vi "tvac_gui_chamber.vi"() -> ()   [LabVIEW 2017]
doc: "GUI For Thermal Vacuum Chamber - Rev 1.0 by S.O. 11/6/2017"
uses:
  Type_Defs/Zones.ctl
  Type_Defs/generalStatus.ctl
  Type_Defs/Digital_In_1.ctl
  Type_Defs/Digital_In_SW_States.ctl
  Type_Defs/Digital_In_SW_Wire_Faults.ctl
  Type_Defs/Cryo_Pump_MCC_Status.ctl
  Type_Defs/Cryo_Pump_MCC_CryoPump.ctl
  Type_Defs/Cryo_Pump_MCC_RoughingInterlock.ctl
  Type_Defs/Cryo_Pump_MCC_Status_Status.ctl
  Type_Defs/Cryo_Pump_Compressor_Status.ctl
  Type_Defs/Cryo_Pump_Compressor_Status_Status.ctl
  <vilib>/httpClient/ClientHandle.ctl
  <vilib>/Utility/miscctls.llb/LVPositionTypeDef.ctl
  <vilib>/Utility/error.llb/DialogType.ctl
  Type_Defs/Cryo_Pump_Plots.ctl
  <vilib>/Utility/miscctls.llb/LVBoundsTypeDef.ctl
  msg7171_linux.llb/send single message.vi
  <vilib>/httpClient/POSTBuffer.vi
  <vilib>/Utility/file.llb/Read Delimited Spreadsheet (string).vi
  <vilib>/Utility/file.llb/Write Delimited Spreadsheet (string).vi
  <vilib>/httpClient/LabVIEWHTTPClient.lvlib
panel:
  out "UTC":string
  out "Local Time":string
  out "Taskbar Status":T1 {"Chamber" format="%#_2g"; "Cryo" format="%#_2g"; "Roughing" format="%#_2g"}
  in  "importexe":dbl
  in  "Path to PNG file":path=path "C:/Users/stefan/Documents/GitHub/TVAC/head/Labview2017/TVAC_GUI/Visualization/chamber_test.png"
  in  "Moving 1":bool
  in  "TC1to45PicRef":refnum<vi>
  in  "profilearray":dbl[][](array[numeric])
  in  "LastSetPt":i32
  in  "string":string
  in  "tprofilesheet":string[][](array[string])
  in  "Custom Graph Selector":i32
  in  "exit":bool
  in  "AlarmColor":u32(colorbox)
  in  "Alarm String":string
  in  "Plot Color":u32(colorbox)=16860
  in  "Temperature":dbl format="%#_13g"
  in  "TC Label":string
  in  "Graph ON/OFF":u32(colorbox)=4250624
  in  "index (col)":i32
  in  "index (row)":i32
  out "working array":bool[](array[boolean])
  in  "Tab Control":T2(tab)
  in  "Log/Linear Y-Axis":u16(ring) items=["Linear", "Log"]
  in  "Total Time":dbl
  in  "Set Time TC Graph":bool
  in  "Graphing Selection":u16(ring) items=["User Selection", "Graph All Thermocouples", "Clear Graph"]
  in  "Time Scale":u16(ring) items=["Minutes", "Hours", "Seconds"]
  out "Waveform Chart":waveform(dbl)[](graph)
  out "Thermocouples":T3(array[cluster])
  in  "Log/Linear Y-Axis 6":u16(ring) items=["Linear", "Log"]
  in  "Log/Linear Y-Axis 5":u16(ring) items=["Linear", "Log"]
  in  "Log/Linear Y-Axis 3":u16(ring) items=["Linear", "Log"]
  in  "Log/Linear Y-Axis 2":u16(ring) items=["Linear", "Log"]
  in  "Total Time 6":dbl=30.0
  in  "Set Time TC Graph 6":bool
  in  "Time Scale 6":u16(ring) items=["Minutes", "Hours", "Seconds"]
  in  "Total Time 5":dbl=30.0
  in  "Set Time TC Graph 5":bool
  in  "Time Scale 5":u16(ring) items=["Minutes", "Hours", "Seconds"]
  in  "Total Time 4":dbl=30.0
  in  "Set Time TC Graph 4":bool
  in  "Time Scale 4":u16(ring) items=["Minutes", "Hours", "Seconds"]
  in  "Total Time 3":dbl=30.0
  in  "Set Time TC Graph 3":bool
  in  "Time Scale 3":u16(ring) items=["Minutes", "Hours", "Seconds"]
  in  "Total Time 2":dbl=30.0
  in  "Set Time TC Graph 2":bool
  in  "Time Scale 2":u16(ring) items=["Minutes", "Hours", "Seconds"]
  in  "Log/Linear Y-Axis 1":u16(ring) items=["Linear", "Log"]
  in  "Total Time 1":dbl=30.0
  in  "Set Time TC Graph 1":bool
  in  "Time Scale 1":u16(ring) items=["Minutes", "Hours", "Seconds"]
  in  "Custom Chart 2 Selection":i32[](listbox)=[0]
  in  "Custom Chart 1 Selection":i32[](listbox)=[0]
  out "Custom Chart 1":waveform(dbl)[](graph)
  in  "Custom Chart 3 Selection":i32[](listbox)=[0]
  in  "Custom Chart 4 Selection":i32[](listbox)=[0]
  in  "Custom Chart 5 Selection":i32[](listbox)=[0]
  in  "Custom Chart 6 Selection":i32[](listbox)=[0]
  out "Custom Chart 2":waveform(dbl)[](graph)
  out "Custom Chart 3":waveform(dbl)[](graph)
  out "Custom Chart 4":waveform(dbl)[](graph)
  out "Custom Chart 5":waveform(dbl)[](graph)
  out "Custom Chart 6":waveform(dbl)[](graph)
  in  "Log/Linear Y-Axis 4":u16(ring) items=["Linear", "Log"]
  in  "Complete Event List":i32(listbox)
  in  "Database Logging On/Off":bool
  out "Thermal Profile Compiling Summary":string
  out "Active Profile":bool
  out "ThermalProfileStatus":string
  out "Thermal Profile":cluster{dbl, dbl, "temp":dbl[][]}(graph)
  in  "Thermal Profile Loader":T4(tab)
  in  "ZoneSetup":T5={"Number of Set points"=0.0, "Zone Selection"=[8], "Initiate Setup"=FALSE, "Thermal Profile Name"="", "Saved Database Profiles"=0, "Import CSV as a Thermal Profile"=path "C:/Users/stefan/Documents/GitHub/TVAC/head/Labview2017/TVAC_GUI/DatabaseCSV/start.csv", "Import Profile"=FALSE, "LoadFromDatabase"=FALSE} {"Saved Database Profiles" items=["debug2"]}
  in  "RampSoakTimes":cluster{"RampSoakTimes":dbl[][]}
  in  "Zone 1":T6={"Zone Thermocouples"=[0], "Temperature Calculation"=0, "Thermocouples Selected"="", "Temperature Goal"=[], "Max Allowable Temp"="", "Min Allowable Temp"="", "Max Temp Slope (K/min)  "=""} {"Temperature Calculation" items=["Average", "Minimum", "Maximum"]}
  in  "Zone 2":T6={"Zone Thermocouples"=[0], "Temperature Calculation"=0, "Thermocouples Selected"="", "Temperature Goal"=[], "Max Allowable Temp"="", "Min Allowable Temp"="", "Max Temp Slope (K/min)  "=""} {"Temperature Calculation" items=["Average", "Minimum", "Maximum"]}
  in  "Zone 3":T6={"Zone Thermocouples"=[0], "Temperature Calculation"=0, "Thermocouples Selected"="", "Temperature Goal"=[], "Max Allowable Temp"="", "Min Allowable Temp"="", "Max Temp Slope (K/min)  "=""} {"Temperature Calculation" items=["Average", "Minimum", "Maximum"]}
  in  "Zone 4":T6={"Zone Thermocouples"=[0], "Temperature Calculation"=0, "Thermocouples Selected"="", "Temperature Goal"=[], "Max Allowable Temp"="", "Min Allowable Temp"="", "Max Temp Slope (K/min)  "=""} {"Temperature Calculation" items=["Average", "Minimum", "Maximum"]}
  in  "Zone 5":T6={"Zone Thermocouples"=[0], "Temperature Calculation"=0, "Thermocouples Selected"="", "Temperature Goal"=[], "Max Allowable Temp"="", "Min Allowable Temp"="", "Max Temp Slope (K/min)  "=""} {"Temperature Calculation" items=["Average", "Minimum", "Maximum"]}
  in  "Zone 6":T6={"Zone Thermocouples"=[0], "Temperature Calculation"=0, "Thermocouples Selected"="", "Temperature Goal"=[], "Max Allowable Temp"="", "Min Allowable Temp"="", "Max Temp Slope (K/min)  "=""} {"Temperature Calculation" items=["Average", "Minimum", "Maximum"]}
  in  "Zone 7":T6={"Zone Thermocouples"=[0], "Temperature Calculation"=0, "Thermocouples Selected"="", "Temperature Goal"=[], "Max Allowable Temp"="", "Min Allowable Temp"="", "Max Temp Slope (K/min)  "=""} {"Temperature Calculation" items=["Average", "Minimum", "Maximum"]}
  in  "Zone 8":T6={"Zone Thermocouples"=[0], "Temperature Calculation"=0, "Thermocouples Selected"="", "Temperature Goal"=[], "Max Allowable Temp"="", "Min Allowable Temp"="", "Max Temp Slope (K/min)  "=""} {"Temperature Calculation" items=["Average", "Minimum", "Maximum"]}
  in  "Zone 9":T6={"Zone Thermocouples"=[0], "Temperature Calculation"=0, "Thermocouples Selected"="", "Temperature Goal"=[], "Max Allowable Temp"="", "Min Allowable Temp"="", "Max Temp Slope (K/min)  "=""} {"Temperature Calculation" items=["Average", "Minimum", "Maximum"]}
  out "Compiled Profile Name":string
  in  "Database Rename":bool
  in  "New Compiled File Name":string
  in  "Compiled Rename":bool
  in  "2. Save Into Database and CSV":bool
  in  "1. Compile Profile":bool
  in  "3. Run Profile":bool
  in  "Rename Existing Database Profile":u16(ring) items=["debug2"]
  in  "HARD STOP":bool
  in  "Hold Profile":bool
  out "tpStatus":T7 {"Chamber" format="%#_2g"; "Cryo" format="%#_2g"; "Roughing" format="%#_2g"}
  out "GenStatus":T7 {"Chamber" format="%#_2g"; "Cryo" format="%#_2g"; "Roughing" format="%#_2g"}
  in  "Tab Control 2":T8(tab)=enum."TCs 76-80, 96-120"
  out "TC1to75visual":T9={"1"=TRUE, "2"=TRUE, "3"=TRUE, "4"=TRUE, "5"=TRUE, "6"=TRUE, "7"=TRUE, "8"=TRUE, "9"=TRUE, "10"=TRUE, "11"=TRUE, "12"=TRUE, "13"=TRUE, "14"=TRUE, "15"=TRUE, "16"=TRUE, "17"=TRUE, "18"=TRUE, "19"=TRUE, "20"=TRUE, "21"=TRUE, "22"=TRUE, "23"=TRUE, "24"=TRUE, "25"=TRUE, "26"=TRUE, "27"=TRUE, "28"=TRUE, "29"=TRUE, "30"=TRUE, "31"=TRUE, "32"=TRUE, "33"=TRUE, "34"=TRUE, "35"=TRUE, "36"=TRUE, "37"=TRUE, "38"=TRUE, "39"=TRUE, "40"=TRUE, "41"=TRUE, "42"=TRUE, "43"=TRUE, "44"=TRUE, "45"=TRUE, "46"=TRUE, "47"=TRUE, "48"=TRUE, "49"=TRUE, "50"=TRUE, "51"=TRUE, "52"=TRUE, "53"=TRUE, "54"=TRUE, "55"=TRUE, "56"=TRUE, "57"=TRUE, "58"=TRUE, "59"=TRUE, "60"=TRUE, "61"=TRUE, "62"=TRUE, "63"=TRUE, "64"=TRUE, "65"=TRUE, "66"=TRUE, "67"=TRUE, "68"=TRUE, "69"=TRUE, "70"=TRUE, "71"=TRUE, "72"=TRUE, "73"=TRUE, "74"=TRUE, "75"=TRUE, "new picture"=bytes[0]}
  in  "Reset All TC Positions":bool
  in  "Import UUT":bool
  out "Chamber Layout":T10 {"TC 120" format="%#_5g"; "TC 119" format="%#_5g"; "TC 118" format="%#_5g"; "TC 117" format="%#_5g"; "TC 116" format="%#_5g"; "TC 115" format="%#_5g"; "TC 114" format="%#_5g"; "TC 113" format="%#_5g"; "TC 112" format="%#_5g"; "TC 111" format="%#_5g"; "TC 110" format="%#_5g"; "TC 109" format="%#_5g"; "TC 108" format="%#_5g"; "TC 107" format="%#_5g"; "TC 106" format="%#_5g"; "TC 105" format="%#_5g"; "TC 104" format="%#_5g"; "TC 103" format="%#_5g"; "TC 102" format="%#_5g"; "TC 101" format="%#_5g"; "TC 100" format="%#_5g"; "TC 99" format="%#_5g"; "TC 98" format="%#_5g"; "TC 97" format="%#_5g"; "TC 96" format="%#_5g"; "TC 80" format="%#_5g"; "TC 79" format="%#_5g"; "TC 78" format="%#_5g"; "TC 77" format="%#_5g"; "TC 76" format="%#_5g"}
  out "Chamber Layout Picture":picture
  out "Miscellaneous TCs":T11
  in  "Events":enum32{"Current", "Past"}(tab)
  in  "Clear All Events":bool
  in  "Current Events (click to clear)":i32(listbox)
  in  "Export Events":bool
  in  "Event History":i32(listbox)
  in  "Errors":enum32{"Current", "Past"}(tab)
  in  "Current Errors (click to clear)":i32(listbox)
  in  "Clear All Errors":bool
  in  "Export Errors":bool
  in  "Error History":i32(listbox)
  in  "Query Expected Temperatures":cluster{"Expected Thermal Profile":bool}
  in  "Complete Event List 2":i32(listbox)
  in  "Query Thermocouples Selection":T12={"UUT Thermocouples (1-75)"=TRUE, "Shroud Thermocouples (96-120)"=TRUE, "Platen Thermocouples (76-80)"=TRUE}
  in  "Query Specific Gauge Pressures":T13={"Roughing Pressure"=TRUE, "Cryopump Pressure"=TRUE, "Chamber Pressure"=TRUE}
  in  "Select Path and Check Save Before Pressing Query":path
  in  "Save Results":bool
  in  "Query Database":bool
  in  "End Time UTC":timestamp format="%^<%H:%M:%S\n%Y/%m/%d>T"
  in  "Start Time UTC":timestamp format="%^<%H:%M:%S\n%Y/%m/%d>T"
  in  "Vacuum Commands":T14 {"LN2 Heater - Platen Duty Cycle %" min=0.0 max=100.0 step=1.0; "LN2 Heater - Shroud Duty Cycle %" min=0.0 max=100.0 step=1.0}
  in  "Interlock Status":T15
  in  "Compressor":T16
  in  "MCC Status":T18
  out "sw wf":T22
  out "in sw":T23
  out "in bits":T24
  out "value":cluster{bool, bool, bool, bool, bool, bool}
  in  "Engineering Interfaces":bool
  in  "getTvacStatus":bool=TRUE
  in  "GetError":bool=TRUE
  in  "ZoneTemps On":bool=TRUE
  in  "MCC On":bool=TRUE
  in  "Pressure On":bool=TRUE
  in  "TCs On":bool=TRUE
  in  "GetEvent":bool=TRUE
  in  "TVAC Labview":bool=TRUE
  in  "Local Debug":bool
  out "system log event":string
  out "error out":errorcluster
  # "Hidden Controls"
  # "Active Thermal Profile Commands"
  # "Create a New Thermal Profile"
  # "Import CSV as a Thermal Profile"
  # "Run Saved Database Profile"
  # "Set Pt #"
  # "Ramp Time (min)"
  # "Soak Time (min)"
  # "Set Pt #"
  # "Goal Temp (K)"
  # "Set Pt #"
  # "Goal Temp (K)"
  # "Set Pt #"
  # "Goal Temp (K)"
  # "Set Pt #"
  # "Goal Temp (K)"
  # "Set Pt #"
  # "Goal Temp (K)"
  # "Set Pt #"
  # "Goal Temp (K)"
  # "Set Pt #"
  # "Goal Temp (K)"
  # "Set Pt #"
  # "Goal Temp (K)"
  # "Set Pt #"
  # "Goal Temp (K)"
  # "Historical Database Query for Thermcouples and Pressure"
  # "General Vacuum and Heater Commands"
  # "General Vacuum Commands"
  # "Cryopump Commands"
  # "TDK Lambda Heaters"
  # "Turn Off Individual Get Calls to Server"
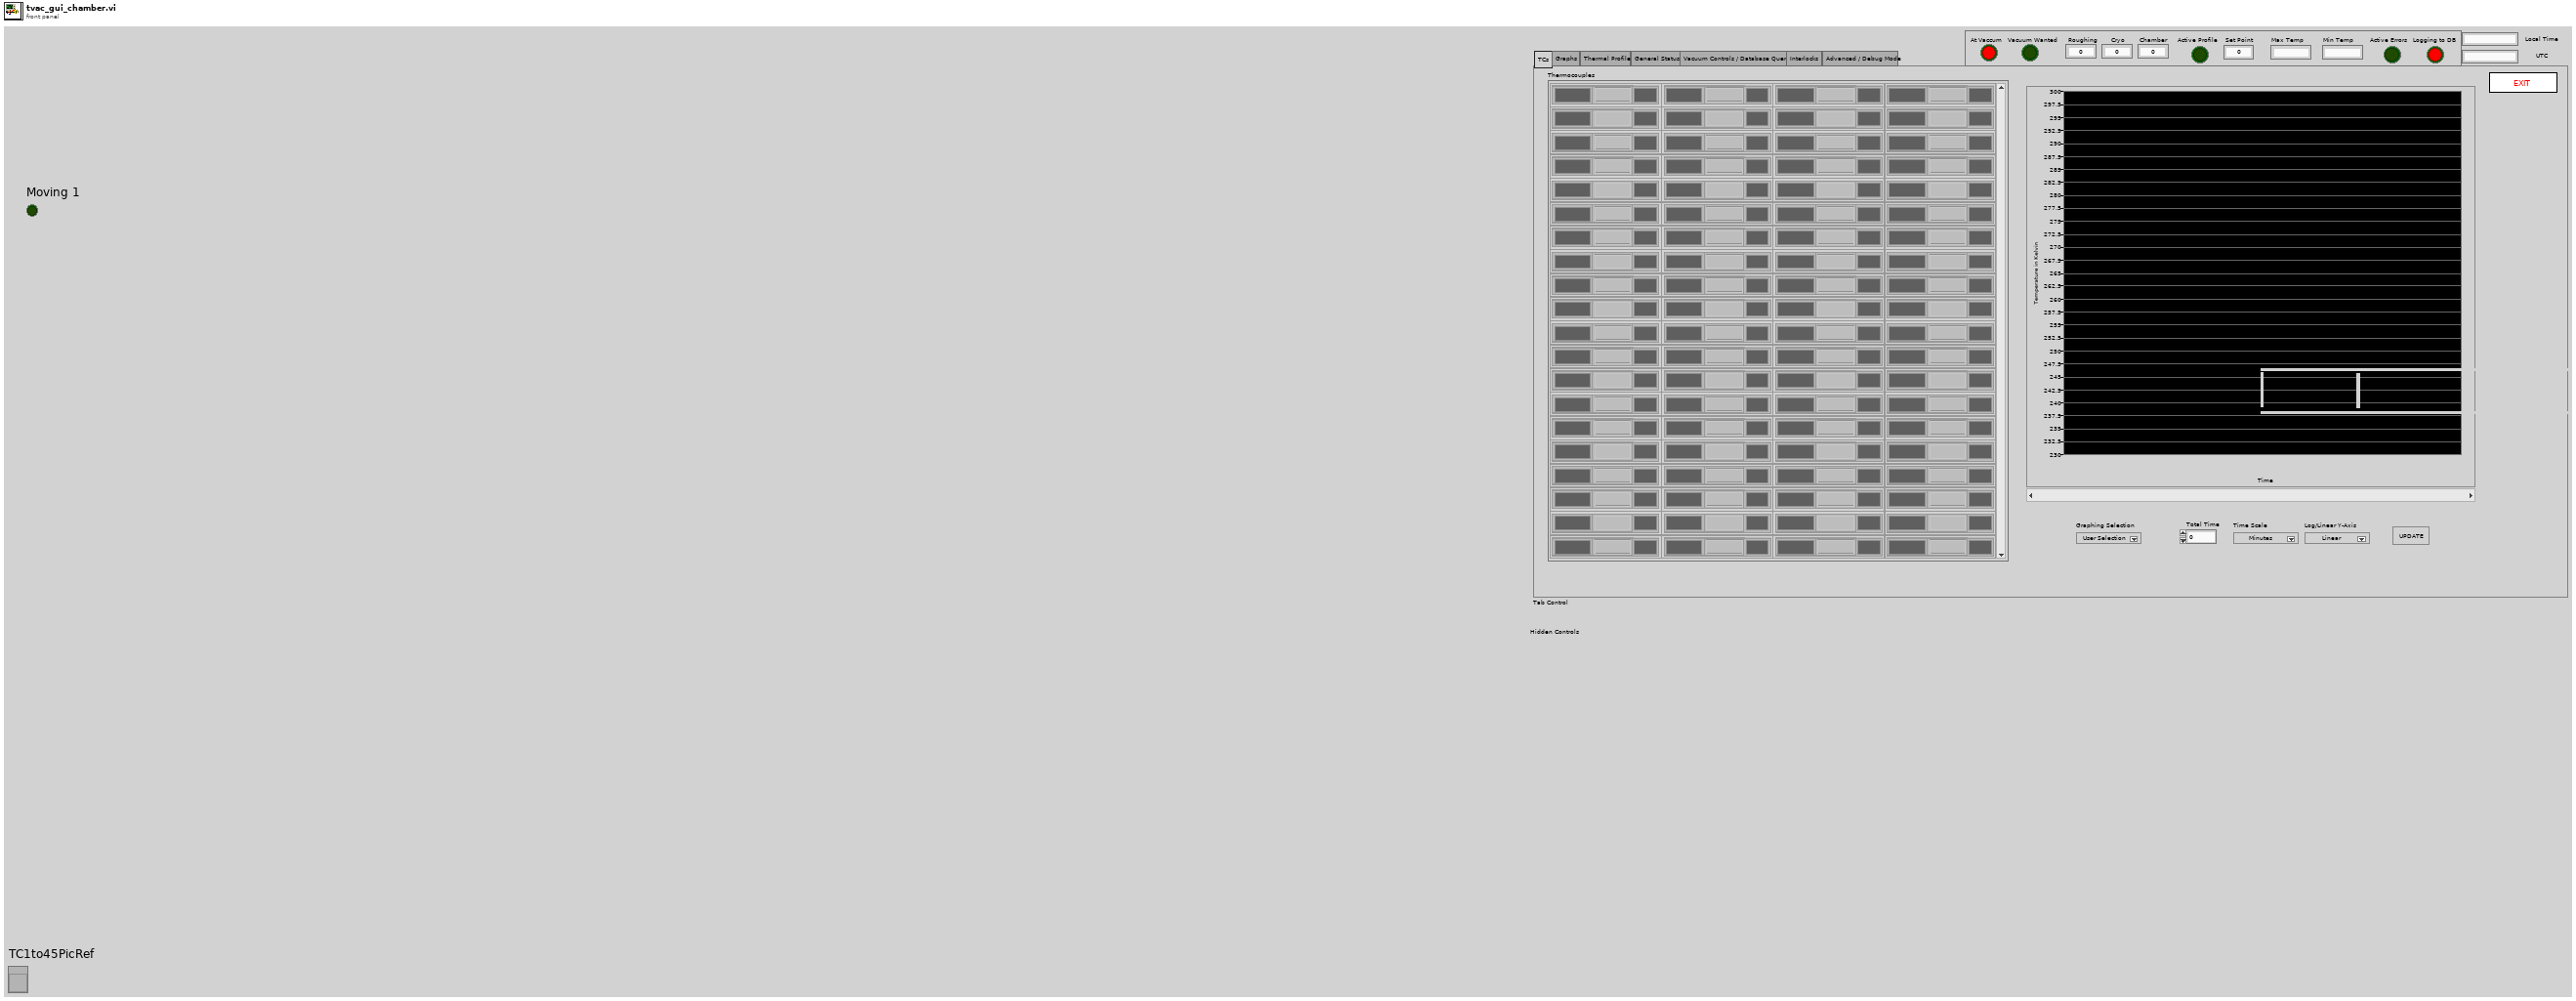
[diagram p1: front panel]
types:
  T1 = cluster{"At Vaccum":bool, "Vacuum Wanted":bool, "Roughing":dbl, "Cryo":dbl, "Chamber":dbl, "Active Profile":bool, "Set Point":dbl, "Max Temp":string, "Min Temp":string, "Active Errors":bool, "Logging to DB":bool}
  T2 = enum32{"TCs", "Graphs", "Thermal Profile", "General Status", "Vacuum Controls / Database Query", "Interlocks", "Advanced / Debug Mode"}
  T3 = cluster{"TC Label":string, "Alarm Status":string, "Alarm Color":u32, "Temperature":string, "PlotColor":u32, "Graph On/Off":u32}[][]
  T4 = enum32{"Setup", "Set Point Timing", "Zone 1", "Zone 2", "Zone 3", "Zone 4", "Zone 5", "Zone 6", "Zone 7", "Zone 8", "Zone 9", "Run"}
  T5 = cluster{"Number of Set points":dbl, "Zone Selection":i32[], "Initiate Setup":bool, "Thermal Profile Name":string, "Saved Database Profiles":u16, "Import CSV as a Thermal Profile":path, "Import Profile":bool, "LoadFromDatabase":bool}
  T6 = typedef "Zones.ctl" = cluster{"Zone Thermocouples":i32[], "Temperature Calculation":u16, "Thermocouples Selected":string, "Temperature Goal":dbl[][], "Max Allowable Temp":string, "Min Allowable Temp":string, "Max Temp Slope (K/min)  ":string}
  T7 = typedef "generalStatus.ctl" = cluster{"Set Point":dbl, "Vacuum Wanted":bool, "Profile State":string, "Active Profile":bool, "Roughing":dbl, "Cryo":dbl, "Chamber":dbl, "Zone Temps:   Z1              Z2              Z3              Z4             Z5              Z6             Z7              Z8              Z9":dbl[], "At Vacuum":bool, "Logging to DB":bool, "Max Temp":string, "Min Temp":string}
  T8 = enum32{"TCs 1-75", "TCs 76-80, 96-120", "TCs 81-95"}
  T9 = cluster{"1":bool, "2":bool, "3":bool, "4":bool, "5":bool, "6":bool, "7":bool, "8":bool, "9":bool, "10":bool, "11":bool, "12":bool, "13":bool, "14":bool, "15":bool, "16":bool, "17":bool, "18":bool, "19":bool, "20":bool, "21":bool, "22":bool, "23":bool, "24":bool, "25":bool, "26":bool, "27":bool, "28":bool, "29":bool, "30":bool, "31":bool, "32":bool, "33":bool, "34":bool, "35":bool, "36":bool, "37":bool, "38":bool, "39":bool, "40":bool, "41":bool, "42":bool, "43":bool, "44":bool, "45":bool, "46":bool, "47":bool, "48":bool, "49":bool, "50":bool, "51":bool, "52":bool, "53":bool, "54":bool, "55":bool, "56":bool, "57":bool, "58":bool, "59":bool, "60":bool, "61":bool, "62":bool, "63":bool, "64":bool, "65":bool, "66":bool, "67":bool, "68":bool, "69":bool, "70":bool, "71":bool, "72":bool, "73":bool, "74":bool, "75":bool, "new picture":picture}
  T10 = cluster{"TC 76":dbl, "TC 77":dbl, "TC 78":dbl, "TC 79":dbl, "TC 80":dbl, "TC 96":dbl, "TC 97":dbl, "TC 98":dbl, "TC 99":dbl, "TC 100":dbl, "TC 101":dbl, "TC 102":dbl, "TC 103":dbl, "TC 104":dbl, "TC 105":dbl, "TC 106":dbl, "TC 107":dbl, "TC 108":dbl, "TC 109":dbl, "TC 110":dbl, "TC 111":dbl, "TC 112":dbl, "TC 113":dbl, "TC 114":dbl, "TC 115":dbl, "TC 116":dbl, "TC 117":dbl, "TC 118":dbl, "TC 119":dbl, "TC 120":dbl}
  T11 = cluster{"TC 81 Platen LN2 In":dbl, "TC 82 Platen Vent 1":dbl, "TC 83 Platen Vent 2":dbl, "TC 84 Platen Vent 3":dbl, "TC 85 F-thruP LN2 In":dbl, "TC 86 F-thruP Vent 1":dbl, "TC 87 F-thruP Vent 2":dbl, "TC 88 F-thruP Vent 3":dbl, "TC 89 Chamber Wall 1":dbl, "TC 90 Chamber Wall 2":dbl, "TC 91 F-thruS LN2 In":dbl, "TC 92 F-thruS Vent 1":dbl, "TC 93 F-thru S Vent 2":dbl, "TC 94 Shroud Vent 1":dbl, "TC 95 Shroud Vent 2":dbl}
  T12 = cluster{"UUT Thermocouples (1-75)":bool, "Shroud Thermocouples (96-120)":bool, "Platen Thermocouples (76-80)":bool}
  T13 = cluster{"Roughing Pressure":bool, "Cryopump Pressure":bool, "Chamber Pressure":bool}
  T14 = cluster{"Vacuum State":bool, "LN2 Heater - Shroud Duty Cycle %":dbl[unit], "LN2 Heater - Platen Duty Cycle %":dbl[unit], "Start Heating Shroud":bool, "Start Heating Platen":bool, "Stop Cryopumping\n(Vacuum Not Maintained)":bool, "Stop Pumping and Shut Off Cryopump":bool, "Stop Roughing Pump":bool, "Vacuum State":string, "Last Response ":string}
  T15 = cluster{"Door Status":bool, "Over Temperature":bool, "Over Pressure":bool, "Gate Valve Interlock":bool, "TC / Temperature Interlock":bool, "Pressure Gauge Interlock":bool, "LN2 Interlock":bool, "Cryopump Gate Valve":bool, "TDK Lambda Heaters":bool, "Main Power Status":bool, "Helium Compressor Status":bool, "Roughing Pump Status":bool}
  T16 = typedef "Cryo_Pump_Compressor_Status.ctl" = cluster{"Helium Return Pressure (psig)":u32, "Helium Discharge Temp (K)":u32, "Water Inlet Temp (K)":u32, "Water Outlet Temp (K)":u32, "Firmware Version":string, "Operating Hours Elapsed":dbl, "Op-State":string, "RS-232 Config":string, "Status":T17}
  T17 = typedef "Cryo_Pump_Compressor_Status_Status.ctl" = cluster{"Solenoid ON":bool, "Pressure Alarm":bool, "Oil Level Alarm":bool, "Water Flow Alarm":bool, "Water Temp Alarm":bool, "Helium Temp Alarm":bool, "Phase/Fuse Alarm":bool, "Motor Temp Alarm":bool, "System ON":bool}
  T18 = typedef "Cryo_Pump_MCC_Status.ctl" = cluster{"Duty Cycle (0-100)":dbl, "1st stage Temp (K)":dbl, "2nd stage Temp (K)":dbl, "Cryo Pump Motor":T19, "Purge Valve State":bool, "Regen Error":string, "Regen Step":string, "Roughing Valve State":bool, "Roughing Interlock":T20, "Status":T21, "Tc Pressure":dbl}
  T19 = typedef "Cryo_Pump_MCC_CryoPump.ctl" = cluster{"Motor On":bool, "Ready":bool}
  T20 = typedef "Cryo_Pump_MCC_RoughingInterlock.ctl" = cluster{"Roughing Permission":bool, "Roughing Needed":bool, "Cryopump is Running":bool}
  T21 = typedef "Cryo_Pump_MCC_Status_Status.ctl" = cluster{"Pump On":bool, "Rough Open":bool, "Purge Open":bool, "Thermocouple Gauge On":bool, "Power Failure Occurred":bool}
  T22 = typedef "Digital_In_SW_Wire_Faults.ctl" = cluster{"LN2-P-Sol-Open: WF":bool, "LN2-P-Sol-Closed: WF":bool, "LN2-S-Sol-Open: WF":bool, "LN2-S-Sol-Closed: WF":bool, "CryoP-GV-Open: WF":bool, "CryoP-GV-Closed: WF":bool, "RoughP Powered: WF":bool, "RoughP_On_Sw: WF":bool}
  T23 = typedef "Digital_In_SW_States.ctl" = cluster{"LN2-P-Sol-Open":bool, "LN2-P-Sol-Closed":bool, "LN2-S-Sol-Open":bool, "LN2-S-Sol-Closed":bool, "CryoP-GV-Open":bool, "CryoP-GV-Closed":bool, "RoughP-GV-Open":bool, "RoughP-GV-Closed":bool, "RoughP Powered":bool, "RoughP_On_Sw":bool, "Chamber Closed":bool}
  T24 = typedef "Digital_In_1.ctl" = cluster{"PG-SW-RoughP-Relay 1":bool, "PG-SW-RoughP-Relay 2":bool, "PG-SW-CryoP-Relay 1":bool, "PG-SW-CryoP-Relay 2":bool, "PG-SW-Chamber-Relay 1":bool, "PG-SW-Chamber-Relay 2":bool, "LN2-P-Sol-Open: NC":bool, "LN2-P-Sol-Open: O":bool, "LN2-P-Sol-Closed: NC":bool, "LN2-P-Sol-Closed: O":bool, "LN2-S-Sol-Open: NC":bool, "LN2-S-Sol-Open: O":bool, "LN2-S-Sol-Closed: NC":bool, "LN2-S-Sol-Closed: O":bool, "CryoP-GV-Open: NC":bool, "CryoP-GV-Open: O":bool, "CryoP-GV-Closed: NC":bool, "CryoP-GV-Closed: O":bool, "RoughP-GV-Open":bool, "RoughP-GV-Closed":bool, "RoughP-Pwr: NC":bool, "RoughP-Pwr: O":bool, "RoughP-On: NC":bool, "RoughP-On: O":bool, "Air supply LN2 OK":bool, "Air supply OK":bool, "Front Door Closed":bool, "Back Door Closed":bool}
  T25 = typedef "LVPositionTypeDef.ctl" = cluster{"Left":i32, "Top":i32}
  T26 = cluster{"recordData":bool, "currentSetpoint":i32, "vacuumWanted":bool, "inPause":bool, "activeProfile":bool, "inRamp":bool, "inHold":bool, "CryoPressure":dbl, "ChamberPressure":dbl, "RoughingPressure":dbl, "OperationalVacuum":bool, "VacuumState":string}
  T27 = cluster{"profiles":cluster{"zone":i32, "average":string, "thermocouples":i32[], "maxTemp":i32, "minTemp":i32, "maxSlope":dbl, "thermalprofiles":cluster{"thermalsetpoint":i32, "tempgoal":i32, "ramp":i32, "soakduration":i32}[]}[]}
  T28 = cluster{"thermocouple":i32, "time":dbl, "temp":dbl, "working":bool, "alarm":i32}[]
  T29 = cluster{"Cp Stage 1 Temp":dbl[], "Cp Stage 2 Temp":dbl[]}
  T30 = typedef "LabVIEWHTTPClient.lvlib/ClientHandle.ctl" = refnum<k1>
  T31 = cluster{"ZoneSetup":cluster{"Number of Set points":dbl, "Zone Selection":i32[], "Initiate Setup":bool, "Thermal Profile Name":string, "Saved Database Profiles":u16, "Import CSV as a Thermal Profile":path, "Import Profile":bool, "LoadFromDatabase":bool}, "go":bool, "Http session":T30, "URL prefex":string, "index (row)":i32, "index (col)":i32, "Graph ON/OFF":u32, "TC Label":string, "Temperature":dbl, "AlarmColor":u32, "Plot Color":u32, "Alarm String":string, "Thermocouples":cluster{"TC Label":string, "Alarm Status":string, "Alarm Color":u32, "Temperature":string, "PlotColor":u32, "Graph On/Off":u32}[][], "working array":bool[], "i":i32, "NumberTCs":i32, "Custom Chart 1":waveform(dbl)[], "Custom Chart 1":waveform(dbl)[], "Pressure":dbl[], "numSensors":i32, "Database":dbl[], "PumpTemps":cluster{"Cp Stage 1 Temp":dbl[], "Cp Stage 2 Temp":dbl[]}, "Zones":dbl[], "Time":i32, "TCs":cluster{"thermocouple":i32, "time":dbl, "temp":dbl, "working":bool, "alarm":i32}[], "ZoneTemps":cluster{"ZoneTemps":dbl[]}, "Compressor":cluster{"CompressorTemp":dbl}, "ErrorArray":string[][], "PrevErrorArray":string[][], "MasterErrorArray":string[][], "tprofilesheet":string[][], "Zone 1":T6, "ZoneProfile":cluster{"profiles":cluster{"zone":i32, "average":string, "thermocouples":i32[], "maxTemp":i32, "minTemp":i32, "maxSlope":dbl, "thermalprofiles":cluster{"thermalsetpoint":i32, "tempgoal":i32, "ramp":i32, "soakduration":i32}[]}[]}, "ZonesSelected":bool[], "Zone 2":T6, "Zone 3":T6, "Zone 4":T6, "Zone 5":T6, "Zone 6":T6, "Zone 7":T6, "Zone 8":T6, "Zone 9":T6, "MasterEventArray":string[][], "PrevEventArray":string[][], "EventArray":string[][], "TC1to45PicRef":refnum<vi>, "TvacStatus":cluster{"recordData":bool, "currentSetpoint":i32, "vacuumWanted":bool, "inPause":bool, "activeProfile":bool, "inRamp":bool, "inHold":bool, "CryoPressure":dbl, "ChamberPressure":dbl, "RoughingPressure":dbl, "OperationalVacuum":bool, "VacuumState":string}, "MaxMinTemps":dbl[], "Interlock Status":cluster{"Door Status":bool, "Over Temperature":bool, "Over Pressure":bool, "Gate Valve Interlock":bool, "TC / Temperature Interlock":bool, "Pressure Gauge Interlock":bool, "LN2 Interlock":bool, "Cryopump Gate Valve":bool, "TDK Lambda Heaters":bool, "Main Power Status":bool, "Helium Compressor Status":bool, "Roughing Pump Status":bool}}
  T32 = cluster{"TC Label":string, "Alarm Status":string, "Alarm Color":u32, "Temperature":string, "PlotColor":u32, "Graph On/Off":u32}
  T33 = cluster{"time":string, "TCs":cluster{"thermocouple":i32, "time":dbl, "temp":dbl, "working":bool, "alarm":i32}[]}
  T34 = cluster{"name":string, "profiles":cluster{"zone":i32, "average":string, "thermocouples":i32[], "maxTemp":i32, "minTemp":i32, "maxSlope":i32, "thermalprofiles":cluster{"thermalsetpoint":i32, "tempgoal":i32, "ramp":i32, "soakduration":i32}[]}[]}
  T35 = enum16{"open", "replace", "create", "open or create", "replace or create", "replace or create with confirmation"}
  T36 = cluster{"zone":i32, "average":string, "thermocouples":i32[], "maxTemp":i32, "minTemp":i32, "maxSlope":dbl, "thermalprofiles":cluster{"thermalsetpoint":i32, "tempgoal":i32, "ramp":i32, "soakduration":i32}[]}
  T37 = cluster{"thermalsetpoint":i32, "tempgoal":i32, "ramp":i32, "soakduration":i32}
  T38 = cluster{"time":string[], "event":string[], "item":string[], "itemID":i32[], "details":string[], "actions":string[][]}
  T39 = cluster{"time":string[], "category":string[], "message":string[]}
  T40 = cluster{"CryoPressure":dbl, "ChamberPressure":dbl, "RoughingPressure":dbl}
  T41 = cluster{"pfeiffer_gauge":bool, "shi_compressor":bool, "shi_mcc":bool, "tdk_lambda":bool, "thermocouple":bool, "pc_104":bool}
  T42 = cluster{"At Vaccum":bool, "Vacuum Wanted":bool, "Roughing":dbl, "Cryo":dbl, "Chamber":dbl, "Active Profile":bool, "Set Point":dbl, "Max Temp":string, "Min Temp":string, "Active Errors":bool, "recordData":bool}
  T43 = cluster{"Set Point":dbl, "Vacuum Wanted":bool, "Profile State":string, "Active Profile":bool, "Roughing":dbl, "Cryo":dbl, "Chamber":dbl, "Zone Temps":dbl[], "At Vacuum":bool, "recordData":bool, "Max Temp":string, "Min Temp":string}
  T44 = typedef "imagedata.ctl" = cluster{"image type":i32, "image depth":i32, "image":u8[], "mask":u8[], "colors":u32[], "Rectangle":cluster{"left":i16, "top":i16, "right":i16, "bottom":i16}}
  T45 = typedef "LVPoint32TypeDef.ctl" = cluster{"Horizontal":i32, "Vertical":i32}
  T46 = typedef "LVRangeTypeDef.ctl" = cluster{"Minimum":dbl, "Maximum":dbl, "Increment":dbl, "Minor Increment":dbl, "Start":dbl}
  T47 = cluster{"zone":i32, "average":string, "thermocouples":i32[], "maxTemp":i32, "minTemp":i32, "maxSlope":dbl, "thermalprofiles":cluster{"thermalsetpoint":i32, "tempgoal":i32, "ramp":i32, "soakduration":i32}[]}[]
  T48 = typedef "LVRowAndColumnTypeDef.ctl" = cluster{"Row":i32, "Column":i32}
  T49 = cluster{"thermalsetpoint":i32, "tempgoal":i32, "ramp":i32, "soakduration":i32}[]
  T50 = cluster{"time":dbl[], "zone1":dbl[], "zone2":dbl[], "zone3":dbl[], "zone4":dbl[], "zone5":dbl[], "zone6":dbl[], "zone7":dbl[], "zone8":dbl[], "zone9":dbl[]}
  T51 = typedef "DialogType.ctl" = u16
  T52 = typedef "Cryo_Pump_Plots.ctl" = cluster{"Duty Cycle (0-100)":dbl, "1st stage Temp (K)":dbl, "2nd stage Temp (K)":dbl, "Helium Return Pressure (psig)":u32, "Helium Discharge Temp (K)":u32, "Water Inlet Temp (K)":u32, "Water Outlet Temp (K)":u32}
  T53 = cluster{"thermocouple":i32, "time":dbl, "temp":dbl, "working":bool, "alarm":i32}
  T54 = cluster{"[0]":dbl, "[1]":dbl, "[2]":dbl, "[3]":dbl, "[4]":dbl, "[5]":dbl, "[6]":dbl, "[7]":dbl, "[8]":dbl, "[9]":dbl, "[10]":dbl, "[11]":dbl, "[12]":dbl, "[13]":dbl, "[14]":dbl}
  T55 = cluster{"[0]":dbl, "[1]":dbl, "[2]":dbl, "[3]":dbl, "[4]":dbl, "[5]":dbl, "[6]":dbl, "[7]":dbl, "[8]":dbl, "[9]":dbl, "[10]":dbl, "[11]":dbl, "[12]":dbl, "[13]":dbl, "[14]":dbl, "[15]":dbl, "[16]":dbl, "[17]":dbl, "[18]":dbl, "[19]":dbl, "[20]":dbl, "[21]":dbl, "[22]":dbl, "[23]":dbl, "[24]":dbl, "[25]":dbl, "[26]":dbl, "[27]":dbl, "[28]":dbl, "[29]":dbl}
  T56 = typedef "LVBoundsTypeDef.ctl" = cluster{"Width":u32, "Height":u32}
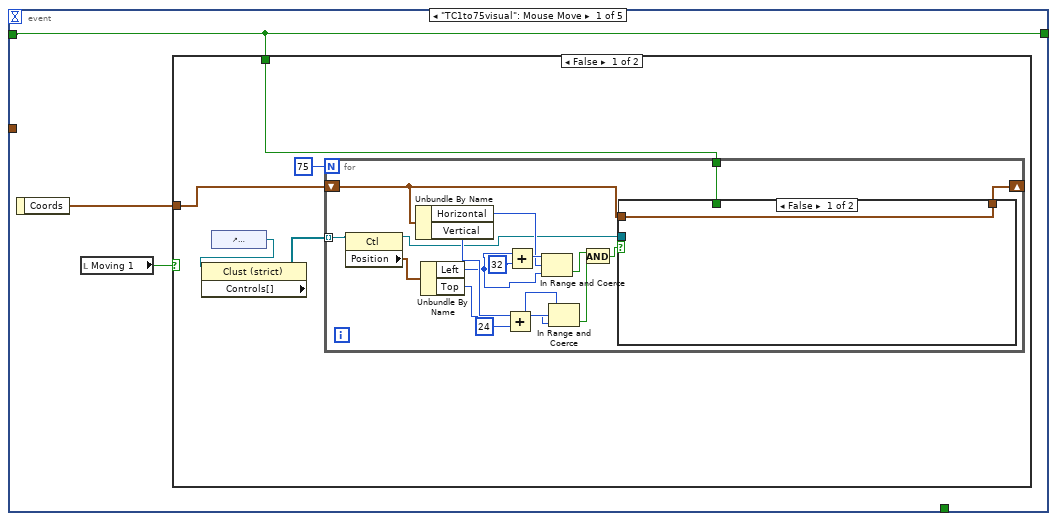
[diagram p3: hidden frame]
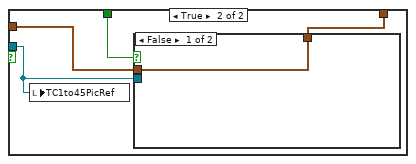
[diagram p4: hidden frame]
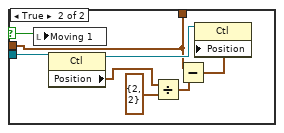
[diagram p5: hidden frame]
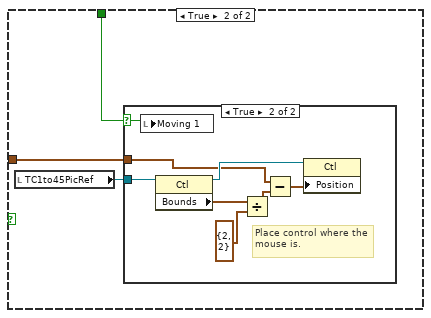
[diagram p6: hidden frame]
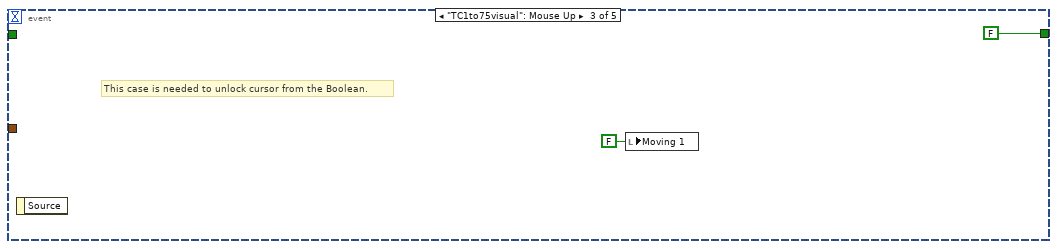
[diagram p8: hidden frame]
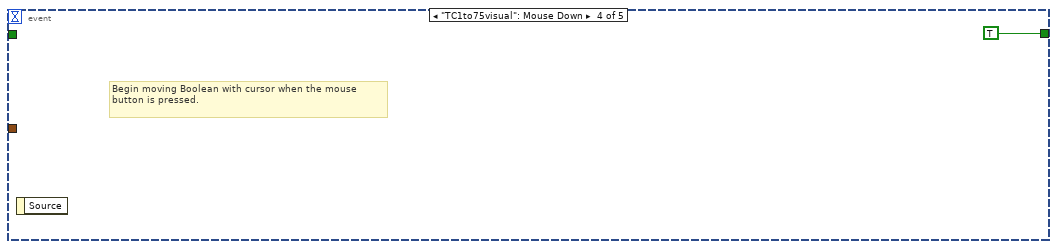
[diagram p9: hidden frame]
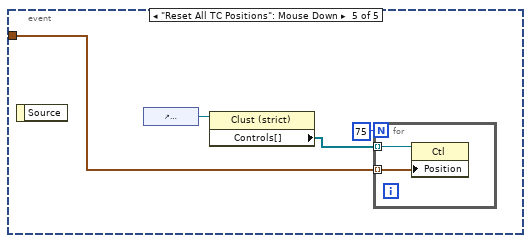
[diagram p10: hidden frame]
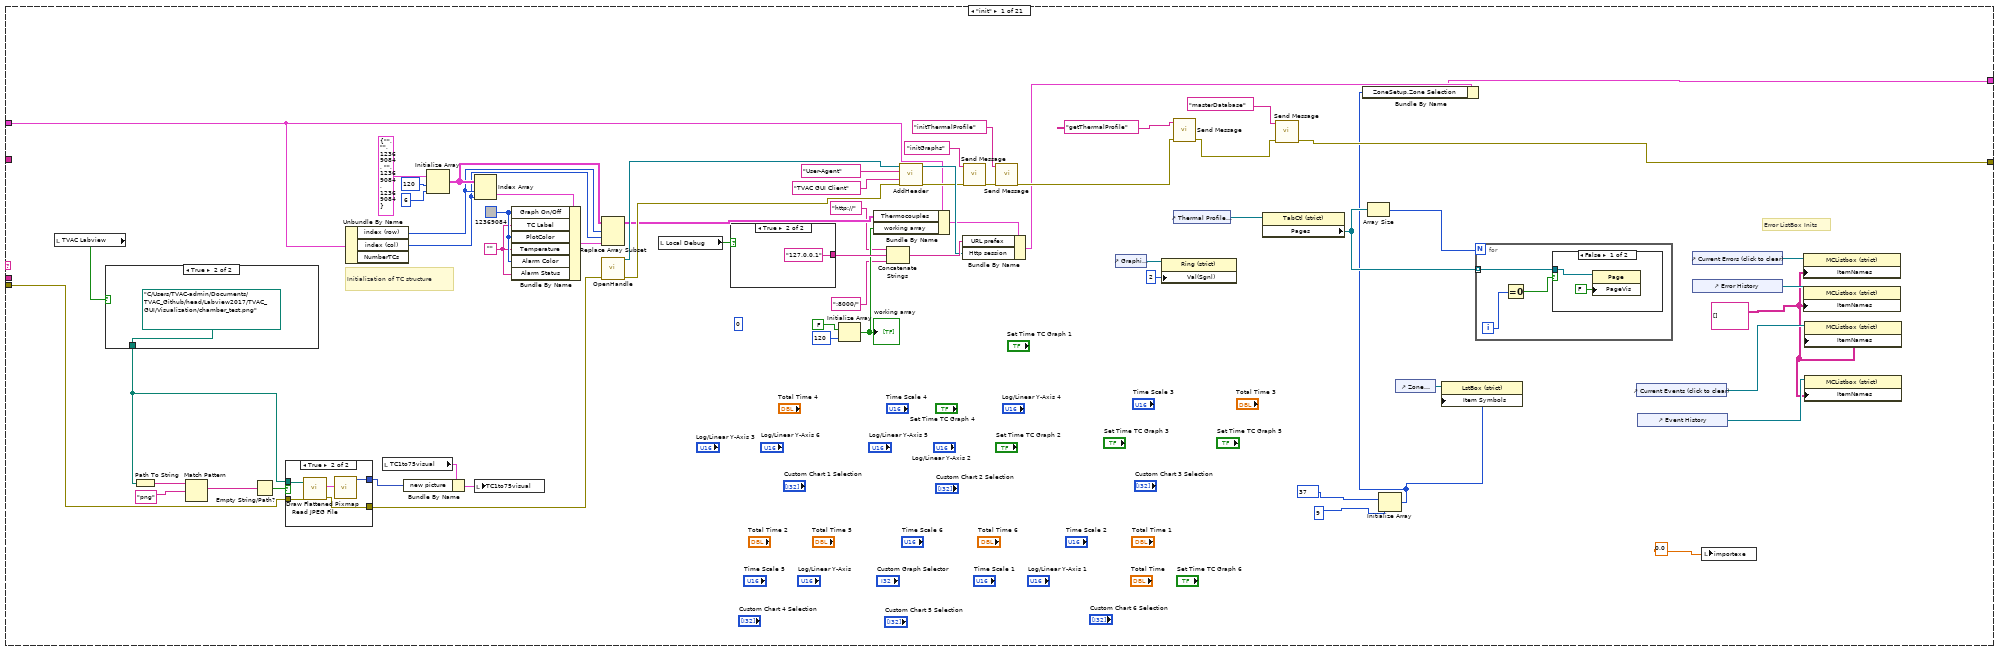
[diagram p11: hidden frame]
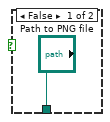
[diagram p12: hidden frame]
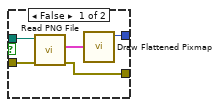
[diagram p13: hidden frame]
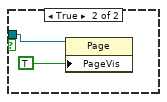
[diagram p14: hidden frame]
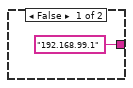
[diagram p15: hidden frame]
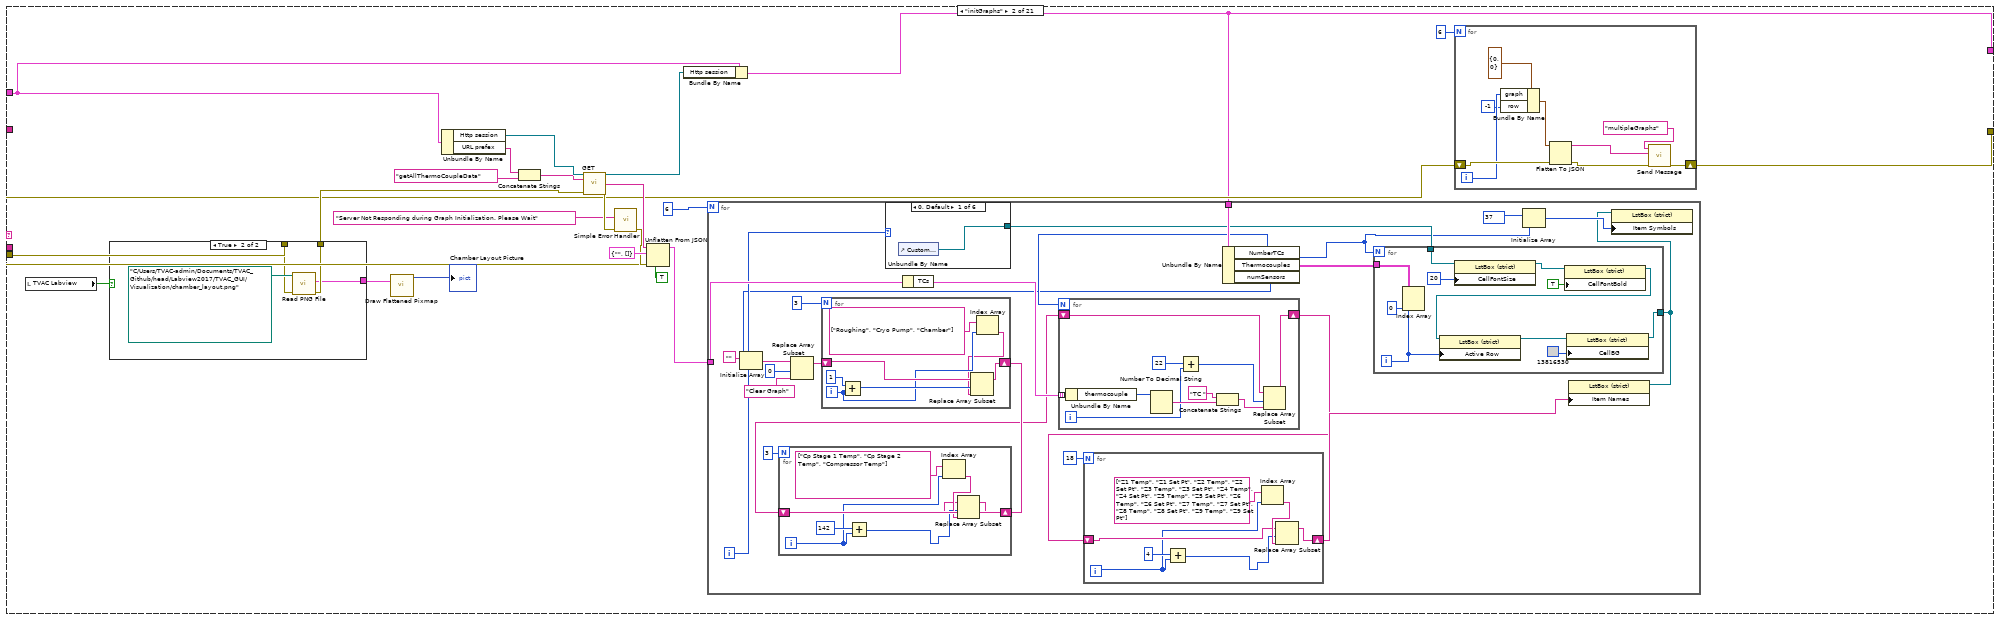
[diagram p16: hidden frame]
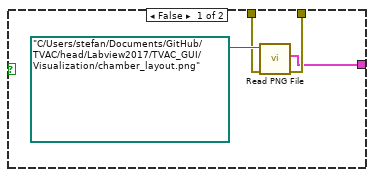
[diagram p17: hidden frame]
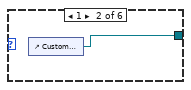
[diagram p18: hidden frame]
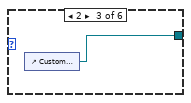
[diagram p19: hidden frame]
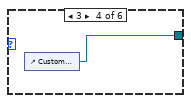
[diagram p20: hidden frame]
diagram:
  w3 = dbl[] []  # Database
  w20 = T26 {"recordData"=FALSE, "currentSetpoint"=0, "vacuumWanted"=FALSE, "inPause"=FALSE, "activeProfile"=FALSE, "inRamp"=FALSE, "inHold"=FALSE, "CryoPressure"=0.0, "ChamberPressure"=0.0, "RoughingPressure"=0.0, "OperationalVacuum"=FALSE, "VacuumState"=""}  # TvacStatus
  w24 = string[][] []  # MasterEventArray
  w22 = string[][] []  # EventArray
  w23 = string[][] []  # PrevEventArray
  w25 = string[][] []  # MasterErrorArray
  w28 = T27 {"profiles"=[]}  # ZoneProfile
  w37 = bool[] [FALSE, FALSE, FALSE, FALSE, FALSE, FALSE, FALSE, FALSE, FALSE]  # ZonesSelected
  w41 = string[][] []  # PrevErrorArray
  w42 = string[][] []  # ErrorArray
  w45 = cluster{"ZoneTemps":dbl[]} {"ZoneTemps"=[]}  # ZoneTemps
  w48 = dbl[] [24.54828257301887, 25.0, 20.035959453954195, 26.0, 28.926820041278148, 27.0, 21.321976066931608, 28.0, 29.197600688359813, 29.0, 29.117373424110085, 30.0, 21.092914485312942, 31.0, 27.791581465649088, 32.0, 24.70861457288988, 33.0]  # Zones
  w49 = T29 {"Cp Stage 1 Temp"=[0.0], "Cp Stage 2 Temp"=[0.0]}  # PumpTemps
  w51 = dbl[] [0.0, 0.0, 0.0]  # Pressure
  w69 = ""  # URL prefex
  w70 = T30 refnum  # Http session
  w71 = TRUE  # go
  # "Only use if the Visualization screen custom tc positions need to be updated"
  # "Interactive Picture Loop"
  n1 = call <vilib>:"OpenHandle.vi"() -> ("client handle out"=w10:T30, "error out"=w13:errorcluster)  [unwired: 14 in]
  n2 = call <vilib>:"AddHeader.vi"("client handle"=w10, "header"="User-Agent", "value"="TVAC GUI Client", "error in (no error)"=w13) -> ("client handle out"=w9:T30)  [unwired: 10 in, 1 out]
  n3 = local read "TVAC Labview"() -> (w16:bool)
  n4 = local read "Local Debug"() -> (w43:bool)
  n5 = call <vilib>:"CloseHandle.vi"("client handle"=w9, "error in (no error)"=errorcluster {"status"=FALSE, "code"=0, "source"=""}) -> ("error out"=w15:errorcluster)  [unwired: 13 in]
  n6 = call "Register Module.vi"("error in (no error)"=w15) -> ("error out"=w67:errorcluster)  [unwired: 9 in, 1 out]
  n7 = call "getData.vi"("TVAC Labview"=w16, "Local Debug"=w43) -> ()  [unwired: 10 in]
  n8 = call-poly "Send Message.vi"("error in (no error)"=w67, "event"="init") -> ("error out"=w66:errorcluster)  [unwired: 9 in]
  n9 = local read "Thermocouples"() -> (w53:T3)
  n10 = local read "Custom Chart 1"() -> (w52:waveform(dbl)[])
  n11 = Bundle("ZoneSetup"="ZoneSetup", "go"=w71, "Http session"=w70, "URL prefex"=w69, "index (row)"="index (row)", "index (col)"="index (col)", "Graph ON/OFF"="Graph ON/OFF", "TC Label"="TC Label", "Temperature"="Temperature", "AlarmColor"="AlarmColor", "Plot Color"="Plot Color", "Alarm String"="Alarm String", "Thermocouples"=w53, "working array"=bool[] [TRUE, TRUE, TRUE, TRUE, TRUE, TRUE, TRUE, TRUE, TRUE, TRUE, TRUE, TRUE, TRUE, TRUE, TRUE, TRUE, TRUE, TRUE, TRUE, TRUE, TRUE, TRUE, TRUE, TRUE, TRUE, TRUE, TRUE, TRUE, TRUE, TRUE, TRUE, TRUE, TRUE, TRUE, TRUE, TRUE, TRUE, TRUE, TRUE, TRUE, TRUE, TRUE, TRUE, TRUE, TRUE, TRUE, TRUE, TRUE, TRUE, TRUE, TRUE, TRUE, TRUE, TRUE, TRUE, TRUE, TRUE, TRUE, TRUE, TRUE, TRUE, TRUE, TRUE, TRUE, TRUE, TRUE, TRUE, TRUE, TRUE, TRUE, TRUE, TRUE, TRUE, TRUE, TRUE, TRUE, TRUE, TRUE, TRUE, TRUE, TRUE, TRUE, TRUE, TRUE, TRUE, TRUE, TRUE, TRUE, TRUE, TRUE, TRUE, TRUE, TRUE, TRUE, TRUE, TRUE, TRUE, TRUE, TRUE, TRUE, TRUE, TRUE, TRUE, TRUE, TRUE, TRUE, TRUE, TRUE, TRUE, TRUE, TRUE, TRUE, TRUE, TRUE, TRUE, TRUE, TRUE, TRUE, TRUE, TRUE], "i"=0, "NumberTCs"=120, "Custom Chart 1"=waveform(dbl)[] [{"t0"=timestamp(3592655846.063698 s since 1904-01-01), "dt"=1.0, "Y"=[0.0]}, {"t0"=timestamp(3592655846.063698 s since 1904-01-01), "dt"=1.0, "Y"=[0.0]}, {"t0"=timestamp(3592655846.063698 s since 1904-01-01), "dt"=1.0, "Y"=[9.415282917660304e-302]}, {"t0"=timestamp(0 s since 1904-01-01), "dt"=1.0, "Y"=[]}, {"t0"=timestamp(0 s since 1904-01-01), "dt"=1.0, "Y"=[]}, {"t0"=timestamp(0 s since 1904-01-01), "dt"=1.0, "Y"=[]}, {"t0"=timestamp(0 s since 1904-01-01), "dt"=1.0, "Y"=[]}, {"t0"=timestamp(0 s since 1904-01-01), "dt"=1.0, "Y"=[]}, {"t0"=timestamp(0 s since 1904-01-01), "dt"=1.0, "Y"=[]}, {"t0"=timestamp(0 s since 1904-01-01), "dt"=1.0, "Y"=[]}, {"t0"=timestamp(0 s since 1904-01-01), "dt"=1.0, "Y"=[]}, {"t0"=timestamp(0 s since 1904-01-01), "dt"=1.0, "Y"=[]}, {"t0"=timestamp(0 s since 1904-01-01), "dt"=1.0, "Y"=[]}, {"t0"=timestamp(0 s since 1904-01-01), "dt"=1.0, "Y"=[]}, {"t0"=timestamp(0 s since 1904-01-01), "dt"=1.0, "Y"=[]}, {"t0"=timestamp(0 s since 1904-01-01), "dt"=1.0, "Y"=[]}, {"t0"=timestamp(0 s since 1904-01-01), "dt"=1.0, "Y"=[]}, {"t0"=timestamp(0 s since 1904-01-01), "dt"=1.0, "Y"=[]}, {"t0"=timestamp(0 s since 1904-01-01), "dt"=1.0, "Y"=[]}, {"t0"=timestamp(0 s since 1904-01-01), "dt"=1.0, "Y"=[]}, {"t0"=timestamp(0 s since 1904-01-01), "dt"=1.0, "Y"=[]}, {"t0"=timestamp(0 s since 1904-01-01), "dt"=1.0, "Y"=[]}, {"t0"=timestamp(3592655846.063698 s since 1904-01-01), "dt"=1.0, "Y"=[nan]}, {"t0"=timestamp(3592655846.063698 s since 1904-01-01), "dt"=1.0, "Y"=[nan]}, {"t0"=timestamp(3592655846.063698 s since 1904-01-01), "dt"=1.0, "Y"=[nan]}, {"t0"=timestamp(3592655846.063698 s since 1904-01-01), "dt"=1.0, "Y"=[nan]}, {"t0"=timestamp(3592655846.063698 s since 1904-01-01), "dt"=1.0, "Y"=[nan]}, {"t0"=timestamp(3592655846.063698 s since 1904-01-01), "dt"=1.0, "Y"=[nan]}, {"t0"=timestamp(3592655846.063698 s since 1904-01-01), "dt"=1.0, "Y"=[nan]}, {"t0"=timestamp(3592655846.063698 s since 1904-01-01), "dt"=1.0, "Y"=[nan]}, {"t0"=timestamp(3592655846.063698 s since 1904-01-01), "dt"=1.0, "Y"=[nan]}, {"t0"=timestamp(3592655846.063698 s since 1904-01-01), "dt"=1.0, "Y"=[nan]}, {"t0"=timestamp(3592655846.063698 s since 1904-01-01), "dt"=1.0, "Y"=[756.0]}, {"t0"=timestamp(3592655846.063698 s since 1904-01-01), "dt"=1.0, "Y"=[nan]}, {"t0"=timestamp(3592655846.063698 s since 1904-01-01), "dt"=1.0, "Y"=[nan]}, {"t0"=timestamp(3592655846.063698 s since 1904-01-01), "dt"=1.0, "Y"=[nan]}, {"t0"=timestamp(3592655846.063698 s since 1904-01-01), "dt"=1.0, "Y"=[2268.0]}, {"t0"=timestamp(3592655846.063698 s since 1904-01-01), "dt"=1.0, "Y"=[3024.0]}, {"t0"=timestamp(3592655846.063698 s since 1904-01-01), "dt"=1.0, "Y"=[3780.0]}, {"t0"=timestamp(3592655846.063698 s since 1904-01-01), "dt"=1.0, "Y"=[0.0]}, {"t0"=timestamp(3592655846.063698 s since 1904-01-01), "dt"=1.0, "Y"=[0.0]}, {"t0"=timestamp(3592655846.063698 s since 1904-01-01), "dt"=1.0, "Y"=[0.0]}, {"t0"=timestamp(3592655846.064698 s since 1904-01-01), "dt"=1.0, "Y"=[nan]}, {"t0"=timestamp(3592655846.064698 s since 1904-01-01), "dt"=1.0, "Y"=[nan]}, {"t0"=timestamp(3592655846.064698 s since 1904-01-01), "dt"=1.0, "Y"=[nan]}, {"t0"=timestamp(3592655846.064698 s since 1904-01-01), "dt"=1.0, "Y"=[nan]}, {"t0"=timestamp(3592655846.064698 s since 1904-01-01), "dt"=1.0, "Y"=[nan]}, {"t0"=timestamp(3592655846.064698 s since 1904-01-01), "dt"=1.0, "Y"=[nan]}, {"t0"=timestamp(3592655846.064698 s since 1904-01-01), "dt"=1.0, "Y"=[nan]}, {"t0"=timestamp(3592655846.064698 s since 1904-01-01), "dt"=1.0, "Y"=[nan]}, {"t0"=timestamp(3592655846.064698 s since 1904-01-01), "dt"=1.0, "Y"=[nan]}, {"t0"=timestamp(3592655846.064698 s since 1904-01-01), "dt"=1.0, "Y"=[nan]}, {"t0"=timestamp(3592655846.064698 s since 1904-01-01), "dt"=1.0, "Y"=[nan]}, {"t0"=timestamp(3592655846.064698 s since 1904-01-01), "dt"=1.0, "Y"=[nan]}, {"t0"=timestamp(3592655846.064698 s since 1904-01-01), "dt"=1.0, "Y"=[nan]}, {"t0"=timestamp(3592655846.064698 s since 1904-01-01), "dt"=1.0, "Y"=[nan]}, {"t0"=timestamp(3592655846.064698 s since 1904-01-01), "dt"=1.0, "Y"=[nan]}, {"t0"=timestamp(3592655846.064698 s since 1904-01-01), "dt"=1.0, "Y"=[nan]}, {"t0"=timestamp(3592655846.064698 s since 1904-01-01), "dt"=1.0, "Y"=[nan]}, {"t0"=timestamp(3592655846.064698 s since 1904-01-01), "dt"=1.0, "Y"=[nan]}, {"t0"=timestamp(3592655846.064698 s since 1904-01-01), "dt"=1.0, "Y"=[nan]}, {"t0"=timestamp(3592655846.064698 s since 1904-01-01), "dt"=1.0, "Y"=[nan]}, {"t0"=timestamp(3592655846.064698 s since 1904-01-01), "dt"=1.0, "Y"=[nan]}, {"t0"=timestamp(3592655846.064698 s since 1904-01-01), "dt"=1.0, "Y"=[nan]}, {"t0"=timestamp(3592655846.064698 s since 1904-01-01), "dt"=1.0, "Y"=[nan]}, {"t0"=timestamp(3592655846.064698 s since 1904-01-01), "dt"=1.0, "Y"=[nan]}, {"t0"=timestamp(3592655846.064698 s since 1904-01-01), "dt"=1.0, "Y"=[nan]}, {"t0"=timestamp(3592655846.064698 s since 1904-01-01), "dt"=1.0, "Y"=[nan]}, {"t0"=timestamp(3592655846.064698 s since 1904-01-01), "dt"=1.0, "Y"=[nan]}, {"t0"=timestamp(3592655846.064698 s since 1904-01-01), "dt"=1.0, "Y"=[nan]}, {"t0"=timestamp(3592655846.064698 s since 1904-01-01), "dt"=1.0, "Y"=[nan]}, {"t0"=timestamp(3592655846.064698 s since 1904-01-01), "dt"=1.0, "Y"=[nan]}, {"t0"=timestamp(3592655846.064698 s since 1904-01-01), "dt"=1.0, "Y"=[nan]}, {"t0"=timestamp(3592655846.064698 s since 1904-01-01), "dt"=1.0, "Y"=[nan]}, {"t0"=timestamp(3592655846.064698 s since 1904-01-01), "dt"=1.0, "Y"=[nan]}, {"t0"=timestamp(3592655846.064698 s since 1904-01-01), "dt"=1.0, "Y"=[nan]}, {"t0"=timestamp(3592655846.064698 s since 1904-01-01), "dt"=1.0, "Y"=[nan]}, {"t0"=timestamp(3592655846.064698 s since 1904-01-01), "dt"=1.0, "Y"=[nan]}, {"t0"=timestamp(3592655846.064698 s since 1904-01-01), "dt"=1.0, "Y"=[nan]}, {"t0"=timestamp(3592655846.064698 s since 1904-01-01), "dt"=1.0, "Y"=[nan]}, {"t0"=timestamp(3592655846.064698 s since 1904-01-01), "dt"=1.0, "Y"=[nan]}, {"t0"=timestamp(3592655846.064698 s since 1904-01-01), "dt"=1.0, "Y"=[nan]}, {"t0"=timestamp(3592655846.064698 s since 1904-01-01), "dt"=1.0, "Y"=[nan]}, {"t0"=timestamp(3592655846.064698 s since 1904-01-01), "dt"=1.0, "Y"=[nan]}, {"t0"=timestamp(3592655846.064698 s since 1904-01-01), "dt"=1.0, "Y"=[nan]}, {"t0"=timestamp(3592655846.064698 s since 1904-01-01), "dt"=1.0, "Y"=[nan]}, {"t0"=timestamp(3592655846.064698 s since 1904-01-01), "dt"=1.0, "Y"=[nan]}, {"t0"=timestamp(3592655846.064698 s since 1904-01-01), "dt"=1.0, "Y"=[nan]}, {"t0"=timestamp(3592655846.064698 s since 1904-01-01), "dt"=1.0, "Y"=[nan]}, {"t0"=timestamp(3592655846.064698 s since 1904-01-01), "dt"=1.0, "Y"=[nan]}, {"t0"=timestamp(3592655846.064698 s since 1904-01-01), "dt"=1.0, "Y"=[nan]}, {"t0"=timestamp(3592655846.064698 s since 1904-01-01), "dt"=1.0, "Y"=[nan]}, {"t0"=timestamp(3592655846.064698 s since 1904-01-01), "dt"=1.0, "Y"=[nan]}, {"t0"=timestamp(3592655846.064698 s since 1904-01-01), "dt"=1.0, "Y"=[nan]}, {"t0"=timestamp(3592655846.064698 s since 1904-01-01), "dt"=1.0, "Y"=[nan]}, {"t0"=timestamp(3592655846.064698 s since 1904-01-01), "dt"=1.0, "Y"=[nan]}, {"t0"=timestamp(3592655846.064698 s since 1904-01-01), "dt"=1.0, "Y"=[nan]}, {"t0"=timestamp(3592655846.064698 s since 1904-01-01), "dt"=1.0, "Y"=[nan]}, {"t0"=timestamp(3592655846.064698 s since 1904-01-01), "dt"=1.0, "Y"=[nan]}, {"t0"=timestamp(3592655846.064698 s since 1904-01-01), "dt"=1.0, "Y"=[nan]}, {"t0"=timestamp(3592655846.064698 s since 1904-01-01), "dt"=1.0, "Y"=[nan]}, {"t0"=timestamp(3592655846.064698 s since 1904-01-01), "dt"=1.0, "Y"=[nan]}, {"t0"=timestamp(3592655846.064698 s since 1904-01-01), "dt"=1.0, "Y"=[nan]}, {"t0"=timestamp(3592655846.064698 s since 1904-01-01), "dt"=1.0, "Y"=[nan]}, {"t0"=timestamp(3592655846.064698 s since 1904-01-01), "dt"=1.0, "Y"=[nan]}, {"t0"=timestamp(3592655846.064698 s since 1904-01-01), "dt"=1.0, "Y"=[nan]}, {"t0"=timestamp(3592655846.064698 s since 1904-01-01), "dt"=1.0, "Y"=[nan]}, {"t0"=timestamp(3592655846.064698 s since 1904-01-01), "dt"=1.0, "Y"=[nan]}, {"t0"=timestamp(3592655846.064698 s since 1904-01-01), "dt"=1.0, "Y"=[nan]}, {"t0"=timestamp(3592655846.064698 s since 1904-01-01), "dt"=1.0, "Y"=[nan]}, {"t0"=timestamp(3592655846.064698 s since 1904-01-01), "dt"=1.0, "Y"=[nan]}, {"t0"=timestamp(3592655846.064698 s since 1904-01-01), "dt"=1.0, "Y"=[1512.0]}, {"t0"=timestamp(3592655846.064698 s since 1904-01-01), "dt"=1.0, "Y"=[nan]}, {"t0"=timestamp(3592655846.064698 s since 1904-01-01), "dt"=1.0, "Y"=[nan]}, {"t0"=timestamp(3592655846.064698 s since 1904-01-01), "dt"=1.0, "Y"=[nan]}, {"t0"=timestamp(3592655846.064698 s since 1904-01-01), "dt"=1.0, "Y"=[nan]}, {"t0"=timestamp(3592655846.064698 s since 1904-01-01), "dt"=1.0, "Y"=[nan]}, {"t0"=timestamp(3592655846.064698 s since 1904-01-01), "dt"=1.0, "Y"=[nan]}, {"t0"=timestamp(3592655846.064698 s since 1904-01-01), "dt"=1.0, "Y"=[nan]}, {"t0"=timestamp(3592655846.064698 s since 1904-01-01), "dt"=1.0, "Y"=[nan]}, {"t0"=timestamp(3592655846.064698 s since 1904-01-01), "dt"=1.0, "Y"=[nan]}, {"t0"=timestamp(3592655846.064698 s since 1904-01-01), "dt"=1.0, "Y"=[nan]}, {"t0"=timestamp(3592655846.064698 s since 1904-01-01), "dt"=1.0, "Y"=[nan]}, {"t0"=timestamp(3592655846.064698 s since 1904-01-01), "dt"=1.0, "Y"=[nan]}, {"t0"=timestamp(3592655846.064698 s since 1904-01-01), "dt"=1.0, "Y"=[nan]}, {"t0"=timestamp(3592655846.064698 s since 1904-01-01), "dt"=1.0, "Y"=[nan]}, {"t0"=timestamp(3592655846.064698 s since 1904-01-01), "dt"=1.0, "Y"=[nan]}, {"t0"=timestamp(3592655846.064698 s since 1904-01-01), "dt"=1.0, "Y"=[nan]}, {"t0"=timestamp(3592655846.064698 s since 1904-01-01), "dt"=1.0, "Y"=[nan]}, {"t0"=timestamp(3592655846.064698 s since 1904-01-01), "dt"=1.0, "Y"=[nan]}, {"t0"=timestamp(3592655846.064698 s since 1904-01-01), "dt"=1.0, "Y"=[nan]}, {"t0"=timestamp(3592655846.064698 s since 1904-01-01), "dt"=1.0, "Y"=[nan]}, {"t0"=timestamp(3592655846.064698 s since 1904-01-01), "dt"=1.0, "Y"=[nan]}, {"t0"=timestamp(3592655846.064698 s since 1904-01-01), "dt"=1.0, "Y"=[nan]}, {"t0"=timestamp(3592655846.064698 s since 1904-01-01), "dt"=1.0, "Y"=[nan]}, {"t0"=timestamp(3592655846.064698 s since 1904-01-01), "dt"=1.0, "Y"=[nan]}, {"t0"=timestamp(3592655846.064698 s since 1904-01-01), "dt"=1.0, "Y"=[nan]}, {"t0"=timestamp(3592655846.064698 s since 1904-01-01), "dt"=1.0, "Y"=[nan]}, {"t0"=timestamp(3592655846.064698 s since 1904-01-01), "dt"=1.0, "Y"=[nan]}, {"t0"=timestamp(3592655846.064698 s since 1904-01-01), "dt"=1.0, "Y"=[nan]}, {"t0"=timestamp(3592655846.064698 s since 1904-01-01), "dt"=1.0, "Y"=[nan]}, {"t0"=timestamp(3592655846.064698 s since 1904-01-01), "dt"=1.0, "Y"=[nan]}, {"t0"=timestamp(0 s since 1904-01-01), "dt"=1.0, "Y"=[]}, {"t0"=timestamp(0 s since 1904-01-01), "dt"=1.0, "Y"=[]}, {"t0"=timestamp(0 s since 1904-01-01), "dt"=1.0, "Y"=[]}], "Custom Chart 1"=w52, "Pressure"=w51, "numSensors"=145, "Database"=w3, "PumpTemps"=w49, "Zones"=w48, "Time"=0, "TCs"=T28 [], "ZoneTemps"=w45, "Compressor"=cluster{"CompressorTemp":dbl} {"CompressorTemp"=0.0}, "ErrorArray"=w42, "PrevErrorArray"=w41, "MasterErrorArray"=w25, "tprofilesheet"="tprofilesheet", "Zone 1"="Zone 1", "ZoneProfile"=w28, "ZonesSelected"=w37, "Zone 2"="Zone 2", "Zone 3"="Zone 3", "Zone 4"="Zone 4", "Zone 5"="Zone 5", "Zone 6"="Zone 6", "Zone 7"="Zone 7", "Zone 8"="Zone 8", "Zone 9"="Zone 9", "MasterEventArray"=w24, "PrevEventArray"=w23, "EventArray"=w22, "TC1to45PicRef"="TC1to45PicRef", "TvacStatus"=w20, "MaxMinTemps"=dbl[] [0.0, 0.0], "Interlock Status"="Interlock Status") -> (w57:T31)  [unwired: 1 in]
  n12 = invoke on="exit" class="Bool (strict)" method="Reinit To Default"() -> ()  [unwired: 3 in, 3 out]
  n13 = while {
    shift-left: w57 -> [w81]
    shift-right: [w79] -> _
    shift-right: [w80] -> w27
    shift-left: w66 -> [w85]
    stop <- w72 continue-if-true
    n14 = call "Get Message.vi"("error in (no error)"=w85) -> ("error out"=w84:errorcluster, "event buffer"=w77:string, "event"=w83:string, "source"=w82:string)  [unwired: 7 in]
    n15 = case shown="\"receiveLastError\"" w83 {
      selector: w83 -> [_ _ _ _ _ _ _ _ _ _ _ _ _ _ _ _ _ _ _ _ w4333]
      tunnel: [w108 w170 w285 w398 w2679 w3066 w3579 w3694 w3775 w3790 w3813 w3905 w3968 w3974 w3983 w4072 w4142 w4155 w4179 w4331 w4335] -> w79
      tunnel: w81 -> [w126 w179 w286 w391 w2729 w3058 w3593 w3699 w3775 w3789 w3807 w3899 w3969 w3974 w4007 w4101 w4141 w4156 w4179 w4327 w4335]
      tunnel: w77 -> [_ _ _ _ w2692 _ _ _ w3773 w3782 w3814 w3906 w3960 w3973 w4006 w4106 w4139 _ w4176 _ _]
      tunnel: w84 -> [w95 w184 w294 w392 w2675 w3054 w3595 w3689 w3776 w3783 w3811 w3903 w3961 w3975 w4005 w4105 w4140 w4161 _ w4330 w4334]
      tunnel: [w118 w172 w291 w400 w2708 w3064 w3595 w3689 w3776 w3783 w3811 w3903 w3961 w3975 w4005 w4105 w4140 w4161 _ w4329 w4332] -> w76
      tunnel: w82 -> [_ _ _ _ _ _ _ _ _ _ _ _ _ _ _ _ _ _ _ _ _]
      frame "init" {
        w103 = string[][] [] ("Item Names")
        (unwired) 0 ("index")
        w131 = ""
        w132 = u32 12369084 ("PlotColor")
        # "Error ListBox Inits"
        # "Initialization of TC structure"
        n16 = local read "TVAC Labview"() -> (w91:bool)
        n17 = case shown="True" w91 {
          tunnel: ["Path to PNG file" path "C:/Users/TVAC-admin/Documents/TVAC_Github/head/Labview2017/TVAC_GUI/Visualization/chamber_test.png" ("Path to PNG file")] -> w96
          frame False {
          }
          frame True {
          }
        }
        n18 = Path To String(path=w96) -> (string=w100:string)
        n19 = Match Pattern(string=w100, regular expression="png") -> (match substring=w98:string)  [unwired: 1 in, 3 out]
        n20 = Empty String/Path?(string/path=w98) -> (empty?=w97:bool)
        n21 = case shown="True" w97 {
          tunnel: [w155 w160] -> w93
          tunnel: w95 -> [w154 w157]
          tunnel: [w153 w158] -> w94
          tunnel: w96 -> [w151 w156]
          frame False {
            n22 = call <vilib>:"Read PNG File.vi"("error in (no error)"=w154, "path to PNG file"=w151) -> ("error out"=w153:errorcluster, "image data"=w152:T44)  [unwired: 7 in, 1 out]
            n23 = call <vilib>:"Draw Flattened Pixmap.vi"("image data"=w152) -> ("new picture"=w155:picture)  [unwired: 8 in]
          }
          frame True {
            n24 = call <vilib>:"Read JPEG File.vi"("error in (no error)"=w157, "path to JPEG file"=w156) -> ("error out"=w158:errorcluster, "image data"=w159:T44)  [unwired: 7 in, 1 out]
            n25 = call <vilib>:"Draw Flattened Pixmap.vi"("image data"=w159) -> ("new picture"=w160:picture)  [unwired: 8 in]
          }
        }
        n26 = Unbundle By Name(w126) -> ("index (row)"=w134:i32, "index (col)"=w133:i32)  [unwired: 1 out]
        n27 = local read "TC1to75visual"() -> (w101:T9)
        n28 = Bundle By Name(cluster=w101, "new picture"=w93) -> (w102:T9)
        n29 = Initialize Array(T32 {"TC Label"="", "Alarm Status"="", "Alarm Color"=12369084, "Temperature"="", "PlotColor"=12369084, "Graph On/Off"=12369084}, 120 ("dimension size"), 6 ("dimension size")) -> (w135:T3)
        n30 = Index Array(array=w135, index (row)=w134, index (col)=w133) -> (element=w130:T32)
        n31 = local write "TC1to75visual"(w102) -> ()
        n32 = Bundle By Name(cluster=w130, "Graph On/Off"=w132, "TC Label"=w131, "PlotColor"=w132, "Temperature"=w131, "Alarm Color"=w132, "Alarm Status"=w131) -> (w129:T32)
        n33 = Replace Array Subset(array=w135, new element=w129, index (row)=w134, index (col)=w133) -> (w123:T3)
        n34 = call <vilib>:"OpenHandle.vi"("error in (no error)"=w94) -> ("client handle out"=w145:T30, "error out"=w148:errorcluster)  [unwired: 13 in]
        n35 = local read "Local Debug"() -> (w139:bool)
        n36 = case shown="True" w139 {
          tunnel: ["192.168.99.1" ("Address") "127.0.0.1" ("Address")] -> w140
          frame False {
          }
          frame True {
          }
        }
        n37 = Initialize Array(FALSE ("Boolean"), 120 ("dimension size")) -> (w124:bool[])
        "working array" <- w124
        n38 = Bundle By Name(cluster=w126, "Thermocouples"=w123, "working array"=w124) -> (w125:T31)
        n39 = Concatenate Strings("http://" ("url"), w140, ":8000/" ("url")) -> (w144:string)
        n40 = call <vilib>:"AddHeader.vi"("client handle"=w145, "header"="User-Agent", "value"="TVAC GUI Client", "error in (no error)"=w148) -> ("client handle out"=w143:T30, "error out"=w142:errorcluster)  [unwired: 10 in]
        n41 = Bundle By Name(cluster=w125, "URL prefex"=w144, "Http session"=w143) -> (w111:T31)
        n42 = call-poly "Send Message.vi"("error in (no error)"=w142, "event"="initGraphs") -> ("error out"=w122:errorcluster)  [unwired: 9 in]
        n43 = call-poly "Send Message.vi"("error in (no error)"=w122, "event"="initThermalProfile") -> ("error out"=w120:errorcluster)  [unwired: 9 in]
        n44 = control-ref of="Graphing Selection"() -> (w90:refnum<vi>)
        n45 = property class="Ring (strict)"(reference=w90, "Val(Sgnl)"=u16 2 ("Value (Signaling)")) -> ()  [unwired: 1 in, 2 out]
        n46 = call-poly "Send Message.vi"("error in (no error)"=w120, "event"="getThermalProfile") -> ("error out"=w119:errorcluster)  [unwired: 9 in]
        n47 = control-ref of="Thermal Profile Loader"() -> (w116:refnum<vi>)
        n48 = property on="Property Node" class="TabCtl (strict)"(reference=w116) -> ("Pages"=w114:refnum<vi>[])  [unwired: 1 in, 2 out]
        n49 = call-poly "Send Message.vi"("error in (no error)"=w119, "event"="masterDatabase") -> ("error out"=w118:errorcluster)  [unwired: 9 in]
        n50 = Array Size(array=w114) -> (size(s)=w115:i32)
        n51 = Initialize Array(37, 9 ("dimension size")) -> (w109:i32[])
        n52 = Bundle By Name(cluster=w111, "ZoneSetup.Zone Selection"=w109) -> (w108:T31)
        n53 = control-ref of="Zone Selection"() -> (w110:refnum<vi>)
        n54 = property class="LstBox (strict)"(reference=w110, "Item Symbols"=w109) -> ()  [unwired: 1 in, 2 out]
        n55 = for {
          N: w115 -> [_]
          tunnel: w114 -> [w161] mode=indexing
          i -> [w163]
          n56 = Equal To 0?(x=w163) -> (x = 0?=w162:bool)
          n57 = case shown="False" w162 {
            tunnel: w161 -> [w164 w166]
            frame False {
              n58 = property on="Property Node" class="Page"(reference=w164, "PageVis"=FALSE ("Page Visible")) -> ()  [unwired: 1 in, 2 out]
            }
            frame True {
              n59 = property on="Property Node" class="Page"(reference=w166, "PageVis"=TRUE ("Page Selector Visible")) -> ()  [unwired: 1 in, 2 out]
            }
          }
        }
        n60 = control-ref of="Current Events (click to clear)"() -> (w105:refnum<vi>)
        n61 = control-ref of="Event History"() -> (w104:refnum<vi>)
        n62 = control-ref of="Current Errors (click to clear)"() -> (w107:refnum<vi>)
        n63 = control-ref of="Error History"() -> (w106:refnum<vi>)
        n64 = local write "importexe"(0.0 ("importexe")) -> ()
        n65 = property on="Property Node" class="MCListbox (strict)"(reference=w107, "ItemNames"=w103) -> ()  [unwired: 1 in, 2 out]
        n66 = property on="Property Node" class="MCListbox (strict)"(reference=w106, "ItemNames"=w103) -> ()  [unwired: 1 in, 2 out]
        n67 = property on="Property Node" class="MCListbox (strict)"(reference=w105, "ItemNames"=w103) -> ()  [unwired: 1 in, 2 out]
        n68 = property on="Property Node" class="MCListbox (strict)"(reference=w104, "ItemNames"=w103) -> ()  [unwired: 1 in, 2 out]
      }
      frame "initGraphs" {
        n69 = local read "TVAC Labview"() -> (w185:bool)
        n70 = case shown="True" w185 {
          tunnel: w184 -> [w204 w208]
          tunnel: [w203 w207] -> w183
          tunnel: [w202 w206] -> w182
          frame False {
            n71 = call <vilib>:"Read PNG File.vi"("error in (no error)"=w204, "path to PNG file"=path "C:/Users/stefan/Documents/GitHub/TVAC/head/Labview2017/TVAC_GUI/Visualization/chamber_layout.png") -> ("error out"=w203:errorcluster, "image data"=w202:T44)  [unwired: 7 in, 1 out]
          }
          frame True {
            n72 = call <vilib>:"Read PNG File.vi"("error in (no error)"=w208, "path to PNG file"=path "C:/Users/TVAC-admin/Documents/TVAC_Github/head/Labview2017/TVAC_GUI/Visualization/chamber_layout.png") -> ("error out"=w207:errorcluster, "image data"=w206:T44)  [unwired: 7 in, 1 out]
          }
        }
        n73 = call <vilib>:"Draw Flattened Pixmap.vi"("image data"=w182) -> ("new picture"=→"Chamber Layout Picture":picture)  [unwired: 8 in]
        n74 = Unbundle By Name(w179) -> ("Http session"=w192:T30, "URL prefex"=w190:string)
        n75 = Concatenate Strings(w190, "getAllThermoCoupleData" ("url")) -> (w191:string)
        n76 = call <vilib>:"GET.vi"("client handle"=w192, "url"=w191, "error in (no error)"=w183) -> ("client handle out"=w178:T30, "body"=w188:string, "error out"=w176:errorcluster)  [unwired: 9 in, 1 out]
        n77 = call <vilib>:"Simple Error Handler.vi"("error source (\" \")"="Server Not Responding during Graph Initialization. Please Wait", "error in (no error)"=w176) -> ("error out"=w175:errorcluster)  [unwired: 3 in, 4 out]
        n78 = Unflatten From JSON(JSON string=w188, type and defaults=T33 {"time"="", "TCs"=[]} ("Cluster"), default null elements? (F)=TRUE, error in (no error)=w175) -> (value=w187:T33, error out=w173:errorcluster)  [unwired: 3 in]
        n79 = Bundle By Name(cluster=w179, "Http session"=w178) -> (w170:T31)
        n80 = for {
          N: 6 ("Numeric") -> [_]
          tunnel: w187 -> [w231]
          tunnel: w170 -> [w230]
          i -> [w213]
          n81 = case shown="0, Default" w213 {
            tunnel: [w233 w234 w235 w236 w237 w238] -> w214
            frame 0, Default {
              n82 = control-ref of="Custom Chart 1 Selection"() -> (w233:refnum<vi>)
            }
            frame 1 {
              n83 = control-ref of="Custom Chart 2 Selection"() -> (w234:refnum<vi>)
            }
            frame 2 {
              n84 = control-ref of="Custom Chart 3 Selection"() -> (w235:refnum<vi>)
            }
            frame 3 {
              n85 = control-ref of="Custom Chart 4 Selection"() -> (w236:refnum<vi>)
            }
            frame 4 {
              n86 = control-ref of="Custom Chart 5 Selection"() -> (w237:refnum<vi>)
            }
            frame 5 {
              n87 = control-ref of="Custom Chart 6 Selection"() -> (w238:refnum<vi>)
            }
          }
          n88 = Unbundle By Name(w231) -> ("TCs"=w227:T28)
          n89 = Unbundle By Name(w230) -> ("NumberTCs"=w225:i32, "Thermocouples"=w232:T3, "numSensors"=w211:i32)
          n90 = Initialize Array("", w211) -> (w223:string[])
          n91 = Replace Array Subset(array=w223, new element="Clear Graph" ("new element/subarray"), index=0) -> (w220:string[])
          n92 = for {
            N: 3 -> [_]
            shift-right: [w258] -> w218
            shift-left: w220 -> [w259]
            i -> [w254]
            n93 = Add(x=1 ("index"), y=w254) -> (x+y=w256:i32)
            n94 = Index Array(array=string[] ["Roughing", "Cryo Pump", "Chamber"], index=w254) -> (element=w253:string)
            n95 = Replace Array Subset(array=w259, new element=w253, index=w256) -> (w258:string[])
          }
          n96 = for {
            N: 3 -> [_]
            shift-right: [w249] -> w217
            shift-left: w218 -> [w250]
            i -> [w246]
            n97 = Add(x=142 ("index"), y=w246) -> (x+y=w247:i32)
            n98 = Index Array(array=string[] ["Cp Stage 1 Temp", "Cp Stage 2 Temp", "Compressor Temp"], index=w246) -> (element=w251:string)
            n99 = Replace Array Subset(array=w250, new element=w251, index=w247) -> (w249:string[])
          }
          n100 = for {
            N: w225 -> [_]
            tunnel: w227 -> [w266] mode=indexing
            shift-right: [w260] -> w210
            shift-left: w217 -> [w262]
            i -> [w264]
            n101 = Unbundle By Name(w266) -> ("thermocouple"=w267:i32)
            n102 = Number To Decimal String(number=w267) -> (decimal integer string=w269:string)  [unwired: 1 in]
            n103 = Add(x=22 ("index"), y=w264) -> (x+y=w263:i32)
            n104 = Concatenate Strings("TC " ("string"), w269) -> (w261:string)
            n105 = Replace Array Subset(array=w262, new element=w261, index=w263) -> (w260:string[])
          }
          n106 = for {
            N: 18 -> [_]
            shift-right: [w239] -> w216
            shift-left: w210 -> [w241]
            i -> [w240]
            n107 = Add(x=4 ("index"), y=w240) -> (x+y=w242:i32)
            n108 = Index Array(array=string[] ["Z1 Temp", "Z1 Set Pt", "Z2 Temp", "Z2 Set Pt", "Z3 Temp", "Z3 Set Pt", "Z4 Temp", "Z4 Set Pt", "Z5 Temp", "Z5 Set Pt", "Z6 Temp", "Z6 Set Pt", "Z7 Temp", "Z7 Set Pt", "Z8 Temp", "Z8 Set Pt", "Z9 Temp", "Z9 Set Pt"], index=w240) -> (element=w244:string)
            n109 = Replace Array Subset(array=w241, new element=w244, index=w242) -> (w239:string[])
          }
          n110 = for {
            N: w211 -> [_]
            tunnel: w232 -> [w280]
            tunnel: w214 -> [w274]
            tunnel: [w270] -> w212
            i -> [w277]
            n111 = Index Array(array=w280, index (row)=w277, index (col)=0 ("disabled index (col)")) -> ()  [unwired: 1 out]
            n112 = property on="Property Node" class="LstBox (strict)"(reference=w274, "CellFontSize"=u32 20 ("Active Row:Cell Font:Size")) -> (reference out=w273:refnum<vi>)  [unwired: 1 in, 1 out]
            n113 = property on="Property Node" class="LstBox (strict)"(reference=w273, "CellFontBold"=TRUE ("Active Row:Cell Font:Bold")) -> (reference out=w272:refnum<vi>)  [unwired: 1 in, 1 out]
            n114 = property on="Property Node" class="LstBox (strict)"(reference=w272, "Active Row"=w277) -> (reference out=w271:refnum<vi>)  [unwired: 1 in, 1 out]
            n115 = property on="Property Node" class="LstBox (strict)"(reference=w271, "CellBG"=u32 13816530 ("Active Row:Cell Background Color")) -> (reference out=w270:refnum<vi>)  [unwired: 1 in, 1 out]
          }
          n116 = Initialize Array(37, w211) -> (w228:i32[])
          n117 = property on="Property Node" class="LstBox (strict)"(reference=w212, "Item Names"=w216) -> ()  [unwired: 1 in, 2 out]
          n118 = property on="Property Node" class="LstBox (strict)"(reference=w212, "Item Symbols"=w228) -> ()  [unwired: 1 in, 2 out]
        }
        n119 = for {
          N: 6 -> [_]
          shift-right: [w199] -> w172
          shift-left: w173 -> [w198]
          i -> [w196]
          n120 = Bundle By Name(cluster=cluster{"graph":i32, "row":i32} {"graph"=0, "row"=0}, "graph"=w196, "row"=-1) -> (w197:cluster{"graph":i32, "row":i32})
          n121 = Flatten To JSON(anything=w197, error in (no error)=w198) -> (JSON string=w194:string, 11:w193:errorcluster)  [unwired: 1 in]
          n122 = call-poly "Send Message.vi"("error in (no error)"=w193, "event buffer"=w194, "event"="multipleGraphs") -> ("error out"=w199:errorcluster)  [unwired: 8 in]
        }
      }
      frame "initThermalProfile" {
        n123 = Unbundle By Name(w286) -> ("Http session"=w300:T30, "URL prefex"=w298:string)
        n124 = Concatenate Strings(w298, "getAllThermoCoupleData" ("url")) -> (w299:string)
        n125 = call <vilib>:"GET.vi"("client handle"=w300, "url"=w299, "error in (no error)"=w294) -> ("client handle out"=w287:T30, "body"=w296:string, "error out"=w283:errorcluster)  [unwired: 9 in, 1 out]
        n126 = call <vilib>:"Simple Error Handler.vi"("error source (\" \")"="Server Not Responding during Graph Initialization. Please Wait", "error in (no error)"=w283) -> ("error out"=w282:errorcluster)  [unwired: 3 in, 4 out]
        n127 = Unflatten From JSON(JSON string=w296, type and defaults=T33 {"time"="", "TCs"=[]} ("Cluster"), default null elements? (F)=TRUE, error in (no error)=w282) -> (value=w295:T33, error out=w284:errorcluster)  [unwired: 3 in]
        n128 = Bundle By Name(cluster=w286, "Http session"=w287) -> (w285:T31)
        n129 = for {
          N: 9 ("Numeric") -> [_]
          tunnel: w295 -> [w323]
          tunnel: w285 -> [w322]
          i -> [w313]
          w301 = ""
          w306 = 81 ("dimension size")
          w307 = 80
          n130 = Add(x=w307, y=1 ("index")) -> (x+y=w308:i32)
          n131 = Initialize Array("", w308) -> (w317:string[])
          n132 = Replace Array Subset(array=w317, new element="Clear Selection" ("new element/subarray"), index=0) -> (w311:string[])
          n133 = case shown="4" w313 {
            tunnel: [w329 w334 w339 w344 w349 w354 w359 w364 w369] -> w314
            tunnel: [w328 w333 w338 w343 w348 w353 w358 w363 w368] -> w305
            tunnel: [w327 w332 w337 w342 w347 w352 w357 w362 w367] -> w304
            tunnel: [w326 w331 w336 w341 w346 w351 w356 w361 w366] -> w303
            tunnel: [w325 w330 w335 w340 w345 w350 w355 w360 w365] -> w302
            frame 0, Default {
              n134 = control-ref of="Zone Thermocouples"() -> (w329:refnum<vi>)
              n135 = control-ref of="Thermocouples Selected"() -> (w328:refnum<vi>)
              n136 = control-ref of="Min Allowable Temp"() -> (w326:refnum<vi>)
              n137 = control-ref of="Max Temp Slope (K/min)"() -> (w325:refnum<vi>)
              n138 = control-ref of="Max Allowable Temp"() -> (w327:refnum<vi>)
            }
            frame 1 {
              n139 = control-ref of="Max Temp Slope (K/min)"() -> (w330:refnum<vi>)
              n140 = control-ref of="Max Allowable Temp"() -> (w332:refnum<vi>)
              n141 = control-ref of="Min Allowable Temp"() -> (w331:refnum<vi>)
              n142 = control-ref of="Thermocouples Selected"() -> (w333:refnum<vi>)
              n143 = control-ref of="Zone Thermocouples"() -> (w334:refnum<vi>)
            }
            frame 2 {
              n144 = control-ref of="Max Temp Slope (K/min)"() -> (w335:refnum<vi>)
              n145 = control-ref of="Min Allowable Temp"() -> (w336:refnum<vi>)
              n146 = control-ref of="Thermocouples Selected"() -> (w338:refnum<vi>)
              n147 = control-ref of="Max Allowable Temp"() -> (w337:refnum<vi>)
              n148 = control-ref of="Zone Thermocouples"() -> (w339:refnum<vi>)
            }
            frame 3 {
              n149 = control-ref of="Max Allowable Temp"() -> (w342:refnum<vi>)
              n150 = control-ref of="Min Allowable Temp"() -> (w341:refnum<vi>)
              n151 = control-ref of="Max Temp Slope (K/min)"() -> (w340:refnum<vi>)
              n152 = control-ref of="Zone Thermocouples"() -> (w344:refnum<vi>)
              n153 = control-ref of="Thermocouples Selected"() -> (w343:refnum<vi>)
            }
            frame 4 {
              n154 = control-ref of="Max Temp Slope (K/min)"() -> (w345:refnum<vi>)
              n155 = control-ref of="Max Allowable Temp"() -> (w347:refnum<vi>)
              n156 = control-ref of="Min Allowable Temp"() -> (w346:refnum<vi>)
              n157 = control-ref of="Zone Thermocouples"() -> (w349:refnum<vi>)
              n158 = control-ref of="Thermocouples Selected"() -> (w348:refnum<vi>)
            }
            frame 5 {
              n159 = control-ref of="Min Allowable Temp"() -> (w351:refnum<vi>)
              n160 = control-ref of="Max Allowable Temp"() -> (w352:refnum<vi>)
              n161 = control-ref of="Max Temp Slope (K/min)"() -> (w350:refnum<vi>)
              n162 = control-ref of="Thermocouples Selected"() -> (w353:refnum<vi>)
              n163 = control-ref of="Zone Thermocouples"() -> (w354:refnum<vi>)
            }
            frame 6 {
              n164 = control-ref of="Max Temp Slope (K/min)"() -> (w355:refnum<vi>)
              n165 = control-ref of="Min Allowable Temp"() -> (w356:refnum<vi>)
              n166 = control-ref of="Max Allowable Temp"() -> (w357:refnum<vi>)
              n167 = control-ref of="Thermocouples Selected"() -> (w358:refnum<vi>)
              n168 = control-ref of="Zone Thermocouples"() -> (w359:refnum<vi>)
            }
            frame 7 {
              n169 = control-ref of="Max Temp Slope (K/min)"() -> (w360:refnum<vi>)
              n170 = control-ref of="Min Allowable Temp"() -> (w361:refnum<vi>)
              n171 = control-ref of="Max Allowable Temp"() -> (w362:refnum<vi>)
              n172 = control-ref of="Thermocouples Selected"() -> (w363:refnum<vi>)
              n173 = control-ref of="Zone Thermocouples"() -> (w364:refnum<vi>)
            }
            frame 8 {
              n174 = control-ref of="Min Allowable Temp"() -> (w366:refnum<vi>)
              n175 = control-ref of="Max Allowable Temp"() -> (w367:refnum<vi>)
              n176 = control-ref of="Zone Thermocouples"() -> (w369:refnum<vi>)
              n177 = control-ref of="Thermocouples Selected"() -> (w368:refnum<vi>)
              n178 = control-ref of="Max Temp Slope (K/min)"() -> (w365:refnum<vi>)
            }
          }
          n179 = Unbundle By Name(w323) -> ("TCs"=w319:T28)
          n180 = for {
            N: w307 -> [_]
            tunnel: w319 -> [w376] mode=indexing
            shift-right: [w370] -> w310
            shift-left: w311 -> [w372]
            i -> [w374]
            n181 = Unbundle By Name(w376) -> ("thermocouple"=w377:i32)
            n182 = Number To Decimal String(number=w377) -> (decimal integer string=w379:string)  [unwired: 1 in]
            n183 = Add(x=1 ("index"), y=w374) -> (x+y=w373:i32)
            n184 = Concatenate Strings("TC " ("string"), w379) -> (w371:string)
            n185 = Replace Array Subset(array=w372, new element=w371, index=w373) -> (w370:string[])
          }
          n186 = property class="Str"(reference=w305, "Text.Text"=w301) -> ()  [unwired: 1 in, 2 out]
          n187 = property class="Str"(reference=w304, "Value"=w301) -> ()  [unwired: 1 in, 2 out]
          n188 = property class="Str"(reference=w302, "Value"=w301) -> ()  [unwired: 1 in, 2 out]
          n189 = property class="Str"(reference=w303, "Value"=w301) -> ()  [unwired: 1 in, 2 out]
          n190 = Unbundle By Name(w322) -> ("Thermocouples"=w324:T3)
          n191 = for {
            N: w306 -> [_]
            tunnel: w324 -> [w390]
            tunnel: w314 -> [w384]
            tunnel: [w380] -> w312
            i -> [w387]
            n192 = Index Array(array=w390, index (row)=w387, index (col)=0 ("disabled index (col)")) -> ()  [unwired: 1 out]
            n193 = property on="Property Node" class="LstBox (strict)"(reference=w384, "CellFontSize"=u32 20 ("Active Row:Cell Font:Size")) -> (reference out=w383:refnum<vi>)  [unwired: 1 in, 1 out]
            n194 = property on="Property Node" class="LstBox (strict)"(reference=w383, "CellFontBold"=TRUE ("Active Row:Cell Font:Bold")) -> (reference out=w382:refnum<vi>)  [unwired: 1 in, 1 out]
            n195 = property on="Property Node" class="LstBox (strict)"(reference=w382, "Active Row"=w387) -> (reference out=w381:refnum<vi>)  [unwired: 1 in, 1 out]
            n196 = property on="Property Node" class="LstBox (strict)"(reference=w381, "CellBG"=u32 13816530 ("Active Row:Cell Background Color")) -> (reference out=w380:refnum<vi>)  [unwired: 1 in, 1 out]
          }
          n197 = Initialize Array(37, w306) -> (w320:i32[])
          n198 = property on="Property Node" class="LstBox (strict)"(reference=w312, "Item Symbols"=w320) -> ()  [unwired: 1 in, 2 out]
          n199 = property on="Property Node" class="LstBox (strict)"(reference=w312, "Item Names"=w310) -> ()  [unwired: 1 in, 2 out]
        }
        n200 = call-poly "Send Message.vi"("error in (no error)"=w284, "event buffer"="1000", "event"="multipleGraphs") -> ("error out"=w291:errorcluster)  [unwired: 8 in]
      }
      frame "", "Idle" {
        w395 = TRUE ("want seconds? (F)")
        n201 = control-ref of="Thermocouples"() -> (w408:refnum<vi>)
        n202 = property on="Property Node" class="Arr (strict)"(reference=w408) -> ("Position"=w407:T25)  [unwired: 1 in, 2 out]
        n203 = Unbundle By Name(w407) -> ("Left"=w406:i32, "Top"=w404:i32)
        n204 = Add(x=4, y=w406) -> (x+y=w402:i32)
        n205 = Add(x=w404, y=23 ("x")) -> (x+y=w401:i32)
        n206 = event shown="[0] Timeout" {
          selector: _ -> [_ _ _ _ _ _ _ _ _ _ _ _ _ _ _ _ _ _ _ _ _ _ _ _ _ _ _ _ _ _ _ _ _ _ _ _ _ _ _ _ _ _ _ _ _ _ _ _ _ _ _ _ _ _]
          dyn-events: _ -> [_ _ _ _ _ _ _ _ _ _ _ _ _ _ _ _ _ _ _ _ _ _ _ _ _ _ _ _ _ _ _ _ _ _ _ _ _ _ _ _ _ _ _ _ _ _ _ _ _ _ _ _ _ _]
          timeout: 200 ("milliseconds to wait") -> [_ _ _ _ _ _ _ _ _ _ _ _ _ _ _ _ _ _ _ _ _ _ _ _ _ _ _ _ _ _ _ _ _ _ _ _ _ _ _ _ _ _ _ _ _ _ _ _ _ _ _ _ _ _]
          tunnel: [w412 w495 w512 w529 w546 w563 w580 w596 w621 w644 w737 w801 w866 w931 w996 w1061 w1126 w1191 w1255 w1261 w1301 w1366 w1368 w1413 w1437 w1450 w1637 w1719 w1760 w1807 w1849 w1880 w1900 w1990 w2044 w2098 w2152 w2206 w2260 w2314 w2368 w2422 w2473 w2477 w2484 w2509 w2535 w2568 w2582 w2607 w2630 w2646 w2662 w2668] -> w400
          tunnel: [w417 w497 w514 w531 w548 w565 w582 w595 w617 w645 w731 w802 w867 w932 w997 w1062 w1127 w1192 w1258 w1274 w1302 w1364 w1370 w1410 w1434 w1453 w1635 w1715 w1756 w1805 w1847 w1875 w1912 w1989 w2043 w2097 w2151 w2205 w2259 w2313 w2367 w2421 w2475 w2479 w2482 w2515 w2548 w2565 w2585 w2610 w2632 w2648 w2664 w2671] -> w398
          tunnel: w391 -> [w418 w497 w514 w531 w548 w565 w582 w595 w617 w646 w733 w802 w867 w932 w997 w1062 w1127 w1192 w1259 w1265 w1312 w1365 w1370 w1411 w1435 w1454 w1636 w1716 w1757 w1806 w1848 w1876 w1912 w1989 w2043 w2097 w2151 w2205 w2259 w2313 w2367 w2421 w2475 w2479 w2482 w2515 w2548 w2566 w2586 w2611 w2633 w2649 w2665 w2671]
          tunnel: w402 -> [_ _ _ _ _ _ _ _ _ w643 _ _ _ _ _ _ _ _ _ _ _ _ _ _ _ _ _ _ _ _ _ _ _ _ _ _ _ _ _ _ _ _ _ _ _ _ _ _ _ _ _ _ _ _]
          tunnel: w401 -> [_ _ _ _ _ _ _ _ _ w640 _ _ _ _ _ _ _ _ _ _ _ _ _ _ _ _ _ _ _ _ _ _ _ _ _ _ _ _ _ _ _ _ _ _ _ _ _ _ _ _ _ _ _ _]
          tunnel: w392 -> [w414 w496 w513 w530 w547 w564 w581 w600 w623 w644 w737 w801 w866 w931 w996 w1061 w1126 w1191 w1252 w1266 w1307 w1366 w1376 w1414 w1438 w1448 w1638 w1719 w1760 w1807 w1849 w1880 w1901 w1990 w2044 w2098 w2152 w2206 w2260 w2314 w2368 w2422 w2474 w2478 w2485 w2512 w2547 w2569 w2587 w2612 w2627 w2643 w2659 w2670]
          event Timeout {
            n207 = event-data() -> ("Time"=w416:u32)  [unwired: 1 in, 1 out]
            n208 = Unbundle By Name(w418) -> ("Time"=w420:i32)
            n209 = Subtract(x=w416, y=w420) -> (x-y=w409:u32)
            n210 = Greater?(x=w409, y=u32 5000 ("millisecond multiple")) -> (0:w413:bool)
            n211 = case shown="True" w413 {
              tunnel: w418 -> [w431 w455]
              tunnel: [w431 w454] -> w417
              tunnel: w416 -> [_ w453]
              tunnel: [w430 w432] -> w415
              tunnel: w414 -> [w430 w452]
              frame False {
              }
              frame True {
                n212 = case shown="True" "TCs On" {
                  tunnel: w452 -> [w466 w470]
                  tunnel: [w466 w468] -> w451
                  frame False {
                  }
                  frame True {
                    n213 = call-poly "Send Message.vi"("Destination Module"="getData.vi", "error in (no error)"=w470, "event"="getTC") -> ("error out"=w468:errorcluster)  [unwired: 8 in]
                  }
                }
                n214 = Bundle By Name(cluster=w455, "Time"=w453) -> (w454:T31)
                n215 = case shown="True" "Pressure On" {
                  tunnel: w451 -> [w481 w484]
                  tunnel: [w481 w482] -> w450
                  frame False {
                  }
                  frame True {
                    n216 = call-poly "Send Message.vi"("Destination Module"="getData.vi", "error in (no error)"=w484, "event"="getPressure") -> ("error out"=w482:errorcluster)  [unwired: 8 in]
                  }
                }
                n217 = case shown="True" "MCC On" {
                  tunnel: w450 -> [w476 w478]
                  tunnel: [w476 w477] -> w449
                  frame False {
                  }
                  frame True {
                    n218 = call-poly "Send Message.vi"("Destination Module"="getData.vi", "error in (no error)"=w478, "event"="getMCCData") -> ("error out"=w477:errorcluster)  [unwired: 8 in]
                  }
                }
                n219 = case shown="True" "ZoneTemps On" {
                  tunnel: w449 -> [w471 w475]
                  tunnel: [w471 w472] -> w436
                  frame False {
                  }
                  frame True {
                    n220 = call-poly "Send Message.vi"("Destination Module"="getData.vi", "error in (no error)"=w475, "event"="getZoneTemps") -> ("error out"=w472:errorcluster)  [unwired: 8 in]
                  }
                }
                n221 = case shown="True" "GetError" {
                  tunnel: w436 -> [w486 w488]
                  tunnel: [w486 w487] -> w443
                  frame False {
                  }
                  frame True {
                    n222 = call-poly "Send Message.vi"("Destination Module"="getData.vi", "error in (no error)"=w488, "event"="getLastError") -> ("error out"=w487:errorcluster)  [unwired: 8 in]
                  }
                }
                n223 = case shown="True" "GetEvent" {
                  tunnel: w443 -> [w461 w464]
                  tunnel: [w461 w463] -> w441
                  frame False {
                  }
                  frame True {
                    n224 = call-poly "Send Message.vi"("Destination Module"="getData.vi", "error in (no error)"=w464, "event"="getLastEvent") -> ("error out"=w463:errorcluster)  [unwired: 8 in]
                  }
                }
                n225 = case shown="True" "getTvacStatus" {
                  tunnel: w441 -> [w456 w459]
                  tunnel: [w456 w458] -> w437
                  frame False {
                  }
                  frame True {
                    n226 = call-poly "Send Message.vi"("Destination Module"="getData.vi", "error in (no error)"=w459, "event"="getTvacStatus") -> ("error out"=w458:errorcluster)  [unwired: 8 in]
                  }
                }
                n227 = call-poly "Send Message.vi"("Destination Module"="getData.vi" ("event"), "error in (no error)"=w437, "event"="getDatabase") -> ("error out"=w433:errorcluster)  [unwired: 8 in]
                n228 = call-poly "Send Message.vi"("Destination Module"="getData.vi" ("event"), "error in (no error)"=w433, "event"="getSystemPower") -> ("error out"=w432:errorcluster)  [unwired: 8 in]
              }
            }
            n229 = Greater?(x=w409, y=u32 1000 ("millisecond multiple")) -> (0:w410:bool)
            n230 = case shown="True" w410 {
              tunnel: w415 -> [w421 w428]
              tunnel: [w421 w424] -> w412
              frame False {
              }
              frame True {
                n231 = call-poly "Send Message.vi"("error in (no error)"=w428, "event"="masterDatabase") -> ("error out"=w427:errorcluster)  [unwired: 9 in]
                n232 = call-poly "Send Message.vi"("error in (no error)"=w427, "event"="graphTC") -> ("error out"=w426:errorcluster)  [unwired: 9 in]
                n233 = call-poly "Send Message.vi"("error in (no error)"=w426, "event buffer"="1000", "event"="multipleGraphs") -> ("error out"=w424:errorcluster)  [unwired: 8 in]
              }
            }
          }
          event "Custom Chart 1 Selection": Mouse Down {
            n234 = event-data() -> ("CtlRef"=w494:refnum<vi>, "Coords"=w493:T45)  [unwired: 1 in, 6 out]
            n235 = invoke on="Invoke Node" class="LstBox (strict)" method="Point To Row"(reference=w494, "Point"=w493) -> ("InBounds"=w491:bool, "Row"=w492:i32)  [unwired: 5 in, 5 out]
            n236 = case shown="True" w491 {
              tunnel: w496 -> [w498 w503]
              tunnel: [w498 w499] -> w495
              tunnel: w492 -> [_ w505]
              frame False {
              }
              frame True {
                n237 = Bundle By Name(cluster=cluster{"graph":i32, "row":i32} {"graph"=0, "row"=0}, "graph"=0, "row"=w505) -> (w504:cluster{"graph":i32, "row":i32})
                n238 = Flatten To JSON(anything=w504, error in (no error)=w503) -> (JSON string=w502:string, 11:w500:errorcluster)  [unwired: 1 in]
                n239 = call-poly "Send Message.vi"("error in (no error)"=w500, "event buffer"=w502, "event"="multipleGraphs") -> ("error out"=w499:errorcluster)  [unwired: 8 in]
              }
            }
          }
          event "Custom Chart 2 Selection": Mouse Down {
            n240 = event-data() -> ("CtlRef"=w511:refnum<vi>, "Coords"=w510:T45)  [unwired: 1 in, 6 out]
            n241 = invoke on="Invoke Node" class="LstBox (strict)" method="Point To Row"(reference=w511, "Point"=w510) -> ("InBounds"=w508:bool, "Row"=w509:i32)  [unwired: 5 in, 5 out]
            n242 = case shown="True" w508 {
              tunnel: w513 -> [w515 w520]
              tunnel: [w515 w516] -> w512
              tunnel: w509 -> [_ w522]
              frame False {
              }
              frame True {
                n243 = Bundle By Name(cluster=cluster{"graph":i32, "row":i32} {"graph"=0, "row"=0}, "graph"=1, "row"=w522) -> (w521:cluster{"graph":i32, "row":i32})
                n244 = Flatten To JSON(anything=w521, error in (no error)=w520) -> (JSON string=w519:string, 11:w517:errorcluster)  [unwired: 1 in]
                n245 = call-poly "Send Message.vi"("error in (no error)"=w517, "event buffer"=w519, "event"="multipleGraphs") -> ("error out"=w516:errorcluster)  [unwired: 8 in]
              }
            }
          }
          event "Custom Chart 3 Selection": Mouse Down {
            n246 = event-data() -> ("CtlRef"=w528:refnum<vi>, "Coords"=w527:T45)  [unwired: 1 in, 6 out]
            n247 = invoke on="Invoke Node" class="LstBox (strict)" method="Point To Row"(reference=w528, "Point"=w527) -> ("InBounds"=w525:bool, "Row"=w526:i32)  [unwired: 5 in, 5 out]
            n248 = case shown="True" w525 {
              tunnel: w530 -> [w532 w537]
              tunnel: [w532 w533] -> w529
              tunnel: w526 -> [_ w539]
              frame False {
              }
              frame True {
                n249 = Bundle By Name(cluster=cluster{"graph":i32, "row":i32} {"graph"=0, "row"=0}, "graph"=2, "row"=w539) -> (w538:cluster{"graph":i32, "row":i32})
                n250 = Flatten To JSON(anything=w538, error in (no error)=w537) -> (JSON string=w536:string, 11:w534:errorcluster)  [unwired: 1 in]
                n251 = call-poly "Send Message.vi"("error in (no error)"=w534, "event buffer"=w536, "event"="multipleGraphs") -> ("error out"=w533:errorcluster)  [unwired: 8 in]
              }
            }
          }
          event "Custom Chart 4 Selection": Mouse Down {
            n252 = event-data() -> ("CtlRef"=w545:refnum<vi>, "Coords"=w544:T45)  [unwired: 1 in, 6 out]
            n253 = invoke on="Invoke Node" class="LstBox (strict)" method="Point To Row"(reference=w545, "Point"=w544) -> ("InBounds"=w542:bool, "Row"=w543:i32)  [unwired: 5 in, 5 out]
            n254 = case shown="True" w542 {
              tunnel: w547 -> [w549 w554]
              tunnel: [w549 w550] -> w546
              tunnel: w543 -> [_ w556]
              frame False {
              }
              frame True {
                n255 = Bundle By Name(cluster=cluster{"graph":i32, "row":i32} {"graph"=0, "row"=0}, "graph"=3, "row"=w556) -> (w555:cluster{"graph":i32, "row":i32})
                n256 = Flatten To JSON(anything=w555, error in (no error)=w554) -> (JSON string=w553:string, 11:w551:errorcluster)  [unwired: 1 in]
                n257 = call-poly "Send Message.vi"("error in (no error)"=w551, "event buffer"=w553, "event"="multipleGraphs") -> ("error out"=w550:errorcluster)  [unwired: 8 in]
              }
            }
          }
          event "Custom Chart 5 Selection": Mouse Down {
            n258 = event-data() -> ("CtlRef"=w562:refnum<vi>, "Coords"=w561:T45)  [unwired: 1 in, 6 out]
            n259 = invoke on="Invoke Node" class="LstBox (strict)" method="Point To Row"(reference=w562, "Point"=w561) -> ("InBounds"=w559:bool, "Row"=w560:i32)  [unwired: 5 in, 5 out]
            n260 = case shown="True" w559 {
              tunnel: w564 -> [w566 w571]
              tunnel: [w566 w567] -> w563
              tunnel: w560 -> [_ w573]
              frame False {
              }
              frame True {
                n261 = Bundle By Name(cluster=cluster{"graph":i32, "row":i32} {"graph"=0, "row"=0}, "graph"=4, "row"=w573) -> (w572:cluster{"graph":i32, "row":i32})
                n262 = Flatten To JSON(anything=w572, error in (no error)=w571) -> (JSON string=w570:string, 11:w568:errorcluster)  [unwired: 1 in]
                n263 = call-poly "Send Message.vi"("error in (no error)"=w568, "event buffer"=w570, "event"="multipleGraphs") -> ("error out"=w567:errorcluster)  [unwired: 8 in]
              }
            }
          }
          event "Custom Chart 6 Selection": Mouse Down {
            n264 = event-data() -> ("CtlRef"=w579:refnum<vi>, "Coords"=w578:T45)  [unwired: 1 in, 6 out]
            n265 = invoke on="Invoke Node" class="LstBox (strict)" method="Point To Row"(reference=w579, "Point"=w578) -> ("InBounds"=w576:bool, "Row"=w577:i32)  [unwired: 5 in, 5 out]
            n266 = case shown="True" w576 {
              tunnel: w581 -> [w583 w588]
              tunnel: [w583 w584] -> w580
              tunnel: w577 -> [_ w590]
              frame False {
              }
              frame True {
                n267 = Bundle By Name(cluster=cluster{"graph":i32, "row":i32} {"graph"=0, "row"=0}, "graph"=5, "row"=w590) -> (w589:cluster{"graph":i32, "row":i32})
                n268 = Flatten To JSON(anything=w589, error in (no error)=w588) -> (JSON string=w587:string, 11:w585:errorcluster)  [unwired: 1 in]
                n269 = call-poly "Send Message.vi"("error in (no error)"=w585, "event buffer"=w587, "event"="multipleGraphs") -> ("error out"=w584:errorcluster)  [unwired: 8 in]
              }
            }
          }
          event "Tab Control": Value Change {
            n270 = event-data() -> ("NewVal"=w598:T2)  [unwired: 1 in, 5 out]
            n271 = Equal?(x=w598, y=T2."Graphs") -> (x = y?=w601:bool)
            n272 = case shown="True" w601 {
              tunnel: w600 -> [w613 w615]
              tunnel: [w613 w614] -> w597
              frame False {
              }
              frame True {
                n273 = call-poly "Send Message.vi"("error in (no error)"=w615, "event"="getGraphs") -> ("error out"=w614:errorcluster)  [unwired: 9 in]
              }
            }
            n274 = Equal?(x=w598, y=T2."Advanced / Debug Mode") -> (x = y?=w599:bool)
            n275 = case shown="True" w599 {
              tunnel: w597 -> [w602 w605]
              tunnel: [w602 w603] -> w596
              frame False {
              }
              frame True {
                n276 = call "engineering_prompt.vi"("error in (no error)"=w605) -> ("Password"=w606:string, "error out"=w604:errorcluster)  [unwired: 16 in, 1 out]
                n277 = Equal?(x=w606, y="admin") -> (x = y?=w608:bool)
                n278 = case shown="False" w608 {
                  tunnel: w604 -> [w610 w612]
                  tunnel: [w610 w612] -> w603
                  frame False {
                    n279 = One Button Dialog(message="Access Denied") -> ()  [unwired: 1 in, 1 out]
                    n280 = local write "Tab Control"(T2."General Status" ("Tab Control")) -> ()
                  }
                  frame True {
                  }
                }
              }
            }
          }
          event "Engineering Interfaces": Mouse Down {
            n281 = event-data() -> ()  [unwired: 1 in, 1 out]
            n282 = Unbundle By Name(w617) -> ("go"=w620:bool, "Http session"=w619:T30, "URL prefex"=w618:string)
            n283 = vi-ref "PC104_interface_GUI.vi"() -> (w636:refnum<vi>)
            n284 = vi-ref "SHI_Cryopump_interface_GUI.vi"() -> (w630:refnum<vi>)
            n285 = property class="VI Interface Type 0"(reference=w636, error in=w623) -> (reference out=w634:refnum<vi>, error out=w633:errorcluster, "Path"=w635:path)
            n286 = Open VI Reference(type specifier VI Refnum (for type only)=w634, vi path=w635, options=128, error in (no error)=w633) -> (vi reference=w632:refnum<vi>, error out=w631:errorcluster)  [unwired: 2 in]
            n287 = call-by-ref "Start Asynchronous Call"(reference=w632, error in=w631, 8:"error in (no error)"=w631, "URL prefex"=w618, "Http session"=w619, "go"=w620) -> (error out=w622:errorcluster)  [unwired: 6 in, 3 out]
            n288 = property class="VI Interface Type 1"(reference=w630, error in=w622) -> (reference out=w628:refnum<vi>, error out=w627:errorcluster, "Path"=w624:path)
            n289 = Open VI Reference(type specifier VI Refnum (for type only)=w628, vi path=w624, options=128, error in (no error)=w627) -> (vi reference=w625:refnum<vi>, error out=w626:errorcluster)  [unwired: 2 in]
            n290 = call-by-ref "Start Asynchronous Call"(reference=w625, error in=w626, 8:"error in (no error)"=w626, "URL prefex"=w618, "Http session"=w619, "go"=w620) -> (error out=w621:errorcluster)  [unwired: 8 in, 1 out]
          }
          event "Thermocouples": Mouse Down {
            n291 = event-data() -> ("CtlRef"=w648:refnum<vi>, "Coords"=w653:T45)  [unwired: 1 in, 3 out]
            n292 = Unbundle By Name(w653) -> ("Horizontal"=w651:i32, "Vertical"=w650:i32)
            n293 = Add(x=783 ("y"), y=w643) -> (x+y=w638:i32)
            n294 = Less?(x=w651, y=w638) -> (x < y?=w652:bool)
            n295 = Add(x=w640, y=854) -> (x+y=w639:i32)
            n296 = Less?(x=w650, y=w639) -> (x < y?=w649:bool)
            n297 = And(x=w652, y=w649) -> (x .and. y?=w647:bool)
            n298 = case shown="True" w647 {
              tunnel: w648 -> [_ w695]
              tunnel: w646 -> [_ w667]
              tunnel: w646 -> [w654 w665]
              tunnel: [w654 w657] -> w645
              tunnel: w643 -> [_ w656]
              tunnel: w640 -> [_ w655]
              frame False {
              }
              frame True {
                w689 = u16 0 items=["User Selection", "Graph All Thermocouples", "Clear Graph"] ("Graphing Selection")
                n299 = property class="Arr (strict)"(reference=w695) -> ("Array Element.Position"=w687:T25)  [unwired: 1 in, 2 out]
                n300 = local write "Graphing Selection"(w689) -> ()
                n301 = Unbundle By Name(w687) -> ("Left"=w685:i32, "Top"=w688:i32)
                n302 = property on="Thermocouples" class="Arr (strict)"() -> ("Index Values"=w679:u32[])  [unwired: 2 in, 2 out]
                n303 = Subtract(x=w656, y=w685) -> (x-y=w684:i32)
                n304 = Subtract(x=w655, y=w688) -> (x-y=w676:i32)
                n305 = Absolute Value(x=w676) -> (abs(x)=w686:i32)
                n306 = Index Array(array=w679, index=0) -> (element=w675:u32)
                n307 = To Byte Integer(number=w675) -> (8bit integer=w674:i8)
                n308 = Absolute Value(x=w684) -> (abs(x)=w683:i32)
                n309 = local read "Thermocouples"() -> (w658:T3)
                n310 = Quotient & Remainder(x=w686, y=42) -> (floor(x/y)=w673:i32)  [unwired: 1 out]
                n311 = Add(x=w674, y=w673) -> (x+y=w660:i32)
                n312 = Quotient & Remainder(x=w683, y=197 ("Numeric 2")) -> (floor(x/y)=w659:i32)  [unwired: 1 out]
                n313 = Index Array(array=w658, index (row)=w660, index (col)=w659) -> (element=w661:T32)
                n314 = Multiply(x=4, y=w660) -> (x*y=w680:i32)
                n315 = Unbundle By Name(w667) -> ("working array"=w666:bool[])  [unwired: 1 out]
                n316 = Unbundle By Name(w661) -> ("Alarm Color"=w693:u32, "Graph On/Off"=w692:u32, "TC Label"=w691:string, "PlotColor"=w672:u32, "Alarm Status"=w690:string, "Temperature"=w663:string)
                n317 = Add(x=w680, y=w659) -> (x+y=w669:i32)
                n318 = control-ref of="Waveform Chart"() -> (w694:refnum<vi>)
                n319 = Index Array(array=w666, index=w669) -> (element=w668:bool)
                n320 = Decimal String To Number(string=w663) -> ()  [unwired: 2 in, 2 out]
                n321 = Equal?(x=w692, y=u32 12369084) -> (x = y?=w670:bool)
                n322 = case shown="True" w668 {
                  selector: w668 -> [_ w701]
                  tunnel: w694 -> [_ w707]
                  tunnel: w693 -> [_ w706]
                  tunnel: w691 -> [_ w705]
                  tunnel: w690 -> [_ w704]
                  tunnel: w669 -> [_ w697]
                  tunnel: w672 -> [_ w703]
                  tunnel: w670 -> [_ w702]
                  tunnel: w663 -> [_ w700]
                  tunnel: [w696 w699] -> w662
                  tunnel: w661 -> [w696 w698]
                  frame False {
                  }
                  frame True {
                    n323 = case shown="True" w702 {
                      tunnel: w707 -> [w717 w728]
                      tunnel: w706 -> [w711 w723]
                      tunnel: w705 -> [w712 w722]
                      tunnel: w704 -> [w713 w724]
                      tunnel: w703 -> [_ w726]
                      tunnel: w701 -> [_ _]
                      tunnel: w700 -> [w714 w725]
                      tunnel: [w709 w721] -> w699
                      tunnel: w698 -> [w710 w720]
                      tunnel: w697 -> [w708 w719]
                      frame False {
                        w715 = u32 12369084
                        n324 = property on="Property Node" class="WFChart (strict)"(reference=w717, "Active Plot"=w708) -> (reference out=w718:refnum<vi>)  [unwired: 1 in, 1 out]
                        n325 = Bundle By Name(cluster=w710, "Graph On/Off"=w715, "TC Label"=w712, "PlotColor"=w715, "Temperature"=w714, "Alarm Color"=w711, "Alarm Status"=w713) -> (w709:T32)
                        n326 = property class="WFChart (strict)"(reference=w718, "Plot.Visible?"=FALSE ("Plot.Visible")) -> ()  [unwired: 1 in, 2 out]
                      }
                      frame True {
                        n327 = property class="WFChart (strict)"(reference=w728, "Active Plot"=w719) -> (reference out=w729:refnum<vi>)  [unwired: 1 in, 1 out]
                        n328 = Bundle By Name(cluster=w720, "Graph On/Off"=u32 6618880, "TC Label"=w722, "PlotColor"=w726, "Temperature"=w725, "Alarm Color"=w723, "Alarm Status"=w724) -> (w721:T32)
                        n329 = property class="WFChart (strict)"(reference=w729, "Plot.Visible?"=TRUE ("Plot.Visible")) -> ()  [unwired: 1 in, 2 out]
                      }
                    }
                  }
                }
                n330 = Replace Array Subset(array=w658, new element=w662, index (row)=w660, index (col)=w659) -> (w664:T3)
                n331 = Bundle By Name(cluster=w665, "Thermocouples"=w664) -> (w657:T31)
              }
            }
          }
          event "Graphing Selection": Value Change {
            n332 = event-data() -> ("NewVal"=w738:u16)  [unwired: 1 in, 5 out]
            n333 = Unbundle By Name(w733) -> ("Thermocouples"=w732:T3, "working array"=w735:bool[])
            n334 = control-ref of="Waveform Chart"() -> (w739:refnum<vi>)
            n335 = case shown="2" w738 {
              tunnel: w732 -> [w740 w745 w776]
              tunnel: w739 -> [_ w744 w775]
              tunnel: 120 ("disabled index (col)") -> [_ w743 w774]
              tunnel: w733 -> [_ _ _]
              tunnel: w735 -> [_ w742 _]
              tunnel: [w740 w741 w773] -> w734
              frame 0, Default {
              }
              frame 1 {
                n336 = for {
                  N: w743 -> [_]
                  tunnel: w744 -> [w751]
                  shift-right: [w746] -> w741
                  shift-left: w745 -> [w750]
                  tunnel: w742 -> [w747]
                  i -> [w749]
                  n337 = Index Array(array=w747, index=w749) -> (element=w748:bool)
                  n338 = case shown="True" w748 {
                    tunnel: w751 -> [_ w772]
                    tunnel: w750 -> [w752 w753]
                    tunnel: [w752 w754] -> w746
                    tunnel: w749 -> [_ w771]
                    frame False {
                    }
                    frame True {
                      n339 = Quotient & Remainder(x=w771, y=4) -> (x-y*floor(x/y)=w757:i32, floor(x/y)=w756:i32)
                      n340 = Multiply(x=4, y=w756) -> (x*y=w767:i32)
                      n341 = Add(x=w767, y=w757) -> (x+y=w766:i32)
                      n342 = property class="WFChart (strict)"(reference=w772, "Active Plot"=w766) -> (reference out=w769:refnum<vi>)  [unwired: 1 in, 1 out]
                      n343 = Index Array(array=w753, index (row)=w756, index (col)=w757) -> (element=w755:T32)
                      n344 = Unbundle By Name(w755) -> ("TC Label"=w758:string, "Alarm Status"=w764:string, "Temperature"=w763:string, "PlotColor"=w760:u32, "Alarm Color"=w759:u32)
                      n345 = property class="WFChart (strict)"(reference=w769, "Plot.Visible?"=TRUE ("Plot.Visible")) -> ()  [unwired: 1 in, 2 out]
                      n346 = Bundle By Name(cluster=w755, "TC Label"=w758, "Alarm Status"=w764, "Alarm Color"=w759, "Temperature"=w763, "PlotColor"=w760, "Graph On/Off"=u32 6618880) -> (w762:T32)
                      n347 = Replace Array Subset(array=w753, new element=w762, index (row)=w756, index (col)=w757) -> (w754:T3)
                    }
                  }
                }
              }
              frame 2 {
                n348 = for {
                  N: w774 -> [_]
                  tunnel: w775 -> [w794]
                  shift-right: [w777] -> w773
                  shift-left: w776 -> [w781]
                  i -> [w795]
                  w787 = u32 12369084
                  n349 = local read "working array"() -> (w796:bool[])
                  n350 = Quotient & Remainder(x=w795, y=4 ("Numeric")) -> (x-y*floor(x/y)=w779:i32, floor(x/y)=w778:i32)
                  n351 = Index Array(array=w781, index (row)=w778, index (col)=w779) -> (element=w786:T32)
                  n352 = Multiply(x=4, y=w778) -> (x*y=w790:i32)
                  n353 = Add(x=w790, y=w779) -> (x+y=w789:i32)
                  n354 = Index Array(array=w796, index=w795) -> ()  [unwired: 1 out]
                  n355 = property class="WFChart (strict)"(reference=w794, "Active Plot"=w789) -> (reference out=w792:refnum<vi>)  [unwired: 1 in, 1 out]
                  n356 = Unbundle By Name(w786) -> ("TC Label"=w785:string, "Alarm Status"=w784:string, "Temperature"=w783:string, "PlotColor"=w782:u32)
                  n357 = property class="WFChart (strict)"(reference=w792, "Plot.Visible?"=FALSE ("Plot.Visible")) -> ()  [unwired: 1 in, 2 out]
                  n358 = Bundle By Name(cluster=w786, "TC Label"=w785, "Alarm Status"=w784, "Alarm Color"=w787, "Temperature"=w783, "PlotColor"=w782, "Graph On/Off"=w787) -> (w780:T32)
                  n359 = Replace Array Subset(array=w781, new element=w780, index (row)=w778, index (col)=w779) -> (w777:T3)
                }
              }
            }
            n360 = Bundle By Name(cluster=w733, "Thermocouples"=w734) -> (w731:T31)
          }
          event "Set Time TC Graph": Mouse Down {
            n361 = event-data() -> ()  [unwired: 1 in, 8 out]
            n362 = local read "Log/Linear Y-Axis"() -> (w797:u16)
            n363 = control-ref of="Waveform Chart"() -> (w798:refnum<vi>)
            n364 = property on="Property Node" class="WFChart (strict)"(reference=w798, "YScale.Mapping Mode"=w797) -> ()  [unwired: 1 in, 2 out]
            n365 = case shown="0, Default" w797 {
              tunnel: w798 -> [w803 w805]
              frame 0, Default {
                n366 = property class="WFChart (strict)"(reference=w803, "YScale.LooseFit"=TRUE ("Y Scale.Flipped")) -> ()  [unwired: 1 in, 2 out]
              }
              frame 1 {
                n367 = property class="WFChart (strict)"(reference=w805, "YScale.LooseFit"=FALSE ("Y Scale.Flipped")) -> ()  [unwired: 1 in, 2 out]
              }
            }
            n368 = local read "Total Time"() -> (w799:dbl)
            n369 = local read "Time Scale"() -> (w800:u16)
            n370 = case shown="1" w800 {
              tunnel: w798 -> [w809 w828 w847]
              tunnel: w799 -> [w807 w826 w845]
              frame 0, Default {
                n371 = Not Equal To 0?(x=w807) -> (x != 0?=w808:bool)
                n372 = case shown="True" w808 {
                  tunnel: w809 -> [w811 w823]
                  tunnel: w807 -> [_ w817]
                  frame False {
                    n373 = property on="Property Node" class="WFChart (strict)"(reference=w811) -> (reference out=w810:refnum<vi>, "XScale.Range"=w816:T46)  [unwired: 1 in, 1 out]
                    n374 = Bundle By Name(cluster=w816, "Minimum"=0.0, "Maximum"=3600.0, "Increment"=60.0) -> (w815:T46)
                    n375 = property on="Property Node" class="WFChart (strict)"(reference=w810, "XScale.Range"=w815) -> ()  [unwired: 1 in, 2 out]
                  }
                  frame True {
                    n376 = property on="Property Node" class="WFChart (strict)"(reference=w823) -> (reference out=w820:refnum<vi>, "XScale.Range"=w825:T46)  [unwired: 1 in, 1 out]
                    n377 = Multiply(x=w817, y=60.0) -> (x*y=w819:dbl)
                    n378 = Bundle By Name(cluster=w825, "Minimum"=0.0, "Maximum"=w819, "Increment"=1.0) -> (w824:T46)
                    n379 = property on="Property Node" class="WFChart (strict)"(reference=w820, "XScale.Range"=w824) -> ()  [unwired: 1 in, 2 out]
                  }
                }
              }
              frame 1 {
                n380 = Not Equal To 0?(x=w826) -> (x != 0?=w827:bool)
                n381 = case shown="True" w827 {
                  tunnel: w828 -> [w830 w840]
                  tunnel: w826 -> [_ w837]
                  frame False {
                    n382 = property on="Property Node" class="WFChart (strict)"(reference=w830) -> (reference out=w829:refnum<vi>, "XScale.Range"=w835:T46)  [unwired: 1 in, 1 out]
                    n383 = Bundle By Name(cluster=w835, "Minimum"=0.0, "Maximum"=43200.0, "Increment"=3600.0) -> (w831:T46)
                    n384 = property on="Property Node" class="WFChart (strict)"(reference=w829, "XScale.Range"=w831) -> ()  [unwired: 1 in, 2 out]
                  }
                  frame True {
                    n385 = Multiply(x=w837, y=3600.0) -> (x*y=w836:dbl)
                    n386 = property on="Property Node" class="WFChart (strict)"(reference=w840) -> (reference out=w839:refnum<vi>, "XScale.Range"=w844:T46)  [unwired: 1 in, 1 out]
                    n387 = Bundle By Name(cluster=w844, "Minimum"=0.0, "Maximum"=w836, "Increment"=3600.0) -> (w841:T46)
                    n388 = property on="Property Node" class="WFChart (strict)"(reference=w839, "XScale.Range"=w841) -> ()  [unwired: 1 in, 2 out]
                  }
                }
              }
              frame 2 {
                n389 = Not Equal To 0?(x=w845) -> (x != 0?=w846:bool)
                n390 = case shown="True" w846 {
                  tunnel: w847 -> [w849 w857]
                  tunnel: w845 -> [_ w855]
                  frame False {
                    n391 = property on="Property Node" class="WFChart (strict)"(reference=w849) -> (reference out=w848:refnum<vi>, "XScale.Range"=w854:T46)  [unwired: 1 in, 1 out]
                    n392 = Bundle By Name(cluster=w854, "Minimum"=0.0, "Maximum"=60.0, "Increment"=1.0) -> (w850:T46)
                    n393 = property on="Property Node" class="WFChart (strict)"(reference=w848, "XScale.Range"=w850) -> ()  [unwired: 1 in, 2 out]
                  }
                  frame True {
                    n394 = property on="Property Node" class="WFChart (strict)"(reference=w857) -> (reference out=w856:refnum<vi>, "XScale.Range"=w861:T46)  [unwired: 1 in, 1 out]
                    n395 = Bundle By Name(cluster=w861, "Minimum"=0.0, "Maximum"=w855, "Increment"=1.0) -> (w858:T46)
                    n396 = property on="Property Node" class="WFChart (strict)"(reference=w856, "XScale.Range"=w858) -> ()  [unwired: 1 in, 2 out]
                  }
                }
              }
            }
          }
          event "Set Time TC Graph 1": Mouse Down {
            n397 = event-data() -> ()  [unwired: 1 in, 8 out]
            n398 = local read "Log/Linear Y-Axis 1"() -> (w862:u16)
            n399 = control-ref of="Custom Chart 1"() -> (w863:refnum<vi>)
            n400 = case shown="0, Default" w862 {
              tunnel: w863 -> [w868 w870]
              frame 0, Default {
                n401 = property class="WFChart (strict)"(reference=w868, "YScale.LooseFit"=TRUE ("Y Scale.Flipped")) -> ()  [unwired: 1 in, 2 out]
              }
              frame 1 {
                n402 = property class="WFChart (strict)"(reference=w870, "YScale.LooseFit"=FALSE ("Y Scale.Flipped")) -> ()  [unwired: 1 in, 2 out]
              }
            }
            n403 = property on="Property Node" class="WFChart (strict)"(reference=w863, "YScale.Mapping Mode"=w862) -> ()  [unwired: 1 in, 2 out]
            n404 = local read "Total Time 1"() -> (w864:dbl)
            n405 = local read "Time Scale 1"() -> (w865:u16)
            n406 = case shown="0, Default" w865 {
              tunnel: w863 -> [w874 w893 w912]
              tunnel: w864 -> [w872 w891 w910]
              frame 0, Default {
                n407 = Not Equal To 0?(x=w872) -> (x != 0?=w873:bool)
                n408 = case shown="True" w873 {
                  tunnel: w874 -> [w876 w888]
                  tunnel: w872 -> [_ w882]
                  frame False {
                    n409 = property on="Property Node" class="WFChart (strict)"(reference=w876) -> (reference out=w875:refnum<vi>, "XScale.Range"=w881:T46)  [unwired: 1 in, 1 out]
                    n410 = Bundle By Name(cluster=w881, "Minimum"=0.0, "Maximum"=3600.0, "Increment"=60.0) -> (w880:T46)
                    n411 = property on="Property Node" class="WFChart (strict)"(reference=w875, "XScale.Range"=w880) -> ()  [unwired: 1 in, 2 out]
                  }
                  frame True {
                    n412 = property on="Property Node" class="WFChart (strict)"(reference=w888) -> (reference out=w885:refnum<vi>, "XScale.Range"=w890:T46)  [unwired: 1 in, 1 out]
                    n413 = Multiply(x=w882, y=60.0) -> (x*y=w884:dbl)
                    n414 = Bundle By Name(cluster=w890, "Minimum"=0.0, "Maximum"=w884, "Increment"=1.0) -> (w889:T46)
                    n415 = property on="Property Node" class="WFChart (strict)"(reference=w885, "XScale.Range"=w889) -> ()  [unwired: 1 in, 2 out]
                  }
                }
              }
              frame 1 {
                n416 = Not Equal To 0?(x=w891) -> (x != 0?=w892:bool)
                n417 = case shown="True" w892 {
                  tunnel: w893 -> [w895 w905]
                  tunnel: w891 -> [_ w902]
                  frame False {
                    n418 = property on="Property Node" class="WFChart (strict)"(reference=w895) -> (reference out=w894:refnum<vi>, "XScale.Range"=w900:T46)  [unwired: 1 in, 1 out]
                    n419 = Bundle By Name(cluster=w900, "Minimum"=0.0, "Maximum"=43200.0, "Increment"=3600.0) -> (w896:T46)
                    n420 = property on="Property Node" class="WFChart (strict)"(reference=w894, "XScale.Range"=w896) -> ()  [unwired: 1 in, 2 out]
                  }
                  frame True {
                    n421 = Multiply(x=w902, y=3600.0) -> (x*y=w901:dbl)
                    n422 = property on="Property Node" class="WFChart (strict)"(reference=w905) -> (reference out=w904:refnum<vi>, "XScale.Range"=w909:T46)  [unwired: 1 in, 1 out]
                    n423 = Bundle By Name(cluster=w909, "Minimum"=0.0, "Maximum"=w901, "Increment"=3600.0) -> (w906:T46)
                    n424 = property on="Property Node" class="WFChart (strict)"(reference=w904, "XScale.Range"=w906) -> ()  [unwired: 1 in, 2 out]
                  }
                }
              }
              frame 2 {
                n425 = Not Equal To 0?(x=w910) -> (x != 0?=w911:bool)
                n426 = case shown="True" w911 {
                  tunnel: w912 -> [w914 w922]
                  tunnel: w910 -> [_ w920]
                  frame False {
                    n427 = property on="Property Node" class="WFChart (strict)"(reference=w914) -> (reference out=w913:refnum<vi>, "XScale.Range"=w919:T46)  [unwired: 1 in, 1 out]
                    n428 = Bundle By Name(cluster=w919, "Minimum"=0.0, "Maximum"=60.0, "Increment"=1.0) -> (w915:T46)
                    n429 = property on="Property Node" class="WFChart (strict)"(reference=w913, "XScale.Range"=w915) -> ()  [unwired: 1 in, 2 out]
                  }
                  frame True {
                    n430 = property on="Property Node" class="WFChart (strict)"(reference=w922) -> (reference out=w921:refnum<vi>, "XScale.Range"=w926:T46)  [unwired: 1 in, 1 out]
                    n431 = Bundle By Name(cluster=w926, "Minimum"=0.0, "Maximum"=w920, "Increment"=1.0) -> (w923:T46)
                    n432 = property on="Property Node" class="WFChart (strict)"(reference=w921, "XScale.Range"=w923) -> ()  [unwired: 1 in, 2 out]
                  }
                }
              }
            }
          }
          event "Set Time TC Graph 2": Mouse Down {
            n433 = event-data() -> ()  [unwired: 1 in, 8 out]
            n434 = local read "Log/Linear Y-Axis 2"() -> (w927:u16)
            n435 = control-ref of="Custom Chart 2"() -> (w928:refnum<vi>)
            n436 = property on="Property Node" class="WFChart (strict)"(reference=w928, "YScale.Mapping Mode"=w927) -> ()  [unwired: 1 in, 2 out]
            n437 = local read "Total Time 2"() -> (w929:dbl)
            n438 = case shown="0, Default" w927 {
              tunnel: w928 -> [w933 w935]
              frame 0, Default {
                n439 = property class="WFChart (strict)"(reference=w933, "YScale.LooseFit"=TRUE ("Y Scale.Flipped")) -> ()  [unwired: 1 in, 2 out]
              }
              frame 1 {
                n440 = property class="WFChart (strict)"(reference=w935, "YScale.LooseFit"=FALSE ("Y Scale.Flipped")) -> ()  [unwired: 1 in, 2 out]
              }
            }
            n441 = local read "Time Scale 2"() -> (w930:u16)
            n442 = case shown="2" w930 {
              tunnel: w928 -> [w939 w958 w977]
              tunnel: w929 -> [w937 w956 w975]
              frame 0, Default {
                n443 = Not Equal To 0?(x=w937) -> (x != 0?=w938:bool)
                n444 = case shown="True" w938 {
                  tunnel: w939 -> [w941 w953]
                  tunnel: w937 -> [_ w947]
                  frame False {
                    n445 = property on="Property Node" class="WFChart (strict)"(reference=w941) -> (reference out=w940:refnum<vi>, "XScale.Range"=w946:T46)  [unwired: 1 in, 1 out]
                    n446 = Bundle By Name(cluster=w946, "Minimum"=0.0, "Maximum"=3600.0, "Increment"=60.0) -> (w945:T46)
                    n447 = property on="Property Node" class="WFChart (strict)"(reference=w940, "XScale.Range"=w945) -> ()  [unwired: 1 in, 2 out]
                  }
                  frame True {
                    n448 = property on="Property Node" class="WFChart (strict)"(reference=w953) -> (reference out=w950:refnum<vi>, "XScale.Range"=w955:T46)  [unwired: 1 in, 1 out]
                    n449 = Multiply(x=w947, y=60.0) -> (x*y=w949:dbl)
                    n450 = Bundle By Name(cluster=w955, "Minimum"=0.0, "Maximum"=w949, "Increment"=1.0) -> (w954:T46)
                    n451 = property on="Property Node" class="WFChart (strict)"(reference=w950, "XScale.Range"=w954) -> ()  [unwired: 1 in, 2 out]
                  }
                }
              }
              frame 1 {
                n452 = Not Equal To 0?(x=w956) -> (x != 0?=w957:bool)
                n453 = case shown="True" w957 {
                  tunnel: w958 -> [w960 w970]
                  tunnel: w956 -> [_ w967]
                  frame False {
                    n454 = property on="Property Node" class="WFChart (strict)"(reference=w960) -> (reference out=w959:refnum<vi>, "XScale.Range"=w965:T46)  [unwired: 1 in, 1 out]
                    n455 = Bundle By Name(cluster=w965, "Minimum"=0.0, "Maximum"=43200.0, "Increment"=3600.0) -> (w961:T46)
                    n456 = property on="Property Node" class="WFChart (strict)"(reference=w959, "XScale.Range"=w961) -> ()  [unwired: 1 in, 2 out]
                  }
                  frame True {
                    n457 = Multiply(x=w967, y=3600.0) -> (x*y=w966:dbl)
                    n458 = property on="Property Node" class="WFChart (strict)"(reference=w970) -> (reference out=w969:refnum<vi>, "XScale.Range"=w974:T46)  [unwired: 1 in, 1 out]
                    n459 = Bundle By Name(cluster=w974, "Minimum"=0.0, "Maximum"=w966, "Increment"=3600.0) -> (w971:T46)
                    n460 = property on="Property Node" class="WFChart (strict)"(reference=w969, "XScale.Range"=w971) -> ()  [unwired: 1 in, 2 out]
                  }
                }
              }
              frame 2 {
                n461 = Not Equal To 0?(x=w975) -> (x != 0?=w976:bool)
                n462 = case shown="True" w976 {
                  tunnel: w977 -> [w979 w987]
                  tunnel: w975 -> [_ w985]
                  frame False {
                    n463 = property on="Property Node" class="WFChart (strict)"(reference=w979) -> (reference out=w978:refnum<vi>, "XScale.Range"=w984:T46)  [unwired: 1 in, 1 out]
                    n464 = Bundle By Name(cluster=w984, "Minimum"=0.0, "Maximum"=60.0, "Increment"=1.0) -> (w980:T46)
                    n465 = property on="Property Node" class="WFChart (strict)"(reference=w978, "XScale.Range"=w980) -> ()  [unwired: 1 in, 2 out]
                  }
                  frame True {
                    n466 = property on="Property Node" class="WFChart (strict)"(reference=w987) -> (reference out=w986:refnum<vi>, "XScale.Range"=w991:T46)  [unwired: 1 in, 1 out]
                    n467 = Bundle By Name(cluster=w991, "Minimum"=0.0, "Maximum"=w985, "Increment"=1.0) -> (w988:T46)
                    n468 = property on="Property Node" class="WFChart (strict)"(reference=w986, "XScale.Range"=w988) -> ()  [unwired: 1 in, 2 out]
                  }
                }
              }
            }
          }
          event "Set Time TC Graph 3": Mouse Down {
            n469 = event-data() -> ()  [unwired: 1 in, 8 out]
            n470 = local read "Log/Linear Y-Axis 3"() -> (w992:u16)
            n471 = control-ref of="Custom Chart 3"() -> (w993:refnum<vi>)
            n472 = property on="Property Node" class="WFChart (strict)"(reference=w993, "YScale.Mapping Mode"=w992) -> ()  [unwired: 1 in, 2 out]
            n473 = local read "Total Time 3"() -> (w994:dbl)
            n474 = case shown="0, Default" w992 {
              tunnel: w993 -> [w998 w1000]
              frame 0, Default {
                n475 = property class="WFChart (strict)"(reference=w998, "YScale.LooseFit"=TRUE ("Y Scale.Flipped")) -> ()  [unwired: 1 in, 2 out]
              }
              frame 1 {
                n476 = property class="WFChart (strict)"(reference=w1000, "YScale.LooseFit"=FALSE ("Y Scale.Flipped")) -> ()  [unwired: 1 in, 2 out]
              }
            }
            n477 = local read "Time Scale 3"() -> (w995:u16)
            n478 = case shown="2" w995 {
              tunnel: w993 -> [w1004 w1023 w1042]
              tunnel: w994 -> [w1002 w1021 w1040]
              frame 0, Default {
                n479 = Not Equal To 0?(x=w1002) -> (x != 0?=w1003:bool)
                n480 = case shown="True" w1003 {
                  tunnel: w1004 -> [w1006 w1018]
                  tunnel: w1002 -> [_ w1012]
                  frame False {
                    n481 = property on="Property Node" class="WFChart (strict)"(reference=w1006) -> (reference out=w1005:refnum<vi>, "XScale.Range"=w1011:T46)  [unwired: 1 in, 1 out]
                    n482 = Bundle By Name(cluster=w1011, "Minimum"=0.0, "Maximum"=3600.0, "Increment"=60.0) -> (w1010:T46)
                    n483 = property on="Property Node" class="WFChart (strict)"(reference=w1005, "XScale.Range"=w1010) -> ()  [unwired: 1 in, 2 out]
                  }
                  frame True {
                    n484 = property on="Property Node" class="WFChart (strict)"(reference=w1018) -> (reference out=w1015:refnum<vi>, "XScale.Range"=w1020:T46)  [unwired: 1 in, 1 out]
                    n485 = Multiply(x=w1012, y=60.0) -> (x*y=w1014:dbl)
                    n486 = Bundle By Name(cluster=w1020, "Minimum"=0.0, "Maximum"=w1014, "Increment"=1.0) -> (w1019:T46)
                    n487 = property on="Property Node" class="WFChart (strict)"(reference=w1015, "XScale.Range"=w1019) -> ()  [unwired: 1 in, 2 out]
                  }
                }
              }
              frame 1 {
                n488 = Not Equal To 0?(x=w1021) -> (x != 0?=w1022:bool)
                n489 = case shown="True" w1022 {
                  tunnel: w1023 -> [w1025 w1035]
                  tunnel: w1021 -> [_ w1032]
                  frame False {
                    n490 = property on="Property Node" class="WFChart (strict)"(reference=w1025) -> (reference out=w1024:refnum<vi>, "XScale.Range"=w1030:T46)  [unwired: 1 in, 1 out]
                    n491 = Bundle By Name(cluster=w1030, "Minimum"=0.0, "Maximum"=43200.0, "Increment"=3600.0) -> (w1026:T46)
                    n492 = property on="Property Node" class="WFChart (strict)"(reference=w1024, "XScale.Range"=w1026) -> ()  [unwired: 1 in, 2 out]
                  }
                  frame True {
                    n493 = Multiply(x=w1032, y=3600.0) -> (x*y=w1031:dbl)
                    n494 = property on="Property Node" class="WFChart (strict)"(reference=w1035) -> (reference out=w1034:refnum<vi>, "XScale.Range"=w1039:T46)  [unwired: 1 in, 1 out]
                    n495 = Bundle By Name(cluster=w1039, "Minimum"=0.0, "Maximum"=w1031, "Increment"=3600.0) -> (w1036:T46)
                    n496 = property on="Property Node" class="WFChart (strict)"(reference=w1034, "XScale.Range"=w1036) -> ()  [unwired: 1 in, 2 out]
                  }
                }
              }
              frame 2 {
                n497 = Not Equal To 0?(x=w1040) -> (x != 0?=w1041:bool)
                n498 = case shown="True" w1041 {
                  tunnel: w1042 -> [w1044 w1052]
                  tunnel: w1040 -> [_ w1050]
                  frame False {
                    n499 = property on="Property Node" class="WFChart (strict)"(reference=w1044) -> (reference out=w1043:refnum<vi>, "XScale.Range"=w1049:T46)  [unwired: 1 in, 1 out]
                    n500 = Bundle By Name(cluster=w1049, "Minimum"=0.0, "Maximum"=60.0, "Increment"=1.0) -> (w1045:T46)
                    n501 = property on="Property Node" class="WFChart (strict)"(reference=w1043, "XScale.Range"=w1045) -> ()  [unwired: 1 in, 2 out]
                  }
                  frame True {
                    n502 = property on="Property Node" class="WFChart (strict)"(reference=w1052) -> (reference out=w1051:refnum<vi>, "XScale.Range"=w1056:T46)  [unwired: 1 in, 1 out]
                    n503 = Bundle By Name(cluster=w1056, "Minimum"=0.0, "Maximum"=w1050, "Increment"=1.0) -> (w1053:T46)
                    n504 = property on="Property Node" class="WFChart (strict)"(reference=w1051, "XScale.Range"=w1053) -> ()  [unwired: 1 in, 2 out]
                  }
                }
              }
            }
          }
          event "Set Time TC Graph 4": Mouse Down {
            n505 = event-data() -> ()  [unwired: 1 in, 8 out]
            n506 = local read "Log/Linear Y-Axis 4"() -> (w1057:u16)
            n507 = control-ref of="Custom Chart 4"() -> (w1058:refnum<vi>)
            n508 = property on="Property Node" class="WFChart (strict)"(reference=w1058, "YScale.Mapping Mode"=w1057) -> ()  [unwired: 1 in, 2 out]
            n509 = local read "Total Time 4"() -> (w1059:dbl)
            n510 = case shown="0, Default" w1057 {
              tunnel: w1058 -> [w1063 w1065]
              frame 0, Default {
                n511 = property class="WFChart (strict)"(reference=w1063, "YScale.LooseFit"=TRUE ("Y Scale.Flipped")) -> ()  [unwired: 1 in, 2 out]
              }
              frame 1 {
                n512 = property class="WFChart (strict)"(reference=w1065, "YScale.LooseFit"=FALSE ("Y Scale.Flipped")) -> ()  [unwired: 1 in, 2 out]
              }
            }
            n513 = local read "Time Scale 4"() -> (w1060:u16)
            n514 = case shown="2" w1060 {
              tunnel: w1058 -> [w1069 w1088 w1107]
              tunnel: w1059 -> [w1067 w1086 w1105]
              frame 0, Default {
                n515 = Not Equal To 0?(x=w1067) -> (x != 0?=w1068:bool)
                n516 = case shown="True" w1068 {
                  tunnel: w1069 -> [w1071 w1083]
                  tunnel: w1067 -> [_ w1077]
                  frame False {
                    n517 = property on="Property Node" class="WFChart (strict)"(reference=w1071) -> (reference out=w1070:refnum<vi>, "XScale.Range"=w1076:T46)  [unwired: 1 in, 1 out]
                    n518 = Bundle By Name(cluster=w1076, "Minimum"=0.0, "Maximum"=3600.0, "Increment"=60.0) -> (w1075:T46)
                    n519 = property on="Property Node" class="WFChart (strict)"(reference=w1070, "XScale.Range"=w1075) -> ()  [unwired: 1 in, 2 out]
                  }
                  frame True {
                    n520 = property on="Property Node" class="WFChart (strict)"(reference=w1083) -> (reference out=w1080:refnum<vi>, "XScale.Range"=w1085:T46)  [unwired: 1 in, 1 out]
                    n521 = Multiply(x=w1077, y=60.0) -> (x*y=w1079:dbl)
                    n522 = Bundle By Name(cluster=w1085, "Minimum"=0.0, "Maximum"=w1079, "Increment"=1.0) -> (w1084:T46)
                    n523 = property on="Property Node" class="WFChart (strict)"(reference=w1080, "XScale.Range"=w1084) -> ()  [unwired: 1 in, 2 out]
                  }
                }
              }
              frame 1 {
                n524 = Not Equal To 0?(x=w1086) -> (x != 0?=w1087:bool)
                n525 = case shown="True" w1087 {
                  tunnel: w1088 -> [w1090 w1100]
                  tunnel: w1086 -> [_ w1097]
                  frame False {
                    n526 = property on="Property Node" class="WFChart (strict)"(reference=w1090) -> (reference out=w1089:refnum<vi>, "XScale.Range"=w1095:T46)  [unwired: 1 in, 1 out]
                    n527 = Bundle By Name(cluster=w1095, "Minimum"=0.0, "Maximum"=43200.0, "Increment"=3600.0) -> (w1091:T46)
                    n528 = property on="Property Node" class="WFChart (strict)"(reference=w1089, "XScale.Range"=w1091) -> ()  [unwired: 1 in, 2 out]
                  }
                  frame True {
                    n529 = Multiply(x=w1097, y=3600.0) -> (x*y=w1096:dbl)
                    n530 = property on="Property Node" class="WFChart (strict)"(reference=w1100) -> (reference out=w1099:refnum<vi>, "XScale.Range"=w1104:T46)  [unwired: 1 in, 1 out]
                    n531 = Bundle By Name(cluster=w1104, "Minimum"=0.0, "Maximum"=w1096, "Increment"=3600.0) -> (w1101:T46)
                    n532 = property on="Property Node" class="WFChart (strict)"(reference=w1099, "XScale.Range"=w1101) -> ()  [unwired: 1 in, 2 out]
                  }
                }
              }
              frame 2 {
                n533 = Not Equal To 0?(x=w1105) -> (x != 0?=w1106:bool)
                n534 = case shown="True" w1106 {
                  tunnel: w1107 -> [w1109 w1117]
                  tunnel: w1105 -> [_ w1115]
                  frame False {
                    n535 = property on="Property Node" class="WFChart (strict)"(reference=w1109) -> (reference out=w1108:refnum<vi>, "XScale.Range"=w1114:T46)  [unwired: 1 in, 1 out]
                    n536 = Bundle By Name(cluster=w1114, "Minimum"=0.0, "Maximum"=60.0, "Increment"=1.0) -> (w1110:T46)
                    n537 = property on="Property Node" class="WFChart (strict)"(reference=w1108, "XScale.Range"=w1110) -> ()  [unwired: 1 in, 2 out]
                  }
                  frame True {
                    n538 = property on="Property Node" class="WFChart (strict)"(reference=w1117) -> (reference out=w1116:refnum<vi>, "XScale.Range"=w1121:T46)  [unwired: 1 in, 1 out]
                    n539 = Bundle By Name(cluster=w1121, "Minimum"=0.0, "Maximum"=w1115, "Increment"=1.0) -> (w1118:T46)
                    n540 = property on="Property Node" class="WFChart (strict)"(reference=w1116, "XScale.Range"=w1118) -> ()  [unwired: 1 in, 2 out]
                  }
                }
              }
            }
          }
          event "Set Time TC Graph 5": Mouse Down {
            n541 = event-data() -> ()  [unwired: 1 in, 8 out]
            n542 = local read "Log/Linear Y-Axis 5"() -> (w1122:u16)
            n543 = control-ref of="Custom Chart 5"() -> (w1123:refnum<vi>)
            n544 = property on="Property Node" class="WFChart (strict)"(reference=w1123, "YScale.Mapping Mode"=w1122) -> ()  [unwired: 1 in, 2 out]
            n545 = case shown="0, Default" w1122 {
              tunnel: w1123 -> [w1128 w1130]
              frame 0, Default {
                n546 = property class="WFChart (strict)"(reference=w1128, "YScale.LooseFit"=TRUE ("Y Scale.Flipped")) -> ()  [unwired: 1 in, 2 out]
              }
              frame 1 {
                n547 = property class="WFChart (strict)"(reference=w1130, "YScale.LooseFit"=FALSE ("Y Scale.Flipped")) -> ()  [unwired: 1 in, 2 out]
              }
            }
            n548 = local read "Total Time 5"() -> (w1124:dbl)
            n549 = local read "Time Scale 5"() -> (w1125:u16)
            n550 = case shown="2" w1125 {
              tunnel: w1123 -> [w1134 w1153 w1172]
              tunnel: w1124 -> [w1132 w1151 w1170]
              frame 0, Default {
                n551 = Not Equal To 0?(x=w1132) -> (x != 0?=w1133:bool)
                n552 = case shown="True" w1133 {
                  tunnel: w1134 -> [w1136 w1148]
                  tunnel: w1132 -> [_ w1142]
                  frame False {
                    n553 = property on="Property Node" class="WFChart (strict)"(reference=w1136) -> (reference out=w1135:refnum<vi>, "XScale.Range"=w1141:T46)  [unwired: 1 in, 1 out]
                    n554 = Bundle By Name(cluster=w1141, "Minimum"=0.0, "Maximum"=3600.0, "Increment"=60.0) -> (w1140:T46)
                    n555 = property on="Property Node" class="WFChart (strict)"(reference=w1135, "XScale.Range"=w1140) -> ()  [unwired: 1 in, 2 out]
                  }
                  frame True {
                    n556 = property on="Property Node" class="WFChart (strict)"(reference=w1148) -> (reference out=w1145:refnum<vi>, "XScale.Range"=w1150:T46)  [unwired: 1 in, 1 out]
                    n557 = Multiply(x=w1142, y=60.0) -> (x*y=w1144:dbl)
                    n558 = Bundle By Name(cluster=w1150, "Minimum"=0.0, "Maximum"=w1144, "Increment"=1.0) -> (w1149:T46)
                    n559 = property on="Property Node" class="WFChart (strict)"(reference=w1145, "XScale.Range"=w1149) -> ()  [unwired: 1 in, 2 out]
                  }
                }
              }
              frame 1 {
                n560 = Not Equal To 0?(x=w1151) -> (x != 0?=w1152:bool)
                n561 = case shown="True" w1152 {
                  tunnel: w1153 -> [w1155 w1165]
                  tunnel: w1151 -> [_ w1162]
                  frame False {
                    n562 = property on="Property Node" class="WFChart (strict)"(reference=w1155) -> (reference out=w1154:refnum<vi>, "XScale.Range"=w1160:T46)  [unwired: 1 in, 1 out]
                    n563 = Bundle By Name(cluster=w1160, "Minimum"=0.0, "Maximum"=43200.0, "Increment"=3600.0) -> (w1156:T46)
                    n564 = property on="Property Node" class="WFChart (strict)"(reference=w1154, "XScale.Range"=w1156) -> ()  [unwired: 1 in, 2 out]
                  }
                  frame True {
                    n565 = Multiply(x=w1162, y=3600.0) -> (x*y=w1161:dbl)
                    n566 = property on="Property Node" class="WFChart (strict)"(reference=w1165) -> (reference out=w1164:refnum<vi>, "XScale.Range"=w1169:T46)  [unwired: 1 in, 1 out]
                    n567 = Bundle By Name(cluster=w1169, "Minimum"=0.0, "Maximum"=w1161, "Increment"=3600.0) -> (w1166:T46)
                    n568 = property on="Property Node" class="WFChart (strict)"(reference=w1164, "XScale.Range"=w1166) -> ()  [unwired: 1 in, 2 out]
                  }
                }
              }
              frame 2 {
                n569 = Not Equal To 0?(x=w1170) -> (x != 0?=w1171:bool)
                n570 = case shown="True" w1171 {
                  tunnel: w1172 -> [w1174 w1182]
                  tunnel: w1170 -> [_ w1180]
                  frame False {
                    n571 = property on="Property Node" class="WFChart (strict)"(reference=w1174) -> (reference out=w1173:refnum<vi>, "XScale.Range"=w1179:T46)  [unwired: 1 in, 1 out]
                    n572 = Bundle By Name(cluster=w1179, "Minimum"=0.0, "Maximum"=60.0, "Increment"=1.0) -> (w1175:T46)
                    n573 = property on="Property Node" class="WFChart (strict)"(reference=w1173, "XScale.Range"=w1175) -> ()  [unwired: 1 in, 2 out]
                  }
                  frame True {
                    n574 = property on="Property Node" class="WFChart (strict)"(reference=w1182) -> (reference out=w1181:refnum<vi>, "XScale.Range"=w1186:T46)  [unwired: 1 in, 1 out]
                    n575 = Bundle By Name(cluster=w1186, "Minimum"=0.0, "Maximum"=w1180, "Increment"=1.0) -> (w1183:T46)
                    n576 = property on="Property Node" class="WFChart (strict)"(reference=w1181, "XScale.Range"=w1183) -> ()  [unwired: 1 in, 2 out]
                  }
                }
              }
            }
          }
          event "Set Time TC Graph 6": Mouse Down {
            n577 = event-data() -> ()  [unwired: 1 in, 8 out]
            n578 = local read "Log/Linear Y-Axis 6"() -> (w1187:u16)
            n579 = control-ref of="Custom Chart 6"() -> (w1188:refnum<vi>)
            n580 = property on="Property Node" class="WFChart (strict)"(reference=w1188, "YScale.Mapping Mode"=w1187) -> ()  [unwired: 1 in, 2 out]
            n581 = local read "Total Time 6"() -> (w1189:dbl)
            n582 = case shown="0, Default" w1187 {
              tunnel: w1188 -> [w1193 w1195]
              frame 0, Default {
                n583 = property class="WFChart (strict)"(reference=w1193, "YScale.LooseFit"=TRUE ("Y Scale.Flipped")) -> ()  [unwired: 1 in, 2 out]
              }
              frame 1 {
                n584 = property class="WFChart (strict)"(reference=w1195, "YScale.LooseFit"=FALSE ("Y Scale.Flipped")) -> ()  [unwired: 1 in, 2 out]
              }
            }
            n585 = local read "Time Scale 6"() -> (w1190:u16)
            n586 = case shown="2" w1190 {
              tunnel: w1188 -> [w1199 w1218 w1237]
              tunnel: w1189 -> [w1197 w1216 w1235]
              frame 0, Default {
                n587 = Not Equal To 0?(x=w1197) -> (x != 0?=w1198:bool)
                n588 = case shown="True" w1198 {
                  tunnel: w1199 -> [w1201 w1213]
                  tunnel: w1197 -> [_ w1207]
                  frame False {
                    n589 = property on="Property Node" class="WFChart (strict)"(reference=w1201) -> (reference out=w1200:refnum<vi>, "XScale.Range"=w1206:T46)  [unwired: 1 in, 1 out]
                    n590 = Bundle By Name(cluster=w1206, "Minimum"=0.0, "Maximum"=3600.0, "Increment"=60.0) -> (w1205:T46)
                    n591 = property on="Property Node" class="WFChart (strict)"(reference=w1200, "XScale.Range"=w1205) -> ()  [unwired: 1 in, 2 out]
                  }
                  frame True {
                    n592 = property on="Property Node" class="WFChart (strict)"(reference=w1213) -> (reference out=w1210:refnum<vi>, "XScale.Range"=w1215:T46)  [unwired: 1 in, 1 out]
                    n593 = Multiply(x=w1207, y=60.0) -> (x*y=w1209:dbl)
                    n594 = Bundle By Name(cluster=w1215, "Minimum"=0.0, "Maximum"=w1209, "Increment"=1.0) -> (w1214:T46)
                    n595 = property on="Property Node" class="WFChart (strict)"(reference=w1210, "XScale.Range"=w1214) -> ()  [unwired: 1 in, 2 out]
                  }
                }
              }
              frame 1 {
                n596 = Not Equal To 0?(x=w1216) -> (x != 0?=w1217:bool)
                n597 = case shown="True" w1217 {
                  tunnel: w1218 -> [w1220 w1230]
                  tunnel: w1216 -> [_ w1227]
                  frame False {
                    n598 = property on="Property Node" class="WFChart (strict)"(reference=w1220) -> (reference out=w1219:refnum<vi>, "XScale.Range"=w1225:T46)  [unwired: 1 in, 1 out]
                    n599 = Bundle By Name(cluster=w1225, "Minimum"=0.0, "Maximum"=43200.0, "Increment"=3600.0) -> (w1221:T46)
                    n600 = property on="Property Node" class="WFChart (strict)"(reference=w1219, "XScale.Range"=w1221) -> ()  [unwired: 1 in, 2 out]
                  }
                  frame True {
                    n601 = Multiply(x=w1227, y=3600.0) -> (x*y=w1226:dbl)
                    n602 = property on="Property Node" class="WFChart (strict)"(reference=w1230) -> (reference out=w1229:refnum<vi>, "XScale.Range"=w1234:T46)  [unwired: 1 in, 1 out]
                    n603 = Bundle By Name(cluster=w1234, "Minimum"=0.0, "Maximum"=w1226, "Increment"=3600.0) -> (w1231:T46)
                    n604 = property on="Property Node" class="WFChart (strict)"(reference=w1229, "XScale.Range"=w1231) -> ()  [unwired: 1 in, 2 out]
                  }
                }
              }
              frame 2 {
                n605 = Not Equal To 0?(x=w1235) -> (x != 0?=w1236:bool)
                n606 = case shown="True" w1236 {
                  tunnel: w1237 -> [w1239 w1247]
                  tunnel: w1235 -> [_ w1245]
                  frame False {
                    n607 = property on="Property Node" class="WFChart (strict)"(reference=w1239) -> (reference out=w1238:refnum<vi>, "XScale.Range"=w1244:T46)  [unwired: 1 in, 1 out]
                    n608 = Bundle By Name(cluster=w1244, "Minimum"=0.0, "Maximum"=60.0, "Increment"=1.0) -> (w1240:T46)
                    n609 = property on="Property Node" class="WFChart (strict)"(reference=w1238, "XScale.Range"=w1240) -> ()  [unwired: 1 in, 2 out]
                  }
                  frame True {
                    n610 = property on="Property Node" class="WFChart (strict)"(reference=w1247) -> (reference out=w1246:refnum<vi>, "XScale.Range"=w1251:T46)  [unwired: 1 in, 1 out]
                    n611 = Bundle By Name(cluster=w1251, "Minimum"=0.0, "Maximum"=w1245, "Increment"=1.0) -> (w1248:T46)
                    n612 = property on="Property Node" class="WFChart (strict)"(reference=w1246, "XScale.Range"=w1248) -> ()  [unwired: 1 in, 2 out]
                  }
                }
              }
            }
          }
          event "1. Compile Profile": Mouse Down {
            n613 = event-data() -> ()  [unwired: 1 in, 1 out]
            n614 = control-ref of="Number of Set points"() -> (w1260:refnum<vi>)
            n615 = property class="DigNum (strict)"(reference=w1260) -> ("Value"=w1257:dbl)  [unwired: 1 in, 2 out]
            n616 = Bundle By Name(cluster=w1259, "ZoneSetup.Number of Set points"=w1257) -> (w1258:T31)
            n617 = local write "ThermalProfileStatus"("Compiling..........." ("String")) -> ()
            n618 = call-poly "Send Message.vi"("error in (no error)"=w1252, "event buffer"="1", "event"="compileProfile") -> ("error out"=w1255:errorcluster)  [unwired: 8 in]
          }
          event "2. Save Into Database and CSV": Mouse Down {
            n619 = event-data() -> ()  [unwired: 1 in, 1 out]
            n620 = Unbundle By Name(w1265) -> ("Http session"=w1282:T30, "URL prefex"=w1278:string, "ZoneProfile.profiles"=w1277:T47, "ZoneSetup.Thermal Profile Name"=w1262:string)
            n621 = Empty String/Path?(string/path=w1262) -> (empty?=w1268:bool)
            n622 = case shown="True" w1268 {
              tunnel: w1262 -> [w1285 _]
              tunnel: [w1285 w1286] -> w1267
              tunnel: w1266 -> [w1284 w1290]
              tunnel: [w1284 w1289] -> w1263
              tunnel: w1265 -> [w1283 w1288]
              tunnel: [w1283 w1287] -> w1264
              frame False {
              }
              frame True {
                n623 = call "Prompt User for Input"("error in (no error)"=w1290) -> ("Profile Name"=w1286:string, "error out"=w1289:errorcluster)  [unwired: 16 in, 1 out]
                n624 = Bundle By Name(cluster=w1288, "ZoneSetup.Thermal Profile Name"=w1286) -> (w1287:T31)
              }
            }
            n625 = Bundle By Name(cluster=T34 {"name"="", "profiles"=[]}, "name"=w1267, "profiles"=w1277) -> (w1275:T34)
            n626 = Concatenate Strings(w1278, "saveProfile" ("url")) -> (w1281:string)
            n627 = Flatten To JSON(anything=w1275) -> (JSON string=w1280:string)  [unwired: 2 in, 1 out]
            n628 = call-poly <vilib>:"POST.vi"("client handle"=w1282, "url"=w1281, "buffer"=w1280) -> ("client handle out"=w1273:T30, "body"=w1269:string)  [unwired: 9 in, 2 out]
            n629 = Match True/False String(2:"" ("false string"), 3:"{'result':'success'}" ("true string"), 4:w1269) -> (0:w1270:bool)  [unwired: 1 out]
            n630 = Bundle By Name(cluster=w1264, "Http session"=w1273) -> (w1274:T31)
            n631 = case shown="True" w1270 {
              tunnel: w1269 -> [w1293 _]
              tunnel: w1263 -> [w1291 w1296]
              tunnel: [w1291 w1295] -> w1261
              frame False {
                n632 = Concatenate Strings("Error While Saving : " ("string"), w1293) -> (w1292:string)
                n633 = One Button Dialog(message=w1292) -> ()  [unwired: 1 in, 1 out]
              }
              frame True {
                n634 = One Button Dialog(message="Profile Saved To Database Successfully") -> ()  [unwired: 1 in, 1 out]
                n635 = call-poly "Send Message.vi"("error in (no error)"=w1296, "event"="saveProfile") -> ("error out"=w1295:errorcluster)  [unwired: 9 in]
              }
            }
          }
          event "3. Run Profile": Mouse Down {
            n636 = event-data() -> ()  [unwired: 1 in, 1 out]
            n637 = Unbundle By Name(w1312) -> ("Http session"=w1313:T30, "URL prefex"=w1304:string, "ZoneSetup.Thermal Profile Name"=w1299:string)  [unwired: 1 out]
            n638 = Bundle By Name(cluster=cluster{"profile_name":string} {"profile_name"=""}, "profile_name"=w1299) -> (w1315:cluster{"profile_name":string})
            n639 = Flatten To JSON(anything=w1315, error in (no error)=w1307) -> (JSON string=w1314:string, 11:w1306:errorcluster)  [unwired: 1 in]
            n640 = Concatenate Strings(w1304, "loadProfile" ("url")) -> (w1317:string)
            n641 = call-poly <vilib>:"POST.vi"("client handle"=w1313, "url"=w1317, "buffer"=w1314, "error in (no error)"=w1306) -> ("client handle out"=w1303:T30, "body"=w1308:string, "error out"=w1305:errorcluster)  [unwired: 8 in, 1 out]
            n642 = Match True/False String(2:"" ("false string"), 3:"{'result':'success'}" ("true string"), 4:w1308) -> (0:w1309:bool)  [unwired: 1 out]
            n643 = case shown="True" w1309 {
              tunnel: w1308 -> [w1324 _]
              tunnel: w1305 -> [w1321 w1342]
              tunnel: [w1320 w1330] -> w1301
              tunnel: w1304 -> [w1319 w1332]
              tunnel: w1303 -> [w1323 w1340]
              tunnel: [w1322 w1331] -> w1300
              tunnel: w1299 -> [_ w1329]
              frame False {
                n644 = Concatenate Strings("Error, Profile Aborted : " ("string"), w1324) -> (w1327:string)
                n645 = Concatenate Strings(w1319, "hardStop" ("url")) -> (w1325:string)
                n646 = call <vilib>:"GET.vi"("client handle"=w1323, "url"=w1325, "error in (no error)"=w1321) -> ("client handle out"=w1322:T30, "error out"=w1320:errorcluster)  [unwired: 9 in, 2 out]
                n647 = One Button Dialog(message=w1327) -> ()  [unwired: 1 in, 1 out]
              }
              frame True {
                n648 = Concatenate Strings(w1332, "runProfile" ("url")) -> (w1341:string)
                n649 = call <vilib>:"GET.vi"("client handle"=w1340, "url"=w1341, "error in (no error)"=w1342) -> ("client handle out"=w1333:T30, "body"=w1337:string, "error out"=w1334:errorcluster)  [unwired: 9 in, 1 out]
                n650 = Match True/False String(2:"" ("false string"), 3:"{'result':'success'}" ("true string"), 4:w1337) -> (0:w1336:bool, 1:w1335:string)
                n651 = case shown="True" w1336 {
                  tunnel: w1335 -> [w1352 _]
                  tunnel: w1334 -> [w1349 w1358]
                  tunnel: w1333 -> [w1350 w1359]
                  tunnel: w1332 -> [w1347 _]
                  tunnel: [w1345 w1359] -> w1331
                  tunnel: [w1344 w1358] -> w1330
                  tunnel: w1329 -> [_ w1356]
                  frame False {
                    n652 = Concatenate Strings("Error, Profile Aborted : " ("string"), w1352) -> (w1351:string)
                    n653 = Concatenate Strings(w1347, "hardStop" ("url")) -> (w1346:string)
                    n654 = call <vilib>:"GET.vi"("client handle"=w1350, "url"=w1346, "error in (no error)"=w1349) -> ("client handle out"=w1345:T30, "error out"=w1344:errorcluster)  [unwired: 9 in, 2 out]
                    n655 = One Button Dialog(message=w1351) -> ()  [unwired: 1 in, 1 out]
                  }
                  frame True {
                    n656 = Concatenate Strings("Success " ("message"), w1356, " is running" ("string")) -> (w1354:string)
                    n657 = One Button Dialog(message=w1354) -> ()  [unwired: 1 in, 1 out]
                  }
                }
              }
            }
            n658 = Bundle By Name(cluster=w1312, "Http session"=w1300) -> (w1302:T31)
          }
          event "Compiled Rename": Value Change {
            n659 = event-data() -> ("CtlRef"=w1362:refnum<vi>, "OldVal"=w1363:bool)  [unwired: 1 in, 4 out]
            n660 = property class="Bool (strict)"(reference=w1362, "Value"=w1363) -> ()  [unwired: 1 in, 2 out]
            n661 = local read "New Compiled File Name"() -> (w1360:string)
            n662 = Bundle By Name(cluster=w1365, "ZoneSetup.Thermal Profile Name"=w1360) -> (w1364:T31)
            n663 = local write "Compiled Profile Name"(w1360) -> ()
            n664 = control-ref of="Thermal Profile Name"() -> (w1361:refnum<vi>)
            n665 = property class="Str"(reference=w1361, "Text.Text"=w1360) -> ()  [unwired: 1 in, 2 out]
          }
          event "Database Rename": Value Change {
            n666 = event-data() -> ("CtlRef"=w1380:refnum<vi>, "OldVal"=w1381:bool)  [unwired: 1 in, 4 out]
            n667 = property class="Bool (strict)"(reference=w1380, "Value"=w1381) -> ()  [unwired: 1 in, 2 out]
            n668 = control-ref of="Rename Existing Database Profile"() -> (w1379:refnum<vi>)
            n669 = property class="Ring (strict)" props=["Value"](reference=w1379, error in=w1376) -> (reference out=w1378:refnum<vi>, error out=w1377:errorcluster)  [unwired: 1 out]
            n670 = property class="Ring (strict)"(reference=w1378, error in=w1377) -> (error out=w1371:errorcluster, "RingText.Text"=w1369:string)  [unwired: 1 out]
            n671 = Concatenate Strings("Are you sure you want to rename " ("string"), w1369) -> (w1374:string)
            n672 = Two Button Dialog(message=w1374, 1:"No" ("F button name (\"Cancel\")"), 2:"Yes" ("T button name (\"OK\")")) -> (T button?=w1367:bool)
            n673 = case shown="True" w1367 {
              tunnel: w1367 -> [_ w1403]
              tunnel: w1371 -> [w1382 w1402]
              tunnel: w1369 -> [_ w1397]
              tunnel: [w1382 w1386] -> w1368
              frame False {
              }
              frame True {
                n674 = call "Prompt User for New Thermal Profile Name"("Enable"=w1403, "error in (no error)"=w1402) -> ("Profile Name"=w1395:string, "error out"=w1401:errorcluster)  [unwired: 15 in, 1 out]
                n675 = local read "TVAC Labview"() -> (w1400:bool)
                n676 = case shown="True" w1400 {
                  tunnel: [path "C:/Users/stefan/AppData/Local/conda/conda/envs/py35/python.exe" ("Path to Python.exe") path "C:/Users/TVAC-admin/AppData/Local/Programs/Python/Python35/python.exe" ("Path to Python.exe")] -> w1399
                  tunnel: [path "C:/Users/stefan/Documents/GitHub/TVAC/head/Labview2017/TVAC_GUI/DatabaseCSV" ("file path (use dialog)") path "C:/Users/TVAC-admin/Documents/TVAC_Github/head/Labview2017/TVAC_GUI/DatabaseCSV" ("file path (use dialog)")] -> w1393
                  frame False {
                  }
                  frame True {
                  }
                }
                n677 = call "lvProfileRename.vi"("error in (no error)"=w1401, "newName"=w1395, "oldName"=w1397, "Path to Python.exe"=w1399) -> ("error out"=w1387:errorcluster, "Raw Python String Output"=w1383:string)  [unwired: 4 in]
                n678 = Concatenate Strings(w1395, ".csv" ("string")) -> (w1390:string)
                n679 = Concatenate Strings(w1397, ".csv" ("string")) -> (w1384:string)
                n680 = Path To String(path=w1393) -> (string=w1392:string)
                n681 = One Button Dialog(message=w1383) -> ()  [unwired: 1 in, 1 out]
                n682 = Concatenate Strings(w1392, "\\" ("string"), w1384) -> (w1391:string)
                n683 = String To Path(string=w1391) -> (path=w1389:path)
                n684 = Strip Path(path=w1389) -> (stripped path=w1394:path)  [unwired: 1 out]
                n685 = Build Path(base path=w1394, name or relative path=w1390) -> (appended path=w1388:path)
                n686 = Move(source path=w1389, error in=w1387, 10:w1388) -> (error out=w1386:errorcluster)  [unwired: 2 in, 2 out]
              }
            }
          }
          event "Hold Profile": Value Change {
            n687 = event-data() -> ("NewVal"=w1408:bool)  [unwired: 1 in, 5 out]
            n688 = Unbundle By Name(w1411) -> ("Http session"=w1412:T30, "URL prefex"=w1415:string)
            n689 = case shown="True" w1408 {
              tunnel: w1415 -> [w1422 w1431]
              tunnel: w1414 -> [w1418 w1429]
              tunnel: [w1419 w1428] -> w1413
              tunnel: w1412 -> [w1421 w1427]
              tunnel: [w1420 w1426] -> w1409
              tunnel: [w1417 w1425] -> _
              tunnel: [w1416 w1424] -> _
              frame False {
                w1416 = "unHold" ("url")
                n690 = Concatenate Strings(w1422, w1416) -> (w1423:string)
                n691 = call <vilib>:"GET.vi"("client handle"=w1421, "url"=w1423, "error in (no error)"=w1418) -> ("client handle out"=w1420:T30, "body"=w1417:string, "error out"=w1419:errorcluster)  [unwired: 9 in, 1 out]
              }
              frame True {
                w1424 = "hold" ("url")
                n692 = Concatenate Strings(w1431, w1424) -> (w1430:string)
                n693 = call <vilib>:"GET.vi"("client handle"=w1427, "url"=w1430, "error in (no error)"=w1429) -> ("client handle out"=w1426:T30, "body"=w1425:string, "error out"=w1428:errorcluster)  [unwired: 9 in, 1 out]
              }
            }
            n694 = Bundle By Name(cluster=w1411, "Http session"=w1409) -> (w1410:T31)
          }
          event "HARD STOP": Mouse Down {
            n695 = event-data() -> ()  [unwired: 1 in, 1 out]
            n696 = Unbundle By Name(w1435) -> ("Http session"=w1436:T30, "URL prefex"=w1440:string)
            n697 = Concatenate Strings(w1440, "hardStop" ("url")) -> (w1439:string)
            n698 = call <vilib>:"GET.vi"("client handle"=w1436, "url"=w1439, "error in (no error)"=w1438) -> ("client handle out"=w1433:T30, "error out"=w1437:errorcluster)  [unwired: 9 in, 2 out]
            n699 = Bundle By Name(cluster=w1435, "Http session"=w1433) -> (w1434:T31)
          }
          event "ZoneSetup.Import Profile": Value Change {
            w1462 = TRUE ("Page Visible")
            n700 = event-data() -> ("CtlRef"=w1447:refnum<vi>, "OldVal"=w1446:bool)  [unwired: 1 in, 4 out]
            n701 = control-ref of="Import CSV as a Thermal Profile"() -> (w1449:refnum<vi>)
            n702 = property class="Path"(reference=w1449, error in=w1448) -> (error out=w1445:errorcluster, "Value"=w1443:path)  [unwired: 1 out]
            n703 = control-ref of="Thermal Profile Loader"() -> (w1472:refnum<vi>)
            n704 = control-ref of="Zone Selection"() -> (w1471:refnum<vi>)
            n705 = property on="Property Node" class="TabCtl (strict)"(reference=w1472) -> ("Pages"=w1465:refnum<vi>[])  [unwired: 1 in, 2 out]
            n706 = property on="Property Node" class="LstBox (strict)"(reference=w1471) -> ("Item Symbols"=w1470:i32[])  [unwired: 1 in, 2 out]
            n707 = Not Equal?(x=path "", y=w1443) -> (x != y?=w1441:bool)
            n708 = Unbundle By Name(w1454) -> ("ZonesSelected"=w1451:bool[])
            n709 = case shown="False" w1441 {
              tunnel: [string[][] [] ("all rows") w1478] -> w1456
              tunnel: w1443 -> [_ w1477]
              tunnel: w1445 -> [w1474 w1476]
              tunnel: [w1474 w1475] -> w1444
              frame False {
              }
              frame True {
                n710 = call-poly <vilib>:"Read Delimited Spreadsheet.vi"("file path (dialog if empty)"=w1477, "error in (no error)"=w1476, "delimiter (\\t)"="," ("delimiter (\\t)")) -> ("all rows"=w1478:string[][], "error out"=w1475:errorcluster)  [unwired: 7 in, 4 out]
              }
            }
            n711 = Array Size(array=w1456) -> (size(s)=w1461:i32[])
            n712 = Index Array(array=w1461, index=0) -> (element=w1459:i32)
            n713 = Subtract(x=w1459, y=7) -> (x-y=w1457:i32)
            n714 = case shown="True" w1441 {
              tunnel: [w1480 w1486] -> w1450
              tunnel: w1447 -> [_ w1483]
              tunnel: w1446 -> [_ w1482]
              tunnel: w1444 -> [w1480 w1481]
              frame False {
              }
              frame True {
                n715 = property class="Bool (strict)"(reference=w1483, "Value"=w1482) -> ()  [unwired: 1 in, 2 out]
                n716 = call-poly "Send Message.vi"("error in (no error)"=w1481, "event"="initThermalProfile") -> ("error out"=w1484:errorcluster)  [unwired: 9 in]
                n717 = local write "ThermalProfileStatus"("Compiling..........." ("String")) -> ()
                n718 = call-poly "Send Message.vi"("error in (no error)"=w1484, "event"="importProfile") -> ("error out"=w1486:errorcluster)  [unwired: 9 in]
              }
            }
            n719 = To Double Precision Float(number=w1457) -> (double precision float=w1455:dbl)
            n720 = for {
              N: 13 -> [_]
              tunnel: w1470 -> [w1605]
              tunnel: w1465 -> [w1606] mode=indexing
              shift-right: [w1598] -> w1452
              shift-left: w1451 -> [w1597]
              i -> [w1600]
              n721 = Greater?(x=w1600, y=1) -> (0:w1602:bool)
              n722 = Less?(x=w1600, y=11 ("x")) -> (x < y?=w1603:bool)
              n723 = And(x=w1603, y=w1602) -> (x .and. y?=w1601:bool)
              n724 = case shown="True" w1601 {
                tunnel: w1606 -> [_ w1617]
                tunnel: w1605 -> [_ w1614]
                tunnel: w1600 -> [_ w1613]
                tunnel: w1597 -> [w1607 w1610]
                tunnel: [w1607 w1608] -> w1598
                frame False {
                }
                frame True {
                  n725 = Subtract(x=w1613, y=2) -> (x-y=w1609:i32)
                  n726 = Index Array(array=w1614, index=w1609) -> (element=w1611:i32)
                  n727 = Equal?(x=38, y=w1611) -> (x = y?=w1615:bool)
                  n728 = case shown="False" w1615 {
                    tunnel: w1617 -> [w1622 w1627]
                    tunnel: w1610 -> [w1621 w1626]
                    tunnel: w1609 -> [w1619 w1625]
                    tunnel: [w1620 w1623] -> w1608
                    frame False {
                      w1618 = FALSE ("Page Visible")
                      n729 = property class="Page"(reference=w1622, "Page Visible"=w1618) -> ()  [unwired: 1 in, 2 out]
                      n730 = Replace Array Subset(array=w1621, new element=w1618, index=w1619) -> (w1620:bool[])
                    }
                    frame True {
                      w1624 = TRUE ("Page Visible")
                      n731 = property class="Page"(reference=w1627, "Page Visible"=w1624) -> ()  [unwired: 1 in, 2 out]
                      n732 = Replace Array Subset(array=w1626, new element=w1624, index=w1625) -> (w1623:bool[])
                    }
                  }
                }
              }
            }
            n733 = Bundle By Name(cluster=w1454, "ZonesSelected"=w1452) -> (w1453:T31)
            n734 = Index Array(array=w1465, index #1=11 ("index"), index #2=1 ("index")) -> (element #1=w1467:refnum<vi>, element #2=w1463:refnum<vi>)
            n735 = property class="Page"(reference=w1467, "Page Visible"=w1462) -> ()  [unwired: 1 in, 2 out]
            n736 = property class="Page"(reference=w1463, "Page Visible"=w1462) -> ()  [unwired: 1 in, 2 out]
            n737 = for {
              N: 9 -> [_]
              tunnel: w1455 -> [w1495]
              i -> [w1489]
              n738 = Initialize Array(0, w1495, 2 ("dimension size")) -> (w1494:i32[][])
              n739 = Initialize Array(0, w1495, 3 ("dimension size")) -> (w1500:i32[][])
              n740 = for {
                N: w1495 -> [_]
                shift-right: [w1595] -> w1491
                shift-left: w1500 -> [w1596]
                shift-right: [w1586] -> w1493
                shift-left: w1494 -> [w1587]
                i -> [w1584]
                w1588 = 0 ("disabled index (col)")
                w1590 = 0 ("disabled index (col)")
                n741 = Increment(x=w1584) -> (x+1=w1589:i32)
                n742 = Increment(x=w1584) -> (x+1=w1591:i32)
                n743 = Replace Array Subset(array=i32[][] [[0]], new element=w1589, index (row)=w1588, index (col)=w1588) -> (w1582:i32[][])
                n744 = Replace Array Subset(array=i32[][] [[0, 0, 0]], new element=w1591, index (row)=w1590, index (col)=w1590) -> (w1594:i32[][])
                n745 = Index Array(array=w1582, index (row)=w1588) -> (element=w1585:i32[])  [unwired: 1 in]
                n746 = Index Array(array=w1594, index (row)=w1590) -> (element=w1593:i32[])  [unwired: 1 in]
                n747 = Replace Array Subset(array=w1587, new element=w1585, index (row)=w1584) -> (w1586:i32[][])  [unwired: 1 in]
                n748 = Replace Array Subset(array=w1596, new element=w1593, index (row)=w1584) -> (w1595:i32[][])  [unwired: 1 in]
              }
              n749 = control-ref of="RampSoakTimes"() -> (w1492:refnum<vi>)
              n750 = To Double Precision Float(number=w1491) -> (double precision float=w1490:dbl[][])
              n751 = property class="Arr (strict)"(reference=w1492, "Value"=w1490) -> ()  [unwired: 1 in, 2 out]
              n752 = Number To Decimal String(number=w1493) -> ()  [unwired: 1 in, 1 out]
              n753 = case shown="8" w1489 {
                frame 0, Default {
                  n754 = control-ref of="Zone Thermocouples"() -> (w1504:refnum<vi>)
                  n755 = property class="LstBox (strict)"(reference=w1504) -> (reference out=w1502:refnum<vi>, "Item Symbols"=w1503:i32[])  [unwired: 1 in, 1 out]
                  n756 = for {
                    N: 81 -> [_]
                    shift-right: [w1506] -> w1501
                    shift-left: w1503 -> [w1508]
                    i -> [w1507]
                    n757 = Replace Array Subset(array=w1508, new element=37, index=w1507) -> (w1506:i32[])
                  }
                  n758 = property class="LstBox (strict)"(reference=w1502, "Item Symbols"=w1501) -> ()  [unwired: 1 in, 2 out]
                }
                frame 1 {
                  n759 = control-ref of="Zone Thermocouples"() -> (w1513:refnum<vi>)
                  n760 = property class="LstBox (strict)"(reference=w1513) -> (reference out=w1511:refnum<vi>, "Item Symbols"=w1512:i32[])  [unwired: 1 in, 1 out]
                  n761 = for {
                    N: 81 -> [_]
                    shift-right: [w1515] -> w1510
                    shift-left: w1512 -> [w1517]
                    i -> [w1516]
                    n762 = Replace Array Subset(array=w1517, new element=37, index=w1516) -> (w1515:i32[])
                  }
                  n763 = property class="LstBox (strict)"(reference=w1511, "Item Symbols"=w1510) -> ()  [unwired: 1 in, 2 out]
                }
                frame 2 {
                  n764 = control-ref of="Zone Thermocouples"() -> (w1522:refnum<vi>)
                  n765 = property class="LstBox (strict)"(reference=w1522) -> (reference out=w1520:refnum<vi>, "Item Symbols"=w1521:i32[])  [unwired: 1 in, 1 out]
                  n766 = for {
                    N: 81 -> [_]
                    shift-right: [w1524] -> w1519
                    shift-left: w1521 -> [w1526]
                    i -> [w1525]
                    n767 = Replace Array Subset(array=w1526, new element=37, index=w1525) -> (w1524:i32[])
                  }
                  n768 = property class="LstBox (strict)"(reference=w1520, "Item Symbols"=w1519) -> ()  [unwired: 1 in, 2 out]
                }
                frame 3 {
                  n769 = control-ref of="Zone Thermocouples"() -> (w1531:refnum<vi>)
                  n770 = property class="LstBox (strict)"(reference=w1531) -> (reference out=w1529:refnum<vi>, "Item Symbols"=w1530:i32[])  [unwired: 1 in, 1 out]
                  n771 = for {
                    N: 81 -> [_]
                    shift-right: [w1533] -> w1528
                    shift-left: w1530 -> [w1535]
                    i -> [w1534]
                    n772 = Replace Array Subset(array=w1535, new element=37, index=w1534) -> (w1533:i32[])
                  }
                  n773 = property class="LstBox (strict)"(reference=w1529, "Item Symbols"=w1528) -> ()  [unwired: 1 in, 2 out]
                }
                frame 4 {
                  n774 = control-ref of="Zone Thermocouples"() -> (w1540:refnum<vi>)
                  n775 = property class="LstBox (strict)"(reference=w1540) -> (reference out=w1538:refnum<vi>, "Item Symbols"=w1539:i32[])  [unwired: 1 in, 1 out]
                  n776 = for {
                    N: 81 -> [_]
                    shift-right: [w1542] -> w1537
                    shift-left: w1539 -> [w1544]
                    i -> [w1543]
                    n777 = Replace Array Subset(array=w1544, new element=37, index=w1543) -> (w1542:i32[])
                  }
                  n778 = property class="LstBox (strict)"(reference=w1538, "Item Symbols"=w1537) -> ()  [unwired: 1 in, 2 out]
                }
                frame 5 {
                  n779 = control-ref of="Zone Thermocouples"() -> (w1549:refnum<vi>)
                  n780 = property class="LstBox (strict)"(reference=w1549) -> (reference out=w1547:refnum<vi>, "Item Symbols"=w1548:i32[])  [unwired: 1 in, 1 out]
                  n781 = for {
                    N: 81 -> [_]
                    shift-right: [w1551] -> w1546
                    shift-left: w1548 -> [w1553]
                    i -> [w1552]
                    n782 = Replace Array Subset(array=w1553, new element=37, index=w1552) -> (w1551:i32[])
                  }
                  n783 = property class="LstBox (strict)"(reference=w1547, "Item Symbols"=w1546) -> ()  [unwired: 1 in, 2 out]
                }
                frame 6 {
                  n784 = control-ref of="Zone Thermocouples"() -> (w1558:refnum<vi>)
                  n785 = property class="LstBox (strict)"(reference=w1558) -> (reference out=w1556:refnum<vi>, "Item Symbols"=w1557:i32[])  [unwired: 1 in, 1 out]
                  n786 = for {
                    N: 81 -> [_]
                    shift-right: [w1560] -> w1555
                    shift-left: w1557 -> [w1562]
                    i -> [w1561]
                    n787 = Replace Array Subset(array=w1562, new element=37, index=w1561) -> (w1560:i32[])
                  }
                  n788 = property class="LstBox (strict)"(reference=w1556, "Item Symbols"=w1555) -> ()  [unwired: 1 in, 2 out]
                }
                frame 7 {
                  n789 = control-ref of="Zone Thermocouples"() -> (w1567:refnum<vi>)
                  n790 = property class="LstBox (strict)"(reference=w1567) -> (reference out=w1565:refnum<vi>, "Item Symbols"=w1566:i32[])  [unwired: 1 in, 1 out]
                  n791 = for {
                    N: 81 -> [_]
                    shift-right: [w1569] -> w1564
                    shift-left: w1566 -> [w1571]
                    i -> [w1570]
                    n792 = Replace Array Subset(array=w1571, new element=37, index=w1570) -> (w1569:i32[])
                  }
                  n793 = property class="LstBox (strict)"(reference=w1565, "Item Symbols"=w1564) -> ()  [unwired: 1 in, 2 out]
                }
                frame 8 {
                  n794 = control-ref of="Zone Thermocouples"() -> (w1576:refnum<vi>)
                  n795 = property class="LstBox (strict)"(reference=w1576) -> (reference out=w1574:refnum<vi>, "Item Symbols"=w1575:i32[])  [unwired: 1 in, 1 out]
                  n796 = for {
                    N: 81 -> [_]
                    shift-right: [w1578] -> w1573
                    shift-left: w1575 -> [w1580]
                    i -> [w1579]
                    n797 = Replace Array Subset(array=w1580, new element=37, index=w1579) -> (w1578:i32[])
                  }
                  n798 = property class="LstBox (strict)"(reference=w1574, "Item Symbols"=w1573) -> ()  [unwired: 1 in, 2 out]
                }
              }
            }
          }
          event "ZoneSetup.LoadFromDatabase": Value Change {
            n799 = event-data() -> ("CtlRef"=w1634:refnum<vi>, "OldVal"=w1633:bool)  [unwired: 1 in, 4 out]
            n800 = local read "TVAC Labview"() -> (w1641:bool)
            n801 = property class="Bool (strict)"(reference=w1634, "Value"=w1633) -> ()  [unwired: 1 in, 2 out]
            n802 = control-ref of="Saved Database Profiles"() -> (w1647:refnum<vi>)
            n803 = property class="Ring (strict)" props=["Value"](reference=w1647, error in=w1638) -> (reference out=w1646:refnum<vi>, error out=w1640:errorcluster)  [unwired: 1 out]
            n804 = case shown="True" w1641 {
              tunnel: ["C:\\Users\\stefan\\Documents\\GitHub\\TVAC\\head\\Labview2017\\TVAC_GUI\\DatabaseCSV\\" "C:\\Users\\TVAC-admin\\Documents\\TVAC_Github\\head\\Labview2017\\TVAC_GUI\\DatabaseCSV\\" ("file path (use dialog)")] -> w1645
              frame False {
              }
              frame True {
              }
            }
            n805 = property class="Ring (strict)"(reference=w1646, error in=w1640) -> (error out=w1639:errorcluster, "RingText.Text"=w1644:string)  [unwired: 1 out]
            n806 = Concatenate Strings(w1645, w1644, ".csv" ("string")) -> (w1642:string)
            n807 = String To Path(string=w1642) -> (path=w1629:path)
            n808 = control-ref of="Import CSV as a Thermal Profile"() -> (w1648:refnum<vi>)
            n809 = property class="Path"(reference=w1648, error in=w1639, "Value"=w1629) -> (error out=w1630:errorcluster)  [unwired: 1 out]
            n810 = call <vilib>:"Simple Error Handler.vi"("error in (no error)"=w1630) -> ("error?"=w1631:bool, "error out"=w1632:errorcluster)  [unwired: 4 in, 3 out]
            n811 = call-poly <vilib>:"Read Delimited Spreadsheet.vi"("file path (dialog if empty)"=w1629) -> ("all rows"=w1628:string[][])  [unwired: 9 in, 5 out]
            n812 = case shown="False" w1631 {
              tunnel: [w1670 w1710] -> w1637
              tunnel: w1636 -> [w1663 w1711]
              tunnel: [w1662 w1711] -> w1635
              tunnel: w1632 -> [w1653 w1710]
              tunnel: w1628 -> [w1649 _]
              frame False {
                w1669 = TRUE ("Page Visible")
                (unwired) 13
                n813 = control-ref of="Thermal Profile Loader"() -> (w1677:refnum<vi>)
                n814 = control-ref of="Zone Selection"() -> (w1676:refnum<vi>)
                n815 = property on="Property Node" class="TabCtl (strict)"(reference=w1677) -> ("Pages"=w1666:refnum<vi>[])  [unwired: 1 in, 2 out]
                n816 = property class="LstBox (strict)"(reference=w1676) -> ("Value"=w1660:i32[])  [unwired: 1 in, 2 out]
                n817 = Index Array(array=w1649, index (row)=1, index (col)=0 ("disabled index (col)")) -> (element=w1656:string)
                n818 = Unbundle By Name(w1663) -> ("ZonesSelected"=w1664:bool[])
                n819 = Spreadsheet String To Array(delimiter (Tab)=",", format string="%s", spreadsheet string=w1656, array type (2D Dbl)=string[] []) -> (array=w1654:string[])
                n820 = call-poly "Send Message.vi"("error in (no error)"=w1653, "event"="initThermalProfile") -> ("error out"=w1652:errorcluster)  [unwired: 9 in]
                n821 = for {
                  N: 9 -> [_]
                  tunnel: w1654 -> [w1680]
                  shift-right: [w1685] -> w1661
                  shift-left: w1664 -> [w1684]
                  shift-right: [w1682] -> _
                  shift-left: w1660 -> [w1683]
                  shift-right: [w1681] -> _
                  shift-left: w1666 -> [w1686]
                  i -> [w1678]
                  n822 = Index Array(array=w1680, index=w1678) -> (element=w1679:string)
                  n823 = Empty String/Path?(string/path=w1679) -> (empty?=w1687:bool)
                  n824 = case shown="True" w1687 {
                    tunnel: w1686 -> [w1688 w1699]
                    tunnel: w1678 -> [w1690 w1701]
                    tunnel: w1684 -> [w1694 w1706]
                    tunnel: [w1693 w1705] -> w1685
                    tunnel: w1683 -> [w1692 w1703]
                    tunnel: [w1691 w1702] -> w1682
                    tunnel: [w1688 w1699] -> w1681
                    frame False {
                      w1695 = TRUE ("Page Visible")
                      n825 = Add(x=2, y=w1690) -> (x+y=w1698:i32)
                      n826 = Index Array(array=w1688, index=w1698) -> (element=w1696:refnum<vi>)
                      n827 = property class="Page"(reference=w1696, "Page Visible"=w1695) -> ()  [unwired: 1 in, 2 out]
                      n828 = Replace Array Subset(array=w1694, new element=w1695, index=w1690) -> (w1693:bool[])
                      n829 = Replace Array Subset(array=w1692, new element=38, index=w1690) -> (w1691:i32[])
                    }
                    frame True {
                      w1704 = FALSE ("Page Visible")
                      n830 = Add(x=2, y=w1701) -> (x+y=w1709:i32)
                      n831 = Index Array(array=w1699, index=w1709) -> (element=w1707:refnum<vi>)
                      n832 = property class="Page"(reference=w1707, "Page Visible"=w1704) -> ()  [unwired: 1 in, 2 out]
                      n833 = Replace Array Subset(array=w1706, new element=w1704, index=w1701) -> (w1705:bool[])
                      n834 = Replace Array Subset(array=w1703, new element=37, index=w1701) -> (w1702:i32[])
                    }
                  }
                }
                n835 = call-poly "Send Message.vi"("error in (no error)"=w1652, "event"="importProfile") -> ("error out"=w1665:errorcluster)  [unwired: 9 in]
                n836 = Bundle By Name(cluster=w1663, "ZonesSelected"=w1661) -> (w1662:T31)
                n837 = Index Array(array=w1666, index #1=11 ("index"), index #2=1 ("index")) -> (element #1=w1673:refnum<vi>, element #2=w1672:refnum<vi>)
                n838 = property class="Page"(reference=w1672, error in=w1665, "Page Visible"=w1669) -> (error out=w1671:errorcluster)  [unwired: 1 out]
                n839 = property class="Page"(reference=w1673, error in=w1671, "Page Visible"=w1669) -> (error out=w1670:errorcluster)  [unwired: 1 out]
              }
              frame True {
              }
            }
          }
          event "Current Errors (click to clear)": Mouse Down {
            n840 = event-data() -> ("CtlRef"=w1721:refnum<vi>, "Coords"=w1720:T45)  [unwired: 1 in]
            n841 = invoke on="Invoke Node" class="MCListbox (strict)" method="Point To Row Column"(reference=w1721, "Point"=w1720) -> (reference out=w1717:refnum<vi>, "InBounds"=w1714:bool, "CellPosition"=w1718:T48)  [unwired: 5 in, 4 out]
            n842 = case shown="True" w1714 {
              tunnel: w1718 -> [_ w1734]
              tunnel: w1717 -> [_ w1733]
              tunnel: w1716 -> [w1722 w1732]
              tunnel: [w1722 w1731] -> w1715
              frame False {
              }
              frame True {
                n843 = Unbundle By Name(w1734) -> ("Row"=w1727:i32)
                n844 = property on="Property Node" class="MCListbox (strict)"(reference=w1733, "ActiveCell"=w1734) -> (reference out=w1729:refnum<vi>)  [unwired: 1 in, 1 out]
                n845 = Unbundle By Name(w1732) -> ("ErrorArray"=w1728:string[][], "PrevErrorArray"=w1730:string[][])
                n846 = Index Array(array=w1728, index (row)=w1727, index (col)=1 ("disabled index (col)")) -> (element=w1723:string)
                n847 = Equal?(x=w1723, y="") -> (x = y?=w1725:bool)
                n848 = case shown="False" w1725 {
                  tunnel: w1732 -> [w1753 w1754]
                  tunnel: [w1752 w1754] -> w1731
                  tunnel: w1730 -> [w1751 _]
                  tunnel: w1729 -> [w1749 _]
                  tunnel: w1728 -> [w1746 _]
                  tunnel: w1727 -> [w1745 _]
                  frame False {
                    n849 = control-ref of="Error History"() -> (w1748:refnum<vi>)
                    n850 = Delete From Array(array=w1746, index (row)=w1745) -> (deleted portion=w1750:string[], array with subset deleted=w1744:string[][])  [unwired: 2 in]
                    n851 = Build Array (concatenate)(w1750, w1751) -> (w1747:string[][])
                    n852 = property on="Property Node" class="MCListbox (strict)"(reference=w1749, "ItemNames"=w1744) -> ()  [unwired: 1 in, 2 out]
                    n853 = property on="Property Node" class="MCListbox (strict)"(reference=w1748, "ItemNames"=w1747) -> ()  [unwired: 1 in, 2 out]
                    n854 = Index Array(array=w1744, index (row)=0, index (col)=1 ("disabled index (col)")) -> (element=w1741:string)
                    n855 = Bundle By Name(cluster=w1753, "ErrorArray"=w1744, "PrevErrorArray"=w1747) -> (w1752:T31)
                    n856 = Equal?(x=w1741, y="") -> (x = y?=w1739:bool)
                    n857 = Select(t=FALSE, s=w1739, f=TRUE) -> (s? t:f=w1735:bool)
                    n858 = control-ref of="Active Errors"() -> (w1736:refnum<vi>)
                    n859 = property class="Bool (strict)"(reference=w1736, "Value"=w1735) -> ()  [unwired: 1 in, 2 out]
                  }
                  frame True {
                  }
                }
              }
            }
          }
          event "Current Events (click to clear)": Mouse Down {
            n860 = event-data() -> ("CtlRef"=w1762:refnum<vi>, "Coords"=w1761:T45)  [unwired: 1 in]
            n861 = invoke on="Invoke Node" class="MCListbox (strict)" method="Point To Row Column"(reference=w1762, "Point"=w1761) -> (reference out=w1758:refnum<vi>, "InBounds"=w1755:bool, "CellPosition"=w1759:T48)  [unwired: 5 in, 4 out]
            n862 = case shown="True" w1755 {
              tunnel: w1759 -> [_ w1775]
              tunnel: w1758 -> [_ w1774]
              tunnel: w1757 -> [w1763 w1773]
              tunnel: [w1763 w1772] -> w1756
              frame False {
              }
              frame True {
                n863 = Unbundle By Name(w1775) -> ("Row"=w1768:i32)
                n864 = property on="Property Node" class="MCListbox (strict)"(reference=w1774, "ActiveCell"=w1775) -> (reference out=w1770:refnum<vi>)  [unwired: 1 in, 1 out]
                n865 = Unbundle By Name(w1773) -> ("EventArray"=w1769:string[][], "PrevEventArray"=w1771:string[][])
                n866 = Index Array(array=w1769, index (row)=w1768, index (col)=1 ("disabled index (col)")) -> (element=w1764:string)
                n867 = Equal?(x=w1764, y="") -> (x = y?=w1766:bool)
                n868 = case shown="False" w1766 {
                  tunnel: w1773 -> [w1785 w1786]
                  tunnel: [w1784 w1786] -> w1772
                  tunnel: w1771 -> [w1783 _]
                  tunnel: w1770 -> [w1781 _]
                  tunnel: w1769 -> [w1777 _]
                  tunnel: w1768 -> [w1776 _]
                  frame False {
                    n869 = control-ref of="Event History"() -> (w1780:refnum<vi>)
                    n870 = Delete From Array(array=w1777, index (row)=w1776) -> (deleted portion=w1782:string[], array with subset deleted=w1778:string[][])  [unwired: 2 in]
                    n871 = Build Array (concatenate)(w1782, w1783) -> (w1779:string[][])
                    n872 = property on="Property Node" class="MCListbox (strict)"(reference=w1781, "ItemNames"=w1778) -> ()  [unwired: 1 in, 2 out]
                    n873 = property on="Property Node" class="MCListbox (strict)"(reference=w1780, "ItemNames"=w1779) -> ()  [unwired: 1 in, 2 out]
                    n874 = Bundle By Name(cluster=w1785, "EventArray"=w1778, "PrevEventArray"=w1779) -> (w1784:T31)
                  }
                  frame True {
                  }
                }
              }
            }
          }
          event "Clear All Errors": Mouse Down {
            w1793 = 0 ("index")
            n875 = event-data() -> ()  [unwired: 1 in, 5 out]
            n876 = Unbundle By Name(w1806) -> ("ErrorArray"=w1792:string[][], "PrevErrorArray"=w1804:string[][])
            n877 = Array Size(array=w1792) -> (size(s)=w1802:i32[])
            n878 = Index Array(array=w1802, index #1=w1793, index #2=1 ("index")) -> (element #1=w1800:i32)  [unwired: 1 out]
            n879 = Index Array(array=w1792, index (col)=1 ("disabled index (col)")) -> (element=w1795:string[])  [unwired: 1 in]
            n880 = Array Size(array=w1792) -> (size(s)=w1791:i32[])
            n881 = Initialize Array(0, w1800) -> (w1798:i32[])
            n882 = Index Array(array=w1795, index=w1793) -> (element=w1794:string)
            n883 = Index Array(array=w1791, index=0) -> (element=w1789:i32)
            n884 = Not Equal?(x=w1794, y="") -> (x != y?=w1797:bool)
            n885 = case shown="True" w1797 {
              tunnel: w1806 -> [w1808 w1819]
              tunnel: [w1808 w1818] -> w1805
              tunnel: w1804 -> [_ w1817]
              tunnel: w1792 -> [_ w1813]
              tunnel: w1798 -> [_ w1816]
              tunnel: w1789 -> [_ w1810]
              frame False {
              }
              frame True {
                w1809 = string[][] [] ("Item Names")
                n886 = for {
                  N: w1810 -> [_]
                  shift-right: [w1825] -> w1811
                  shift-left: w1817 -> [w1826]
                  shift-right: [w1824] -> w1814
                  shift-left: w1816 -> [w1824]
                  tunnel: w1813 -> [w1820] mode=indexing
                  n887 = Index Array(array=w1820, index=1) -> (element=w1821:string)
                  n888 = Empty String/Path?(string/path=w1821) -> (empty?=w1823:bool)
                  n889 = case shown="False" w1823 {
                    tunnel: w1826 -> [w1829 w1830]
                    tunnel: [w1828 w1830] -> w1825
                    tunnel: w1820 -> [w1827 _]
                    frame False {
                      n890 = Build Array (concatenate)(w1827, w1829) -> (w1828:string[][])
                    }
                    frame True {
                    }
                  }
                }
                n891 = Bundle By Name(cluster=w1819, "ErrorArray"=w1809, "PrevErrorArray"=w1811) -> (w1818:T31)
                n892 = control-ref of="Current Errors (click to clear)"() -> (w1815:refnum<vi>)
                n893 = property on="Property Node" class="MCListbox (strict)"(reference=w1815, "ItemNames"=w1809) -> ()  [unwired: 1 in, 2 out]
                n894 = property on="Property Node" class="MCListbox (strict)"(reference=w1815, "ItemSyms"=w1814) -> ()  [unwired: 1 in, 2 out]
                n895 = control-ref of="Error History"() -> (w1812:refnum<vi>)
                n896 = property on="Property Node" class="MCListbox (strict)"(reference=w1812, "ItemNames"=w1811) -> ()  [unwired: 1 in, 2 out]
              }
            }
            n897 = control-ref of="Active Errors"() -> (w1788:refnum<vi>)
            n898 = property class="Bool (strict)"(reference=w1788, "Value"=FALSE) -> ()  [unwired: 1 in, 2 out]
          }
          event "Clear All Events": Mouse Down {
            w1835 = 0 ("index")
            n899 = event-data() -> ()  [unwired: 1 in, 5 out]
            n900 = Unbundle By Name(w1848) -> ("EventArray"=w1834:string[][], "PrevEventArray"=w1846:string[][])
            n901 = Array Size(array=w1834) -> (size(s)=w1844:i32[])
            n902 = Index Array(array=w1844, index #1=w1835, index #2=1 ("index")) -> (element #1=w1842:i32)  [unwired: 1 out]
            n903 = Index Array(array=w1834, index (col)=1 ("disabled index (col)")) -> (element=w1837:string[])  [unwired: 1 in]
            n904 = Array Size(array=w1834) -> (size(s)=w1833:i32[])
            n905 = Initialize Array(0, w1842) -> (w1840:i32[])
            n906 = Index Array(array=w1837, index=w1835) -> (element=w1836:string)
            n907 = Index Array(array=w1833, index=0) -> (element=w1831:i32)
            n908 = Not Equal?(x=w1836, y="") -> (x != y?=w1839:bool)
            n909 = case shown="True" w1839 {
              tunnel: w1848 -> [w1850 w1861]
              tunnel: [w1850 w1860] -> w1847
              tunnel: w1846 -> [_ w1859]
              tunnel: w1834 -> [_ w1855]
              tunnel: w1840 -> [_ w1858]
              tunnel: w1831 -> [_ w1852]
              frame False {
              }
              frame True {
                w1851 = string[][] [] ("Item Names")
                n910 = for {
                  N: w1852 -> [_]
                  shift-right: [w1867] -> w1853
                  shift-left: w1859 -> [w1868]
                  shift-right: [w1866] -> w1856
                  shift-left: w1858 -> [w1866]
                  tunnel: w1855 -> [w1862] mode=indexing
                  n911 = Index Array(array=w1862, index=1) -> (element=w1863:string)
                  n912 = Empty String/Path?(string/path=w1863) -> (empty?=w1865:bool)
                  n913 = case shown="False" w1865 {
                    tunnel: w1868 -> [w1871 w1872]
                    tunnel: [w1870 w1872] -> w1867
                    tunnel: w1862 -> [w1869 _]
                    frame False {
                      n914 = Build Array (concatenate)(w1869, w1871) -> (w1870:string[][])
                    }
                    frame True {
                    }
                  }
                }
                n915 = Bundle By Name(cluster=w1861, "EventArray"=w1851, "PrevEventArray"=w1853) -> (w1860:T31)
                n916 = control-ref of="Current Events (click to clear)"() -> (w1857:refnum<vi>)
                n917 = property on="Property Node" class="MCListbox (strict)"(reference=w1857, "ItemNames"=w1851) -> ()  [unwired: 1 in, 2 out]
                n918 = property on="Property Node" class="MCListbox (strict)"(reference=w1857, "ItemSyms"=w1856) -> ()  [unwired: 1 in, 2 out]
                n919 = control-ref of="Event History"() -> (w1854:refnum<vi>)
                n920 = property on="Property Node" class="MCListbox (strict)"(reference=w1854, "ItemNames"=w1853) -> ()  [unwired: 1 in, 2 out]
              }
            }
          }
          event "ZoneSetup.Zone Selection": Mouse Down {
            n921 = event-data() -> ("CtlRef"=w1879:refnum<vi>, "Coords"=w1885:T45)  [unwired: 1 in]
            n922 = Unbundle By Name(w1876) -> ("ZonesSelected"=w1877:bool[])
            n923 = invoke on="Invoke Node" class="LstBox (strict)" method="Point To Row"(reference=w1879, "Point"=w1885) -> ("Row"=w1878:i32)  [unwired: 5 in, 6 out]
            n924 = property on="Property Node" class="LstBox (strict)"(reference=w1879) -> ("Item Symbols"=w1881:i32[])  [unwired: 1 in, 2 out]
            n925 = Index Array(array=w1881, index=w1878) -> (element=w1883:i32)
            n926 = Equal?(x=w1883, y=37) -> (x = y?=w1884:bool)
            n927 = case shown="True" w1884 {
              tunnel: w1881 -> [w1891 w1899]
              tunnel: w1878 -> [w1887 w1896]
              tunnel: [w1890 w1897] -> w1873
              tunnel: w1877 -> [w1889 w1894]
              tunnel: [w1886 w1893] -> w1874
              frame False {
                n928 = Replace Array Subset(array=w1889, new element=FALSE ("Boolean"), index=w1887) -> (w1886:bool[])
                n929 = Replace Array Subset(array=w1891, new element=37, index=w1887) -> (w1890:i32[])
              }
              frame True {
                n930 = Replace Array Subset(array=w1894, new element=TRUE ("Boolean"), index=w1896) -> (w1893:bool[])
                n931 = Replace Array Subset(array=w1899, new element=38, index=w1896) -> (w1897:i32[])
              }
            }
            n932 = Bundle By Name(cluster=w1876, "ZonesSelected"=w1874, "ZoneSetup.Zone Selection"=w1873) -> (w1875:T31)
            n933 = property on="Property Node" class="LstBox (strict)"(reference=w1879, "Item Symbols"=w1873) -> ()  [unwired: 1 in, 2 out]
          }
          event "ZoneSetup.Initiate Setup": Value Change {
            w1906 = TRUE ("Page Visible")
            n934 = event-data() -> ("CtlRef"=w1905:refnum<vi>, "OldVal"=w1904:bool)  [unwired: 1 in, 4 out]
            n935 = control-ref of="Thermal Profile Loader"() -> (w1918:refnum<vi>)
            n936 = property class="Bool (strict)"(reference=w1905, "Value"=w1904) -> ()  [unwired: 1 in, 2 out]
            n937 = control-ref of="Zone Selection"() -> (w1917:refnum<vi>)
            n938 = property on="Property Node" class="TabCtl (strict)"(reference=w1918) -> ("Pages"=w1909:refnum<vi>[])  [unwired: 1 in, 2 out]
            n939 = property on="Property Node" class="LstBox (strict)"(reference=w1917) -> ("Item Symbols"=w1916:i32[])  [unwired: 1 in, 2 out]
            n940 = for {
              N: 13 -> [_]
              tunnel: w1916 -> [w1972]
              tunnel: w1909 -> [w1973] mode=indexing
              i -> [w1967]
              n941 = Greater?(x=w1967, y=1) -> (0:w1969:bool)
              n942 = Less?(x=w1967, y=11 ("x")) -> (x < y?=w1970:bool)
              n943 = And(x=w1970, y=w1969) -> (x .and. y?=w1968:bool)
              n944 = case shown="True" w1968 {
                tunnel: w1973 -> [_ w1981]
                tunnel: w1972 -> [_ w1978]
                tunnel: w1967 -> [_ w1977]
                frame False {
                }
                frame True {
                  n945 = Subtract(x=w1977, y=2) -> (x-y=w1975:i32)
                  n946 = Index Array(array=w1978, index=w1975) -> (element=w1974:i32)
                  n947 = Equal?(x=38, y=w1974) -> (x = y?=w1979:bool)
                  n948 = case shown="True" w1979 {
                    tunnel: w1981 -> [w1982 w1984]
                    frame False {
                      n949 = property class="Page"(reference=w1982, "Page Visible"=FALSE) -> ()  [unwired: 1 in, 2 out]
                    }
                    frame True {
                      n950 = property class="Page"(reference=w1984, "Page Visible"=TRUE) -> ()  [unwired: 1 in, 2 out]
                    }
                  }
                }
              }
            }
            n951 = call-poly "Send Message.vi"("error in (no error)"=w1901, "event"="initThermalProfile") -> ("error out"=w1900:errorcluster)  [unwired: 9 in]
            n952 = Index Array(array=w1909, index #1=11 ("index"), index #2=1 ("index")) -> (element #1=w1913:refnum<vi>, element #2=w1907:refnum<vi>)
            n953 = property class="Page"(reference=w1913, "Page Visible"=w1906) -> ()  [unwired: 1 in, 2 out]
            n954 = property class="Page"(reference=w1907, "Page Visible"=w1906) -> ()  [unwired: 1 in, 2 out]
            n955 = property on="Number of Set points" class="DigNum (strict)"() -> ("NumText.Text"=w1910:string)  [unwired: 2 in, 2 out]
            n956 = Decimal String To Number(string=w1910) -> (number=w1903:i32)  [unwired: 2 in, 1 out]
            n957 = for {
              N: 9 -> [_]
              tunnel: w1903 -> [w1925]
              i -> [w1923]
              n958 = Initialize Array(0, w1925, 2 ("dimension size")) -> (w1924:i32[][])
              n959 = Initialize Array(0, w1925, 3 ("dimension size")) -> (w1930:i32[][])
              n960 = for {
                N: w1925 -> [_]
                shift-right: [w1964] -> w1921
                shift-left: w1930 -> [w1965]
                shift-right: [w1955] -> w1920
                shift-left: w1924 -> [w1956]
                i -> [w1953]
                w1957 = 0 ("disabled index (col)")
                w1959 = 0 ("disabled index (col)")
                n961 = Increment(x=w1953) -> (x+1=w1958:i32)
                n962 = Increment(x=w1953) -> (x+1=w1960:i32)
                n963 = Replace Array Subset(array=i32[][] [[0, 0]], new element=w1958, index (row)=w1957, index (col)=w1957) -> (w1951:i32[][])
                n964 = Replace Array Subset(array=i32[][] [[0, 0, 0]], new element=w1960, index (row)=w1959, index (col)=w1959) -> (w1963:i32[][])
                n965 = Index Array(array=w1951, index (row)=w1957) -> (element=w1954:i32[])  [unwired: 1 in]
                n966 = Index Array(array=w1963, index (row)=w1959) -> (element=w1962:i32[])  [unwired: 1 in]
                n967 = Replace Array Subset(array=w1956, new element=w1954, index (row)=w1953) -> (w1955:i32[][])  [unwired: 1 in]
                n968 = Replace Array Subset(array=w1965, new element=w1962, index (row)=w1953) -> (w1964:i32[][])  [unwired: 1 in]
              }
              n969 = To Double Precision Float(number=w1920) -> (double precision float=w1919:dbl[][])
              n970 = To Double Precision Float(number=w1921) -> (double precision float=w1922:dbl[][])
              n971 = case shown="0, Default" w1923 {
                tunnel: w1922 -> [w1932 _ _ _ _ _ _ _ _]
                tunnel: w1919 -> [w1931 w1935 w1937 w1939 w1941 w1943 w1945 w1947 w1949]
                frame 0, Default {
                  n972 = control-ref of="Temperature Goal"() -> (w1934:refnum<vi>)
                  n973 = control-ref of="RampSoakTimes"() -> (w1933:refnum<vi>)
                  n974 = property class="Arr (strict)"(reference=w1934, "Value"=w1931) -> ()  [unwired: 1 in, 2 out]
                  n975 = property class="Arr (strict)"(reference=w1933, "Value"=w1932) -> ()  [unwired: 1 in, 2 out]
                }
                frame 1 {
                  n976 = control-ref of="Temperature Goal"() -> (w1936:refnum<vi>)
                  n977 = property class="Arr (strict)"(reference=w1936, "Value"=w1935) -> ()  [unwired: 1 in, 2 out]
                }
                frame 2 {
                  n978 = control-ref of="Temperature Goal"() -> (w1938:refnum<vi>)
                  n979 = property class="Arr (strict)"(reference=w1938, "Value"=w1937) -> ()  [unwired: 1 in, 2 out]
                }
                frame 3 {
                  n980 = control-ref of="Temperature Goal"() -> (w1940:refnum<vi>)
                  n981 = property class="Arr (strict)"(reference=w1940, "Value"=w1939) -> ()  [unwired: 1 in, 2 out]
                }
                frame 4 {
                  n982 = control-ref of="Temperature Goal"() -> (w1942:refnum<vi>)
                  n983 = property class="Arr (strict)"(reference=w1942, "Value"=w1941) -> ()  [unwired: 1 in, 2 out]
                }
                frame 5 {
                  n984 = control-ref of="Temperature Goal"() -> (w1944:refnum<vi>)
                  n985 = property class="Arr (strict)"(reference=w1944, "Value"=w1943) -> ()  [unwired: 1 in, 2 out]
                }
                frame 6 {
                  n986 = control-ref of="Temperature Goal"() -> (w1946:refnum<vi>)
                  n987 = property class="Arr (strict)"(reference=w1946, "Value"=w1945) -> ()  [unwired: 1 in, 2 out]
                }
                frame 7 {
                  n988 = control-ref of="Temperature Goal"() -> (w1948:refnum<vi>)
                  n989 = property class="Arr (strict)"(reference=w1948, "Value"=w1947) -> ()  [unwired: 1 in, 2 out]
                }
                frame 8 {
                  n990 = control-ref of="Temperature Goal"() -> (w1950:refnum<vi>)
                  n991 = property class="Arr (strict)"(reference=w1950, "Value"=w1949) -> ()  [unwired: 1 in, 2 out]
                }
              }
            }
          }
          event Mouse Down {
            n992 = event-data() -> ("CtlRef"=w1986:refnum<vi>, "Coords"=w1992:T45)  [unwired: 1 in, 6 out]
            n993 = invoke on="Invoke Node" class="LstBox (strict)" method="Point To Row"(reference=w1986, "Point"=w1992) -> ("InBounds"=w1987:bool, "Row"=w1988:i32)  [unwired: 5 in, 5 out]
            n994 = property on="Property Node" class="LstBox (strict)"(reference=w1986) -> ("Item Symbols"=w1991:i32[])  [unwired: 1 in, 2 out]
            n995 = case shown="True" w1987 {
              tunnel: w1986 -> [_ w1994]
              tunnel: w1991 -> [_ w2002]
              tunnel: w1988 -> [_ w2001]
              frame False {
              }
              frame True {
                n996 = Index Array(array=w2002, index=w2001) -> (element=w2004:i32)
                n997 = control-ref of="Thermocouples Selected"() -> (w1993:refnum<vi>)
                n998 = Equal?(x=w2004, y=37) -> (x = y?=w1999:bool)
                n999 = case shown="True" w1999 {
                  tunnel: w2002 -> [w2017 w2031]
                  tunnel: w2001 -> [w2014 w2027]
                  tunnel: [w2016 w2029] -> w1996
                  tunnel: w1993 -> [w2015 w2028]
                  frame False {
                    n1000 = Not Equal To 0?(x=w2014) -> (x != 0?=w2013:bool)
                    n1001 = case shown="True" w2013 {
                      tunnel: w2014 -> [_ w2025]
                      tunnel: w2015 -> [_ w2024]
                      frame False {
                      }
                      frame True {
                        n1002 = Number To Decimal String(number=w2025) -> (decimal integer string=w2022:string)  [unwired: 1 in]
                        n1003 = property class="Str"(reference=w2024) -> (reference out=w2023:refnum<vi>, "Text.Text"=w2020:string)  [unwired: 1 in, 1 out]
                        n1004 = call <vilib>:"Space Constant.vi"() -> ("String"=w2021:string)
                        n1005 = Search and Replace String(input string=w2020, search string=w2022, replace string=w2021) -> (result string=w2019:string)  [unwired: 5 in, 3 out]
                        n1006 = property class="Str"(reference=w2023, "Text.Text"=w2019) -> ()  [unwired: 1 in, 2 out]
                      }
                    }
                    n1007 = Replace Array Subset(array=w2017, new element=37, index=w2014) -> (w2016:i32[])
                  }
                  frame True {
                    n1008 = Not Equal To 0?(x=w2027) -> (x != 0?=w2026:bool)
                    n1009 = case shown="False" w2026 {
                      tunnel: w2028 -> [w2032 w2039]
                      tunnel: w2027 -> [_ w2038]
                      frame False {
                        n1010 = property class="Str"(reference=w2032, "Text.Text"="") -> ()  [unwired: 1 in, 2 out]
                      }
                      frame True {
                        n1011 = Number To Decimal String(number=w2038) -> (decimal integer string=w2034:string)  [unwired: 1 in]
                        n1012 = property class="Str"(reference=w2039) -> ("Text.Text"=w2037:string)  [unwired: 1 in, 2 out]
                        n1013 = call <vilib>:"Space Constant.vi"() -> ("String"=w2035:string)
                        n1014 = Concatenate Strings(w2037, w2035, w2034) -> (w2036:string)
                        n1015 = property class="Str"(reference=w2039, "Text.Text"=w2036) -> ()  [unwired: 1 in, 2 out]
                      }
                    }
                    n1016 = Replace Array Subset(array=w2031, new element=38, index=w2027) -> (w2029:i32[])
                  }
                }
                n1017 = Equal To 0?(x=w2001) -> (x = 0?=w2000:bool)
                n1018 = Array Size(array=w1996) -> (size(s)=w1995:i32)
                n1019 = And(x=w1999, y=w2000) -> (x .and. y?=w1998:bool)
                n1020 = case shown="True" w1998 {
                  tunnel: w1996 -> [w2005 w2008]
                  tunnel: [w2005 w2007] -> w1997
                  tunnel: w1995 -> [_ w2006]
                  frame False {
                  }
                  frame True {
                    n1021 = for {
                      N: w2006 -> [_]
                      shift-right: [w2009] -> w2007
                      shift-left: w2008 -> [w2012]
                      i -> [w2011]
                      n1022 = Replace Array Subset(array=w2012, new element=37, index=w2011) -> (w2009:i32[])
                    }
                  }
                }
                n1023 = property on="Property Node" class="LstBox (strict)"(reference=w1994, "Item Symbols"=w1997) -> ()  [unwired: 1 in, 2 out]
              }
            }
          }
          event Mouse Down {
            n1024 = event-data() -> ("CtlRef"=w2040:refnum<vi>, "Coords"=w2046:T45)  [unwired: 1 in, 6 out]
            n1025 = invoke on="Invoke Node" class="LstBox (strict)" method="Point To Row"(reference=w2040, "Point"=w2046) -> ("InBounds"=w2041:bool, "Row"=w2042:i32)  [unwired: 5 in, 5 out]
            n1026 = property on="Property Node" class="LstBox (strict)"(reference=w2040) -> ("Item Symbols"=w2045:i32[])  [unwired: 1 in, 2 out]
            n1027 = case shown="True" w2041 {
              tunnel: w2040 -> [_ w2048]
              tunnel: w2045 -> [_ w2056]
              tunnel: w2042 -> [_ w2055]
              frame False {
              }
              frame True {
                n1028 = Index Array(array=w2056, index=w2055) -> (element=w2058:i32)
                n1029 = control-ref of="Thermocouples Selected"() -> (w2047:refnum<vi>)
                n1030 = Equal?(x=w2058, y=37) -> (x = y?=w2053:bool)
                n1031 = case shown="True" w2053 {
                  tunnel: w2056 -> [w2071 w2085]
                  tunnel: w2055 -> [w2068 w2081]
                  tunnel: [w2070 w2083] -> w2050
                  tunnel: w2047 -> [w2069 w2082]
                  frame False {
                    n1032 = Not Equal To 0?(x=w2068) -> (x != 0?=w2067:bool)
                    n1033 = case shown="True" w2067 {
                      tunnel: w2068 -> [_ w2079]
                      tunnel: w2069 -> [_ w2078]
                      frame False {
                      }
                      frame True {
                        n1034 = Number To Decimal String(number=w2079) -> (decimal integer string=w2076:string)  [unwired: 1 in]
                        n1035 = property class="Str"(reference=w2078) -> (reference out=w2077:refnum<vi>, "Text.Text"=w2074:string)  [unwired: 1 in, 1 out]
                        n1036 = call <vilib>:"Space Constant.vi"() -> ("String"=w2075:string)
                        n1037 = Search and Replace String(input string=w2074, search string=w2076, replace string=w2075) -> (result string=w2073:string)  [unwired: 5 in, 3 out]
                        n1038 = property class="Str"(reference=w2077, "Text.Text"=w2073) -> ()  [unwired: 1 in, 2 out]
                      }
                    }
                    n1039 = Replace Array Subset(array=w2071, new element=37, index=w2068) -> (w2070:i32[])
                  }
                  frame True {
                    n1040 = Not Equal To 0?(x=w2081) -> (x != 0?=w2080:bool)
                    n1041 = case shown="True" w2080 {
                      tunnel: w2082 -> [w2086 w2093]
                      tunnel: w2081 -> [_ w2092]
                      frame False {
                        n1042 = property class="Str"(reference=w2086, "Text.Text"="") -> ()  [unwired: 1 in, 2 out]
                      }
                      frame True {
                        n1043 = Number To Decimal String(number=w2092) -> (decimal integer string=w2088:string)  [unwired: 1 in]
                        n1044 = property class="Str"(reference=w2093) -> ("Text.Text"=w2091:string)  [unwired: 1 in, 2 out]
                        n1045 = call <vilib>:"Space Constant.vi"() -> ("String"=w2089:string)
                        n1046 = Concatenate Strings(w2091, w2089, w2088) -> (w2090:string)
                        n1047 = property class="Str"(reference=w2093, "Text.Text"=w2090) -> ()  [unwired: 1 in, 2 out]
                      }
                    }
                    n1048 = Replace Array Subset(array=w2085, new element=38, index=w2081) -> (w2083:i32[])
                  }
                }
                n1049 = Equal To 0?(x=w2055) -> (x = 0?=w2054:bool)
                n1050 = Array Size(array=w2050) -> (size(s)=w2049:i32)
                n1051 = And(x=w2053, y=w2054) -> (x .and. y?=w2052:bool)
                n1052 = case shown="True" w2052 {
                  tunnel: w2050 -> [w2059 w2062]
                  tunnel: [w2059 w2061] -> w2051
                  tunnel: w2049 -> [_ w2060]
                  frame False {
                  }
                  frame True {
                    n1053 = for {
                      N: w2060 -> [_]
                      shift-right: [w2063] -> w2061
                      shift-left: w2062 -> [w2066]
                      i -> [w2065]
                      n1054 = Replace Array Subset(array=w2066, new element=37, index=w2065) -> (w2063:i32[])
                    }
                  }
                }
                n1055 = property on="Property Node" class="LstBox (strict)"(reference=w2048, "Item Symbols"=w2051) -> ()  [unwired: 1 in, 2 out]
              }
            }
          }
          event Mouse Down {
            n1056 = event-data() -> ("CtlRef"=w2094:refnum<vi>, "Coords"=w2100:T45)  [unwired: 1 in, 6 out]
            n1057 = invoke on="Invoke Node" class="LstBox (strict)" method="Point To Row"(reference=w2094, "Point"=w2100) -> ("InBounds"=w2095:bool, "Row"=w2096:i32)  [unwired: 5 in, 5 out]
            n1058 = property on="Property Node" class="LstBox (strict)"(reference=w2094) -> ("Item Symbols"=w2099:i32[])  [unwired: 1 in, 2 out]
            n1059 = case shown="True" w2095 {
              tunnel: w2094 -> [_ w2102]
              tunnel: w2099 -> [_ w2110]
              tunnel: w2096 -> [_ w2109]
              frame False {
              }
              frame True {
                n1060 = Index Array(array=w2110, index=w2109) -> (element=w2112:i32)
                n1061 = control-ref of="Thermocouples Selected"() -> (w2101:refnum<vi>)
                n1062 = Equal?(x=w2112, y=37) -> (x = y?=w2107:bool)
                n1063 = case shown="True" w2107 {
                  tunnel: w2110 -> [w2125 w2139]
                  tunnel: w2109 -> [w2122 w2135]
                  tunnel: [w2124 w2137] -> w2104
                  tunnel: w2101 -> [w2123 w2136]
                  frame False {
                    n1064 = Not Equal To 0?(x=w2122) -> (x != 0?=w2121:bool)
                    n1065 = case shown="True" w2121 {
                      tunnel: w2122 -> [_ w2133]
                      tunnel: w2123 -> [_ w2132]
                      frame False {
                      }
                      frame True {
                        n1066 = Number To Decimal String(number=w2133) -> (decimal integer string=w2130:string)  [unwired: 1 in]
                        n1067 = property class="Str"(reference=w2132) -> (reference out=w2131:refnum<vi>, "Text.Text"=w2128:string)  [unwired: 1 in, 1 out]
                        n1068 = call <vilib>:"Space Constant.vi"() -> ("String"=w2129:string)
                        n1069 = Search and Replace String(input string=w2128, search string=w2130, replace string=w2129) -> (result string=w2127:string)  [unwired: 5 in, 3 out]
                        n1070 = property class="Str"(reference=w2131, "Text.Text"=w2127) -> ()  [unwired: 1 in, 2 out]
                      }
                    }
                    n1071 = Replace Array Subset(array=w2125, new element=37, index=w2122) -> (w2124:i32[])
                  }
                  frame True {
                    n1072 = Not Equal To 0?(x=w2135) -> (x != 0?=w2134:bool)
                    n1073 = case shown="True" w2134 {
                      tunnel: w2136 -> [w2140 w2147]
                      tunnel: w2135 -> [_ w2146]
                      frame False {
                        n1074 = property class="Str"(reference=w2140, "Text.Text"="") -> ()  [unwired: 1 in, 2 out]
                      }
                      frame True {
                        n1075 = Number To Decimal String(number=w2146) -> (decimal integer string=w2142:string)  [unwired: 1 in]
                        n1076 = property class="Str"(reference=w2147) -> ("Text.Text"=w2145:string)  [unwired: 1 in, 2 out]
                        n1077 = call <vilib>:"Space Constant.vi"() -> ("String"=w2143:string)
                        n1078 = Concatenate Strings(w2145, w2143, w2142) -> (w2144:string)
                        n1079 = property class="Str"(reference=w2147, "Text.Text"=w2144) -> ()  [unwired: 1 in, 2 out]
                      }
                    }
                    n1080 = Replace Array Subset(array=w2139, new element=38, index=w2135) -> (w2137:i32[])
                  }
                }
                n1081 = Equal To 0?(x=w2109) -> (x = 0?=w2108:bool)
                n1082 = Array Size(array=w2104) -> (size(s)=w2103:i32)
                n1083 = And(x=w2107, y=w2108) -> (x .and. y?=w2106:bool)
                n1084 = case shown="True" w2106 {
                  tunnel: w2104 -> [w2113 w2116]
                  tunnel: [w2113 w2115] -> w2105
                  tunnel: w2103 -> [_ w2114]
                  frame False {
                  }
                  frame True {
                    n1085 = for {
                      N: w2114 -> [_]
                      shift-right: [w2117] -> w2115
                      shift-left: w2116 -> [w2120]
                      i -> [w2119]
                      n1086 = Replace Array Subset(array=w2120, new element=37, index=w2119) -> (w2117:i32[])
                    }
                  }
                }
                n1087 = property on="Property Node" class="LstBox (strict)"(reference=w2102, "Item Symbols"=w2105) -> ()  [unwired: 1 in, 2 out]
              }
            }
          }
          event Mouse Down {
            n1088 = event-data() -> ("CtlRef"=w2148:refnum<vi>, "Coords"=w2154:T45)  [unwired: 1 in, 6 out]
            n1089 = invoke on="Invoke Node" class="LstBox (strict)" method="Point To Row"(reference=w2148, "Point"=w2154) -> ("InBounds"=w2149:bool, "Row"=w2150:i32)  [unwired: 5 in, 5 out]
            n1090 = property on="Property Node" class="LstBox (strict)"(reference=w2148) -> ("Item Symbols"=w2153:i32[])  [unwired: 1 in, 2 out]
            n1091 = case shown="True" w2149 {
              tunnel: w2148 -> [_ w2156]
              tunnel: w2153 -> [_ w2164]
              tunnel: w2150 -> [_ w2163]
              frame False {
              }
              frame True {
                n1092 = Index Array(array=w2164, index=w2163) -> (element=w2166:i32)
                n1093 = control-ref of="Thermocouples Selected"() -> (w2155:refnum<vi>)
                n1094 = Equal?(x=w2166, y=37) -> (x = y?=w2161:bool)
                n1095 = case shown="True" w2161 {
                  tunnel: w2164 -> [w2179 w2193]
                  tunnel: w2163 -> [w2176 w2189]
                  tunnel: [w2178 w2191] -> w2158
                  tunnel: w2155 -> [w2177 w2190]
                  frame False {
                    n1096 = Not Equal To 0?(x=w2176) -> (x != 0?=w2175:bool)
                    n1097 = case shown="True" w2175 {
                      tunnel: w2176 -> [_ w2187]
                      tunnel: w2177 -> [_ w2186]
                      frame False {
                      }
                      frame True {
                        n1098 = Number To Decimal String(number=w2187) -> (decimal integer string=w2184:string)  [unwired: 1 in]
                        n1099 = property class="Str"(reference=w2186) -> (reference out=w2185:refnum<vi>, "Text.Text"=w2182:string)  [unwired: 1 in, 1 out]
                        n1100 = call <vilib>:"Space Constant.vi"() -> ("String"=w2183:string)
                        n1101 = Search and Replace String(input string=w2182, search string=w2184, replace string=w2183) -> (result string=w2181:string)  [unwired: 5 in, 3 out]
                        n1102 = property class="Str"(reference=w2185, "Text.Text"=w2181) -> ()  [unwired: 1 in, 2 out]
                      }
                    }
                    n1103 = Replace Array Subset(array=w2179, new element=37, index=w2176) -> (w2178:i32[])
                  }
                  frame True {
                    n1104 = Not Equal To 0?(x=w2189) -> (x != 0?=w2188:bool)
                    n1105 = case shown="True" w2188 {
                      tunnel: w2190 -> [w2194 w2201]
                      tunnel: w2189 -> [_ w2200]
                      frame False {
                        n1106 = property class="Str"(reference=w2194, "Text.Text"="") -> ()  [unwired: 1 in, 2 out]
                      }
                      frame True {
                        n1107 = Number To Decimal String(number=w2200) -> (decimal integer string=w2196:string)  [unwired: 1 in]
                        n1108 = property class="Str"(reference=w2201) -> ("Text.Text"=w2199:string)  [unwired: 1 in, 2 out]
                        n1109 = call <vilib>:"Space Constant.vi"() -> ("String"=w2197:string)
                        n1110 = Concatenate Strings(w2199, w2197, w2196) -> (w2198:string)
                        n1111 = property class="Str"(reference=w2201, "Text.Text"=w2198) -> ()  [unwired: 1 in, 2 out]
                      }
                    }
                    n1112 = Replace Array Subset(array=w2193, new element=38, index=w2189) -> (w2191:i32[])
                  }
                }
                n1113 = Equal To 0?(x=w2163) -> (x = 0?=w2162:bool)
                n1114 = Array Size(array=w2158) -> (size(s)=w2157:i32)
                n1115 = And(x=w2161, y=w2162) -> (x .and. y?=w2160:bool)
                n1116 = case shown="True" w2160 {
                  tunnel: w2158 -> [w2167 w2170]
                  tunnel: [w2167 w2169] -> w2159
                  tunnel: w2157 -> [_ w2168]
                  frame False {
                  }
                  frame True {
                    n1117 = for {
                      N: w2168 -> [_]
                      shift-right: [w2171] -> w2169
                      shift-left: w2170 -> [w2174]
                      i -> [w2173]
                      n1118 = Replace Array Subset(array=w2174, new element=37, index=w2173) -> (w2171:i32[])
                    }
                  }
                }
                n1119 = property on="Property Node" class="LstBox (strict)"(reference=w2156, "Item Symbols"=w2159) -> ()  [unwired: 1 in, 2 out]
              }
            }
          }
          event Mouse Down {
            n1120 = event-data() -> ("CtlRef"=w2202:refnum<vi>, "Coords"=w2208:T45)  [unwired: 1 in, 6 out]
            n1121 = invoke on="Invoke Node" class="LstBox (strict)" method="Point To Row"(reference=w2202, "Point"=w2208) -> ("InBounds"=w2203:bool, "Row"=w2204:i32)  [unwired: 5 in, 5 out]
            n1122 = property on="Property Node" class="LstBox (strict)"(reference=w2202) -> ("Item Symbols"=w2207:i32[])  [unwired: 1 in, 2 out]
            n1123 = case shown="True" w2203 {
              tunnel: w2202 -> [_ w2210]
              tunnel: w2207 -> [_ w2218]
              tunnel: w2204 -> [_ w2217]
              frame False {
              }
              frame True {
                n1124 = Index Array(array=w2218, index=w2217) -> (element=w2220:i32)
                n1125 = control-ref of="Thermocouples Selected"() -> (w2209:refnum<vi>)
                n1126 = Equal?(x=w2220, y=37) -> (x = y?=w2215:bool)
                n1127 = case shown="True" w2215 {
                  tunnel: w2218 -> [w2233 w2247]
                  tunnel: w2217 -> [w2230 w2243]
                  tunnel: [w2232 w2245] -> w2212
                  tunnel: w2209 -> [w2231 w2244]
                  frame False {
                    n1128 = Not Equal To 0?(x=w2230) -> (x != 0?=w2229:bool)
                    n1129 = case shown="True" w2229 {
                      tunnel: w2230 -> [_ w2241]
                      tunnel: w2231 -> [_ w2240]
                      frame False {
                      }
                      frame True {
                        n1130 = Number To Decimal String(number=w2241) -> (decimal integer string=w2238:string)  [unwired: 1 in]
                        n1131 = property class="Str"(reference=w2240) -> (reference out=w2239:refnum<vi>, "Text.Text"=w2236:string)  [unwired: 1 in, 1 out]
                        n1132 = call <vilib>:"Space Constant.vi"() -> ("String"=w2237:string)
                        n1133 = Search and Replace String(input string=w2236, search string=w2238, replace string=w2237) -> (result string=w2235:string)  [unwired: 5 in, 3 out]
                        n1134 = property class="Str"(reference=w2239, "Text.Text"=w2235) -> ()  [unwired: 1 in, 2 out]
                      }
                    }
                    n1135 = Replace Array Subset(array=w2233, new element=37, index=w2230) -> (w2232:i32[])
                  }
                  frame True {
                    n1136 = Not Equal To 0?(x=w2243) -> (x != 0?=w2242:bool)
                    n1137 = case shown="True" w2242 {
                      tunnel: w2244 -> [w2248 w2255]
                      tunnel: w2243 -> [_ w2254]
                      frame False {
                        n1138 = property class="Str"(reference=w2248, "Text.Text"="") -> ()  [unwired: 1 in, 2 out]
                      }
                      frame True {
                        n1139 = Number To Decimal String(number=w2254) -> (decimal integer string=w2250:string)  [unwired: 1 in]
                        n1140 = property class="Str"(reference=w2255) -> ("Text.Text"=w2253:string)  [unwired: 1 in, 2 out]
                        n1141 = call <vilib>:"Space Constant.vi"() -> ("String"=w2251:string)
                        n1142 = Concatenate Strings(w2253, w2251, w2250) -> (w2252:string)
                        n1143 = property class="Str"(reference=w2255, "Text.Text"=w2252) -> ()  [unwired: 1 in, 2 out]
                      }
                    }
                    n1144 = Replace Array Subset(array=w2247, new element=38, index=w2243) -> (w2245:i32[])
                  }
                }
                n1145 = Equal To 0?(x=w2217) -> (x = 0?=w2216:bool)
                n1146 = Array Size(array=w2212) -> (size(s)=w2211:i32)
                n1147 = And(x=w2215, y=w2216) -> (x .and. y?=w2214:bool)
                n1148 = case shown="True" w2214 {
                  tunnel: w2212 -> [w2221 w2224]
                  tunnel: [w2221 w2223] -> w2213
                  tunnel: w2211 -> [_ w2222]
                  frame False {
                  }
                  frame True {
                    n1149 = for {
                      N: w2222 -> [_]
                      shift-right: [w2225] -> w2223
                      shift-left: w2224 -> [w2228]
                      i -> [w2227]
                      n1150 = Replace Array Subset(array=w2228, new element=37, index=w2227) -> (w2225:i32[])
                    }
                  }
                }
                n1151 = property on="Property Node" class="LstBox (strict)"(reference=w2210, "Item Symbols"=w2213) -> ()  [unwired: 1 in, 2 out]
              }
            }
          }
          event Mouse Down {
            n1152 = event-data() -> ("CtlRef"=w2256:refnum<vi>, "Coords"=w2262:T45)  [unwired: 1 in, 6 out]
            n1153 = invoke on="Invoke Node" class="LstBox (strict)" method="Point To Row"(reference=w2256, "Point"=w2262) -> ("InBounds"=w2257:bool, "Row"=w2258:i32)  [unwired: 5 in, 5 out]
            n1154 = property on="Property Node" class="LstBox (strict)"(reference=w2256) -> ("Item Symbols"=w2261:i32[])  [unwired: 1 in, 2 out]
            n1155 = case shown="True" w2257 {
              tunnel: w2256 -> [_ w2264]
              tunnel: w2261 -> [_ w2272]
              tunnel: w2258 -> [_ w2271]
              frame False {
              }
              frame True {
                n1156 = Index Array(array=w2272, index=w2271) -> (element=w2274:i32)
                n1157 = control-ref of="Thermocouples Selected"() -> (w2263:refnum<vi>)
                n1158 = Equal?(x=w2274, y=37) -> (x = y?=w2269:bool)
                n1159 = case shown="True" w2269 {
                  tunnel: w2272 -> [w2287 w2301]
                  tunnel: w2271 -> [w2284 w2297]
                  tunnel: [w2286 w2299] -> w2266
                  tunnel: w2263 -> [w2285 w2298]
                  frame False {
                    n1160 = Not Equal To 0?(x=w2284) -> (x != 0?=w2283:bool)
                    n1161 = case shown="True" w2283 {
                      tunnel: w2284 -> [_ w2295]
                      tunnel: w2285 -> [_ w2294]
                      frame False {
                      }
                      frame True {
                        n1162 = Number To Decimal String(number=w2295) -> (decimal integer string=w2292:string)  [unwired: 1 in]
                        n1163 = property class="Str"(reference=w2294) -> (reference out=w2293:refnum<vi>, "Text.Text"=w2290:string)  [unwired: 1 in, 1 out]
                        n1164 = call <vilib>:"Space Constant.vi"() -> ("String"=w2291:string)
                        n1165 = Search and Replace String(input string=w2290, search string=w2292, replace string=w2291) -> (result string=w2289:string)  [unwired: 5 in, 3 out]
                        n1166 = property class="Str"(reference=w2293, "Text.Text"=w2289) -> ()  [unwired: 1 in, 2 out]
                      }
                    }
                    n1167 = Replace Array Subset(array=w2287, new element=37, index=w2284) -> (w2286:i32[])
                  }
                  frame True {
                    n1168 = Not Equal To 0?(x=w2297) -> (x != 0?=w2296:bool)
                    n1169 = case shown="True" w2296 {
                      tunnel: w2298 -> [w2302 w2309]
                      tunnel: w2297 -> [_ w2308]
                      frame False {
                        n1170 = property class="Str"(reference=w2302, "Text.Text"="") -> ()  [unwired: 1 in, 2 out]
                      }
                      frame True {
                        n1171 = Number To Decimal String(number=w2308) -> (decimal integer string=w2304:string)  [unwired: 1 in]
                        n1172 = property class="Str"(reference=w2309) -> ("Text.Text"=w2307:string)  [unwired: 1 in, 2 out]
                        n1173 = call <vilib>:"Space Constant.vi"() -> ("String"=w2305:string)
                        n1174 = Concatenate Strings(w2307, w2305, w2304) -> (w2306:string)
                        n1175 = property class="Str"(reference=w2309, "Text.Text"=w2306) -> ()  [unwired: 1 in, 2 out]
                      }
                    }
                    n1176 = Replace Array Subset(array=w2301, new element=38, index=w2297) -> (w2299:i32[])
                  }
                }
                n1177 = Equal To 0?(x=w2271) -> (x = 0?=w2270:bool)
                n1178 = Array Size(array=w2266) -> (size(s)=w2265:i32)
                n1179 = And(x=w2269, y=w2270) -> (x .and. y?=w2268:bool)
                n1180 = case shown="True" w2268 {
                  tunnel: w2266 -> [w2275 w2278]
                  tunnel: [w2275 w2277] -> w2267
                  tunnel: w2265 -> [_ w2276]
                  frame False {
                  }
                  frame True {
                    n1181 = for {
                      N: w2276 -> [_]
                      shift-right: [w2279] -> w2277
                      shift-left: w2278 -> [w2282]
                      i -> [w2281]
                      n1182 = Replace Array Subset(array=w2282, new element=37, index=w2281) -> (w2279:i32[])
                    }
                  }
                }
                n1183 = property on="Property Node" class="LstBox (strict)"(reference=w2264, "Item Symbols"=w2267) -> ()  [unwired: 1 in, 2 out]
              }
            }
          }
          event Mouse Down {
            n1184 = event-data() -> ("CtlRef"=w2310:refnum<vi>, "Coords"=w2316:T45)  [unwired: 1 in, 6 out]
            n1185 = invoke on="Invoke Node" class="LstBox (strict)" method="Point To Row"(reference=w2310, "Point"=w2316) -> ("InBounds"=w2311:bool, "Row"=w2312:i32)  [unwired: 5 in, 5 out]
            n1186 = property on="Property Node" class="LstBox (strict)"(reference=w2310) -> ("Item Symbols"=w2315:i32[])  [unwired: 1 in, 2 out]
            n1187 = case shown="True" w2311 {
              tunnel: w2310 -> [_ w2318]
              tunnel: w2315 -> [_ w2326]
              tunnel: w2312 -> [_ w2325]
              frame False {
              }
              frame True {
                n1188 = Index Array(array=w2326, index=w2325) -> (element=w2328:i32)
                n1189 = control-ref of="Thermocouples Selected"() -> (w2317:refnum<vi>)
                n1190 = Equal?(x=w2328, y=37) -> (x = y?=w2323:bool)
                n1191 = case shown="True" w2323 {
                  tunnel: w2326 -> [w2341 w2355]
                  tunnel: w2325 -> [w2338 w2351]
                  tunnel: [w2340 w2353] -> w2320
                  tunnel: w2317 -> [w2339 w2352]
                  frame False {
                    n1192 = Not Equal To 0?(x=w2338) -> (x != 0?=w2337:bool)
                    n1193 = case shown="True" w2337 {
                      tunnel: w2338 -> [_ w2349]
                      tunnel: w2339 -> [_ w2348]
                      frame False {
                      }
                      frame True {
                        n1194 = Number To Decimal String(number=w2349) -> (decimal integer string=w2346:string)  [unwired: 1 in]
                        n1195 = property class="Str"(reference=w2348) -> (reference out=w2347:refnum<vi>, "Text.Text"=w2344:string)  [unwired: 1 in, 1 out]
                        n1196 = call <vilib>:"Space Constant.vi"() -> ("String"=w2345:string)
                        n1197 = Search and Replace String(input string=w2344, search string=w2346, replace string=w2345) -> (result string=w2343:string)  [unwired: 5 in, 3 out]
                        n1198 = property class="Str"(reference=w2347, "Text.Text"=w2343) -> ()  [unwired: 1 in, 2 out]
                      }
                    }
                    n1199 = Replace Array Subset(array=w2341, new element=37, index=w2338) -> (w2340:i32[])
                  }
                  frame True {
                    n1200 = Not Equal To 0?(x=w2351) -> (x != 0?=w2350:bool)
                    n1201 = case shown="True" w2350 {
                      tunnel: w2352 -> [w2356 w2363]
                      tunnel: w2351 -> [_ w2362]
                      frame False {
                        n1202 = property class="Str"(reference=w2356, "Text.Text"="") -> ()  [unwired: 1 in, 2 out]
                      }
                      frame True {
                        n1203 = Number To Decimal String(number=w2362) -> (decimal integer string=w2358:string)  [unwired: 1 in]
                        n1204 = property class="Str"(reference=w2363) -> ("Text.Text"=w2361:string)  [unwired: 1 in, 2 out]
                        n1205 = call <vilib>:"Space Constant.vi"() -> ("String"=w2359:string)
                        n1206 = Concatenate Strings(w2361, w2359, w2358) -> (w2360:string)
                        n1207 = property class="Str"(reference=w2363, "Text.Text"=w2360) -> ()  [unwired: 1 in, 2 out]
                      }
                    }
                    n1208 = Replace Array Subset(array=w2355, new element=38, index=w2351) -> (w2353:i32[])
                  }
                }
                n1209 = Equal To 0?(x=w2325) -> (x = 0?=w2324:bool)
                n1210 = Array Size(array=w2320) -> (size(s)=w2319:i32)
                n1211 = And(x=w2323, y=w2324) -> (x .and. y?=w2322:bool)
                n1212 = case shown="True" w2322 {
                  tunnel: w2320 -> [w2329 w2332]
                  tunnel: [w2329 w2331] -> w2321
                  tunnel: w2319 -> [_ w2330]
                  frame False {
                  }
                  frame True {
                    n1213 = for {
                      N: w2330 -> [_]
                      shift-right: [w2333] -> w2331
                      shift-left: w2332 -> [w2336]
                      i -> [w2335]
                      n1214 = Replace Array Subset(array=w2336, new element=37, index=w2335) -> (w2333:i32[])
                    }
                  }
                }
                n1215 = property on="Property Node" class="LstBox (strict)"(reference=w2318, "Item Symbols"=w2321) -> ()  [unwired: 1 in, 2 out]
              }
            }
          }
          event Mouse Down {
            n1216 = event-data() -> ("CtlRef"=w2364:refnum<vi>, "Coords"=w2370:T45)  [unwired: 1 in, 6 out]
            n1217 = invoke on="Invoke Node" class="LstBox (strict)" method="Point To Row"(reference=w2364, "Point"=w2370) -> ("InBounds"=w2365:bool, "Row"=w2366:i32)  [unwired: 5 in, 5 out]
            n1218 = property on="Property Node" class="LstBox (strict)"(reference=w2364) -> ("Item Symbols"=w2369:i32[])  [unwired: 1 in, 2 out]
            n1219 = case shown="True" w2365 {
              tunnel: w2364 -> [_ w2372]
              tunnel: w2369 -> [_ w2380]
              tunnel: w2366 -> [_ w2379]
              frame False {
              }
              frame True {
                n1220 = Index Array(array=w2380, index=w2379) -> (element=w2382:i32)
                n1221 = control-ref of="Thermocouples Selected"() -> (w2371:refnum<vi>)
                n1222 = Equal?(x=w2382, y=37) -> (x = y?=w2377:bool)
                n1223 = case shown="True" w2377 {
                  tunnel: w2380 -> [w2395 w2409]
                  tunnel: w2379 -> [w2392 w2405]
                  tunnel: [w2394 w2407] -> w2374
                  tunnel: w2371 -> [w2393 w2406]
                  frame False {
                    n1224 = Not Equal To 0?(x=w2392) -> (x != 0?=w2391:bool)
                    n1225 = case shown="True" w2391 {
                      tunnel: w2392 -> [_ w2403]
                      tunnel: w2393 -> [_ w2402]
                      frame False {
                      }
                      frame True {
                        n1226 = Number To Decimal String(number=w2403) -> (decimal integer string=w2400:string)  [unwired: 1 in]
                        n1227 = property class="Str"(reference=w2402) -> (reference out=w2401:refnum<vi>, "Text.Text"=w2398:string)  [unwired: 1 in, 1 out]
                        n1228 = call <vilib>:"Space Constant.vi"() -> ("String"=w2399:string)
                        n1229 = Search and Replace String(input string=w2398, search string=w2400, replace string=w2399) -> (result string=w2397:string)  [unwired: 5 in, 3 out]
                        n1230 = property class="Str"(reference=w2401, "Text.Text"=w2397) -> ()  [unwired: 1 in, 2 out]
                      }
                    }
                    n1231 = Replace Array Subset(array=w2395, new element=37, index=w2392) -> (w2394:i32[])
                  }
                  frame True {
                    n1232 = Not Equal To 0?(x=w2405) -> (x != 0?=w2404:bool)
                    n1233 = case shown="True" w2404 {
                      tunnel: w2406 -> [w2410 w2417]
                      tunnel: w2405 -> [_ w2416]
                      frame False {
                        n1234 = property class="Str"(reference=w2410, "Text.Text"="") -> ()  [unwired: 1 in, 2 out]
                      }
                      frame True {
                        n1235 = Number To Decimal String(number=w2416) -> (decimal integer string=w2412:string)  [unwired: 1 in]
                        n1236 = property class="Str"(reference=w2417) -> ("Text.Text"=w2415:string)  [unwired: 1 in, 2 out]
                        n1237 = call <vilib>:"Space Constant.vi"() -> ("String"=w2413:string)
                        n1238 = Concatenate Strings(w2415, w2413, w2412) -> (w2414:string)
                        n1239 = property class="Str"(reference=w2417, "Text.Text"=w2414) -> ()  [unwired: 1 in, 2 out]
                      }
                    }
                    n1240 = Replace Array Subset(array=w2409, new element=38, index=w2405) -> (w2407:i32[])
                  }
                }
                n1241 = Equal To 0?(x=w2379) -> (x = 0?=w2378:bool)
                n1242 = Array Size(array=w2374) -> (size(s)=w2373:i32)
                n1243 = And(x=w2377, y=w2378) -> (x .and. y?=w2376:bool)
                n1244 = case shown="True" w2376 {
                  tunnel: w2374 -> [w2383 w2386]
                  tunnel: [w2383 w2385] -> w2375
                  tunnel: w2373 -> [_ w2384]
                  frame False {
                  }
                  frame True {
                    n1245 = for {
                      N: w2384 -> [_]
                      shift-right: [w2387] -> w2385
                      shift-left: w2386 -> [w2390]
                      i -> [w2389]
                      n1246 = Replace Array Subset(array=w2390, new element=37, index=w2389) -> (w2387:i32[])
                    }
                  }
                }
                n1247 = property on="Property Node" class="LstBox (strict)"(reference=w2372, "Item Symbols"=w2375) -> ()  [unwired: 1 in, 2 out]
              }
            }
          }
          event Mouse Down {
            n1248 = event-data() -> ("CtlRef"=w2418:refnum<vi>, "Coords"=w2424:T45)  [unwired: 1 in, 6 out]
            n1249 = invoke on="Invoke Node" class="LstBox (strict)" method="Point To Row"(reference=w2418, "Point"=w2424) -> ("InBounds"=w2419:bool, "Row"=w2420:i32)  [unwired: 5 in, 5 out]
            n1250 = property on="Property Node" class="LstBox (strict)"(reference=w2418) -> ("Item Symbols"=w2423:i32[])  [unwired: 1 in, 2 out]
            n1251 = case shown="True" w2419 {
              tunnel: w2418 -> [_ w2426]
              tunnel: w2423 -> [_ w2434]
              tunnel: w2420 -> [_ w2433]
              frame False {
              }
              frame True {
                n1252 = Index Array(array=w2434, index=w2433) -> (element=w2436:i32)
                n1253 = control-ref of="Thermocouples Selected"() -> (w2425:refnum<vi>)
                n1254 = Equal?(x=w2436, y=37) -> (x = y?=w2431:bool)
                n1255 = case shown="True" w2431 {
                  tunnel: w2434 -> [w2449 w2463]
                  tunnel: w2433 -> [w2446 w2459]
                  tunnel: [w2448 w2461] -> w2428
                  tunnel: w2425 -> [w2447 w2460]
                  frame False {
                    n1256 = Not Equal To 0?(x=w2446) -> (x != 0?=w2445:bool)
                    n1257 = case shown="True" w2445 {
                      tunnel: w2446 -> [_ w2457]
                      tunnel: w2447 -> [_ w2456]
                      frame False {
                      }
                      frame True {
                        n1258 = Number To Decimal String(number=w2457) -> (decimal integer string=w2454:string)  [unwired: 1 in]
                        n1259 = property class="Str"(reference=w2456) -> (reference out=w2455:refnum<vi>, "Text.Text"=w2452:string)  [unwired: 1 in, 1 out]
                        n1260 = call <vilib>:"Space Constant.vi"() -> ("String"=w2453:string)
                        n1261 = Search and Replace String(input string=w2452, search string=w2454, replace string=w2453) -> (result string=w2451:string)  [unwired: 5 in, 3 out]
                        n1262 = property class="Str"(reference=w2455, "Text.Text"=w2451) -> ()  [unwired: 1 in, 2 out]
                      }
                    }
                    n1263 = Replace Array Subset(array=w2449, new element=37, index=w2446) -> (w2448:i32[])
                  }
                  frame True {
                    n1264 = Not Equal To 0?(x=w2459) -> (x != 0?=w2458:bool)
                    n1265 = case shown="True" w2458 {
                      tunnel: w2460 -> [w2464 w2471]
                      tunnel: w2459 -> [_ w2470]
                      frame False {
                        n1266 = property class="Str"(reference=w2464, "Text.Text"="") -> ()  [unwired: 1 in, 2 out]
                      }
                      frame True {
                        n1267 = Number To Decimal String(number=w2470) -> (decimal integer string=w2466:string)  [unwired: 1 in]
                        n1268 = property class="Str"(reference=w2471) -> ("Text.Text"=w2469:string)  [unwired: 1 in, 2 out]
                        n1269 = call <vilib>:"Space Constant.vi"() -> ("String"=w2467:string)
                        n1270 = Concatenate Strings(w2469, w2467, w2466) -> (w2468:string)
                        n1271 = property class="Str"(reference=w2471, "Text.Text"=w2468) -> ()  [unwired: 1 in, 2 out]
                      }
                    }
                    n1272 = Replace Array Subset(array=w2463, new element=38, index=w2459) -> (w2461:i32[])
                  }
                }
                n1273 = Equal To 0?(x=w2433) -> (x = 0?=w2432:bool)
                n1274 = Array Size(array=w2428) -> (size(s)=w2427:i32)
                n1275 = And(x=w2431, y=w2432) -> (x .and. y?=w2430:bool)
                n1276 = case shown="True" w2430 {
                  tunnel: w2428 -> [w2437 w2440]
                  tunnel: [w2437 w2439] -> w2429
                  tunnel: w2427 -> [_ w2438]
                  frame False {
                  }
                  frame True {
                    n1277 = for {
                      N: w2438 -> [_]
                      shift-right: [w2441] -> w2439
                      shift-left: w2440 -> [w2444]
                      i -> [w2443]
                      n1278 = Replace Array Subset(array=w2444, new element=37, index=w2443) -> (w2441:i32[])
                    }
                  }
                }
                n1279 = property on="Property Node" class="LstBox (strict)"(reference=w2426, "Item Symbols"=w2429) -> ()  [unwired: 1 in, 2 out]
              }
            }
          }
          event "Export Errors": Mouse Down {
            n1280 = event-data() -> ()  [unwired: 1 in, 1 out]
            n1281 = Unbundle By Name(w2475) -> ("MasterErrorArray"=w2472:string[][])
            n1282 = call-poly <vilib>:"Write Delimited Spreadsheet.vi"("2D data"=w2472, "error in (no error)"=w2474) -> ("error out"=w2473:errorcluster)  [unwired: 12 in, 1 out]
          }
          event "Export Events": Mouse Down {
            n1283 = event-data() -> ()  [unwired: 1 in, 1 out]
            n1284 = Unbundle By Name(w2479) -> ("MasterEventArray"=w2476:string[][])
            n1285 = call-poly <vilib>:"Write Delimited Spreadsheet.vi"("2D data"=w2476, "error in (no error)"=w2478) -> ("error out"=w2477:errorcluster)  [unwired: 12 in, 1 out]
          }
          event "Database Logging On/Off": Mouse Down {
            n1286 = event-data() -> ("CtlRef"=w2481:refnum<vi>)  [unwired: 1 in, 7 out]
            n1287 = Unbundle By Name(w2482) -> ("Http session"=w2487:T30, "URL prefex"=w2486:string)
            n1288 = property class="Bool (strict)"(reference=w2481) -> ("Value"=w2480:bool)  [unwired: 1 in, 2 out]
            n1289 = case shown="True" w2480 {
              tunnel: w2485 -> [w2490 w2497]
              tunnel: w2487 -> [w2491 w2498]
              tunnel: w2486 -> [w2492 w2500]
              tunnel: [w2489 w2496] -> w2484
              tunnel: [w2488 w2495] -> w2483
              frame False {
                n1290 = Concatenate Strings(w2492, "StoprecordData" ("string")) -> (w2494:string)
                n1291 = call <vilib>:"GET.vi"("client handle"=w2491, "url"=w2494, "error in (no error)"=w2490) -> ("client handle out"=w2488:T30, "error out"=w2489:errorcluster)  [unwired: 9 in, 2 out]
              }
              frame True {
                n1292 = Concatenate Strings(w2500, "recordData" ("string")) -> (w2501:string)
                n1293 = call <vilib>:"GET.vi"("client handle"=w2498, "url"=w2501, "error in (no error)"=w2497) -> ("client handle out"=w2495:T30, "error out"=w2496:errorcluster)  [unwired: 9 in, 2 out]
              }
            }
            n1294 = Bundle By Name(cluster=w2482, "Http session"=w2483) -> ()  [unwired: 1 out]
          }
          event "Import UUT": Mouse Down {
            n1295 = event-data() -> ()  [unwired: 1 in, 1 out]
            n1296 = call "File Dialog"("prompt"="Select a new image for the UUT", "error in"=w2512, "pattern (all files)"="*.png;*.jpg;*.JPEG") -> ("selected path"=w2506:path, "error out"=w2510:errorcluster)  [unwired: 9 in, 2 out]
            n1297 = Path To String(path=w2506) -> (string=w2505:string)
            n1298 = local write "Path to PNG file"(w2506) -> ()
            n1299 = Match Pattern(string=w2505, regular expression="png") -> (match substring=w2503:string)  [unwired: 1 in, 3 out]
            n1300 = Empty String/Path?(string/path=w2503) -> (empty?=w2502:bool)
            n1301 = case shown="False" w2502 {
              tunnel: [w2520 w2525] -> w2511
              tunnel: w2510 -> [w2519 w2522]
              tunnel: [w2518 w2523] -> w2509
              tunnel: w2506 -> [w2516 w2521]
              frame False {
                n1302 = call <vilib>:"Read PNG File.vi"("error in (no error)"=w2519, "path to PNG file"=w2516) -> ("error out"=w2518:errorcluster, "image data"=w2517:T44)  [unwired: 7 in, 1 out]
                n1303 = call <vilib>:"Draw Flattened Pixmap.vi"("image data"=w2517) -> ("new picture"=w2520:picture)  [unwired: 8 in]
              }
              frame True {
                n1304 = call <vilib>:"Read JPEG File.vi"("error in (no error)"=w2522, "path to JPEG file"=w2521) -> ("error out"=w2523:errorcluster, "image data"=w2524:T44)  [unwired: 7 in, 1 out]
                n1305 = call <vilib>:"Draw Flattened Pixmap.vi"("image data"=w2524) -> ("new picture"=w2525:picture)  [unwired: 8 in]
              }
            }
            n1306 = local read "TC1to75visual"() -> (w2507:T9)
            n1307 = Bundle By Name(cluster=w2507, "new picture"=w2511) -> (w2508:T9)
            n1308 = local write "TC1to75visual"(w2508) -> ()
          }
          event "Query Database": Mouse Down {
            w2532 = TRUE ("UTC format")
            w2536 = "%Y-%m-%d %H:%M:%S" ("time format string (%c)")
            w2540 = "\"" ("string")
            w2542 = "\"" ("string")
            n1309 = event-data() -> ()  [unwired: 1 in, 1 out]
            n1310 = local read "TVAC Labview"() -> (w2545:bool)
            n1311 = Cluster To Array(cluster="Query Expected Temperatures") -> (array=w2526:bool[])
            n1312 = Cluster To Array(cluster="Query Specific Gauge Pressures") -> (array=w2530:bool[])
            n1313 = Cluster To Array(cluster="Query Thermocouples Selection") -> (array=w2528:bool[])
            n1314 = case shown="True" w2545 {
              tunnel: [path "C:/Users/stefan/AppData/Local/conda/conda/envs/py35/python.exe" ("Path to Python.exe") path "C:/Users/TVAC-admin/AppData/Local/Programs/Python/Python35/python.exe" ("Path to Python.exe")] -> w2546
              frame False {
              }
              frame True {
              }
            }
            n1315 = Format Date/Time String(time format string (%c)=w2536, seconds (now)="End Time UTC", UTC format=w2532) -> (date/time string=w2541:string)
            n1316 = Format Date/Time String(time format string (%c)=w2536, seconds (now)="Start Time UTC", UTC format=w2532) -> (date/time string=w2543:string)
            n1317 = local read "Select Path and Check Save Before Pressing Query"() -> (w2533:path)
            n1318 = Concatenate Strings(w2540, w2541, w2540) -> (w2537:string)
            n1319 = Concatenate Strings(w2542, w2543, w2542) -> (w2538:string)
            n1320 = local read "Save Results"() -> (w2534:bool)
            n1321 = call "lvHistoricalQuery.vi"("Path to Python.exe"=w2546, "startTime"=w2538, "endTime"=w2537, "error in (no error)"=w2547, "gaugeselection"=w2530, "Path"=w2533, "SaveData"=w2534, "tcselection"=w2528, "expected"=w2526) -> ("error out"=w2535:errorcluster)  [unwired: 9 in, 1 out]
          }
          event "Vacuum Commands.Vacuum State": Mouse Down {
            n1322 = event-data() -> ("CtlRef"=w2555:refnum<vi>)  [unwired: 1 in, 3 out]
            n1323 = property class="Bool (strict)"(reference=w2555) -> ("Value"=w2554:bool)  [unwired: 1 in, 2 out]
            n1324 = Select(t="putUnderVacuum" ("string"), s=w2554, f="VacuumNotNeeded" ("string")) -> (s? t:f=w2551:string)
            n1325 = Unbundle By Name(w2566) -> ("Http session"=w2567:T30, "URL prefex"=w2562:string)
            n1326 = Concatenate Strings(w2562, w2551) -> (w2561:string)
            n1327 = call <vilib>:"GET.vi"("client handle"=w2567, "url"=w2561, "error in (no error)"=w2569) -> ("client handle out"=w2564:T30, "body"=w2558:string, "error out"=w2568:errorcluster)  [unwired: 9 in, 1 out]
            n1328 = Match True/False String(2:"" ("false string"), 3:"{'result':'success'}" ("true string"), 4:w2558) -> (0:w2560:bool)  [unwired: 1 out]
            n1329 = Bundle By Name(cluster=w2566, "Http session"=w2564) -> (w2565:T31)
            n1330 = Select(t="Vacuum State Change Initated" ("true string"), s=w2560, f=w2558) -> (s? t:f=w2557:string)
            n1331 = One Button Dialog(message=w2557) -> ()  [unwired: 1 in, 1 out]
          }
          event "Vacuum Commands.Start Heating Shroud": Value Change {
            n1332 = event-data() -> ("NewVal"=w2578:bool)  [unwired: 1 in, 5 out]
            n1333 = control-ref of="LN2 Heater - Shroud Duty Cycle %"() -> (w2594:refnum<vi>)
            n1334 = property class="DigNum (strict)"(reference=w2594) -> ("Value"=w2589:dbl[unit])  [unwired: 1 in, 2 out]
            n1335 = Divide(x=w2589, y=dbl[unit] 100.0) -> (x/y=w2577:dbl)
            n1336 = Select(t=w2577, s=w2578, f=0.0) -> (s? t:f=w2575:dbl)
            n1337 = Bundle By Name(cluster=cluster{"dutyCycle":dbl} {"dutyCycle"=0.0}, "dutyCycle"=w2575) -> (w2590:cluster{"dutyCycle":dbl})
            n1338 = Unbundle By Name(w2586) -> ("Http session"=w2593:T30, "URL prefex"=w2592:string)
            n1339 = Flatten To JSON(anything=w2590, error in (no error)=w2587) -> (JSON string=w2580:string, 11:w2583:errorcluster)  [unwired: 1 in]
            n1340 = Concatenate Strings(w2592, "heatUpShroud" ("string")) -> (w2581:string)
            n1341 = call-poly <vilib>:"POST.vi"("client handle"=w2593, "url"=w2581, "buffer"=w2580, "error in (no error)"=w2583) -> ("client handle out"=w2584:T30, "body"=w2571:string, "error out"=w2582:errorcluster)  [unwired: 8 in, 1 out]
            n1342 = local read "UTC"() -> (w2573:string)
            n1343 = Bundle By Name(cluster=w2586, "Http session"=w2584) -> (w2585:T31)
            n1344 = Concatenate Strings(w2573, " UTC ", w2571) -> (w2572:string)
            n1345 = control-ref of="Last Response"() -> (w2574:refnum<vi>)
            n1346 = property class="Str"(reference=w2574, "Text.Text"=w2572) -> ()  [unwired: 1 in, 2 out]
          }
          event "Vacuum Commands.Start Heating Platen": Value Change {
            n1347 = event-data() -> ("NewVal"=w2602:bool)  [unwired: 1 in, 5 out]
            n1348 = control-ref of="LN2 Heater - Platen Duty Cycle %"() -> (w2619:refnum<vi>)
            n1349 = property class="DigNum (strict)"(reference=w2619) -> ("Value"=w2614:dbl[unit])  [unwired: 1 in, 2 out]
            n1350 = Divide(x=w2614, y=dbl[unit] 100.0) -> (x/y=w2603:dbl)
            n1351 = Select(t=w2603, s=w2602, f=0.0) -> (s? t:f=w2600:dbl)
            n1352 = Bundle By Name(cluster=cluster{"dutyCycle":dbl} {"dutyCycle"=0.0}, "dutyCycle"=w2600) -> (w2615:cluster{"dutyCycle":dbl})
            n1353 = Unbundle By Name(w2611) -> ("Http session"=w2618:T30, "URL prefex"=w2617:string)
            n1354 = Flatten To JSON(anything=w2615, error in (no error)=w2612) -> (JSON string=w2605:string, 11:w2608:errorcluster)  [unwired: 1 in]
            n1355 = Concatenate Strings(w2617, "heatUpPlaten" ("string")) -> (w2606:string)
            n1356 = call-poly <vilib>:"POST.vi"("client handle"=w2618, "url"=w2606, "buffer"=w2605, "error in (no error)"=w2608) -> ("client handle out"=w2609:T30, "body"=w2596:string, "error out"=w2607:errorcluster)  [unwired: 8 in, 1 out]
            n1357 = local read "UTC"() -> (w2599:string)
            n1358 = Bundle By Name(cluster=w2611, "Http session"=w2609) -> (w2610:T31)
            n1359 = Concatenate Strings(w2599, " UTC " ("string"), w2596) -> (w2597:string)
            n1360 = control-ref of="Last Response"() -> (w2598:refnum<vi>)
            n1361 = property class="Str"(reference=w2598, "Text.Text"=w2597) -> ()  [unwired: 1 in, 2 out]
          }
          event "Vacuum Commands.Stop Cryopumping\n(Vacuum Not Maintained)": Mouse Down {
            n1362 = event-data() -> ()  [unwired: 1 in, 1 out]
            n1363 = Unbundle By Name(w2633) -> ("Http session"=w2635:T30, "URL prefex"=w2634:string)
            n1364 = Concatenate Strings(w2634, "StopCryoPumpingChamber" ("string")) -> (w2629:string)
            n1365 = call <vilib>:"GET.vi"("client handle"=w2635, "url"=w2629, "error in (no error)"=w2627) -> ("client handle out"=w2631:T30, "body"=w2622:string, "error out"=w2630:errorcluster)  [unwired: 9 in, 1 out]
            n1366 = Bundle By Name(cluster=w2633, "Http session"=w2631) -> (w2632:T31)
            n1367 = Match True/False String(2:"" ("false string"), 3:"{'result':'success'}" ("true string"), 4:w2622) -> (0:w2625:bool, 1:w2620:string)
            n1368 = Select(t="Gate Valve Closed, Cryopump Not Maintaining Vacuum" ("true string"), s=w2625, f=w2620) -> (s? t:f=w2623:string)
            n1369 = One Button Dialog(message=w2623) -> ()  [unwired: 1 in, 1 out]
          }
          event "Vacuum Commands.Stop Pumping and Shut Off Cryopump": Mouse Down {
            n1370 = event-data() -> ()  [unwired: 1 in, 2 out]
            n1371 = Unbundle By Name(w2649) -> ("Http session"=w2651:T30, "URL prefex"=w2650:string)
            n1372 = Concatenate Strings(w2650, "StopCryoPump" ("string")) -> (w2645:string)
            n1373 = call <vilib>:"GET.vi"("client handle"=w2651, "url"=w2645, "error in (no error)"=w2643) -> ("client handle out"=w2647:T30, "body"=w2636:string, "error out"=w2646:errorcluster)  [unwired: 9 in, 1 out]
            n1374 = Bundle By Name(cluster=w2649, "Http session"=w2647) -> (w2648:T31)
            n1375 = Match True/False String(2:"" ("false string"), 3:"{'result':'success'}" ("true string"), 4:w2636) -> (0:w2641:bool, 1:w2637:string)
            n1376 = Select(t="Shutdown of Cryopump Initated" ("true string"), s=w2641, f=w2637) -> (s? t:f=w2639:string)
            n1377 = One Button Dialog(message=w2639) -> ()  [unwired: 1 in, 1 out]
          }
          event "Vacuum Commands.Stop Roughing Pump": Mouse Down {
            n1378 = event-data() -> ()  [unwired: 1 in, 2 out]
            n1379 = Unbundle By Name(w2665) -> ("Http session"=w2667:T30, "URL prefex"=w2666:string)
            n1380 = Concatenate Strings(w2666, "StopRoughingPump" ("string")) -> (w2661:string)
            n1381 = call <vilib>:"GET.vi"("client handle"=w2667, "url"=w2661, "error in (no error)"=w2659) -> ("client handle out"=w2663:T30, "body"=w2652:string, "error out"=w2662:errorcluster)  [unwired: 9 in, 1 out]
            n1382 = Bundle By Name(cluster=w2665, "Http session"=w2663) -> (w2664:T31)
            n1383 = Match True/False String(2:"" ("false string"), 3:"{'result':'success'}" ("true string"), 4:w2652) -> (0:w2657:bool, 1:w2653:string)
            n1384 = Select(t="Roughing Pump Stopping" ("true string"), s=w2657, f=w2653) -> (s? t:f=w2655:string)
            n1385 = One Button Dialog(message=w2655) -> ()  [unwired: 1 in, 1 out]
          }
          event "exit": Value Change {
            n1386 = event-data() -> ()  [unwired: 1 in, 1 out]
            n1387 = call "Broadcast Message.vi"("error in (no error)"=w2670, "event"="exit") -> ("error out"=w2668:errorcluster)  [unwired: 9 in]
          }
        }
        n1388 = Get Date/Time In Seconds() -> (seconds since 1Jan1904=w396:timestamp)
        n1389 = Get Date/Time String(seconds (now)=w396, want seconds? (F)=w395) -> (time string=→"Local Time":string)  [unwired: 1 in, 1 out]
        n1390 = Format Date/Time String(time format string (%c)="%H:%M:%S", seconds (now)=w396, UTC format=w395) -> (date/time string=→"UTC":string)
      }
      frame "compileProfile" {
        n1391 = Empty String/Path?(string/path=w2692) -> (empty?=w2694:bool)
        n1392 = case shown="False" w2694 {
          tunnel: [w2734 0.0] -> w2693
          tunnel: w2692 -> [w2738 _]
          frame False {
            n1393 = Equal?(x=w2738, y="2") -> (x = y?=w2736:bool)
            n1394 = case shown="True" w2736 {
              tunnel: 1.0 -> [w2739 w2741]
              tunnel: [w2739 w2740] -> w2734
              frame False {
              }
              frame True {
                n1395 = local read "importexe"() -> (w2743:dbl)
                n1396 = Equal?(x=w2743, y=2.0) -> (x = y?=w2744:bool)
                n1397 = case shown="True" w2744 {
                  tunnel: w2741 -> [_ w2746]
                  tunnel: [0.0 w2746] -> w2740
                  frame False {
                  }
                  frame True {
                    n1398 = local write "importexe"(0.0 ("importexe")) -> ()
                  }
                }
              }
            }
          }
          frame True {
          }
        }
        n1399 = local write "ThermalProfileStatus"("Compiling..........." ("String")) -> ()
        n1400 = Unbundle By Name(w2729) -> ("ZonesSelected"=w2730:bool[], "ZoneSetup.Number of Set points"=w2728:dbl)
        n1401 = Initialize Array(T36 {"zone"=0, "average"="", "thermocouples"=[0], "maxTemp"=0, "minTemp"=0, "maxSlope"=0.0, "thermalprofiles"=[{"thermalsetpoint"=0, "tempgoal"=0, "ramp"=0, "soakduration"=0}]} ("ThermalProfileCluster.profiles"), 1 ("dimension size")) -> (w2727:T47)
        n1402 = for {
          N: 9 -> [_]
          tunnel: w2729 -> [w2907]
          tunnel: w2730 -> [w2906] mode=indexing
          shift-right: [w2904] -> w2703
          shift-left: w2729 -> [w2905]
          tunnel: w2728 -> [w2900]
          shift-right: [w2898] -> w2724
          shift-left: w2727 -> [w2899]
          shift-right: [w2896] -> w2674
          shift-left: w2675 -> [w2896]
          i -> [w2897]
          w2903 = 0  # zone
          n1403 = Add(x=w2903, y=w2897) -> (x+y=w2902:i32)
          n1404 = Increment(x=w2902) -> (x+1=w2901:i32)
          n1405 = case shown="True" w2906 {
            tunnel: w2907 -> [_ _]
            tunnel: w2897 -> [_ w2942]
            tunnel: w2905 -> [w2909 w2946]
            tunnel: [w2909 w2946] -> w2904
            tunnel: w2901 -> [_ w2947]
            tunnel: w2900 -> [_ w2910]
            tunnel: w2899 -> [w2908 w2919]
            tunnel: [w2908 w2918] -> w2898
            tunnel: w2897 -> [_ _]
            frame False {
            }
            frame True {
              n1406 = case shown="7" w2942 {
                tunnel: [w2981 w2987 w2993 w2999 w3005 w3011 w3017 w3023 w3029] -> w2938
                tunnel: [w2980 w2986 w2992 w2998 w3004 w3010 w3016 w3022 w3028] -> w2941
                tunnel: [w2979 w2985 w2991 w2997 w3003 w3009 w3015 w3021 w3027] -> w2933
                tunnel: [w2978 w2984 w2990 w2996 w3002 w3008 w3014 w3020 w3026] -> w2929
                tunnel: [w2977 w2983 w2989 w2995 w3001 w3007 w3013 w3019 w3025] -> w2928
                tunnel: [w2976 w2982 w2988 w2994 w3000 w3006 w3012 w3018 w3024] -> w2924
                frame 0, Default {
                  n1407 = control-ref of="Zone Thermocouples"() -> (w2981:refnum<vi>)
                  n1408 = control-ref of="Temperature Goal"() -> (w2979:refnum<vi>)
                  n1409 = control-ref of="Max Temp Slope (K/min)"() -> (w2976:refnum<vi>)
                  n1410 = control-ref of="Max Allowable Temp"() -> (w2978:refnum<vi>)
                  n1411 = control-ref of="Temperature Calculation"() -> (w2980:refnum<vi>)
                  n1412 = control-ref of="Min Allowable Temp"() -> (w2977:refnum<vi>)
                }
                frame 1 {
                  n1413 = control-ref of="Zone Thermocouples"() -> (w2987:refnum<vi>)
                  n1414 = control-ref of="Max Temp Slope (K/min)"() -> (w2982:refnum<vi>)
                  n1415 = control-ref of="Temperature Goal"() -> (w2985:refnum<vi>)
                  n1416 = control-ref of="Max Allowable Temp"() -> (w2984:refnum<vi>)
                  n1417 = control-ref of="Temperature Calculation"() -> (w2986:refnum<vi>)
                  n1418 = control-ref of="Min Allowable Temp"() -> (w2983:refnum<vi>)
                }
                frame 2 {
                  n1419 = control-ref of="Zone Thermocouples"() -> (w2993:refnum<vi>)
                  n1420 = control-ref of="Max Temp Slope (K/min)"() -> (w2988:refnum<vi>)
                  n1421 = control-ref of="Temperature Goal"() -> (w2991:refnum<vi>)
                  n1422 = control-ref of="Max Allowable Temp"() -> (w2990:refnum<vi>)
                  n1423 = control-ref of="Temperature Calculation"() -> (w2992:refnum<vi>)
                  n1424 = control-ref of="Min Allowable Temp"() -> (w2989:refnum<vi>)
                }
                frame 3 {
                  n1425 = control-ref of="Zone Thermocouples"() -> (w2999:refnum<vi>)
                  n1426 = control-ref of="Max Temp Slope (K/min)"() -> (w2994:refnum<vi>)
                  n1427 = control-ref of="Temperature Goal"() -> (w2997:refnum<vi>)
                  n1428 = control-ref of="Max Allowable Temp"() -> (w2996:refnum<vi>)
                  n1429 = control-ref of="Temperature Calculation"() -> (w2998:refnum<vi>)
                  n1430 = control-ref of="Min Allowable Temp"() -> (w2995:refnum<vi>)
                }
                frame 4 {
                  n1431 = control-ref of="Zone Thermocouples"() -> (w3005:refnum<vi>)
                  n1432 = control-ref of="Max Temp Slope (K/min)"() -> (w3000:refnum<vi>)
                  n1433 = control-ref of="Temperature Goal"() -> (w3003:refnum<vi>)
                  n1434 = control-ref of="Max Allowable Temp"() -> (w3002:refnum<vi>)
                  n1435 = control-ref of="Temperature Calculation"() -> (w3004:refnum<vi>)
                  n1436 = control-ref of="Min Allowable Temp"() -> (w3001:refnum<vi>)
                }
                frame 5 {
                  n1437 = control-ref of="Zone Thermocouples"() -> (w3011:refnum<vi>)
                  n1438 = control-ref of="Max Temp Slope (K/min)"() -> (w3006:refnum<vi>)
                  n1439 = control-ref of="Temperature Goal"() -> (w3009:refnum<vi>)
                  n1440 = control-ref of="Max Allowable Temp"() -> (w3008:refnum<vi>)
                  n1441 = control-ref of="Temperature Calculation"() -> (w3010:refnum<vi>)
                  n1442 = control-ref of="Min Allowable Temp"() -> (w3007:refnum<vi>)
                }
                frame 6 {
                  n1443 = control-ref of="Zone Thermocouples"() -> (w3017:refnum<vi>)
                  n1444 = control-ref of="Temperature Goal"() -> (w3015:refnum<vi>)
                  n1445 = control-ref of="Max Temp Slope (K/min)"() -> (w3012:refnum<vi>)
                  n1446 = control-ref of="Max Allowable Temp"() -> (w3014:refnum<vi>)
                  n1447 = control-ref of="Temperature Calculation"() -> (w3016:refnum<vi>)
                  n1448 = control-ref of="Min Allowable Temp"() -> (w3013:refnum<vi>)
                }
                frame 7 {
                  n1449 = control-ref of="Zone Thermocouples"() -> (w3023:refnum<vi>)
                  n1450 = control-ref of="Temperature Goal"() -> (w3021:refnum<vi>)
                  n1451 = control-ref of="Max Temp Slope (K/min)"() -> (w3018:refnum<vi>)
                  n1452 = control-ref of="Max Allowable Temp"() -> (w3020:refnum<vi>)
                  n1453 = control-ref of="Temperature Calculation"() -> (w3022:refnum<vi>)
                  n1454 = control-ref of="Min Allowable Temp"() -> (w3019:refnum<vi>)
                }
                frame 8 {
                  n1455 = control-ref of="Zone Thermocouples"() -> (w3029:refnum<vi>)
                  n1456 = control-ref of="Temperature Goal"() -> (w3027:refnum<vi>)
                  n1457 = control-ref of="Max Temp Slope (K/min)"() -> (w3024:refnum<vi>)
                  n1458 = control-ref of="Max Allowable Temp"() -> (w3026:refnum<vi>)
                  n1459 = control-ref of="Temperature Calculation"() -> (w3028:refnum<vi>)
                  n1460 = control-ref of="Min Allowable Temp"() -> (w3025:refnum<vi>)
                }
              }
              n1461 = To Long Integer(number=w2910) -> (32bit integer=w2915:i32)
              n1462 = property class="Arr (strict)"(reference=w2933) -> ("Value"=w2934:dbl[][])  [unwired: 1 in, 2 out]
              n1463 = property class="LstBox (strict)"(reference=w2938) -> ("Item Symbols"=w2939:i32[])  [unwired: 1 in, 2 out]
              n1464 = property class="Str"(reference=w2924) -> ("Value"=w2923:string)  [unwired: 1 in, 2 out]
              n1465 = Fract/Exp String To Number(string=w2923) -> (number=w2922:dbl)  [unwired: 3 in, 1 out]
              n1466 = Array Size(array=w2939) -> (size(s)=w2940:i32)
              n1467 = for {
                N: w2940 -> [_]
                tunnel: w2939 -> [w2971]
                shift-right: [w2967] -> w2936
                shift-left: i32[] [] -> [w2966]
                i -> [w2965]
                n1468 = Index Array(array=w2971, index=w2965) -> (element=w2969:i32)
                n1469 = Equal?(x=w2969, y=38) -> (x = y?=w2970:bool)
                n1470 = case shown="True" w2970 {
                  tunnel: w2965 -> [_ w2975]
                  tunnel: [w2972 w2973] -> w2967
                  tunnel: w2966 -> [w2972 w2974]
                  frame False {
                  }
                  frame True {
                    n1471 = Build Array (concatenate)(w2974, w2975) -> (w2973:i32[])
                  }
                }
              }
              n1472 = property class="Ring (strict)"(reference=w2941) -> ("Value"=w2921:u16)  [unwired: 1 in, 2 out]
              n1473 = property class="Str"(reference=w2928) -> ("Value"=w2930:string)  [unwired: 1 in, 2 out]
              n1474 = property class="Str"(reference=w2929) -> ("Value"=w2931:string)  [unwired: 1 in, 2 out]
              n1475 = control-ref of="RampSoakTimes"() -> (w2935:refnum<vi>)
              n1476 = Decimal String To Number(string=w2931) -> (number=w2927:i32)  [unwired: 2 in, 1 out]
              n1477 = Decimal String To Number(string=w2930) -> (number=w2926:i32)  [unwired: 2 in, 1 out]
              n1478 = property class="Arr (strict)"(reference=w2935) -> ("Value"=w2914:dbl[][])  [unwired: 1 in, 2 out]
              n1479 = for {
                N: w2915 -> [_]
                shift-right: [w2948] -> w2913
                shift-left: w2914 -> [w2950]
                i -> [w2949]
                n1480 = Index Array(array=w2950, index (row) #1=w2949, index (col) #1=1 ("disabled index (col)"), index (row) #2=w2949, index (col) #2=2 ("disabled index (col)")) -> (element #1=w2955:dbl, element #2=w2954:dbl)
                n1481 = Less Than 0?(x=w2955) -> (x < 0?=w2952:bool)
                n1482 = Less Than 0?(x=w2954) -> (x < 0?=w2953:bool)
                n1483 = Or(x=w2952, y=w2953) -> (x .or. y?=w2951:bool)
                n1484 = case shown="True" w2951 {
                  tunnel: w2950 -> [w2958 w2961]
                  tunnel: w2949 -> [_ w2960]
                  tunnel: [w2958 w2959] -> w2948
                  frame False {
                  }
                  frame True {
                    n1485 = Delete From Array(array=w2961, index (row)=w2960) -> (array with subset deleted=w2959:dbl[][])  [unwired: 2 in, 1 out]
                  }
                }
              }
              n1486 = Array Size(array=w2913) -> (size(s)=w2912:i32[])
              n1487 = Index Array(array=w2912) -> (element=w2911:i32)  [unwired: 1 in]
              n1488 = Initialize Array(T37 {"thermalsetpoint"=0, "tempgoal"=0, "ramp"=0, "soakduration"=0} ("thermalprofiles"), w2911) -> (w2943:T49)
              n1489 = for {
                N: w2911 -> [_]
                tunnel: w2934 -> [w3038]
                tunnel: T37 {"thermalsetpoint"=0, "tempgoal"=0, "ramp"=0, "soakduration"=0} ("thermalprofiles") -> [w3049]
                shift-right: [w3047] -> w2932
                shift-left: w2943 -> [w3048]
                tunnel: w2913 -> [w3040]
                i -> [w3043]
                w3032 = 60.0 ("y")
                n1490 = Index Array(array=w3038, index (row)=w3043) -> (element=w3037:dbl[])  [unwired: 1 in]
                n1491 = Index Array(array=w3040, index (row)=w3043) -> (element=w3039:dbl[])  [unwired: 1 in]
                n1492 = Index Array(array=w3037, index #1=0 ("index (row)"), index #2=1 ("index (row)")) -> (element #1=w3036:dbl, element #2=w3035:dbl)
                n1493 = Index Array(array=w3039, index #1=1 ("index (row)"), index #2=2 ("index (row)")) -> (element #1=w3033:dbl, element #2=w3034:dbl)
                n1494 = Multiply(x=w3034, y=w3032) -> (x*y=w3030:dbl)
                n1495 = Multiply(x=w3033, y=w3032) -> (x*y=w3031:dbl)
                n1496 = Bundle By Name(cluster=w3049, "thermalsetpoint"=w3036, "tempgoal"=w3035, "ramp"=w3031, "soakduration"=w3030) -> (w3046:T37)
                n1497 = Replace Array Subset(array=w3048, new element=w3046, index=w3043) -> (w3047:T49)
              }
              n1498 = case shown="0, Default" w2921 {
                tunnel: ["Average" "Min" "Max"] -> w2920
                frame 0, Default {
                }
                frame 1 {
                }
                frame 2 {
                }
              }
              n1499 = Bundle By Name(cluster=T36 {"zone"=0, "average"="", "thermocouples"=[0], "maxTemp"=0, "minTemp"=0, "maxSlope"=0.0, "thermalprofiles"=[{"thermalsetpoint"=0, "tempgoal"=0, "ramp"=0, "soakduration"=0}]} ("ThermalProfileCluster.profiles"), "zone"=w2947, "average"=w2920, "thermocouples"=w2936, "maxTemp"=w2927, "minTemp"=w2926, "maxSlope"=w2922, "thermalprofiles"=w2932) -> (w2917:T36)
              n1500 = local write "profilearray"(dbl[][] []) -> ()
              n1501 = Build Array (concatenate)(w2919, w2917) -> (w2918:T47)
            }
          }
        }
        n1502 = control-ref of="Thermal Profile Name"() -> (w2706:refnum<vi>)
        n1503 = property on="Property Node" class="Str"(reference=w2706) -> ("Text.Text"=w2673:string)  [unwired: 1 in, 2 out]
        n1504 = Unbundle By Name(w2703) -> ("ZonesSelected"=w2702:bool[])
        n1505 = case shown="False" "TVAC Labview" {
          tunnel: [path "C:/Users/stefan/AppData/Local/conda/conda/envs/py35/python.exe" ("Path to Python.exe") path "C:/Users/TVAC-admin/AppData/Local/Programs/Python/Python35/python.exe" ("Path to Python.exe")] -> w2707
          frame False {
          }
          frame True {
          }
        }
        n1506 = local read "profilearray"() -> (w2689:dbl[][])
        n1507 = Delete From Array(array=w2724, index=0) -> (array with subset deleted=w2672:T47)  [unwired: 1 in, 1 out]
        n1508 = Bundle By Name(cluster=w2703, "ZoneProfile.profiles"=w2672, "ZoneSetup.Thermal Profile Name"=w2673) -> (w2679:T31)
        n1509 = local write "Compiled Profile Name"(w2673) -> ()
        n1510 = Flatten To JSON(anything=w2672, error in (no error)=w2674) -> (JSON string=w2720:string, 11:w2722:errorcluster)  [unwired: 1 in]
        n1511 = case shown="False" "TVAC Labview" {
          tunnel: [path "C:/Users/stefan/Documents/GitHub/TVAC/head/Labview2017/TVAC_GUI/Python_scripting/graph.json" ("file path (use dialog)") path "C:/Users/TVAC-admin/Documents/TVAC_Github/head/Labview2017/TVAC_GUI/Python_scripting/graph.json" ("file path (use dialog)")] -> w2718
          frame False {
          }
          frame True {
          }
        }
        n1512 = Open/Create/Replace File(file path (use dialog)=w2718, error in=w2722, operation (0:open)=T35."replace or create") -> (refnum out=w2721:refnum<file>, error out=w2719:errorcluster)  [unwired: 3 in, 1 out]
        n1513 = Write to Text File(file (use dialog)=w2721, text=w2720, error in=w2719) -> (refnum out=w2717:refnum<file>, error out=w2685:errorcluster)  [unwired: 1 in, 1 out]
        n1514 = Close File(refnum=w2717, error in=w2685) -> (error out=w2688:errorcluster)  [unwired: 1 out]
        n1515 = Concatenate Strings("Thermal Profile : ", w2673) -> (w2697:string)
        n1516 = Unbundle By Name(w2679) -> ("TCs"=w2678:T28)
        n1517 = Flatten To JSON(anything=w2678) -> (JSON string=w2677:string)  [unwired: 2 in, 1 out]
        n1518 = case shown="True" "TVAC Labview" {
          tunnel: [path "C:/Users/stefan/Documents/GitHub/TVAC/head/Labview2017/TVAC_GUI/Python_scripting/currentTC.json" ("file path (use dialog)") path "C:/Users/TVAC-admin/Documents/TVAC_Github/head/Labview2017/TVAC_GUI/Python_scripting/currentTC.json" ("file path (use dialog)")] -> w2676
          frame False {
          }
          frame True {
          }
        }
        n1519 = Open/Create/Replace File(file path (use dialog)=w2676, error in=w2688, operation (0:open)=T35."replace or create") -> (refnum out=w2682:refnum<file>, error out=w2687:errorcluster)  [unwired: 3 in, 1 out]
        n1520 = Write to Text File(file (use dialog)=w2682, text=w2677, error in=w2687) -> (refnum out=w2681:refnum<file>, error out=w2686:errorcluster)  [unwired: 1 in, 1 out]
        n1521 = Close File(refnum=w2681, error in=w2686) -> (error out=w2684:errorcluster)  [unwired: 1 out]
        n1522 = call "lvGraphProfile.vi"("pathToJson"=w2718, "error in (no error)"=w2684, "pathToJson 2"=w2676, "Path to Python.exe"=w2707, "RunCount"=w2693) -> ("graphCluster"=w2704:T50, "Raw Python String Output"=w2691:string, "error out"=w2708:errorcluster)  [unwired: 8 in]
        n1523 = Unbundle By Name(w2704) -> ("time"=w2701:dbl[])
        n1524 = for {
          N: 9 -> [_]
          tunnel: w2704 -> [w2761]
          tunnel: w2702 -> [_] mode=indexing
          shift-right: [w2762] -> w2700
          shift-left: w2701 -> [w2762]
          tunnel: w2697 -> [w2760]
          shift-right: [w2759] -> w2690
          shift-left: w2689 -> [w2757]
          tunnel: w2672 -> [w2751]
          i -> [w2750]
          n1525 = Equal To 0?(x=w2750) -> (x = 0?=w2758:bool)
          n1526 = Index Array(array=w2751, index=w2750) -> (element=w2749:T36)
          n1527 = case shown="True" w2758 {
            tunnel: w2757 -> [w2763 _]
            tunnel: [w2763 dbl[][] [] ("profilearray")] -> w2756
            frame False {
            }
            frame True {
            }
          }
          n1528 = Unbundle By Name(w2749) -> ("zone"=w2755:i32)
          n1529 = Number To Decimal String(number=w2755) -> (decimal integer string=w2753:string)  [unwired: 1 in]
          n1530 = Concatenate Strings("Zone " ("string"), w2753) -> (w2752:string)
          n1531 = case shown="8" w2750 {
            tunnel: w2761 -> [w2772 w2786 w2800 w2814 w2828 w2842 w2856 w2870 w2885]
            tunnel: w2760 -> [_ _ _ _ _ _ _ _ w2881]
            tunnel: [w2768 w2782 w2796 w2810 w2824 w2838 w2852 w2866 w2880] -> w2759
            tunnel: w2756 -> [w2767 w2781 w2795 w2809 w2823 w2837 w2851 w2865 w2879]
            tunnel: w2750 -> [w2766 w2780 w2794 w2808 w2822 w2836 w2850 w2864 w2878]
            tunnel: w2752 -> [w2765 w2779 w2793 w2807 w2821 w2835 w2849 w2863 w2877]
            frame 0, Default {
              n1532 = Unbundle By Name(w2772) -> ("zone1"=w2771:dbl[])
              n1533 = Index Array(array=w2771) -> (element=w2769:dbl)  [unwired: 1 in]
              n1534 = Not Equal To 0?(x=w2769) -> (x != 0?=w2770:bool)
              n1535 = case shown="True" w2770 {
                tunnel: w2771 -> [_ w2777]
                tunnel: [w2773 w2776] -> w2768
                tunnel: w2767 -> [w2773 _]
                tunnel: w2766 -> [_ w2775]
                tunnel: w2765 -> [_ w2774]
                frame False {
                }
                frame True {
                  n1536 = local read "profilearray"() -> (w2778:dbl[][])
                  n1537 = Build Array (concatenate)(w2778, w2777) -> (w2776:dbl[][])
                  n1538 = property on="Thermal Profile" class="WFGraph (strict)"("Active Plot"=w2775, "Plot.Plot Name"=w2774) -> ()  [unwired: 2 in, 2 out]
                  n1539 = local write "profilearray"(w2776) -> ()
                }
              }
            }
            frame 1 {
              n1540 = Unbundle By Name(w2786) -> ("zone2"=w2785:dbl[])
              n1541 = Index Array(array=w2785) -> (element=w2783:dbl)  [unwired: 1 in]
              n1542 = Not Equal To 0?(x=w2783) -> (x != 0?=w2784:bool)
              n1543 = case shown="True" w2784 {
                tunnel: w2785 -> [_ w2791]
                tunnel: [w2787 w2790] -> w2782
                tunnel: w2781 -> [w2787 _]
                tunnel: w2780 -> [_ w2789]
                tunnel: w2779 -> [_ w2788]
                frame False {
                }
                frame True {
                  n1544 = local read "profilearray"() -> (w2792:dbl[][])
                  n1545 = Build Array (concatenate)(w2792, w2791) -> (w2790:dbl[][])
                  n1546 = property on="Thermal Profile" class="WFGraph (strict)"("Active Plot"=w2789, "Plot.Plot Name"=w2788) -> ()  [unwired: 2 in, 2 out]
                  n1547 = local write "profilearray"(w2790) -> ()
                }
              }
            }
            frame 2 {
              n1548 = Unbundle By Name(w2800) -> ("zone3"=w2799:dbl[])
              n1549 = Index Array(array=w2799) -> (element=w2797:dbl)  [unwired: 1 in]
              n1550 = Not Equal To 0?(x=w2797) -> (x != 0?=w2798:bool)
              n1551 = case shown="True" w2798 {
                tunnel: w2799 -> [_ w2805]
                tunnel: [w2801 w2804] -> w2796
                tunnel: w2795 -> [w2801 _]
                tunnel: w2794 -> [_ w2803]
                tunnel: w2793 -> [_ w2802]
                frame False {
                }
                frame True {
                  n1552 = local read "profilearray"() -> (w2806:dbl[][])
                  n1553 = Build Array (concatenate)(w2806, w2805) -> (w2804:dbl[][])
                  n1554 = property on="Thermal Profile" class="WFGraph (strict)"("Active Plot"=w2803, "Plot.Plot Name"=w2802) -> ()  [unwired: 2 in, 2 out]
                  n1555 = local write "profilearray"(w2804) -> ()
                }
              }
            }
            frame 3 {
              n1556 = Unbundle By Name(w2814) -> ("zone4"=w2813:dbl[])
              n1557 = Index Array(array=w2813) -> (element=w2811:dbl)  [unwired: 1 in]
              n1558 = Not Equal To 0?(x=w2811) -> (x != 0?=w2812:bool)
              n1559 = case shown="True" w2812 {
                tunnel: w2813 -> [_ w2819]
                tunnel: [w2815 w2818] -> w2810
                tunnel: w2809 -> [w2815 _]
                tunnel: w2808 -> [_ w2817]
                tunnel: w2807 -> [_ w2816]
                frame False {
                }
                frame True {
                  n1560 = local read "profilearray"() -> (w2820:dbl[][])
                  n1561 = Build Array (concatenate)(w2820, w2819) -> (w2818:dbl[][])
                  n1562 = property on="Thermal Profile" class="WFGraph (strict)"("Active Plot"=w2817, "Plot.Plot Name"=w2816) -> ()  [unwired: 2 in, 2 out]
                  n1563 = local write "profilearray"(w2818) -> ()
                }
              }
            }
            frame 4 {
              n1564 = Unbundle By Name(w2828) -> ("zone5"=w2827:dbl[])
              n1565 = Index Array(array=w2827) -> (element=w2825:dbl)  [unwired: 1 in]
              n1566 = Not Equal To 0?(x=w2825) -> (x != 0?=w2826:bool)
              n1567 = case shown="True" w2826 {
                tunnel: w2827 -> [_ w2833]
                tunnel: [w2829 w2832] -> w2824
                tunnel: w2823 -> [w2829 _]
                tunnel: w2822 -> [_ w2831]
                tunnel: w2821 -> [_ w2830]
                frame False {
                }
                frame True {
                  n1568 = local read "profilearray"() -> (w2834:dbl[][])
                  n1569 = Build Array (concatenate)(w2834, w2833) -> (w2832:dbl[][])
                  n1570 = property on="Thermal Profile" class="WFGraph (strict)"("Active Plot"=w2831, "Plot.Plot Name"=w2830) -> ()  [unwired: 2 in, 2 out]
                  n1571 = local write "profilearray"(w2832) -> ()
                }
              }
            }
            frame 5 {
              n1572 = Unbundle By Name(w2842) -> ("zone6"=w2841:dbl[])
              n1573 = Index Array(array=w2841) -> (element=w2839:dbl)  [unwired: 1 in]
              n1574 = Not Equal To 0?(x=w2839) -> (x != 0?=w2840:bool)
              n1575 = case shown="True" w2840 {
                tunnel: w2841 -> [_ w2847]
                tunnel: [w2843 w2846] -> w2838
                tunnel: w2837 -> [w2843 _]
                tunnel: w2836 -> [_ w2845]
                tunnel: w2835 -> [_ w2844]
                frame False {
                }
                frame True {
                  n1576 = local read "profilearray"() -> (w2848:dbl[][])
                  n1577 = Build Array (concatenate)(w2848, w2847) -> (w2846:dbl[][])
                  n1578 = property on="Thermal Profile" class="WFGraph (strict)"("Active Plot"=w2845, "Plot.Plot Name"=w2844) -> ()  [unwired: 2 in, 2 out]
                  n1579 = local write "profilearray"(w2846) -> ()
                }
              }
            }
            frame 6 {
              n1580 = Unbundle By Name(w2856) -> ("zone7"=w2855:dbl[])
              n1581 = Index Array(array=w2855) -> (element=w2853:dbl)  [unwired: 1 in]
              n1582 = Not Equal To 0?(x=w2853) -> (x != 0?=w2854:bool)
              n1583 = case shown="True" w2854 {
                tunnel: w2855 -> [_ w2861]
                tunnel: [w2857 w2860] -> w2852
                tunnel: w2851 -> [w2857 _]
                tunnel: w2850 -> [_ w2859]
                tunnel: w2849 -> [_ w2858]
                frame False {
                }
                frame True {
                  n1584 = local read "profilearray"() -> (w2862:dbl[][])
                  n1585 = Build Array (concatenate)(w2862, w2861) -> (w2860:dbl[][])
                  n1586 = property on="Thermal Profile" class="WFGraph (strict)"("Active Plot"=w2859, "Plot.Plot Name"=w2858) -> ()  [unwired: 2 in, 2 out]
                  n1587 = local write "profilearray"(w2860) -> ()
                }
              }
            }
            frame 7 {
              n1588 = Unbundle By Name(w2870) -> ("zone8"=w2869:dbl[])
              n1589 = Index Array(array=w2869) -> (element=w2867:dbl)  [unwired: 1 in]
              n1590 = Not Equal To 0?(x=w2867) -> (x != 0?=w2868:bool)
              n1591 = case shown="True" w2868 {
                tunnel: w2869 -> [_ w2875]
                tunnel: [w2871 w2874] -> w2866
                tunnel: w2865 -> [w2871 _]
                tunnel: w2864 -> [_ w2873]
                tunnel: w2863 -> [_ w2872]
                frame False {
                }
                frame True {
                  n1592 = local read "profilearray"() -> (w2876:dbl[][])
                  n1593 = Build Array (concatenate)(w2876, w2875) -> (w2874:dbl[][])
                  n1594 = property on="Thermal Profile" class="WFGraph (strict)"("Active Plot"=w2873, "Plot.Plot Name"=w2872) -> ()  [unwired: 2 in, 2 out]
                  n1595 = local write "profilearray"(w2874) -> ()
                }
              }
            }
            frame 8 {
              n1596 = Unbundle By Name(w2885) -> ("zone9"=w2884:dbl[])
              n1597 = Index Array(array=w2884) -> (element=w2882:dbl)  [unwired: 1 in]
              n1598 = Not Equal To 0?(x=w2882) -> (x != 0?=w2883:bool)
              n1599 = case shown="True" w2883 {
                tunnel: w2884 -> [_ w2890]
                tunnel: [w2886 w2889] -> w2880
                tunnel: w2879 -> [w2886 _]
                tunnel: w2878 -> [_ w2888]
                tunnel: w2877 -> [_ w2887]
                frame False {
                }
                frame True {
                  n1600 = local read "profilearray"() -> (w2891:dbl[][])
                  n1601 = Build Array (concatenate)(w2891, w2890) -> (w2889:dbl[][])
                  n1602 = property on="Thermal Profile" class="WFGraph (strict)"("Active Plot"=w2888, "Plot.Plot Name"=w2887) -> ()  [unwired: 2 in, 2 out]
                  n1603 = local write "profilearray"(w2889) -> ()
                }
              }
              "ThermalProfileStatus" <- w2881
            }
          }
        }
        n1604 = local write "Thermal Profile Compiling Summary"(w2691) -> ()
        n1605 = Index Array(array=w2700, index=1) -> (element=w2699:dbl)
        n1606 = Index Array(array=w2700, index=0) -> (element=w2709:dbl)
        n1607 = Subtract(x=w2699, y=w2709) -> (x-y=w2714:dbl)
        n1608 = Divide(x=w2714, y=60.0) -> (x/y=w2712:dbl)
        n1609 = Bundle(0.0, w2712, "profilearray"=w2690) -> (→"Thermal Profile":cluster{dbl, dbl, "profilearray":dbl[][]})  [unwired: 1 in]
      }
      frame "importProfile" {
        w3055 = T51 0 items=["no dialog", "OK message", "continue or stop message", "OK message + warnings", "continue/stop + warnings"] ("type of dialog (OK msg:1)")
        n1610 = control-ref of="Import CSV as a Thermal Profile"() -> (w3057:refnum<vi>)
        n1611 = property on="Import CSV as a Thermal Profile" class="Path"() -> ("Text.Text"=w3090:string)  [unwired: 2 in, 2 out]
        n1612 = property class="Path"(reference=w3057, error in=w3054) -> (error out=w3051:errorcluster, "Value"=w3056:path)  [unwired: 1 out]
        n1613 = call-poly <vilib>:"Read Delimited Spreadsheet.vi"("file path (dialog if empty)"=w3056, "error in (no error)"=w3051, "delimiter (\\t)"="," ("delimiter (\\t)")) -> ("all rows"=w3075:string[][], "error out"=w3052:errorcluster)  [unwired: 7 in, 4 out]
        n1614 = Merge Errors(w3051, w3052) -> (w3050:errorcluster)
        n1615 = call <vilib>:"Simple Error Handler.vi"("type of dialog (OK msg:1)"=w3055, "error in (no error)"=w3050) -> ("error out"=w3053:errorcluster)  [unwired: 3 in, 4 out]
        n1616 = Bundle By Name(cluster=w3058, "tprofilesheet"=w3075) -> (w3100:T31)
        n1617 = local write "tprofilesheet"(w3075) -> ()
        n1618 = Array Size(array=w3075) -> (size(s)=w3094:i32[])
        n1619 = Index Array(array=w3075, index (row)=1) -> (element=w3101:string[])  [unwired: 1 in]
        n1620 = Index Array(array=w3075, index (row)=2) -> (element=w3097:string[])  [unwired: 1 in]
        n1621 = Spreadsheet String To Array(delimiter (Tab)="\\", format string="%s", spreadsheet string=w3090, array type (2D Dbl)=string[][] []) -> (array=w3085:string[][])
        n1622 = Array Size(array=w3085) -> (size(s)=w3084:i32[])
        n1623 = Index Array(array=w3094, index=0) -> (element=w3076:i32)
        n1624 = for {
          N: w3076 -> [_]
          shift-right: [w3129] -> w3074
          shift-left: w3075 -> [w3130]
          shift-right: [w3121] -> w3071
          shift-left: "LastSetPt" -> [w3120]
          i -> [w3125]
          n1625 = Add(x=7 ("y"), y=w3125) -> (x+y=w3124:i32)
          n1626 = Index Array(array=w3130, index (row)=w3124, index (col)=0 ("disabled index (col)")) -> (element=w3131:string)
          n1627 = Subtract(x=w3124, y=6) -> (x-y=w3122:i32)
          n1628 = Number To Decimal String(number=w3122) -> (decimal integer string=w3123:string)  [unwired: 1 in]
          n1629 = Equal?(x=w3131, y=w3123) -> (x = y?=w3128:bool)
          n1630 = case shown="True" w3128 {
            tunnel: w3130 -> [w3134 w3136]
            tunnel: [w3134 w3136] -> w3129
            tunnel: w3122 -> [_ w3135]
            tunnel: [w3133 w3135] -> w3121
            tunnel: w3120 -> [w3133 _]
            frame False {
            }
            frame True {
              n1631 = local write "LastSetPt"(w3135) -> ()
            }
          }
        }
        n1632 = Unbundle By Name(w3100) -> ("ZoneSetup.Zone Selection"=w3099:i32[])
        n1633 = Index Array(array=w3084, index=1) -> (element=w3082:i32)
        n1634 = Decrement(x=w3082) -> (x-1=w3081:i32)
        n1635 = Index Array(array=w3085, index (row)=0, index (col)=w3081) -> (element=w3080:string)
        n1636 = Match Pattern(string=w3080, regular expression=".csv") -> (before substring=w3077:string)  [unwired: 1 in, 3 out]
        n1637 = To Double Precision Float(number=w3071) -> (double precision float=w3091:dbl)
        n1638 = for {
          N: 9 -> [_]
          shift-right: [w3165] -> w3098
          shift-left: w3100 -> [w3178]
          tunnel: w3101 -> [w3177] mode=indexing
          shift-right: [w3175] -> w3095
          shift-left: w3099 -> [w3176]
          tunnel: w3097 -> [w3169]
          tunnel: w3074 -> [w3150]
          tunnel: w3071 -> [w3140]
          i -> [w3146]
          n1639 = case shown="0, Default" w3146 {
            selector: w3146 -> [w3273 w3308 w3343 w3378 w3413 w3448 w3483 w3518 w3553]
            tunnel: w3178 -> [w3277 w3312 w3347 w3382 w3417 w3452 w3487 w3522 w3557]
            tunnel: [w3276 w3311 w3346 w3381 w3416 w3451 w3486 w3521 w3556] -> w3166
            tunnel: w3177 -> [w3275 w3310 w3345 w3380 w3415 w3450 w3485 w3520 w3555]
            tunnel: w3176 -> [w3274 w3309 w3344 w3379 w3414 w3449 w3484 w3519 w3554]
            tunnel: [w3272 w3307 w3342 w3377 w3412 w3447 w3482 w3517 w3552] -> w3175
            tunnel: [w3271 w3306 w3341 w3376 w3411 w3446 w3481 w3516 w3551] -> w3138
            tunnel: [w3270 w3305 w3340 w3375 w3410 w3445 w3480 w3515 w3550] -> w3163
            tunnel: [w3267 w3302 w3337 w3372 w3407 w3442 w3477 w3512 w3547] -> w3164
            tunnel: [w3265 w3300 w3335 w3370 w3405 w3440 w3475 w3510 w3545] -> w3142
            tunnel: [w3264 w3299 w3334 w3369 w3404 w3439 w3474 w3509 w3544] -> w3151
            tunnel: [w3263 w3298 w3333 w3368 w3403 w3438 w3473 w3508 w3543] -> w3141
            frame 0, Default {
              n1640 = control-ref of="Thermocouples Selected"() -> (w3267:refnum<vi>)
              n1641 = case shown="\"Min\"" w3275 {
                tunnel: [2 1 0 0] -> w3268
                tunnel: w3274 -> [w3281 w3286 w3291 w3296]
                tunnel: w3273 -> [w3280 w3285 w3290 w3295]
                tunnel: [w3279 w3284 w3289 w3294] -> w3272
                frame "Max" {
                  n1642 = Replace Array Subset(array=w3281, new element=38, index=w3280) -> (w3279:i32[])
                }
                frame "Min" {
                  n1643 = Replace Array Subset(array=w3286, new element=38, index=w3285) -> (w3284:i32[])
                }
                frame "Average" {
                  n1644 = Replace Array Subset(array=w3291, new element=38, index=w3290) -> (w3289:i32[])
                }
                frame "", Default {
                  n1645 = Replace Array Subset(array=w3296, new element=37, index=w3295) -> (w3294:i32[])
                }
              }
              n1646 = control-ref of="Max Temp Slope (K/min)"() -> (w3265:refnum<vi>)
              n1647 = property class="Str"(reference=w3267, "Text.Text"="") -> ()  [unwired: 1 in, 2 out]
              n1648 = control-ref of="Min Allowable Temp"() -> (w3264:refnum<vi>)
              n1649 = control-ref of="Zone Thermocouples"() -> (w3270:refnum<vi>)
              n1650 = property class="LstBox (strict)"(reference=w3270) -> ("Item Symbols"=w3271:i32[])  [unwired: 1 in, 2 out]
              n1651 = control-ref of="Max Allowable Temp"() -> (w3263:refnum<vi>)
              n1652 = Bundle By Name(cluster=w3277, "Zone 1.Temperature Calculation"=w3268) -> (w3276:T31)
              n1653 = control-ref of="Temperature Calculation"() -> (w3269:refnum<vi>)
              n1654 = property class="Ring (strict)"(reference=w3269, "Value"=w3268) -> ()  [unwired: 1 in, 2 out]
            }
            frame 1 {
              n1655 = control-ref of="Thermocouples Selected"() -> (w3302:refnum<vi>)
              n1656 = case shown="\"Min\"" w3310 {
                tunnel: [2 1 0 0] -> w3303
                tunnel: w3309 -> [w3316 w3321 w3326 w3331]
                tunnel: w3308 -> [w3315 w3320 w3325 w3330]
                tunnel: [w3314 w3319 w3324 w3329] -> w3307
                frame "Max" {
                  n1657 = Replace Array Subset(array=w3316, new element=38, index=w3315) -> (w3314:i32[])
                }
                frame "Min" {
                  n1658 = Replace Array Subset(array=w3321, new element=38, index=w3320) -> (w3319:i32[])
                }
                frame "Average" {
                  n1659 = Replace Array Subset(array=w3326, new element=38, index=w3325) -> (w3324:i32[])
                }
                frame "", Default {
                  n1660 = Replace Array Subset(array=w3331, new element=37, index=w3330) -> (w3329:i32[])
                }
              }
              n1661 = control-ref of="Max Temp Slope (K/min)"() -> (w3300:refnum<vi>)
              n1662 = property class="Str"(reference=w3302, "Text.Text"="") -> ()  [unwired: 1 in, 2 out]
              n1663 = control-ref of="Min Allowable Temp"() -> (w3299:refnum<vi>)
              n1664 = control-ref of="Zone Thermocouples"() -> (w3305:refnum<vi>)
              n1665 = property class="LstBox (strict)"(reference=w3305) -> ("Item Symbols"=w3306:i32[])  [unwired: 1 in, 2 out]
              n1666 = control-ref of="Max Allowable Temp"() -> (w3298:refnum<vi>)
              n1667 = Bundle By Name(cluster=w3312, "Zone 2.Temperature Calculation"=w3303) -> (w3311:T31)
              n1668 = control-ref of="Temperature Calculation"() -> (w3304:refnum<vi>)
              n1669 = property class="Ring (strict)"(reference=w3304, "Value"=w3303) -> ()  [unwired: 1 in, 2 out]
            }
            frame 2 {
              n1670 = control-ref of="Thermocouples Selected"() -> (w3337:refnum<vi>)
              n1671 = case shown="\"Min\"" w3345 {
                tunnel: [2 1 0 0] -> w3338
                tunnel: w3344 -> [w3351 w3356 w3361 w3366]
                tunnel: w3343 -> [w3350 w3355 w3360 w3365]
                tunnel: [w3349 w3354 w3359 w3364] -> w3342
                frame "Max" {
                  n1672 = Replace Array Subset(array=w3351, new element=38, index=w3350) -> (w3349:i32[])
                }
                frame "Min" {
                  n1673 = Replace Array Subset(array=w3356, new element=38, index=w3355) -> (w3354:i32[])
                }
                frame "Average" {
                  n1674 = Replace Array Subset(array=w3361, new element=38, index=w3360) -> (w3359:i32[])
                }
                frame "", Default {
                  n1675 = Replace Array Subset(array=w3366, new element=37, index=w3365) -> (w3364:i32[])
                }
              }
              n1676 = control-ref of="Max Temp Slope (K/min)"() -> (w3335:refnum<vi>)
              n1677 = property class="Str"(reference=w3337, "Text.Text"="") -> ()  [unwired: 1 in, 2 out]
              n1678 = control-ref of="Min Allowable Temp"() -> (w3334:refnum<vi>)
              n1679 = control-ref of="Zone Thermocouples"() -> (w3340:refnum<vi>)
              n1680 = property class="LstBox (strict)"(reference=w3340) -> ("Item Symbols"=w3341:i32[])  [unwired: 1 in, 2 out]
              n1681 = control-ref of="Max Allowable Temp"() -> (w3333:refnum<vi>)
              n1682 = Bundle By Name(cluster=w3347, "Zone 3.Temperature Calculation"=w3338) -> (w3346:T31)
              n1683 = control-ref of="Temperature Calculation"() -> (w3339:refnum<vi>)
              n1684 = property class="Ring (strict)"(reference=w3339, "Value"=w3338) -> ()  [unwired: 1 in, 2 out]
            }
            frame 3 {
              n1685 = control-ref of="Thermocouples Selected"() -> (w3372:refnum<vi>)
              n1686 = case shown="\"Min\"" w3380 {
                tunnel: [2 1 0 0] -> w3373
                tunnel: w3379 -> [w3386 w3391 w3396 w3401]
                tunnel: w3378 -> [w3385 w3390 w3395 w3400]
                tunnel: [w3384 w3389 w3394 w3399] -> w3377
                frame "Max" {
                  n1687 = Replace Array Subset(array=w3386, new element=38, index=w3385) -> (w3384:i32[])
                }
                frame "Min" {
                  n1688 = Replace Array Subset(array=w3391, new element=38, index=w3390) -> (w3389:i32[])
                }
                frame "Average" {
                  n1689 = Replace Array Subset(array=w3396, new element=38, index=w3395) -> (w3394:i32[])
                }
                frame "", Default {
                  n1690 = Replace Array Subset(array=w3401, new element=37, index=w3400) -> (w3399:i32[])
                }
              }
              n1691 = control-ref of="Max Temp Slope (K/min)"() -> (w3370:refnum<vi>)
              n1692 = property class="Str"(reference=w3372, "Text.Text"="") -> ()  [unwired: 1 in, 2 out]
              n1693 = control-ref of="Min Allowable Temp"() -> (w3369:refnum<vi>)
              n1694 = control-ref of="Zone Thermocouples"() -> (w3375:refnum<vi>)
              n1695 = property class="LstBox (strict)"(reference=w3375) -> ("Item Symbols"=w3376:i32[])  [unwired: 1 in, 2 out]
              n1696 = control-ref of="Max Allowable Temp"() -> (w3368:refnum<vi>)
              n1697 = Bundle By Name(cluster=w3382, "Zone 4.Temperature Calculation"=w3373) -> (w3381:T31)
              n1698 = control-ref of="Temperature Calculation"() -> (w3374:refnum<vi>)
              n1699 = property class="Ring (strict)"(reference=w3374, "Value"=w3373) -> ()  [unwired: 1 in, 2 out]
            }
            frame 4 {
              n1700 = control-ref of="Thermocouples Selected"() -> (w3407:refnum<vi>)
              n1701 = case shown="\"Min\"" w3415 {
                tunnel: [2 1 0 0] -> w3408
                tunnel: w3414 -> [w3421 w3426 w3431 w3436]
                tunnel: w3413 -> [w3420 w3425 w3430 w3435]
                tunnel: [w3419 w3424 w3429 w3434] -> w3412
                frame "Max" {
                  n1702 = Replace Array Subset(array=w3421, new element=38, index=w3420) -> (w3419:i32[])
                }
                frame "Min" {
                  n1703 = Replace Array Subset(array=w3426, new element=38, index=w3425) -> (w3424:i32[])
                }
                frame "Average" {
                  n1704 = Replace Array Subset(array=w3431, new element=38, index=w3430) -> (w3429:i32[])
                }
                frame "", Default {
                  n1705 = Replace Array Subset(array=w3436, new element=37, index=w3435) -> (w3434:i32[])
                }
              }
              n1706 = control-ref of="Max Temp Slope (K/min)"() -> (w3405:refnum<vi>)
              n1707 = property class="Str"(reference=w3407, "Text.Text"="") -> ()  [unwired: 1 in, 2 out]
              n1708 = control-ref of="Min Allowable Temp"() -> (w3404:refnum<vi>)
              n1709 = control-ref of="Zone Thermocouples"() -> (w3410:refnum<vi>)
              n1710 = property class="LstBox (strict)"(reference=w3410) -> ("Item Symbols"=w3411:i32[])  [unwired: 1 in, 2 out]
              n1711 = control-ref of="Max Allowable Temp"() -> (w3403:refnum<vi>)
              n1712 = Bundle By Name(cluster=w3417, "Zone 5.Temperature Calculation"=w3408) -> (w3416:T31)
              n1713 = control-ref of="Temperature Calculation"() -> (w3409:refnum<vi>)
              n1714 = property class="Ring (strict)"(reference=w3409, "Value"=w3408) -> ()  [unwired: 1 in, 2 out]
            }
            frame 5 {
              n1715 = control-ref of="Thermocouples Selected"() -> (w3442:refnum<vi>)
              n1716 = case shown="\"Min\"" w3450 {
                tunnel: [2 1 0 0] -> w3443
                tunnel: w3449 -> [w3456 w3461 w3466 w3471]
                tunnel: w3448 -> [w3455 w3460 w3465 w3470]
                tunnel: [w3454 w3459 w3464 w3469] -> w3447
                frame "Max" {
                  n1717 = Replace Array Subset(array=w3456, new element=38, index=w3455) -> (w3454:i32[])
                }
                frame "Min" {
                  n1718 = Replace Array Subset(array=w3461, new element=38, index=w3460) -> (w3459:i32[])
                }
                frame "Average" {
                  n1719 = Replace Array Subset(array=w3466, new element=38, index=w3465) -> (w3464:i32[])
                }
                frame "", Default {
                  n1720 = Replace Array Subset(array=w3471, new element=37, index=w3470) -> (w3469:i32[])
                }
              }
              n1721 = control-ref of="Max Temp Slope (K/min)"() -> (w3440:refnum<vi>)
              n1722 = property class="Str"(reference=w3442, "Text.Text"="") -> ()  [unwired: 1 in, 2 out]
              n1723 = control-ref of="Min Allowable Temp"() -> (w3439:refnum<vi>)
              n1724 = control-ref of="Zone Thermocouples"() -> (w3445:refnum<vi>)
              n1725 = property class="LstBox (strict)"(reference=w3445) -> ("Item Symbols"=w3446:i32[])  [unwired: 1 in, 2 out]
              n1726 = control-ref of="Max Allowable Temp"() -> (w3438:refnum<vi>)
              n1727 = Bundle By Name(cluster=w3452, "Zone 6.Temperature Calculation"=w3443) -> (w3451:T31)
              n1728 = control-ref of="Temperature Calculation"() -> (w3444:refnum<vi>)
              n1729 = property class="Ring (strict)"(reference=w3444, "Value"=w3443) -> ()  [unwired: 1 in, 2 out]
            }
            frame 6 {
              n1730 = control-ref of="Thermocouples Selected"() -> (w3477:refnum<vi>)
              n1731 = case shown="\"Average\"" w3485 {
                tunnel: [2 1 0 0] -> w3478
                tunnel: w3484 -> [w3491 w3496 w3501 w3506]
                tunnel: w3483 -> [w3490 w3495 w3500 w3505]
                tunnel: [w3489 w3494 w3499 w3504] -> w3482
                frame "Max" {
                  n1732 = Replace Array Subset(array=w3491, new element=38, index=w3490) -> (w3489:i32[])
                }
                frame "Min" {
                  n1733 = Replace Array Subset(array=w3496, new element=38, index=w3495) -> (w3494:i32[])
                }
                frame "Average" {
                  n1734 = Replace Array Subset(array=w3501, new element=38, index=w3500) -> (w3499:i32[])
                }
                frame "", Default {
                  n1735 = Replace Array Subset(array=w3506, new element=37, index=w3505) -> (w3504:i32[])
                }
              }
              n1736 = control-ref of="Max Temp Slope (K/min)"() -> (w3475:refnum<vi>)
              n1737 = property class="Str"(reference=w3477, "Text.Text"="") -> ()  [unwired: 1 in, 2 out]
              n1738 = control-ref of="Min Allowable Temp"() -> (w3474:refnum<vi>)
              n1739 = control-ref of="Zone Thermocouples"() -> (w3480:refnum<vi>)
              n1740 = property class="LstBox (strict)"(reference=w3480) -> ("Item Symbols"=w3481:i32[])  [unwired: 1 in, 2 out]
              n1741 = control-ref of="Max Allowable Temp"() -> (w3473:refnum<vi>)
              n1742 = Bundle By Name(cluster=w3487, "Zone 7.Temperature Calculation"=w3478) -> (w3486:T31)
              n1743 = control-ref of="Temperature Calculation"() -> (w3479:refnum<vi>)
              n1744 = property class="Ring (strict)"(reference=w3479, "Value"=w3478) -> ()  [unwired: 1 in, 2 out]
            }
            frame 7 {
              n1745 = control-ref of="Thermocouples Selected"() -> (w3512:refnum<vi>)
              n1746 = case shown="\"Min\"" w3520 {
                tunnel: [2 1 0 0] -> w3513
                tunnel: w3519 -> [w3526 w3531 w3536 w3541]
                tunnel: w3518 -> [w3525 w3530 w3535 w3540]
                tunnel: [w3524 w3529 w3534 w3539] -> w3517
                frame "Max" {
                  n1747 = Replace Array Subset(array=w3526, new element=38, index=w3525) -> (w3524:i32[])
                }
                frame "Min" {
                  n1748 = Replace Array Subset(array=w3531, new element=38, index=w3530) -> (w3529:i32[])
                }
                frame "Average" {
                  n1749 = Replace Array Subset(array=w3536, new element=38, index=w3535) -> (w3534:i32[])
                }
                frame "", Default {
                  n1750 = Replace Array Subset(array=w3541, new element=37, index=w3540) -> (w3539:i32[])
                }
              }
              n1751 = control-ref of="Max Temp Slope (K/min)"() -> (w3510:refnum<vi>)
              n1752 = property class="Str"(reference=w3512, "Text.Text"="") -> ()  [unwired: 1 in, 2 out]
              n1753 = control-ref of="Min Allowable Temp"() -> (w3509:refnum<vi>)
              n1754 = control-ref of="Zone Thermocouples"() -> (w3515:refnum<vi>)
              n1755 = property class="LstBox (strict)"(reference=w3515) -> ("Item Symbols"=w3516:i32[])  [unwired: 1 in, 2 out]
              n1756 = control-ref of="Max Allowable Temp"() -> (w3508:refnum<vi>)
              n1757 = Bundle By Name(cluster=w3522, "Zone 8.Temperature Calculation"=w3513) -> (w3521:T31)
              n1758 = control-ref of="Temperature Calculation"() -> (w3514:refnum<vi>)
              n1759 = property class="Ring (strict)"(reference=w3514, "Value"=w3513) -> ()  [unwired: 1 in, 2 out]
            }
            frame 8 {
              n1760 = control-ref of="Thermocouples Selected"() -> (w3547:refnum<vi>)
              n1761 = case shown="\"Min\"" w3555 {
                tunnel: [2 1 0 0] -> w3548
                tunnel: w3554 -> [w3561 w3566 w3571 w3576]
                tunnel: w3553 -> [w3560 w3565 w3570 w3575]
                tunnel: [w3559 w3564 w3569 w3574] -> w3552
                frame "Max" {
                  n1762 = Replace Array Subset(array=w3561, new element=38, index=w3560) -> (w3559:i32[])
                }
                frame "Min" {
                  n1763 = Replace Array Subset(array=w3566, new element=38, index=w3565) -> (w3564:i32[])
                }
                frame "Average" {
                  n1764 = Replace Array Subset(array=w3571, new element=38, index=w3570) -> (w3569:i32[])
                }
                frame "", Default {
                  n1765 = Replace Array Subset(array=w3576, new element=37, index=w3575) -> (w3574:i32[])
                }
              }
              n1766 = control-ref of="Max Temp Slope (K/min)"() -> (w3545:refnum<vi>)
              n1767 = property class="Str"(reference=w3547, "Text.Text"="") -> ()  [unwired: 1 in, 2 out]
              n1768 = control-ref of="Min Allowable Temp"() -> (w3544:refnum<vi>)
              n1769 = control-ref of="Zone Thermocouples"() -> (w3550:refnum<vi>)
              n1770 = property class="LstBox (strict)"(reference=w3550) -> ("Item Symbols"=w3551:i32[])  [unwired: 1 in, 2 out]
              n1771 = control-ref of="Max Allowable Temp"() -> (w3543:refnum<vi>)
              n1772 = Bundle By Name(cluster=w3557, "Zone 9.Temperature Calculation"=w3548) -> (w3556:T31)
              n1773 = control-ref of="Temperature Calculation"() -> (w3549:refnum<vi>)
              n1774 = property class="Ring (strict)"(reference=w3549, "Value"=w3548) -> ()  [unwired: 1 in, 2 out]
            }
          }
          n1775 = Index Array(array=w3169, index=w3146) -> (element=w3172:string)
          n1776 = call <vilib>:"Space Constant.vi"() -> ("String"=w3173:string)
          n1777 = Initialize Array("", w3140, 3 ("dimension size")) -> (w3155:string[][])
          n1778 = Spreadsheet String To Array(delimiter (Tab)=w3173, format string="%d", spreadsheet string=w3172) -> (array=w3174:dbl[][])  [unwired: 1 in]
          n1779 = Initialize Array("", w3140, 2 ("dimension size")) -> (w3162:string[][])
          n1780 = Index Array(array=w3174, index (row)=0) -> (element=w3168:dbl[])  [unwired: 1 in]
          n1781 = for {
            N: w3140 -> [_]
            tunnel: w3150 -> [w3200]
            shift-right: [w3197] -> w3159
            shift-left: w3162 -> [w3198]
            tunnel: w3146 -> [w3192]
            shift-right: [w3181] -> w3154
            shift-left: w3155 -> [w3182]
            i -> [w3184]
            n1782 = Add(x=3, y=w3192) -> (x+y=w3191:i32)
            n1783 = Add(x=7, y=w3184) -> (x+y=w3190:i32)
            n1784 = Index Array(array=w3200, index (row) #1=w3190, index (col) #1=0 ("disabled index (col)"), index (row) #2=w3190, index (col) #2=w3191, index (row) #3=w3190, index (col) #3=1 ("disabled index (col)"), index (row) #4=w3190, index (col) #4=2 ("disabled index (col)")) -> (element #1=w3187:string, element #2=w3195:string, element #3=w3186:string, element #4=w3185:string)
            n1785 = Build Array(w3187, w3195) -> (w3194:string[])
            n1786 = Build Array(w3187, w3186, w3185) -> (w3183:string[])
            n1787 = Replace Array Subset(array=w3198, new element=w3194, index (row)=w3184) -> (w3197:string[][])  [unwired: 1 in]
            n1788 = Replace Array Subset(array=w3182, new element=w3183, index (row)=w3184) -> (w3181:string[][])  [unwired: 1 in]
          }
          n1789 = To Long Integer(number=w3168) -> (32bit integer=w3167:i32[])
          n1790 = Array Size(array=w3167) -> (size(s)=w3139:i32)
          n1791 = for {
            N: w3139 -> [_]
            tunnel: w3167 -> [w3248] mode=indexing
            shift-right: [w3246] -> w3137
            shift-left: w3138 -> [w3247]
            tunnel: w3164 -> [w3251]
            n1792 = Not Equal To 0?(x=w3248) -> (x != 0?=w3250:bool)
            n1793 = case shown="True" w3250 {
              tunnel: w3248 -> [_ w3258]
              tunnel: w3251 -> [_ w3257]
              tunnel: 38 -> [_ w3256]
              tunnel: w3248 -> [_ w3255]
              tunnel: [w3252 w3254] -> w3246
              tunnel: w3247 -> [w3252 w3253]
              frame False {
              }
              frame True {
                n1794 = Number To Decimal String(number=w3258) -> (decimal integer string=w3259:string)  [unwired: 1 in]
                n1795 = property class="Str"(reference=w3257) -> ("Text.Text"=w3262:string)  [unwired: 1 in, 2 out]
                n1796 = call <vilib>:"Space Constant.vi"() -> ("String"=w3260:string)
                n1797 = Replace Array Subset(array=w3253, new element=w3256, index=w3255) -> (w3254:i32[])
                n1798 = Concatenate Strings(w3262, w3260, w3259) -> (w3261:string)
                n1799 = property class="Str"(reference=w3257, "Text.Text"=w3261) -> ()  [unwired: 1 in, 2 out]
              }
            }
          }
          n1800 = property class="LstBox (strict)"(reference=w3163, "Item Symbols"=w3137) -> ()  [unwired: 1 in, 2 out]
          n1801 = Fract/Exp String To Number(string=w3154) -> (number=w3152:dbl[][])  [unwired: 3 in, 1 out]
          n1802 = Fract/Exp String To Number(string=w3159) -> (number=w3158:dbl[][])  [unwired: 3 in, 1 out]
          n1803 = case shown="0, Default" w3146 {
            tunnel: w3166 -> [w3205 w3210 w3215 w3220 w3225 w3230 w3235 w3240 w3245]
            tunnel: [w3204 w3209 w3214 w3219 w3224 w3229 w3234 w3239 w3244] -> w3165
            tunnel: w3137 -> [w3203 w3208 w3213 w3218 w3223 w3228 w3233 w3238 w3243]
            tunnel: w3158 -> [w3201 w3206 w3211 w3216 w3221 w3226 w3231 w3236 w3241]
            frame 0, Default {
              n1804 = Bundle By Name(cluster=w3205, "Zone 1.Zone Thermocouples"=w3203) -> (w3204:T31)
              n1805 = control-ref of="Temperature Goal"() -> (w3202:refnum<vi>)
              n1806 = property class="Arr (strict)"(reference=w3202, "Value"=w3201) -> ()  [unwired: 1 in, 2 out]
            }
            frame 1 {
              n1807 = Bundle By Name(cluster=w3210, "Zone 2.Zone Thermocouples"=w3208) -> (w3209:T31)
              n1808 = control-ref of="Temperature Goal"() -> (w3207:refnum<vi>)
              n1809 = property class="Arr (strict)"(reference=w3207, "Value"=w3206) -> ()  [unwired: 1 in, 2 out]
            }
            frame 2 {
              n1810 = Bundle By Name(cluster=w3215, "Zone 3.Zone Thermocouples"=w3213) -> (w3214:T31)
              n1811 = control-ref of="Temperature Goal"() -> (w3212:refnum<vi>)
              n1812 = property class="Arr (strict)"(reference=w3212, "Value"=w3211) -> ()  [unwired: 1 in, 2 out]
            }
            frame 3 {
              n1813 = Bundle By Name(cluster=w3220, "Zone 4.Zone Thermocouples"=w3218) -> (w3219:T31)
              n1814 = control-ref of="Temperature Goal"() -> (w3217:refnum<vi>)
              n1815 = property class="Arr (strict)"(reference=w3217, "Value"=w3216) -> ()  [unwired: 1 in, 2 out]
            }
            frame 4 {
              n1816 = Bundle By Name(cluster=w3225, "Zone 5.Zone Thermocouples"=w3223) -> (w3224:T31)
              n1817 = control-ref of="Temperature Goal"() -> (w3222:refnum<vi>)
              n1818 = property class="Arr (strict)"(reference=w3222, "Value"=w3221) -> ()  [unwired: 1 in, 2 out]
            }
            frame 5 {
              n1819 = Bundle By Name(cluster=w3230, "Zone 6.Zone Thermocouples"=w3228) -> (w3229:T31)
              n1820 = control-ref of="Temperature Goal"() -> (w3227:refnum<vi>)
              n1821 = property class="Arr (strict)"(reference=w3227, "Value"=w3226) -> ()  [unwired: 1 in, 2 out]
            }
            frame 6 {
              n1822 = Bundle By Name(cluster=w3235, "Zone 7.Zone Thermocouples"=w3233) -> (w3234:T31)
              n1823 = control-ref of="Temperature Goal"() -> (w3232:refnum<vi>)
              n1824 = property class="Arr (strict)"(reference=w3232, "Value"=w3231) -> ()  [unwired: 1 in, 2 out]
            }
            frame 7 {
              n1825 = Bundle By Name(cluster=w3240, "Zone 8.Zone Thermocouples"=w3238) -> (w3239:T31)
              n1826 = control-ref of="Temperature Goal"() -> (w3237:refnum<vi>)
              n1827 = property class="Arr (strict)"(reference=w3237, "Value"=w3236) -> ()  [unwired: 1 in, 2 out]
            }
            frame 8 {
              n1828 = Bundle By Name(cluster=w3245, "Zone 9.Zone Thermocouples"=w3243) -> (w3244:T31)
              n1829 = control-ref of="Temperature Goal"() -> (w3242:refnum<vi>)
              n1830 = property class="Arr (strict)"(reference=w3242, "Value"=w3241) -> ()  [unwired: 1 in, 2 out]
            }
          }
          n1831 = Equal To 0?(x=w3146) -> (x = 0?=w3153:bool)
          n1832 = case shown="True" w3153 {
            tunnel: w3152 -> [_ w3179]
            frame False {
            }
            frame True {
              n1833 = control-ref of="RampSoakTimes"() -> (w3180:refnum<vi>)
              n1834 = property class="Arr (strict)"(reference=w3180, "Value"=w3179) -> ()  [unwired: 1 in, 2 out]
            }
          }
          n1835 = Index Array(array=w3150, index (row) #1=3 ("dimension size"), index (col) #1=w3146, index (row) #2=4 ("dimension size"), index (col) #2=w3146, index (row) #3=5 ("dimension size"), index (col) #3=w3146) -> (element #1=w3145:string, element #2=w3144:string, element #3=w3143:string)
          n1836 = property class="Str"(reference=w3141, "Value"=w3145) -> ()  [unwired: 1 in, 2 out]
          n1837 = property class="Str"(reference=w3151, "Value"=w3144) -> ()  [unwired: 1 in, 2 out]
          n1838 = property class="Str"(reference=w3142, "Value"=w3143) -> ()  [unwired: 1 in, 2 out]
        }
        n1839 = control-ref of="Zone Selection"() -> (w3096:refnum<vi>)
        n1840 = control-ref of="Number of Set points"() -> (w3092:refnum<vi>)
        n1841 = control-ref of="Thermal Profile Name"() -> (w3078:refnum<vi>)
        n1842 = Bundle By Name(cluster=w3098, "ZoneSetup.Zone Selection"=w3095, "ZoneSetup.Number of Set points"=w3091, "ZoneSetup.Thermal Profile Name"=w3077) -> (w3065:T31)
        n1843 = Unbundle By Name(w3065) -> ("ZoneSetup.Zone Selection"=w3070:i32[], "ZonesSelected"=w3068:bool[])
        n1844 = property class="LstBox (strict)"(reference=w3096, "Item Symbols"=w3095) -> ()  [unwired: 1 in, 2 out]
        n1845 = property class="Str"(reference=w3078, "Text.Text"=w3077) -> ()  [unwired: 1 in, 2 out]
        n1846 = property class="DigNum (strict)"(reference=w3092, "Value"=w3091) -> ()  [unwired: 1 in, 2 out]
        n1847 = for {
          N: 9 -> [_]
          tunnel: w3070 -> [w3108] mode=indexing
          shift-right: [w3106] -> w3067
          shift-left: w3068 -> [w3111]
          shift-right: [w3110] -> w3062
          shift-left: w3053 -> [w3110]
          i -> [w3105]
          n1848 = Equal?(x=37, y=w3108) -> (x = y?=w3107:bool)
          n1849 = case shown="False" w3107 {
            tunnel: w3111 -> [w3115 w3119]
            tunnel: w3105 -> [w3114 w3118]
            tunnel: [w3112 w3116] -> w3106
            frame False {
              n1850 = Replace Array Subset(array=w3115, new element=TRUE ("new element/subarray"), index=w3114) -> (w3112:bool[])
            }
            frame True {
              n1851 = Replace Array Subset(array=w3119, new element=FALSE ("new element/subarray"), index=w3118) -> (w3116:bool[])
            }
          }
        }
        n1852 = local read "importexe"() -> (w3060:dbl)
        n1853 = Increment(x=w3060) -> (x+1=w3059:dbl)
        n1854 = local write "importexe"(w3059) -> ()
        n1855 = Bundle By Name(cluster=w3065, "ZonesSelected"=w3067) -> (w3066:T31)
        n1856 = call-poly "Send Message.vi"("error in (no error)"=w3062, "event buffer"="2", "event"="compileProfile") -> ("error out"=w3064:errorcluster)  [unwired: 8 in]
      }
      frame "saveProfile" {
        n1857 = Unbundle By Name(w3593) -> ("ZoneSetup.Number of Set points"=w3589:dbl)
        n1858 = Initialize Array("", w3589, 12 ("dimension size")) -> (w3588:string[][])
        n1859 = Build Array (concatenate)(string[][] [["zone1", "zone2", "zone3", "zone4", "zone5", "zone6", "zone7", "zone8", "zone9", "", "", ""], ["", "", "", "", "", "", "", "", "", "", "", ""], ["", "", "", "", "", "", "", "", "", "", "", ""], ["", "", "", "", "", "", "", "", "", "", "", ""], ["", "", "", "", "", "", "", "", "", "", "", ""], ["", "", "", "", "", "", "", "", "", "", "", ""], ["setpt", "ramptime", "soaktime", "zone1", "zone2", "zone3", "zone4", "zone5", "zone6", "zone7", "zone8", "zone9"]], w3588) -> (w3587:string[][])
        n1860 = for {
          N: 9 -> [_]
          shift-right: [w3619] -> w3579
          shift-left: w3593 -> [w3619]
          tunnel: w3589 -> [w3601]
          shift-right: [w3611] -> w3586
          shift-left: w3587 -> [w3615]
          i -> [w3609]
          n1861 = Unbundle By Name(w3619) -> ("ZoneProfile.profiles"=w3614:T47)
          n1862 = Index Array(array=w3614, index=w3609) -> (element=w3613:T36)
          n1863 = Unbundle By Name(w3613) -> ("zone"=w3604:i32, "average"=w3599:string, "thermocouples"=w3610:i32[], "maxTemp"=w3618:i32, "minTemp"=w3617:i32, "maxSlope"=w3616:dbl, "thermalprofiles"=w3600:T49)
          n1864 = Subtract(x=w3604, y=1) -> (x-y=w3602:i32)
          n1865 = Equal?(x=w3599, y="") -> (x = y?=w3607:bool)
          n1866 = Equal?(x=w3599, y="0") -> (x = y?=w3598:bool)
          n1867 = Or(x=w3607, y=w3598) -> (x .or. y?=w3603:bool)
          n1868 = case shown="False" w3603 {
            tunnel: w3599 -> [w3666 _]
            tunnel: w3618 -> [w3662 _]
            tunnel: w3617 -> [w3657 _]
            tunnel: w3616 -> [w3653 _]
            tunnel: w3615 -> [w3652 w3687]
            tunnel: [w3641 w3687] -> w3612
            tunnel: w3610 -> [w3651 _]
            tunnel: w3602 -> [w3640 _]
            tunnel: w3601 -> [w3644 _]
            tunnel: w3600 -> [w3643 _]
            frame False {
              n1869 = Number To Decimal String(number=w3662) -> (decimal integer string=w3661:string)  [unwired: 1 in]
              n1870 = Number To Decimal String(number=w3657) -> (decimal integer string=w3660:string)  [unwired: 1 in]
              n1871 = Number To Decimal String(number=w3651) -> (decimal integer string=w3649:string[])  [unwired: 1 in]
              n1872 = Array Size(array=w3649) -> (size(s)=w3650:i32)
              n1873 = Replace Array Subset(array=w3652, new element=w3666, index (row)=1 ("disabled index (row)"), index (col)=w3640) -> (w3648:string[][])
              n1874 = Number To Fractional String(number=w3653) -> (F-format string=w3656:string)  [unwired: 3 in]
              n1875 = for {
                N: w3650 -> [_]
                tunnel: w3649 -> [w3683] mode=indexing
                shift-right: [w3679] -> w3646
                shift-left: w3648 -> [w3679]
                tunnel: [w3678] -> w3647
                i -> [w3681]
                n1876 = Equal To 0?(x=w3681) -> (x = 0?=w3682:bool)
                n1877 = case shown="True" w3682 {
                  tunnel: [w3685 w3686] -> w3680
                  frame False {
                    n1878 = local read "string"() -> (w3685:string)
                  }
                  frame True {
                    w3686 = ""
                    n1879 = local write "string"(w3686) -> ()
                  }
                }
                n1880 = call <vilib>:"Space Constant.vi"() -> ("String"=w3684:string)
                n1881 = Concatenate Strings(w3680, w3683, w3684) -> (w3678:string)
                n1882 = local write "string"(w3678) -> ()
              }
              n1883 = Replace Array Subset(array=w3646, new element=w3647, index (row)=2 ("disabled index (row)"), index (col)=w3640) -> (w3645:string[][])
              n1884 = Replace Array Subset(array=w3645, new element=w3661, index (row)=3 ("disabled index (row)"), index (col)=w3640) -> (w3658:string[][])
              n1885 = Replace Array Subset(array=w3658, new element=w3660, index (row)=4 ("disabled index (row)"), index (col)=w3640) -> (w3654:string[][])
              n1886 = Replace Array Subset(array=w3654, new element=w3656, index (row)=5 ("disabled index (row)"), index (col)=w3640) -> (w3642:string[][])
              n1887 = for {
                N: w3644 -> [_]
                tunnel: w3643 -> [w3677] mode=indexing
                shift-right: [w3674] -> w3641
                shift-left: w3642 -> [w3675]
                tunnel: w3640 -> [w3670]
                i -> [w3673]
                n1888 = Unbundle By Name(w3677) -> ("tempgoal"=w3676:i32)
                n1889 = Add(x=3 ("disabled index (row)"), y=w3670) -> (x+y=w3668:i32)
                n1890 = Add(x=7 ("disabled index (row)"), y=w3673) -> (x+y=w3671:i32)
                n1891 = Number To Decimal String(number=w3676) -> (decimal integer string=w3667:string)  [unwired: 1 in]
                n1892 = Replace Array Subset(array=w3675, new element=w3667, index (row)=w3671, index (col)=w3668) -> (w3674:string[][])
              }
            }
            frame True {
            }
          }
          n1893 = for {
            N: w3601 -> [_]
            tunnel: w3600 -> [w3633] mode=indexing
            shift-right: [w3636] -> w3611
            shift-left: w3612 -> [w3638]
            tunnel: w3609 -> [_]
            tunnel: w3602 -> [_]
            i -> [w3634]
            w3620 = 60.0
            (unwired) 3 ("disabled index (row)")
            n1894 = Unbundle By Name(w3633) -> ("thermalsetpoint"=w3639:i32, "ramp"=w3632:i32, "soakduration"=w3631:i32)
            n1895 = Add(x=7 ("disabled index (row)"), y=w3634) -> (x+y=w3635:i32)
            n1896 = Number To Decimal String(number=w3639) -> (decimal integer string=w3629:string)  [unwired: 1 in]
            n1897 = Divide(x=w3632, y=w3620) -> (x/y=w3622:dbl)
            n1898 = Divide(x=w3631, y=w3620) -> (x/y=w3621:dbl)
            n1899 = Replace Array Subset(array=w3638, new element=w3629, index (row)=w3635, index (col)=0 ("disabled index (row)")) -> (w3628:string[][])
            n1900 = Number To Decimal String(number=w3622) -> (decimal integer string=w3627:string)  [unwired: 1 in]
            n1901 = Replace Array Subset(array=w3628, new element=w3627, index (row)=w3635, index (col)=1 ("disabled index (row)")) -> (w3623:string[][])
            n1902 = Number To Decimal String(number=w3621) -> (decimal integer string=w3625:string)  [unwired: 1 in]
            n1903 = Replace Array Subset(array=w3623, new element=w3625, index (row)=w3635, index (col)=2 ("disabled index (row)")) -> (w3636:string[][])
          }
        }
        n1904 = local read "TVAC Labview"() -> (w3584:bool)
        n1905 = case shown="True" w3584 {
          tunnel: ["C:\\Users\\stefan\\Documents\\GitHub\\TVAC\\head\\Labview2017\\TVAC_GUI\\DatabaseCSV\\" "C:\\Users\\TVAC-admin\\Documents\\TVAC_Github\\head\\Labview2017\\TVAC_GUI\\DatabaseCSV\\" ("file path (use dialog)")] -> w3583
          frame False {
          }
          frame True {
          }
        }
        n1906 = Unbundle By Name(w3579) -> ("ZoneSetup.Thermal Profile Name"=w3578:string)
        n1907 = Concatenate Strings(w3583, w3578, ".csv" ("string")) -> (w3582:string)
        n1908 = String To Path(string=w3582) -> (path=w3580:path)
        n1909 = call-poly <vilib>:"Write Delimited Spreadsheet.vi"("file path (dialog if empty)"=w3580, "2D data"=w3586, "delimiter (\\t)"="," ("delimiter (\\t)")) -> ()  [unwired: 11 in, 2 out]
      }
      frame "graphTC" {
        n1910 = Unbundle By Name(w3699) -> ("working array"=w3696:bool[], "Thermocouples"=w3697:T3, "TCs"=w3690:T28)
        n1911 = property on="Waveform Chart" class="WFChart (strict)"("LegScrollVis"=TRUE ("Legend:Scrollbar Visible")) -> ()  [unwired: 2 in, 2 out]
        n1912 = for {
          N: 120 -> [_]
          tunnel: w3690 -> [w3732] mode=indexing
          tunnel: [w3731] -> w3691 mode=indexing
          shift-right: [w3710] -> w3693
          shift-left: w3697 -> [w3717]
          shift-right: [w3709] -> w3698
          shift-left: w3696 -> [w3708]
          i -> [w3707]
          n1913 = Unbundle By Name(w3732) -> ("thermocouple"=w3741:i32, "temp"=w3704:dbl, "alarm"=w3736:i32, "working"=w3735:bool)
          n1914 = Quotient & Remainder(x=w3707, y=4) -> (x-y*floor(x/y)=w3715:i32, floor(x/y)=w3716:i32)
          n1915 = Index Array(array=w3717, index (row)=w3716, index (col)=w3715) -> (element=w3730:T32)
          n1916 = Multiply(x=w3716, y=4) -> (x*y=w3725:i32)
          n1917 = Multiply(x=w3716, y=4) -> (x*y=w3737:i32)
          n1918 = Unbundle By Name(w3730) -> ("Graph On/Off"=w3714:u32)
          n1919 = Add(x=w3725, y=w3715) -> (x+y=w3723:i32)
          n1920 = Add(x=w3737, y=w3715) -> (x+y=w3706:i32)
          n1921 = Replace Array Subset(array=w3708, new element=w3735, index=w3707) -> (w3709:bool[])
          n1922 = To Double Precision Float(number=w3704) -> (double precision float=w3703:dbl)
          n1923 = Get Date/Time In Seconds() -> (seconds since 1Jan1904=w3734:timestamp)
          n1924 = property on="Waveform Chart" class="WFChart (strict)"("Active Plot"=w3706) -> ()  [unwired: 2 in, 2 out]
          n1925 = Index Array(array=w3709, index=w3723) -> (element=w3722:bool)
          n1926 = Bundle By Name("t0"=w3734) -> (w3733:waveform(dbl))  [unwired: 1 in]
          n1927 = Build Array(w3703) -> (w3705:dbl[])
          n1928 = Number To Fractional String(number=w3703, precision (6)=i16 2 ("width (-)")) -> (F-format string=w3720:string)  [unwired: 2 in]
          n1929 = Bundle By Name(cluster=w3733, "Y"=w3705) -> (w3731:waveform(dbl))
          n1930 = case shown="True" w3722 {
            tunnel: w3714 -> [_ w3746]
            tunnel: [u32 12369084 ("y") w3746] -> w3718
            tunnel: w3720 -> [_ w3745]
            tunnel: ["NaN" w3745] -> w3719
            frame False {
            }
            frame True {
            }
          }
          n1931 = case shown="2" w3736 {
            tunnel: ["" "L" "H"] -> w3711
            tunnel: w3736 -> [_ _ _]
            tunnel: [u32 12369084 u32 2812927 u32 16711680] -> w3712
            frame 0, Default {
            }
            frame 1 {
            }
            frame 2 {
            }
          }
          n1932 = Number To Decimal String(number=w3741) -> (decimal integer string=w3742:string)  [unwired: 1 in]
          n1933 = Index Array(array=w3717, index (row)=w3716, index (col)=w3715) -> (element=w3728:T32)
          n1934 = Equal?(x=w3718, y=u32 6618880) -> (x = y?=w3726:bool)
          n1935 = Concatenate Strings("TC " ("string"), w3742) -> (w3713:string)
          n1936 = property on="Waveform Chart" class="WFChart (strict)"("Plot.Plot Name"=w3713) -> ()  [unwired: 2 in, 2 out]
          n1937 = case shown="True" w3726 {
            tunnel: [w3754 w3762] -> w3729
            tunnel: w3728 -> [w3753 w3761]
            tunnel: w3718 -> [w3751 w3760]
            tunnel: w3719 -> [w3752 w3759]
            tunnel: w3713 -> [w3750 w3758]
            tunnel: w3712 -> [w3749 w3757]
            tunnel: w3711 -> [w3748 w3756]
            frame False {
              n1938 = Bundle By Name(cluster=w3753, "Graph On/Off"=w3751, "TC Label"=w3750, "PlotColor"=u32 12369084 ("y"), "Temperature"=w3752, "Alarm Color"=w3749, "Alarm Status"=w3748) -> (w3754:T32)
            }
            frame True {
              n1939 = property on="Waveform Chart" class="WFChart (strict)"() -> ("Plot.Plot Color"=w3755:u32)  [unwired: 2 in, 2 out]
              n1940 = Bundle By Name(cluster=w3761, "Graph On/Off"=w3760, "TC Label"=w3758, "PlotColor"=w3755, "Temperature"=w3759, "Alarm Color"=w3757, "Alarm Status"=w3756) -> (w3762:T32)
            }
          }
          n1941 = Replace Array Subset(array=w3717, new element=w3729, index (row)=w3716, index (col)=w3715) -> (w3710:T3)
        }
        n1942 = local write "Thermocouples"(w3693) -> ()
        n1943 = Bundle By Name(cluster=w3699, "Thermocouples"=w3693, "working array"=w3698) -> (w3694:T31)
        n1944 = Build Array (concatenate)(waveform(dbl) {"t0"=timestamp(0 s since 1904-01-01), "dt"=1.0, "Y"=[]} ("element"), w3691) -> (w3701:waveform(dbl)[])
        n1945 = Delete From Array(array=w3701, index=0) -> (array with subset deleted=→"Waveform Chart":waveform(dbl)[])  [unwired: 1 in, 1 out]
      }
      frame "receiveDatabase" {
        n1946 = control-ref of="Saved Database Profiles"() -> (w3774:refnum<vi>)
        n1947 = control-ref of="Rename Existing Database Profile"() -> (w3770:refnum<vi>)
        n1948 = Spreadsheet String To Array(format string="%s", spreadsheet string=w3773, array type (2D Dbl)=string[] []) -> (array=w3769:string[])  [unwired: 1 in]
        n1949 = property class="Ring (strict)"(reference=w3774, "Strings []"=w3769) -> ()  [unwired: 1 in, 2 out]
        n1950 = property class="Ring (strict)"(reference=w3770, "Strings []"=w3769) -> ()  [unwired: 1 in, 2 out]
      }
      frame "receiveCryoPump_plots" {
        w3779 = T52 {"Duty Cycle (0-100)"=0.0, "1st stage Temp (K)"=0.0, "2nd stage Temp (K)"=0.0, "Helium Return Pressure (psig)"=0, "Helium Discharge Temp (K)"=0, "Water Inlet Temp (K)"=0, "Water Outlet Temp (K)"=0}
        n1951 = Flatten To JSON(anything=w3779) -> (JSON string=w3778:string)  [unwired: 2 in, 1 out]
        n1952 = Empty String/Path?(string/path=w3778) -> ()  [unwired: 1 out]
        n1953 = Unflatten From JSON(JSON string=w3782, type and defaults=w3779, default null elements? (F)=TRUE) -> (value=w3788:T52)  [unwired: 4 in, 1 out]
        n1954 = Unbundle By Name(w3788) -> ("1st stage Temp (K)"=w3787:dbl, "2nd stage Temp (K)"=w3786:dbl, "Helium Discharge Temp (K)"=w3777:u32)  [unwired: 4 out]
        n1955 = Build Array(w3787) -> (w3784:dbl[])
        n1956 = Build Array(w3786) -> (w3785:dbl[])
        n1957 = Bundle(w3784, w3785) -> (w3781:cluster{dbl[], dbl[]})  [unwired: 1 in]
        n1958 = Bundle By Name(cluster=w3789, "PumpTemps"=w3781, "Compressor.CompressorTemp"=w3777) -> (w3790:T31)
      }
      frame "receiveLastError" {
        w3808 = T51 0 items=["no dialog", "OK message", "continue or stop message", "OK message + warnings", "continue/stop + warnings"] ("type of dialog (OK msg:1)")
        n1959 = Unflatten From JSON(JSON string=w3814, type and defaults=T38 {"time"=[], "event"=[], "item"=[], "itemID"=[], "details"=[], "actions"=[]}, default null elements? (F)=TRUE) -> (value=w3802:T38, error out=w3809:errorcluster)  [unwired: 4 in]
        n1960 = Unbundle By Name(w3802) -> ("time"=w3799:string[])
        n1961 = call <vilib>:"Simple Error Handler.vi"("type of dialog (OK msg:1)"=w3808, "error in (no error)"=w3809) -> ("error?"=w3792:bool, "code out"=w3795:i32)  [unwired: 3 in, 3 out]
        n1962 = Equal?(x=w3795, y=-375008) -> (x = y?=w3793:bool)
        n1963 = Index Array(array=w3799, index=0) -> (element=w3798:string)
        n1964 = Not Exclusive Or(1:w3793, 2:w3792) -> (0:w3791:bool)
        n1965 = Equal?(x=w3798, y="") -> (x = y?=w3800:bool)
        n1966 = And(x=w3791, y=w3800) -> (x .and. y?=w3803:bool)
        n1967 = Unbundle By Name(w3807) -> ("ErrorArray"=w3805:string[][], "MasterErrorArray"=w3806:string[][])
        n1968 = case shown="False" w3803 {
          tunnel: [w3837 w3885] -> w3812
          tunnel: w3802 -> [w3836 _]
          tunnel: w3806 -> [w3835 w3885]
          tunnel: w3805 -> [w3834 w3884]
          tunnel: [w3833 w3884] -> w3804
          frame False {
            n1969 = Unbundle By Name(w3836) -> ("time"=w3825:string[], "event"=w3826:string[], "item"=w3820:string[], "itemID"=w3819:i32[], "details"=w3818:string[])
            n1970 = control-ref of="Active Errors"() -> (w3816:refnum<vi>)
            n1971 = Array Size(array=w3825) -> (size(s)=w3824:i32)
            n1972 = property class="Bool (strict)"(reference=w3816, "Value"=TRUE) -> ()  [unwired: 1 in, 2 out]
            n1973 = control-ref of="Current Errors (click to clear)"() -> (w3817:refnum<vi>)
            n1974 = Initialize Array("", 7 ("dimension size")) -> (w3830:string[])
            n1975 = for {
              N: w3824 -> [_]
              shift-right: [w3869] -> w3837
              shift-left: w3835 -> [w3864]
              tunnel: w3826 -> [w3858]
              tunnel: w3825 -> [w3850]
              shift-right: [w3868] -> w3833
              shift-left: w3834 -> [w3838]
              tunnel: w3820 -> [w3849]
              tunnel: w3819 -> [w3847]
              tunnel: w3818 -> [w3842]
              shift-right: [w3870] -> w3829
              shift-left: w3817 -> [w3865]
              shift-right: [w3841] -> _
              shift-left: w3830 -> [w3861]
              i -> [w3840]
              n1976 = Index Array(array=w3838, index (col)=2 ("index (row)")) -> (element=w3866:string[])  [unwired: 1 in]
              n1977 = Index Array(array=w3858, index=w3840) -> (element=w3860:string)
              n1978 = Search 1D Array(1D array=w3866, element=w3860) -> (index of element=w3863:i32)  [unwired: 1 in]
              n1979 = Less Than 0?(x=w3863) -> (x < 0?=w3862:bool)
              n1980 = Replace Array Subset(array=w3861, new element=w3860, index=2) -> (w3857:string[])
              n1981 = Index Array(array=w3850, index=w3840) -> (element=w3851:string)
              n1982 = Bundle(w3840, 2) -> (w3871:cluster{i32, i32})  [unwired: 1 in]
              n1983 = Replace Array Subset(array=w3857, new element=w3851, index=1) -> (w3853:string[])
              n1984 = property on="Property Node" class="MCListbox (strict)"(reference=w3865, "ActiveCell"=w3871) -> (reference out=w3870:refnum<vi>)  [unwired: 1 in, 1 out]
              n1985 = Index Array(array=w3849, index=w3840) -> (element=w3848:string)
              n1986 = Replace Array Subset(array=w3853, new element=w3848, index=3) -> (w3852:string[])
              n1987 = Index Array(array=w3847, index=w3840) -> (element=w3846:i32)
              n1988 = Number To Decimal String(number=w3846) -> (decimal integer string=w3845:string)  [unwired: 1 in]
              n1989 = Replace Array Subset(array=w3852, new element=w3845, index=4) -> (w3839:string[])
              n1990 = Index Array(array=w3842, index=w3840) -> (element=w3843:string)
              n1991 = Replace Array Subset(array=w3839, new element=w3843, index=5) -> (w3841:string[])
              n1992 = case shown="True" w3862 {
                tunnel: [w3880 w3882] -> w3869
                tunnel: w3838 -> [w3877 w3883]
                tunnel: [w3879 w3883] -> w3868
                tunnel: w3864 -> [w3878 w3882]
                tunnel: w3841 -> [w3876 _]
                frame True {
                  n1993 = Build Array (concatenate)(w3876, w3877) -> (w3879:string[][])
                  n1994 = Build Array (concatenate)(w3876, w3878) -> (w3880:string[][])
                  n1995 = One Button Dialog(message="There has been an error", button name ("OK")="Proceed to Error Log") -> (true=w3873:bool)
                  n1996 = case shown="True" w3873 {
                    frame False {
                    }
                    frame True {
                      n1997 = local write "Tab Control"(T2."General Status" ("Tab Control")) -> ()
                    }
                  }
                }
                frame False {
                }
              }
            }
            n1998 = Array Size(array=w3833) -> (size(s)=w3823:i32[])
            n1999 = property class="MCListbox (strict)"(reference=w3829, "ItemNames"=w3833) -> ()  [unwired: 1 in, 2 out]
            n2000 = Index Array(array=w3823, index=0) -> (element=w3821:i32)
            n2001 = Initialize Array(37, w3821) -> (w3827:i32[])
            n2002 = property class="MCListbox (strict)"(reference=w3829, "ItemSyms"=w3827) -> ()  [unwired: 1 in, 2 out]
          }
          frame True {
          }
        }
        n2003 = Bundle By Name(cluster=w3807, "MasterErrorArray"=w3812, "ErrorArray"=w3804) -> (w3813:T31)
      }
      frame "receiveLastEvent" {
        w3900 = T51 0 items=["no dialog", "OK message", "continue or stop message", "OK message + warnings", "continue/stop + warnings"] ("type of dialog (OK msg:1)")
        n2004 = Unflatten From JSON(JSON string=w3906, type and defaults=T39 {"time"=[], "category"=[], "message"=[]}, default null elements? (F)=TRUE) -> (value=w3895:T39, error out=w3901:errorcluster)  [unwired: 4 in]
        n2005 = Unbundle By Name(w3895) -> ("time"=w3893:string[])
        n2006 = call <vilib>:"Simple Error Handler.vi"("type of dialog (OK msg:1)"=w3900, "error in (no error)"=w3901) -> ("error?"=w3889:bool)  [unwired: 3 in, 4 out]
        n2007 = Index Array(array=w3893, index=0) -> (element=w3892:string)
        n2008 = Not(x=w3889) -> (.not. x?=w3888:bool)
        n2009 = Equal?(x=w3892, y="") -> (x = y?=w3886:bool)
        n2010 = And(x=w3888, y=w3886) -> (x .and. y?=w3887:bool)
        n2011 = Unbundle By Name(w3899) -> ("EventArray"=w3897:string[][], "MasterEventArray"=w3898:string[][])
        n2012 = case shown="False" w3887 {
          tunnel: [w3926 w3958] -> w3904
          tunnel: w3895 -> [w3925 _]
          tunnel: w3898 -> [w3924 w3958]
          tunnel: w3897 -> [w3923 w3957]
          tunnel: [w3907 w3957] -> w3896
          frame False {
            n2013 = Unbundle By Name(w3925) -> ("time"=w3915:string[], "message"=w3916:string[], "category"=w3910:string[])
            n2014 = Array Size(array=w3915) -> (size(s)=w3914:i32)
            n2015 = Initialize Array("", 4 ("dimension size")) -> (w3920:string[])
            n2016 = for {
              N: w3914 -> [_]
              tunnel: w3920 -> [w3946]
              tunnel: [w3944] -> w3919
              shift-right: [w3940] -> w3926
              shift-left: w3924 -> [w3934]
              tunnel: w3916 -> [w3941]
              tunnel: w3915 -> [w3933]
              shift-right: [w3938] -> w3907
              shift-left: w3923 -> [w3939]
              tunnel: w3910 -> [w3928]
              i -> [w3932]
              n2017 = Index Array(array=w3934, index (col)=1 ("index (row)")) -> (element=w3936:string[])  [unwired: 1 in]
              n2018 = Index Array(array=w3933, index=w3932) -> (element=w3931:string)
              n2019 = control-ref of="Current Events (click to clear)"() -> (w3949:refnum<vi>)
              n2020 = Replace Array Subset(array=w3946, new element=w3941, index=3) -> (w3943:string[])
              n2021 = Search 1D Array(1D array=w3936, element=w3931) -> (index of element=w3935:i32)  [unwired: 1 in]
              n2022 = Replace Array Subset(array=w3943, new element=w3931, index=1) -> (w3929:string[])
              n2023 = Replace Array Subset(array=w3929, new element=w3928, index=2) -> (w3930:string[])
              n2024 = case shown="-1" w3935 {
                tunnel: [w3950 w3956] -> w3940
                tunnel: w3939 -> [w3951 w3954]
                tunnel: [w3951 w3955] -> w3938
                tunnel: w3930 -> [_ w3953]
                tunnel: w3934 -> [w3950 w3952]
                frame 0, Default {
                }
                frame -1 {
                  n2025 = Build Array (concatenate)(w3953, w3954) -> (w3955:string[][])
                  n2026 = Build Array (concatenate)(w3953, w3952) -> (w3956:string[][])
                }
              }
              n2027 = Bundle(w3932, 2) -> (w3947:cluster{i32, i32})  [unwired: 1 in]
              n2028 = property on="Property Node" class="MCListbox (strict)"(reference=w3949, "ActiveCell"=w3947) -> (reference out=w3944:refnum<vi>)  [unwired: 1 in, 1 out]
            }
            n2029 = control-ref of="Complete Event List"() -> (w3909:refnum<vi>)
            n2030 = Array Size(array=w3907) -> (size(s)=w3913:i32[])
            n2031 = property class="MCListbox (strict)"(reference=w3919, "ItemNames"=w3907) -> ()  [unwired: 1 in, 2 out]
            n2032 = Index Array(array=w3913, index=0) -> (element=w3911:i32)
            n2033 = Initialize Array(37, w3911) -> (w3917:i32[])
            n2034 = property class="MCListbox (strict)"(reference=w3919, "ItemSyms"=w3917) -> ()  [unwired: 1 in, 2 out]
            n2035 = property class="MCListbox (strict)"(reference=w3909, "ItemNames"=w3907) -> ()  [unwired: 1 in, 2 out]
            n2036 = control-ref of="Complete Event List 2"() -> (w3908:refnum<vi>)
            n2037 = property class="MCListbox (strict)"(reference=w3908, "ItemNames"=w3907) -> ()  [unwired: 1 in, 2 out]
          }
          frame True {
          }
        }
        n2038 = Bundle By Name(cluster=w3899, "MasterEventArray"=w3904, "EventArray"=w3896) -> (w3905:T31)
      }
      frame "receivePressure" {
        n2039 = Unflatten From JSON(JSON string=w3960, type and defaults=T40 {"CryoPressure"=0.0, "ChamberPressure"=0.0, "RoughingPressure"=0.0}, default null elements? (F)=TRUE) -> (value=w3966:T40)  [unwired: 4 in, 1 out]
        n2040 = Unbundle By Name(w3966) -> ("RoughingPressure"=w3965:dbl, "CryoPressure"=w3964:dbl, "ChamberPressure"=w3963:dbl)
        n2041 = Build Array(w3965, w3964, w3963) -> (w3967:dbl[])
        n2042 = Bundle By Name(cluster=w3969, "Pressure"=w3967) -> (w3968:T31)
      }
      frame "receiveSystemPower" {
        n2043 = Unflatten From JSON(JSON string=w3973, type and defaults=T41 {"pfeiffer_gauge"=FALSE, "shi_compressor"=FALSE, "shi_mcc"=FALSE, "tdk_lambda"=FALSE, "thermocouple"=FALSE, "pc_104"=FALSE}, default null elements? (F)=TRUE) -> (value=→"value":T41)  [unwired: 4 in, 1 out]
      }
      frame "receiveTC" {
        w3980 = 15
        n2044 = Unflatten From JSON(JSON string=w4006, type and defaults=T33 {"time"="", "TCs"=[]} ("Cluster"), default null elements? (F)=TRUE) -> (value=w3991:T33)  [unwired: 4 in, 1 out]
        n2045 = control-ref of="TC1to75visual"() -> (w4003:refnum<vi>)
        n2046 = Unbundle By Name(w3991) -> ("TCs"=w3981:T28)
        n2047 = property class="Clust (strict)"(reference=w4003) -> ("Controls[]"=w4001:refnum<vi>[])  [unwired: 1 in, 2 out]
        n2048 = Bundle By Name(cluster=w4007, "TCs"=w3981) -> (w3984:T31)
        n2049 = for {
          tunnel: w3981 -> [w4024] mode=indexing
          shift-right: [w4022] -> w3989
          shift-left: -inf -> [w4023]
          shift-right: [w4020] -> w3986
          shift-left: inf -> [w4021]
          n2050 = Unbundle By Name(w4024) -> ("temp"=w4018:dbl)
          n2051 = Not Equal To 0?(x=w4018) -> (x != 0?=w4019:bool)
          n2052 = Select(t=w4018, s=w4019, f=inf) -> (s? t:f=w4016:dbl)
          n2053 = Max & Min(x=w4021, y=w4016) -> (min(x,y)=w4020:dbl)  [unwired: 1 out]
          n2054 = Max & Min(x=w4023, y=w4018) -> (max(x,y)=w4022:dbl)  [unwired: 1 out]
        }
        n2055 = for {
          N: 75 -> [_]
          tunnel: w4001 -> [w4051] mode=indexing
          tunnel: w3981 -> [w4053] mode=indexing
          n2056 = Unbundle By Name(w4053) -> ("temp"=w4052:dbl)
          n2057 = Number To Decimal String(number=w4052) -> (decimal integer string=w4050:string)  [unwired: 1 in]
          n2058 = property class="Ctl"(reference=w4051, "TipStrip"=w4050) -> ()  [unwired: 1 in, 2 out]
        }
        n2059 = Unbundle By Name(w3984) -> ("MaxMinTemps"=w3990:dbl[])
        n2060 = Initialize Array(0.0 ("element"), 30 ("dimension size")) -> (w3996:dbl[])
        n2061 = Replace Array Subset(array=w3990, new element=w3989, index=0) -> (w3987:dbl[])
        n2062 = Initialize Array(0.0 ("element"), w3980) -> (w3978:dbl[])
        n2063 = for {
          N: 30 -> [_]
          shift-right: [w4027] -> w3995
          shift-left: w3996 -> [w4028]
          tunnel: w3981 -> [w4026]
          i -> [w4025]
          n2064 = In Range and Coerce(upper limit=5 ("lower limit"), x=w4025, lower limit=0) -> (In Range?=w4031:bool)  [unwired: 1 out]
          n2065 = case shown="False" w4031 {
            tunnel: w4028 -> [w4040 w4049]
            tunnel: w4025 -> [w4038 w4047]
            tunnel: [w4039 w4048] -> w4027
            tunnel: w4026 -> [w4037 w4043]
            tunnel: w4025 -> [w4036 w4042]
            frame False {
              n2066 = Add(x=90, y=w4036) -> (x+y=w4034:i32)
              n2067 = Index Array(array=w4037, index=w4034) -> (element=w4033:T53)
              n2068 = Unbundle By Name(w4033) -> ("temp"=w4032:dbl)
              n2069 = Replace Array Subset(array=w4040, new element=w4032, index=w4038) -> (w4039:dbl[])
            }
            frame True {
              n2070 = Add(x=75, y=w4042) -> (x+y=w4045:i32)
              n2071 = Index Array(array=w4043, index=w4045) -> (element=w4044:T53)
              n2072 = Unbundle By Name(w4044) -> ("temp"=w4041:dbl)
              n2073 = Replace Array Subset(array=w4049, new element=w4041, index=w4047) -> (w4048:dbl[])
            }
          }
        }
        n2074 = Replace Array Subset(array=w3987, new element=w3986, index=1) -> (w3982:dbl[])
        n2075 = for {
          N: w3980 -> [_]
          tunnel: w3981 -> [w4013]
          shift-right: [w4008] -> w3977
          shift-left: w3978 -> [w4010]
          i -> [w4011]
          n2076 = Add(x=80, y=w4011) -> (x+y=w4012:i32)
          n2077 = Index Array(array=w4013, index=w4012) -> (element=w4014:T53)
          n2078 = Unbundle By Name(w4014) -> ("temp"=w4009:dbl)
          n2079 = Replace Array Subset(array=w4010, new element=w4009, index=w4011) -> (w4008:dbl[])
        }
        n2080 = Array To Cluster(array=w3977) -> (cluster=w3976:T54)
        n2081 = local write "Miscellaneous TCs"(w3976) -> ()
        n2082 = Array To Cluster(array=w3995) -> (cluster=w3994:T55)
        n2083 = local write "Chamber Layout"(w3994) -> ()
        n2084 = Bundle By Name(cluster=w3984, "MaxMinTemps"=w3982) -> (w3983:T31)
      }
      frame "receiveTvacStatus" {
        n2085 = Unflatten From JSON(JSON string=w4106, type and defaults=T26 {"recordData"=FALSE, "currentSetpoint"=0, "vacuumWanted"=FALSE, "inPause"=FALSE, "activeProfile"=FALSE, "inRamp"=FALSE, "inHold"=FALSE, "CryoPressure"=0.0, "ChamberPressure"=0.0, "RoughingPressure"=0.0, "OperationalVacuum"=FALSE, "VacuumState"=""} ("OperationalVacuum"), default null elements? (F)=TRUE) -> (value=w4102:T26)  [unwired: 4 in, 1 out]
        n2086 = Bundle By Name(cluster=w4101, "TvacStatus"=w4102) -> (w4072:T31)
        n2087 = Initialize Array(0.0 ("element"), 9 ("dimension size")) -> (w4087:dbl[])
        n2088 = Unbundle By Name(w4072) -> ("TvacStatus"=w4083:T26, "ZoneTemps.ZoneTemps"=w4086:dbl[])
        n2089 = Array Size(array=w4086) -> (size(s)=w4089:i32)
        n2090 = for {
          N: w4089 -> [_]
          shift-right: [w4115] -> _
          shift-left: w4086 -> [w4116]
          shift-right: [w4107] -> w4085
          shift-left: w4087 -> [w4110]
          shift-right: [w4108] -> _
          shift-left: 0 ("dimension size") -> [w4109]
          i -> [w4114]
          n2091 = Quotient & Remainder(x=w4114, y=2) -> (x-y*floor(x/y)=w4112:i32)  [unwired: 1 out]
          n2092 = Equal To 0?(x=w4112) -> (x = 0?=w4111:bool)
          n2093 = case shown="True" w4111 {
            tunnel: w4116 -> [w4117 w4120]
            tunnel: [w4117 w4120] -> w4115
            tunnel: w4114 -> [_ w4126]
            tunnel: w4110 -> [w4118 w4123]
            tunnel: w4109 -> [w4119 w4125]
            tunnel: [w4119 w4124] -> w4108
            tunnel: [w4118 w4121] -> w4107
            frame False {
            }
            frame True {
              n2094 = Index Array(array=w4120, index=w4126) -> (element=w4122:dbl)
              n2095 = Replace Array Subset(array=w4123, new element=w4122, index=w4125) -> (w4121:dbl[])
              n2096 = Increment(x=w4125) -> (x+1=w4124:i32)
            }
          }
        }
        n2097 = Unbundle By Name(w4083) -> ("recordData"=w4074:bool, "currentSetpoint"=w4100:i32, "vacuumWanted"=w4062:bool, "inPause"=w4095:bool, "activeProfile"=w4099:bool, "inRamp"=w4094:bool, "inHold"=w4093:bool, "CryoPressure"=w4097:dbl, "ChamberPressure"=w4096:dbl, "RoughingPressure"=w4098:dbl, "OperationalVacuum"=w4075:bool, "VacuumState"=w4054:string)
        n2098 = case shown="False" w4095 {
          tunnel: w4094 -> [w4129 _]
          tunnel: w4093 -> [w4128 _]
          tunnel: [w4127 "Paused"] -> w4092
          frame False {
            n2099 = case shown="False" w4129 {
              tunnel: w4128 -> [w4131 _]
              tunnel: [w4130 "Ramping"] -> w4127
              frame False {
                n2100 = case shown="True" w4131 {
                  tunnel: ["" "Holding"] -> w4130
                  frame False {
                  }
                  frame True {
                  }
                }
              }
              frame True {
              }
            }
          }
          frame True {
          }
        }
        n2101 = local write "Database Logging On/Off"(w4074) -> ()
        n2102 = control-ref of="Vacuum State"() -> (w4055:refnum<vi>)
        n2103 = Select(t=TRUE, s=w4062, f=FALSE) -> (s? t:f=w4060:bool)
        n2104 = property class="Str"(reference=w4055, "Text.Text"=w4054) -> ()  [unwired: 1 in, 2 out]
        n2105 = control-ref of="Vacuum State"() -> (w4061:refnum<vi>)
        n2106 = property class="Bool (strict)"(reference=w4061, "Value"=w4060) -> ()  [unwired: 1 in, 2 out]
        n2107 = Unbundle By Name(w4072) -> ("MaxMinTemps"=w4071:dbl[])
        n2108 = Number To Fractional String(number=w4071, precision (6)=i16 2) -> (F-format string=w4070:string[])  [unwired: 2 in]
        n2109 = Unbundle By Name(w4083) -> ("currentSetpoint"=w4076:i32, "vacuumWanted"=w4080:bool, "activeProfile"=w4066:bool, "CryoPressure"=w4079:dbl, "ChamberPressure"=w4078:dbl, "RoughingPressure"=w4077:dbl, "recordData"=w4073:bool)
        "Active Profile" <- w4066
        n2110 = control-ref of="Active Errors"() -> (w4057:refnum<vi>)
        n2111 = Index Array(array=w4070, index #1=0 ("index"), index #2=1 ("index")) -> (element #1=w4064:string, element #2=w4063:string)
        n2112 = Bundle By Name(cluster=T43 {"Set Point"=0.0, "Vacuum Wanted"=FALSE, "Profile State"="", "Active Profile"=FALSE, "Roughing"=0.0, "Cryo"=0.0, "Chamber"=0.0, "Zone Temps"=[], "At Vacuum"=FALSE, "recordData"=FALSE, "Max Temp"="", "Min Temp"=""} ("tpStatus"), "Set Point"=w4100, "Vacuum Wanted"=w4062, "Profile State"=w4092, "Active Profile"=w4099, "Roughing"=w4098, "Cryo"=w4097, "Chamber"=w4096, "Zone Temps"=w4085, "At Vacuum"=w4075, "recordData"=w4074, "Max Temp"=w4064, "Min Temp"=w4063) -> (w4065:T43)
        n2113 = local write "tpStatus"(w4065) -> ()
        n2114 = local write "GenStatus"(w4065) -> ()
        n2115 = property class="Bool (strict)"(reference=w4057) -> ("Value"=w4056:bool)  [unwired: 1 in, 2 out]
        n2116 = Bundle By Name(cluster=T42 {"At Vaccum"=FALSE, "Vacuum Wanted"=FALSE, "Roughing"=0.0, "Cryo"=0.0, "Chamber"=0.0, "Active Profile"=FALSE, "Set Point"=0.0, "Max Temp"="", "Min Temp"="", "Active Errors"=FALSE, "recordData"=FALSE} ("Taskbar Status"), "At Vaccum"=w4075, "Vacuum Wanted"=w4080, "Roughing"=w4077, "Cryo"=w4079, "Chamber"=w4078, "Active Profile"=w4066, "Set Point"=w4076, "recordData"=w4073, "Max Temp"=w4064, "Min Temp"=w4063, "Active Errors"=w4056) -> (w4081:T42)
        n2117 = local write "Taskbar Status"(w4081) -> ()
      }
      frame "receiveZoneTemps" {
        n2118 = Unflatten From JSON(JSON string=w4139, type and defaults=cluster{"ZoneTemps":dbl[]} {"ZoneTemps"=[]}, default null elements? (F)=TRUE) -> (value=w4137:cluster{"ZoneTemps":dbl[]})  [unwired: 4 in, 1 out]
        n2119 = Bundle By Name(cluster=w4141, "ZoneTemps"=w4137) -> (w4142:T31)
      }
      frame "masterDatabase" {
        n2120 = Unbundle By Name(w4156) -> ("Thermocouples"=w4157:T3, "Pressure"=w4149:dbl[], "PumpTemps"=w4152:T29, "NumberTCs"=w4158:i32, "ZoneTemps"=w4146:cluster{"ZoneTemps":dbl[]}, "Compressor.CompressorTemp"=w4144:dbl)  [unwired: 1 out]
        n2121 = Initialize Array(0.0 ("element"), w4158) -> (w4160:dbl[])
        n2122 = Unbundle(w4152) -> ("Cp Stage 1 Temp"=w4151:dbl[], "Cp Stage 2 Temp"=w4150:dbl[])
        n2123 = Unbundle(w4146) -> ("ZoneTemps"=w4145:dbl[])
        n2124 = Build Array (concatenate)(w4151, w4150) -> (w4148:dbl[])
        n2125 = Build Array(w4144) -> (w4143:dbl[])
        n2126 = for {
          N: w4158 -> [_]
          shift-right: [w4170] -> w4147
          shift-left: w4160 -> [w4171]
          tunnel: w4157 -> [w4166]
          i -> [w4168]
          n2127 = Quotient & Remainder(x=w4168, y=4) -> (x-y*floor(x/y)=w4165:i32, floor(x/y)=w4167:i32)
          n2128 = Index Array(array=w4166, index (row)=w4167, index (col)=w4165) -> (element=w4164:T32)
          n2129 = Unbundle By Name(w4164) -> ("Temperature"=w4163:string)
          n2130 = Fract/Exp String To Number(string=w4163) -> (number=w4162:dbl)  [unwired: 3 in, 1 out]
          n2131 = To Double Precision Float(number=w4162) -> (double precision float=w4172:dbl)
          n2132 = Replace Array Subset(array=w4171, new element=w4172, index=w4168) -> (w4170:dbl[])
        }
        n2133 = Build Array (concatenate)(dbl[] [0.0], w4149, w4145, w4147, w4148, w4143) -> (w4154:dbl[])
        n2134 = Bundle By Name(cluster=w4156, "Database"=w4154) -> (w4155:T31)
      }
      frame "multipleGraphs" {
        n2135 = Not Equal?(x=w4176, y="1000") -> (x != y?=w4177:bool)
        n2136 = case shown="True" w4177 {
          tunnel: w4176 -> [_ w4184]
          tunnel: [_ w4182] -> w4174
          tunnel: [1000 ("row") w4181] -> w4173
          frame False {
          }
          frame True {
            n2137 = Unflatten From JSON(JSON string=w4184, type and defaults=cluster{"graph":i32, "row":i32} {"graph"=0, "row"=0}) -> (value=w4183:cluster{"graph":i32, "row":i32})  [unwired: 5 in, 1 out]
            n2138 = Unbundle By Name(w4183) -> ("graph"=w4182:i32, "row"=w4181:i32)
          }
        }
        n2139 = for {
          N: 6 ("Numeric") -> [_]
          tunnel: w4179 -> [w4199]
          tunnel: w4174 -> [w4190]
          tunnel: w4173 -> [w4186]
          i -> [w4187]
          n2140 = case shown="0, Default" w4187 {
            tunnel: [w4244 w4245 w4247 w4249 w4251 w4253] -> w4192
            tunnel: [w4243 w4246 w4248 w4250 w4252 w4254] -> w4191
            frame 0, Default {
              n2141 = control-ref of="Custom Chart 1 Selection"() -> (w4243:refnum<vi>)
              n2142 = control-ref of="Custom Chart 1"() -> (w4244:refnum<vi>)
            }
            frame 1 {
              n2143 = control-ref of="Custom Chart 2 Selection"() -> (w4246:refnum<vi>)
              n2144 = control-ref of="Custom Chart 2"() -> (w4245:refnum<vi>)
            }
            frame 2 {
              n2145 = control-ref of="Custom Chart 3 Selection"() -> (w4248:refnum<vi>)
              n2146 = control-ref of="Custom Chart 3"() -> (w4247:refnum<vi>)
            }
            frame 3 {
              n2147 = control-ref of="Custom Chart 4 Selection"() -> (w4250:refnum<vi>)
              n2148 = control-ref of="Custom Chart 4"() -> (w4249:refnum<vi>)
            }
            frame 4 {
              n2149 = control-ref of="Custom Chart 5 Selection"() -> (w4252:refnum<vi>)
              n2150 = control-ref of="Custom Chart 5"() -> (w4251:refnum<vi>)
            }
            frame 5 {
              n2151 = control-ref of="Custom Chart 6 Selection"() -> (w4254:refnum<vi>)
              n2152 = control-ref of="Custom Chart 6"() -> (w4253:refnum<vi>)
            }
          }
          n2153 = Equal?(x=w4190, y=w4187) -> (x = y?=w4188:bool)
          n2154 = Unbundle By Name(w4199) -> ("Database"=w4197:dbl[], "numSensors"=w4198:i32)
          n2155 = case shown="True" w4188 {
            tunnel: [w4202 w4207] -> w4196
            tunnel: [1000 w4204] -> w4195
            tunnel: w4191 -> [w4203 w4206]
            tunnel: [FALSE w4205] -> w4189
            tunnel: w4186 -> [_ w4204]
            frame False {
              n2156 = property on="Property Node" class="LstBox (strict)"(reference=w4203) -> ("Item Symbols"=w4202:i32[])  [unwired: 1 in, 2 out]
            }
            frame True {
              n2157 = property on="Property Node" class="LstBox (strict)"(reference=w4206) -> ("Item Symbols"=w4207:i32[])  [unwired: 1 in, 2 out]
              n2158 = Index Array(array=w4207, index=0) -> (element=w4208:i32)
              n2159 = Equal?(x=37, y=w4208) -> (x = y?=w4210:bool)
              n2160 = Equal To 0?(x=w4204) -> (x = 0?=w4212:bool)
              n2161 = And(x=w4210, y=w4212) -> (x .and. y?=w4205:bool)
            }
          }
          n2162 = case shown="False" w4189 {
            tunnel: [0 ("index") w4319] -> w4194
            tunnel: w4198 -> [w4261 w4315]
            tunnel: w4197 -> [w4260 _]
            tunnel: [w4259 _] -> w4193
            tunnel: w4195 -> [w4257 w4319]
            tunnel: w4196 -> [w4258 w4318]
            tunnel: w4191 -> [w4256 w4314]
            tunnel: w4192 -> [w4255 w4313]
            frame False {
              n2163 = for {
                N: w4261 -> [_]
                tunnel: [w4284] -> w4259 mode=indexing
                tunnel: w4257 -> [w4268]
                tunnel: w4258 -> [w4274]
                tunnel: w4260 -> [w4269] mode=indexing
                tunnel: w4256 -> [w4272]
                tunnel: w4255 -> [w4264]
                i -> [w4265]
                n2164 = Equal?(x=w4268, y=-1) -> (x = y?=w4266:bool)
                n2165 = Wait (ms)(milliseconds to wait=u32 0) -> ()  [unwired: 1 out]
                n2166 = case shown="True" w4266 {
                  tunnel: w4265 -> [_ w4288]
                  tunnel: w4264 -> [_ w4287]
                  frame False {
                  }
                  frame True {
                    n2167 = property on="Property Node" class="WFChart (strict)"(reference=w4287, "Active Plot"=w4288) -> (reference out=w4285:refnum<vi>)  [unwired: 1 in, 1 out]
                    n2168 = property on="Property Node" class="WFChart (strict)"(reference=w4285, "Plot.Visible?"=FALSE ("Plot.Visible")) -> ()  [unwired: 1 in, 2 out]
                  }
                }
                n2169 = Equal To 0?(x=w4269) -> (x = 0?=w4271:bool)
                n2170 = Not A Number/Path/Refnum?(number/path/refnum=w4269) -> (NaN/Path/Refnum?=w4270:bool)
                n2171 = Or(x=w4270, y=w4271) -> (x .or. y?=w4263:bool)
                n2172 = case shown="True" w4263 {
                  tunnel: [w4291 waveform(dbl) {"t0"=timestamp(0 s since 1904-01-01), "dt"=1.0, "Y"=[]}] -> w4284
                  tunnel: w4269 -> [w4289 _]
                  frame False {
                    n2173 = Get Date/Time In Seconds() -> (seconds since 1Jan1904=w4293:timestamp)
                    n2174 = Bundle By Name("t0"=w4293) -> (w4292:waveform(dbl))  [unwired: 1 in]
                    n2175 = Build Array(w4289) -> (w4290:dbl[])
                    n2176 = Bundle By Name(cluster=w4292, "Y"=w4290) -> (w4291:waveform(dbl))
                  }
                  frame True {
                  }
                }
                n2177 = Index Array(array=w4274, index=w4268) -> (element=w4277:i32)
                n2178 = Index Array(array=w4274, index=w4268) -> (element=w4279:i32)
                n2179 = Equal?(x=w4277, y=38) -> (x = y?=w4276:bool)
                n2180 = Equal?(x=w4279, y=37) -> (x = y?=w4281:bool)
                n2181 = Equal?(x=w4265, y=w4268) -> (x = y?=w4275:bool)
                n2182 = And(x=w4275, y=w4276) -> (x .and. y?=w4273:bool)
                n2183 = And(x=w4275, y=w4281) -> (x .and. y?=w4280:bool)
                n2184 = case shown="True" w4280 {
                  tunnel: w4274 -> [w4312 _]
                  tunnel: w4268 -> [_ _]
                  tunnel: w4265 -> [w4307 _]
                  tunnel: w4264 -> [w4306 _]
                  tunnel: w4272 -> [w4305 _]
                  frame True {
                    n2185 = property on="Property Node" class="WFChart (strict)"(reference=w4306, "Active Plot"=w4307) -> (reference out=w4310:refnum<vi>)  [unwired: 1 in, 1 out]
                    n2186 = Replace Array Subset(array=w4312, new element=38, index=w4307) -> (w4308:i32[])
                    n2187 = property on="Property Node" class="WFChart (strict)"(reference=w4306) -> ("Plot.Plot Color"=w4304:u32)  [unwired: 1 in, 2 out]
                    n2188 = property on="Property Node" class="WFChart (strict)"(reference=w4310, "Plot.Visible?"=TRUE ("Plot.Visible")) -> ()  [unwired: 1 in, 2 out]
                    n2189 = property on="Property Node" class="LstBox (strict)"(reference=w4305, "Active Row"=w4307) -> ()  [unwired: 1 in, 2 out]
                    n2190 = property on="Property Node" class="LstBox (strict)"(reference=w4305, "CellBG"=w4304) -> ()  [unwired: 1 in, 2 out]
                    n2191 = property on="Property Node" class="LstBox (strict)"(reference=w4305, "Item Symbols"=w4308) -> ()  [unwired: 1 in, 2 out]
                  }
                  frame False {
                  }
                }
                n2192 = case shown="True" w4273 {
                  tunnel: w4274 -> [_ w4303]
                  tunnel: w4265 -> [_ w4296]
                  tunnel: w4264 -> [_ w4297]
                  tunnel: w4272 -> [_ w4298]
                  frame False {
                  }
                  frame True {
                    n2193 = property on="Property Node" class="WFChart (strict)"(reference=w4297, "Active Plot"=w4296) -> (reference out=w4301:refnum<vi>)  [unwired: 1 in, 1 out]
                    n2194 = Replace Array Subset(array=w4303, new element=37, index=w4296) -> (w4299:i32[])
                    n2195 = property on="Property Node" class="WFChart (strict)"(reference=w4301, "Plot.Visible?"=FALSE ("Plot.Visible")) -> ()  [unwired: 1 in, 2 out]
                    n2196 = property on="Property Node" class="LstBox (strict)"(reference=w4298, "Active Row"=w4296) -> ()  [unwired: 1 in, 2 out]
                    n2197 = property on="Property Node" class="LstBox (strict)"(reference=w4298, "CellBG"=u32 13816530 ("Active Row:Cell Background Color")) -> ()  [unwired: 1 in, 2 out]
                    n2198 = property on="Property Node" class="LstBox (strict)"(reference=w4298, "Item Symbols"=w4299) -> ()  [unwired: 1 in, 2 out]
                  }
                }
              }
            }
            frame True {
              n2199 = for {
                N: w4315 -> [_]
                tunnel: w4318 -> [_]
                tunnel: w4314 -> [w4321]
                tunnel: w4313 -> [w4320]
                i -> [w4322]
                n2200 = property on="Property Node" class="WFChart (strict)"(reference=w4320, "Active Plot"=w4322) -> (reference out=w4325:refnum<vi>)  [unwired: 1 in, 1 out]
                n2201 = property on="Property Node" class="WFChart (strict)"(reference=w4325, "Plot.Visible?"=FALSE ("Plot.Visible")) -> ()  [unwired: 1 in, 2 out]
                n2202 = property on="Property Node" class="LstBox (strict)"(reference=w4321, "Active Row"=w4322) -> ()  [unwired: 1 in, 2 out]
                n2203 = property on="Property Node" class="LstBox (strict)"(reference=w4321, "CellBG"=u32 13816530 ("Active Row:Cell Background Color")) -> ()  [unwired: 1 in, 2 out]
              }
              n2204 = Initialize Array(37, w4315) -> (w4316:i32[])
              n2205 = property on="Property Node" class="LstBox (strict)"(reference=w4314, "Item Symbols"=w4316) -> ()  [unwired: 1 in, 2 out]
            }
          }
          n2206 = case shown="0, Default" w4187 {
            tunnel: w4194 -> [w4216 w4219 w4224 w4229 w4234 w4239]
            tunnel: w4193 -> [w4214 w4218 w4223 w4228 w4233 w4238]
            frame 0, Default {
              n2207 = Build Array (concatenate)(waveform(dbl) {"t0"=timestamp(0 s since 1904-01-01), "dt"=1.0, "Y"=[]} ("element"), w4214) -> (w4213:waveform(dbl)[])
              n2208 = Delete From Array(array=w4213, index=w4216) -> (array with subset deleted=→"Custom Chart 1":waveform(dbl)[])  [unwired: 1 in, 1 out]
            }
            frame 1 {
              n2209 = Build Array (concatenate)(waveform(dbl) {"t0"=timestamp(0 s since 1904-01-01), "dt"=1.0, "Y"=[]} ("element"), w4218) -> (w4222:waveform(dbl)[])
              n2210 = Delete From Array(array=w4222, index=w4219) -> (array with subset deleted=→"Custom Chart 2":waveform(dbl)[])  [unwired: 1 in, 1 out]
            }
            frame 2 {
              n2211 = Build Array (concatenate)(waveform(dbl) {"t0"=timestamp(0 s since 1904-01-01), "dt"=1.0, "Y"=[]} ("element"), w4223) -> (w4227:waveform(dbl)[])
              n2212 = Delete From Array(array=w4227, index=w4224) -> (array with subset deleted=→"Custom Chart 3":waveform(dbl)[])  [unwired: 1 in, 1 out]
            }
            frame 3 {
              n2213 = Build Array (concatenate)(waveform(dbl) {"t0"=timestamp(0 s since 1904-01-01), "dt"=1.0, "Y"=[]} ("element"), w4228) -> (w4232:waveform(dbl)[])
              n2214 = Delete From Array(array=w4232, index=w4229) -> (array with subset deleted=→"Custom Chart 4":waveform(dbl)[])  [unwired: 1 in, 1 out]
            }
            frame 4 {
              n2215 = Build Array (concatenate)(waveform(dbl) {"t0"=timestamp(0 s since 1904-01-01), "dt"=1.0, "Y"=[]} ("element"), w4233) -> (w4237:waveform(dbl)[])
              n2216 = Delete From Array(array=w4237, index=w4234) -> (array with subset deleted=→"Custom Chart 5":waveform(dbl)[])  [unwired: 1 in, 1 out]
            }
            frame 5 {
              n2217 = Build Array (concatenate)(waveform(dbl) {"t0"=timestamp(0 s since 1904-01-01), "dt"=1.0, "Y"=[]} ("element"), w4238) -> (w4242:waveform(dbl)[])
              n2218 = Delete From Array(array=w4242, index=w4239) -> (array with subset deleted=→"Custom Chart 6":waveform(dbl)[])  [unwired: 1 in, 1 out]
            }
          }
        }
      }
      frame "exit" {
        n2219 = Unbundle By Name(w4327) -> ("Http session"=w4328:T30)
        n2220 = call <vilib>:"CloseHandle.vi"("client handle"=w4328, "error in (no error)"=w4330) -> ("error out"=w4329:errorcluster)  [unwired: 13 in]
        n2221 = Bundle By Name(cluster=w4327, "go"=FALSE ("Bundle Element")) -> (w4331:T31)
      }
      frame Default {
        n2222 = call "Unknown Message Dialog.vi"("error in (no error)"=w4334, "event name"=w4333) -> ("error out"=w4332:errorcluster)  [unwired: 9 in]
      }
    }
    n2223 = control-ref of="This VI"() -> (w75:refnum<vi>)
    n2224 = property class="VI"(reference=w75) -> ("Panel"=w74:refnum<vi>)  [unwired: 1 in, 2 out]
    n2225 = property class="Pnl"(reference=w74, "DeferPanUpdts"=FALSE ("Defer Panel Updates")) -> ()  [unwired: 1 in, 2 out]
    n2226 = Unbundle By Name(w79) -> ("go"=w72:bool)
    n2227 = call "log system event.vi"("error in (no error)"=w76) -> ("error out"=w80:errorcluster, "description"=→"system log event":string)  [unwired: 9 in]
    n2228 = call <vilib>:"Simple Error Handler.vi"("error in (no error)"=w76) -> ()  [unwired: 4 in, 5 out]
  }
  n2229 = control-ref of="This VI"() -> (w6:refnum<vi>)
  n2230 = property class="VI"(reference=w6) -> ("Panel"=w5:refnum<vi>)  [unwired: 1 in, 2 out]
  n2231 = property class="Pnl"(reference=w5, "DeferPanUpdts"=TRUE ("Defer Panel Updates")) -> ()  [unwired: 1 in, 2 out]
  n2232 = while {
    shift-right: [w4339] -> _
    shift-left: "Moving 1" -> [w4340]
    tunnel: T25[] [{"Left"=436, "Top"=451}, {"Left"=477, "Top"=451}, {"Left"=519, "Top"=451}, {"Left"=561, "Top"=451}, {"Left"=602, "Top"=451}, {"Left"=644, "Top"=451}, {"Left"=686, "Top"=451}, {"Left"=727, "Top"=451}, {"Left"=769, "Top"=451}, {"Left"=811, "Top"=451}, {"Left"=851, "Top"=449}, {"Left"=894, "Top"=451}, {"Left"=935, "Top"=451}, {"Left"=977, "Top"=451}, {"Left"=1019, "Top"=451}, {"Left"=1062, "Top"=451}, {"Left"=1103, "Top"=451}, {"Left"=1145, "Top"=451}, {"Left"=1187, "Top"=451}, {"Left"=1228, "Top"=451}, {"Left"=437, "Top"=486}, {"Left"=479, "Top"=486}, {"Left"=520, "Top"=486}, {"Left"=562, "Top"=486}, {"Left"=604, "Top"=486}, {"Left"=645, "Top"=486}, {"Left"=687, "Top"=486}, {"Left"=729, "Top"=486}, {"Left"=770, "Top"=486}, {"Left"=812, "Top"=486}, {"Left"=851, "Top"=484}, {"Left"=894, "Top"=486}, {"Left"=936, "Top"=486}, {"Left"=978, "Top"=486}, {"Left"=1019, "Top"=486}, {"Left"=1061, "Top"=486}, {"Left"=1103, "Top"=486}, {"Left"=1144, "Top"=486}, {"Left"=1186, "Top"=486}, {"Left"=1228, "Top"=486}, {"Left"=438, "Top"=520}, {"Left"=480, "Top"=520}, {"Left"=522, "Top"=520}, {"Left"=563, "Top"=520}, {"Left"=605, "Top"=520}, {"Left"=646, "Top"=521}, {"Left"=687, "Top"=520}, {"Left"=729, "Top"=520}, {"Left"=771, "Top"=520}, {"Left"=812, "Top"=520}, {"Left"=854, "Top"=520}, {"Left"=895, "Top"=520}, {"Left"=936, "Top"=520}, {"Left"=978, "Top"=520}, {"Left"=1020, "Top"=520}, {"Left"=1061, "Top"=520}, {"Left"=1101, "Top"=520}, {"Left"=1145, "Top"=520}, {"Left"=1186, "Top"=520}, {"Left"=1228, "Top"=520}, {"Left"=439, "Top"=554}, {"Left"=480, "Top"=554}, {"Left"=522, "Top"=554}, {"Left"=564, "Top"=554}, {"Left"=605, "Top"=554}, {"Left"=647, "Top"=554}, {"Left"=688, "Top"=554}, {"Left"=730, "Top"=554}, {"Left"=772, "Top"=554}, {"Left"=813, "Top"=554}, {"Left"=854, "Top"=554}, {"Left"=896, "Top"=554}, {"Left"=936, "Top"=554}, {"Left"=978, "Top"=554}, {"Left"=1020, "Top"=554}] ("TCs1to75InitialPositions") -> [w4338]
    stop <- w4336 stop-if-true
    n2233 = event shown="[1] Timeout" {
      selector: _ -> [_ _ _ _ _]
      dyn-events: _ -> [_ _ _ _ _]
      timeout: 500 -> [_ _ _ _ _]
      tunnel: w4340 -> [w4341 _ _ _ _]
      tunnel: [w4341 _ FALSE TRUE _] -> w4339
      tunnel: w4338 -> [_ _ _ _ w4395]
      tunnel: [_ w4391 _ _ _] -> w4336
      event "TC1to75visual": Mouse Move {
        n2234 = event-data() -> ("Coords"=w4342:T45)  [unwired: 1 in]
        n2235 = local read "Moving 1"() -> (w4343:bool)
        n2236 = case shown="False" w4343 {
          tunnel: w4341 -> [w4344 w4382]
          tunnel: w4342 -> [w4345 w4380]
          frame False {
            n2237 = control-ref of="TC1to75visual"() -> (w4348:refnum<vi>)
            n2238 = property class="Clust (strict)"(reference=w4348) -> ("Controls[]"=w4346:refnum<vi>[])  [unwired: 1 in, 2 out]
            n2239 = for {
              N: 75 -> [_]
              shift-right: [w4350] -> _
              shift-left: w4345 -> [w4353]
              tunnel: w4346 -> [w4365] mode=indexing
              tunnel: w4344 -> [w4351]
              n2240 = property class="Ctl"(reference=w4365) -> (reference out=w4352:refnum<vi>, "Position"=w4354:T25)  [unwired: 1 in, 1 out]
              n2241 = Unbundle By Name(w4353) -> ("Horizontal"=w4361:i32, "Vertical"=w4360:i32)
              n2242 = Unbundle By Name(w4354) -> ("Left"=w4355:i32, "Top"=w4358:i32)
              n2243 = Add(x=w4358, y=24) -> (x+y=w4359:i32)
              n2244 = Add(x=w4355, y=32) -> (x+y=w4364:i32)
              n2245 = In Range and Coerce(upper limit=w4364, x=w4361, lower limit=w4355) -> (In Range?=w4357:bool)  [unwired: 1 out]
              n2246 = In Range and Coerce(upper limit=w4359, x=w4360, lower limit=w4358) -> (In Range?=w4356:bool)  [unwired: 1 out]
              n2247 = And(x=w4357, y=w4356) -> (x .and. y?=w4349:bool)
              n2248 = case shown="False" w4349 {
                tunnel: w4353 -> [w4366 w4368]
                tunnel: w4352 -> [_ w4370]
                tunnel: w4351 -> [_ w4369]
                tunnel: [w4366 w4367] -> w4350
                frame False {
                }
                frame True {
                  n2249 = local write "TC1to45PicRef"(w4370) -> ()
                  n2250 = case shown="False" w4369 {
                    selector: w4369 -> [_ w4378]
                    tunnel: w4370 -> [_ w4379]
                    tunnel: w4368 -> [w4371 w4372]
                    tunnel: [w4371 w4372] -> w4367
                    frame False {
                    }
                    frame True {
                      n2251 = local write "Moving 1"(w4378) -> ()
                      n2252 = property class="Ctl"(reference=w4379) -> (reference out=w4373:refnum<vi>, "Position"=w4377:T25)  [unwired: 1 in, 1 out]
                      n2253 = Divide(x=w4377, y=T56 {"Width"=2, "Height"=2}) -> (x/y=w4375:cluster{dbl, dbl})
                      n2254 = Subtract(x=w4372, y=w4375) -> (x-y=w4374:cluster{dbl, dbl})
                      n2255 = property on="Property Node" class="Ctl"(reference=w4373, "Position"=w4374) -> ()  [unwired: 1 in, 2 out]
                    }
                  }
                }
              }
            }
          }
          frame True {
            n2256 = local read "TC1to45PicRef"() -> (w4381:refnum<vi>)
            n2257 = case shown="True" w4382 {
              selector: w4382 -> [_ w4390]
              tunnel: w4381 -> [_ w4389]
              tunnel: w4380 -> [_ w4384]
              frame False {
              }
              frame True {
                # "Place control where the mouse is."
                n2258 = local write "Moving 1"(w4390) -> ()
                n2259 = property class="Ctl"(reference=w4389) -> (reference out=w4385:refnum<vi>, "Bounds"=w4387:T56)  [unwired: 1 in, 1 out]
                n2260 = Divide(x=w4387, y=T56 {"Width"=2, "Height"=2}) -> (x/y=w4383:cluster{"Width":dbl, "Height":dbl})
                n2261 = Subtract(x=w4384, y=w4383) -> (x-y=w4386:cluster{dbl, dbl})
                n2262 = property on="Property Node" class="Ctl"(reference=w4385, "Position"=w4386) -> ()  [unwired: 1 in, 2 out]
              }
            }
          }
        }
      }
      event Timeout {
        n2263 = event-data() -> ()  [unwired: 1 in, 3 out]
        n2264 = local read "exit"() -> (w4391:bool)
      }
      event "TC1to75visual": Mouse Up {
        # "This case is needed to unlock cursor from the Boolean."
        n2265 = event-data() -> ()  [unwired: 1 in, 1 out]
        n2266 = local write "Moving 1"(FALSE ("Moving 1")) -> ()
      }
      event "TC1to75visual": Mouse Down {
        # "Begin moving Boolean with cursor when the mouse button is pressed."
        n2267 = event-data() -> ()  [unwired: 1 in, 1 out]
      }
      event "Reset All TC Positions": Mouse Down {
        n2268 = event-data() -> ()  [unwired: 1 in, 1 out]
        n2269 = control-ref of="TC1to75visual"() -> (w4397:refnum<vi>)
        n2270 = property class="Clust (strict)"(reference=w4397) -> ("Controls[]"=w4396:refnum<vi>[])  [unwired: 1 in, 2 out]
        n2271 = for {
          N: 75 -> [_]
          tunnel: w4396 -> [w4400] mode=indexing
          tunnel: w4395 -> [w4399] mode=indexing
          n2272 = property class="Ctl"(reference=w4400, "Position"=w4399) -> ()  [unwired: 1 in, 2 out]
        }
      }
    }
  }
  n2273 = case shown="True" FALSE {
    frame False {
    }
    frame True {
      n2274 = control-ref of="TC1to75visual"() -> (w4405:refnum<vi>)
      n2275 = property class="Clust (strict)"(reference=w4405) -> ("Controls[]"=w4404:refnum<vi>[])  [unwired: 1 in, 2 out]
      n2276 = Initialize Array(T25 {"Left"=0, "Top"=0} ("Position"), 75 ("dimension size")) -> (w4401:T25[])
      n2277 = for {
        N: 75 -> [_]
        tunnel: w4404 -> [w4411] mode=indexing
        shift-right: [w4409] -> _
        shift-left: w4401 -> [w4410]
        i -> [w4407]
        # "Delete at End"
        n2278 = property class="Ctl"(reference=w4411) -> ("Position"=w4408:T25)  [unwired: 1 in, 2 out]
        n2279 = Replace Array Subset(array=w4410, new element=w4408, index=w4407) -> (w4409:T25[])
      }
    }
  }
  n2280 = call "Flush Module Queue.vi"("error in (no error)"=w27) -> ("error out"=w26:errorcluster)  [unwired: 9 in, 1 out]
  n2281 = call "Unload Module.vi"("error in (no error)"=w26) -> ("error out"=→"error out":errorcluster)  [unwired: 10 in]
  n2282 = property on="Waveform Chart" class="WFChart (strict)" props=["Plot", "Visible?"]() -> ()  [unwired: 2 in, 3 out]
